vi "NoGV_Omniax_MotorDrive_XYZR_20112StableILK.vi"() -> ()   [LabVIEW 2010]
uses:
  <vilib>/Utility/file.llb/Read From Spreadsheet File (string).vi
  <vilib>/Utility/file.llb/Read From Spreadsheet File (DBL).vi
  <vilib>/Instr/_visa.llb/VISA Configure Serial Port (Instr).vi
  <vilib>/Utility/file.llb/Write To Spreadsheet File (string).vi
  <vilib>/Utility/file.llb/Write To Spreadsheet File (DBL).vi
panel:
  in  "GVposition SP 15360000":i64
  out "Scanning":bool
  out "Laser Shutter":bool
  in  "SHUTTER SYNC":bool
  in  "Laser Shutter":bool
  out "#th loop":dbl
  in  "# of loops":dbl
  in  "LOOP":bool
  out "OP":bool
  out "CL":bool
  out "V5 Valve \nopend/closed":bool
  in  "OK Button":bool
  out "STATUS":string
  in  "Delete Button":bool
  in  "String":string
  in  "Add Button":bool
  in  "Set Button":bool
  in  "Preset positions":i32(ring) items=["ZERO", "Default", "CDOSE", "QMS", "test", "test2", "test3", "yag position", "Sample Long Edge  ", "SPUTTER POS"]
  out "Presets":i32[][](array[numeric])
  out "X MINPOS":i32=-94296
  out "X MAXPOS":i32=-34296
  out "Y MINPOS":i32=-94296
  out "Y MAXPOS":i32=-34296
  out "R MAXPOS":i32=-34296
  out "R MINPOS":i32=-94296
  out "Z MINPOS":i32=-94296
  out "Z MAXPOS":i32=-34296
  in  "HARDSTOP":bool
  in  "GO":bool
  out "XYZR VEL PV Array":i32[](array[numeric])
  out "XYZ in RANGE Array":bool[](array[boolean])
  out "STEP SP Array":i32[](array[numeric])
  out "RUNHOLDArray":i32[](array[numeric])
  out "ZCONSTArray":dbl[](array[numeric])
  out "RCONSTArray":dbl[](array[numeric])
  out "XCONSTArray":dbl[](array[numeric])
  out "YCONSTArray":dbl[](array[numeric])
  out "Error Array":errorcluster[](array[cluster])
  out "COM PORT Array":refnum<visa-resource-name>[](array[refnum])
  out "Z COM PORT":refnum<visa-resource-name>="COM6"
  in  "Tab Control 3":enum32{"Status", "Reset"}(tab)
  out "Y in Range":bool
  out "Y Scan":bool
  out "Y in Motion":bool
  out "Y Backlash corr":bool
  out "X  in Range":bool
  out "X Scan":bool
  out "X  in Motion":bool
  out "X Backlash corr":bool
  out "Z in Range":bool
  out "Z Scan":bool
  out "Z in Motion":bool
  out "Z Backlash corr":bool
  out "R in Range":bool
  out "R Scan":bool
  out "R in Motion":bool
  out "R Backlash corr":bool
  out "X Ready":bool
  out "Y Ready":bool
  out "Z Ready":bool
  out "R Ready":bool
  in  "Reset Y Position mm":dbl
  out "Reset Y Motor Steps":i32
  in  "Reset X Position mm":dbl
  out "Reset X Motor Steps":i32
  in  "Reset Z Position mm":dbl
  out "Reset Z Motor Steps":i32
  in  "Reset R Position deg":dbl
  out "Reset R Motor Steps":i32
  in  "Reset":bool
  in  "Tab Control 2":enum32{"mm", "step"}(tab)
  in  "X Scan Length SP mm":dbl
  in  "X Scan Velocity SP mm/sec":dbl
  in  "Y Scan Length SP mm":dbl
  in  "Y Scan Velocity SP mm/sec":dbl
  in  "Set Scan \nParameters":bool
  in  "Z Scan Length SP mm":dbl
  in  "Z Scan Velocity SP mm/sec":dbl
  in  "R Scan Length SP deg":dbl
  in  "R Scan Velocity SP deg/sec":dbl
  in  "Z as dominating length":bool
  in  "X Scan Velocity SP steps/sec":i32=1 min=1 max=102400 step=1
  in  "X Scan Length SP steps":i32 min=-2304000 max=2304000 step=100
  out "X Scan length MV mm":dbl
  out "X Scan velocity MV mm/sec":dbl format="%#_6f"
  in  "Y Scan Velocity SP steps/sec":i32=1 min=1 max=102400 step=1
  in  "Y Scan Length SP steps":i32 min=-2304000 max=2304000 step=100
  out "Y Scan length MV mm":dbl
  out "Y Scan velocity MV mm/sec":dbl format="%#_6f"
  in  "Z Scan Velocity SP steps/sec":i32=1 min=1 max=204800 step=1
  in  "Z Scan Length SP steps":i32 min=-10240000 max=92160000 step=100
  out "Z Scan length MV mm":dbl
  out "Z Scan velocity MV mm/sec":dbl format="%#_6f"
  in  "R Scan Velocity SP steps/sec":i32=1 min=1 max=102400 step=1
  in  "R Scan Length SP steps":i32 min=-1501867 max=4642133 step=100
  out "R Scan length MV deg":dbl
  out "R Scan velocity MV deg/sec":dbl format="%#_6f"
  out "atan Y/Z":dbl
  in  "Tab Control":enum32{"mm", "step"}(tab)
  in  "X Position SP mm":dbl
  in  "X Velocity SP mm/sec":dbl
  in  "X Move Set":bool
  in  "Y Move Set":bool
  in  "Y Position SP mm":dbl
  in  "Y Velocity SP mm/sec":dbl
  in  "Z Position SP mm":dbl
  in  "Z Velocity SP mm/sec":dbl
  in  "Z Move Set":bool
  in  "R Position SP deg":dbl
  in  "R Velocity SP deg/sec":dbl
  in  "R Move Set":bool
  in  "X Velocity SP step/sec":i32 min=1 max=128000
  out "X Velocity MV mm/sec":dbl
  in  "Y Velocity SP step/sec":i32 min=1 max=128000
  out "Y Velocity MV mm/sec":dbl
  in  "Z Velocity SP step/sec":i32 min=1 max=204800
  out "Z Velocity MV mm/sec":dbl
  in  "R Velocity SP step/sec":i32 min=1 max=20000
  out "R Velocity MVdeg/sec":dbl
  in  "Y Step SP":i32=-20000 min=-2304000 max=2304000 step=500
  out "Y Position MV mm":dbl
  in  "X Step SP":i32=-20000 min=-2304000 max=2304000 step=500
  out "X Position MV mm":dbl
  in  "Z Step SP":i32=-20000 min=0 max=102400000 step=500
  out "Z Position MV mm":dbl
  in  "R Step SP":i32=-20000 min=-6144000 max=0 step=500
  out "R Position MV deg":dbl
  out "X Step PV":i32 max=2000
  out "Y Step PV":i32 max=2000
  out "Z Step PV":i32 max=2000
  out "R Step PV":i32 max=2000
  in  "Clear ZY":bool
  out "ZY Graph":cluster{dbl[], dbl[]}(graph)
  out "ZR Graph":cluster{"Y":dbl[], "Y":dbl[]}[](graph)
  out "XY Graph":cluster{"Y":dbl[], "Y":dbl[]}[](graph)
  out "X Scan Duration":dbl
  out "Y Scan Duration":dbl
  out "Z Scan Duration":dbl
  out "R Scan Duration":dbl
  out "R Backlash steps/sec":i32
  out "R Backlash":i32
  out "R Holding Current %":i32
  out "R Run Current %":i32
  out "R offset deg":dbl
  out "R deg/rev":dbl
  out "R steps/rev":u32
  out "R velocity PV step/sec":i32
  out "R COM PORT":refnum<visa-resource-name>="COM5"
  out "R Position deg PV":dbl=270.5
  out "Z Backlash steps/sec":i32
  out "Z Backlash":i32
  out "Z Holding Current %":i32
  out "Z Run Current %":i32
  out "Z offset mm":dbl
  out "Z mm/rev":dbl
  out "Z steps/rev":u32
  out "Z  velocity PV step/sec":i32
  out "Z Position mm PV":dbl=45.0
  out "X Position mm PV":dbl
  out "X velocity PV step/sec":i32
  in  "Send scan parameter":bool
  out "X Backlash steps/sec":i32
  out "X Backlash":i32
  out "X Holding Current %":i32
  out "X Run Current %":i32
  out "X offset mm":dbl
  out "X mm/rev":dbl
  out "X steps/rev":u32
  out "X COM PORT":refnum<visa-resource-name>="COM5"
  out "Y Backlash steps/sec":i32
  out "Y Backlash":i32
  out "Y Holding Current %":i32
  out "Y Run Current %":i32
  in  "Scan Cancel":bool
  out "Y Position mm PV":dbl
  out "Y offset mm":dbl
  out "Y mm/rev":dbl
  out "Y steps/rev":u32
  out "Y velocity PV step/sec":i32
  in  "Scan Go":bool
  in  "Stop":bool
  out "Y COM PORT":refnum<visa-resource-name>="COM5"
  # "MX"
  # "MY"
  # "MZ"
  # "MR"
  # "V5 Indicators"
  # "L"
  # "M"
  # "B"
  # "S"
  # "R"
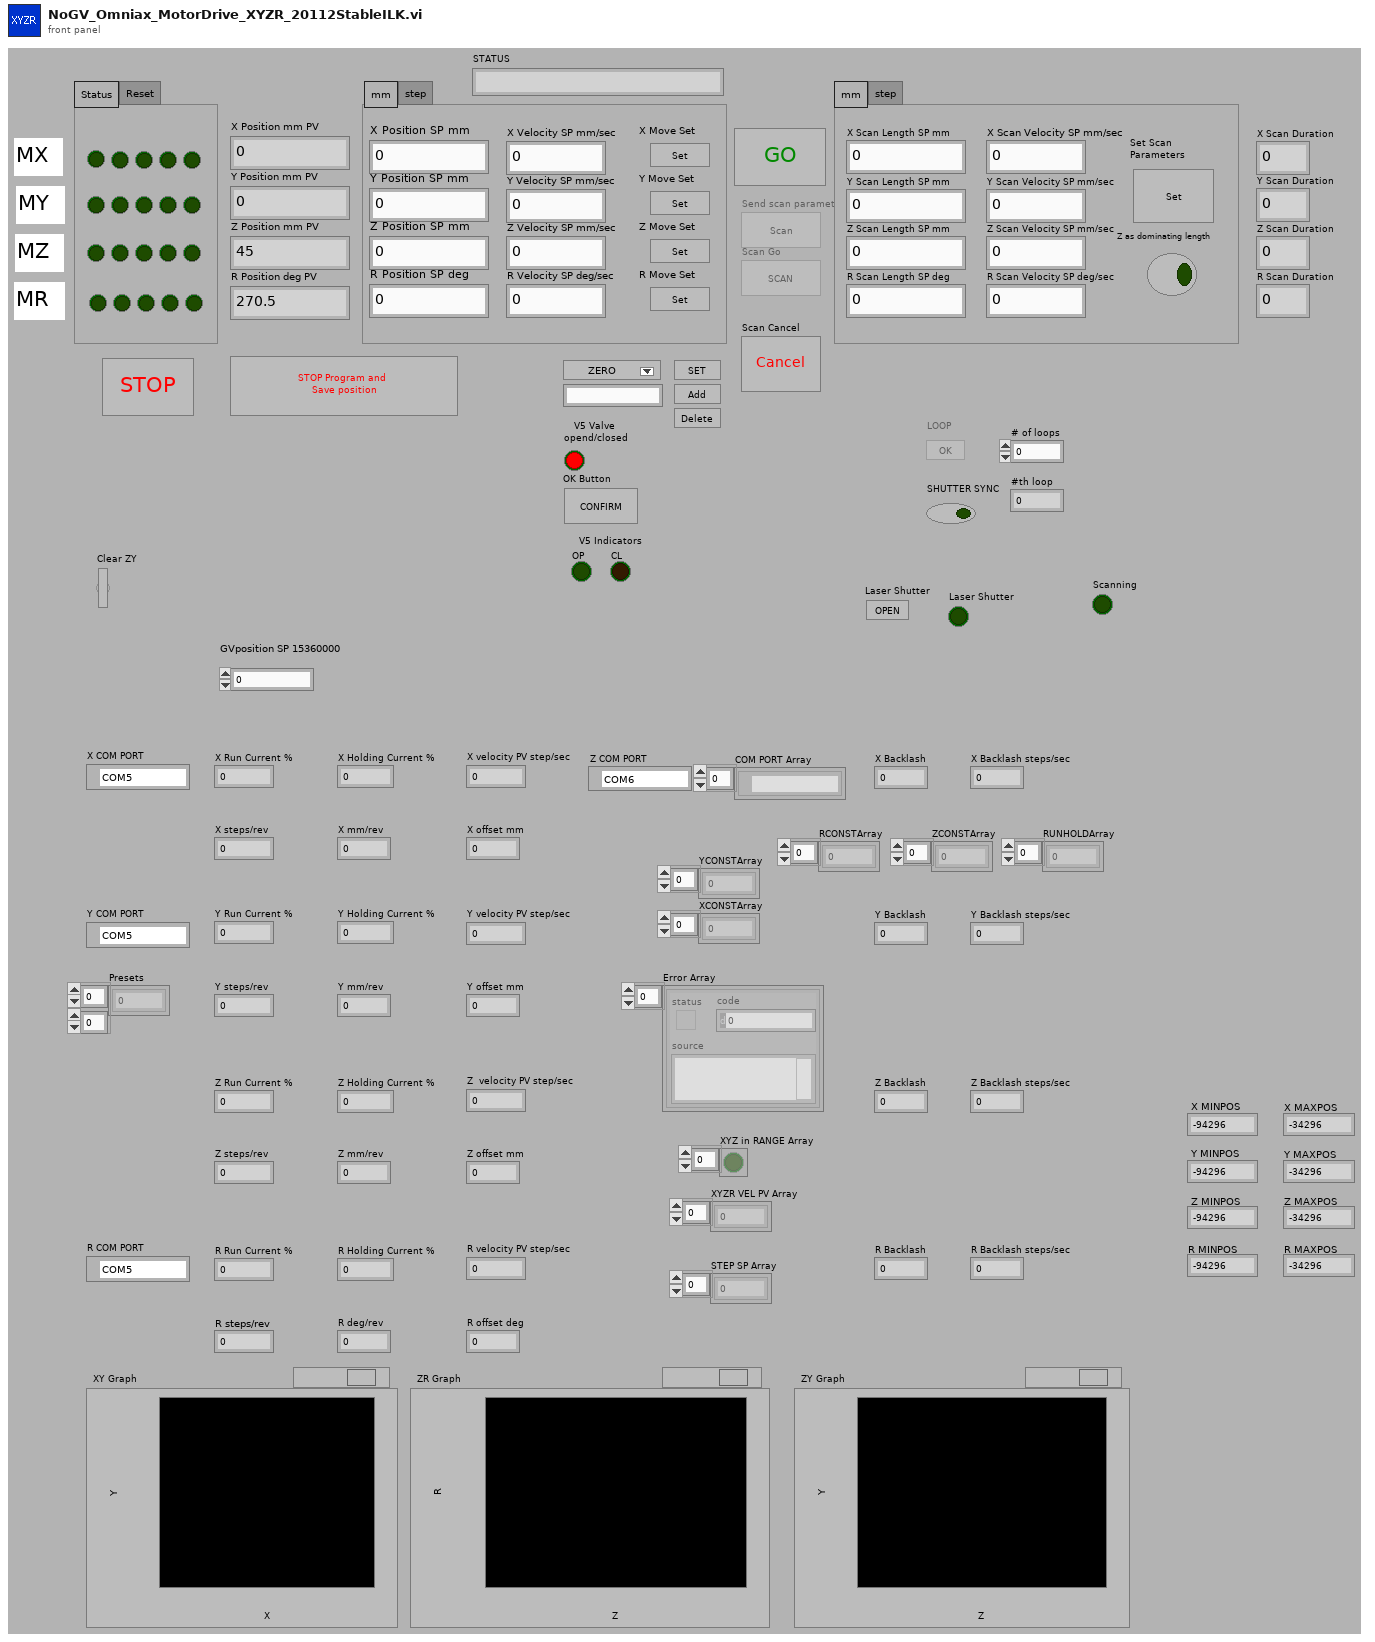
[diagram p1: front panel]
types:
  T1 = cluster{"Error Array OUT[0]":errorcluster, "Error Array OUT[1]":errorcluster, "Error Array OUT[2]":errorcluster, "Error Array OUT[3]":errorcluster, "Error Array OUT[4]":errorcluster, "Error Array OUT[5]":errorcluster, "Error Array OUT[6]":errorcluster, "Error Array OUT[7]":errorcluster, "Error Array OUT[8]":errorcluster}
  T2 = cluster{"COM PORT Array OUT[0]":refnum<visa-resource-name>, "COM PORT Array OUT[1]":refnum<visa-resource-name>, "COM PORT Array OUT[2]":refnum<visa-resource-name>, "COM PORT Array OUT[3]":refnum<visa-resource-name>, "COM PORT Array OUT[4]":refnum<visa-resource-name>, "COM PORT Array OUT[5]":refnum<visa-resource-name>, "COM PORT Array OUT[6]":refnum<visa-resource-name>, "COM PORT Array OUT[7]":refnum<visa-resource-name>, "COM PORT Array OUT[8]":refnum<visa-resource-name>}
  T3 = cluster{"STEP SP Array OUT[0]":i32, "STEP SP Array OUT[1]":i32, "STEP SP Array OUT[2]":i32, "STEP SP Array OUT[3]":i32, "STEP SP Array OUT[4]":i32, "STEP SP Array OUT[5]":i32, "STEP SP Array OUT[6]":i32, "STEP SP Array OUT[7]":i32, "STEP SP Array OUT[8]":i32}
  T4 = cluster{"XYZR MAX MIN POS[0]":i32, "XYZR MAX MIN POS[1]":i32, "XYZR MAX MIN POS[2]":i32, "XYZR MAX MIN POS[3]":i32, "XYZR MAX MIN POS[4]":i32, "XYZR MAX MIN POS[5]":i32, "XYZR MAX MIN POS[6]":i32, "XYZR MAX MIN POS[7]":i32, "XYZR MAX MIN POS[8]":i32}
  T5 = cluster{"XYZ in RANGE Array OUT[0]":bool, "XYZ in RANGE Array OUT[1]":bool, "XYZ in RANGE Array OUT[2]":bool, "XYZ in RANGE Array OUT[3]":bool, "XYZ in RANGE Array OUT[4]":bool, "XYZ in RANGE Array OUT[5]":bool, "XYZ in RANGE Array OUT[6]":bool, "XYZ in RANGE Array OUT[7]":bool, "XYZ in RANGE Array OUT[8]":bool}
  T6 = cluster{"XY Max Min array OUT[0]":dbl, "XY Max Min array OUT[1]":dbl, "XY Max Min array OUT[2]":dbl, "XY Max Min array OUT[3]":dbl, "XY Max Min array OUT[4]":dbl, "XY Max Min array OUT[5]":dbl, "XY Max Min array OUT[6]":dbl, "XY Max Min array OUT[7]":dbl, "XY Max Min array OUT[8]":dbl}
  T7 = cluster{"XYZR VEL PV Array OUT[0]":i32, "XYZR VEL PV Array OUT[1]":i32, "XYZR VEL PV Array OUT[2]":i32, "XYZR VEL PV Array OUT[3]":i32, "XYZR VEL PV Array OUT[4]":i32, "XYZR VEL PV Array OUT[5]":i32, "XYZR VEL PV Array OUT[6]":i32, "XYZR VEL PV Array OUT[7]":i32, "XYZR VEL PV Array OUT[8]":i32}
  T8 = cluster{"[0]":i32, "[1]":i32, "[2]":i32, "[3]":i32, "[4]":i32, "[5]":i32, "[6]":i32, "[7]":i32, "[8]":i32}
  T9 = enum8{"Enabled", "Disabled", "Disabled and Grayed Out"}
  T10 = enum16{"Stop", "Reset", "Run Current", "Holding Current", "Accel Rate", "Decel Rate", "Move to Relative Position", "Move to Absolute Position", "Echo Mode", "Print Parameter", "Send String", "Microstep Resolution", "Set Current Position", "Max Velocity"}
  T11 = cluster{"Presets[0]":i32, "Presets[1]":i32, "Presets[2]":i32, "Presets[3]":i32, "Presets[4]":i32, "Presets[5]":i32, "Presets[6]":i32, "Presets[7]":i32, "Presets[8]":i32}
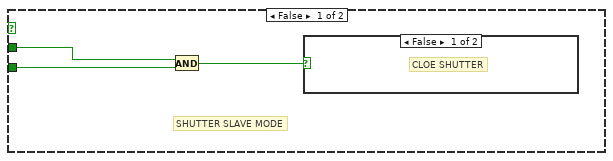
[diagram p2: hidden frame]
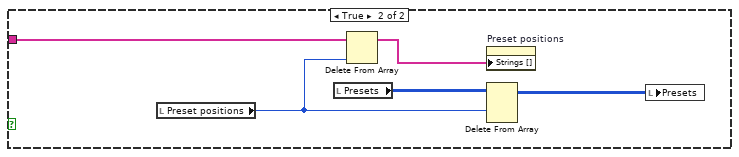
[diagram p4: hidden frame]
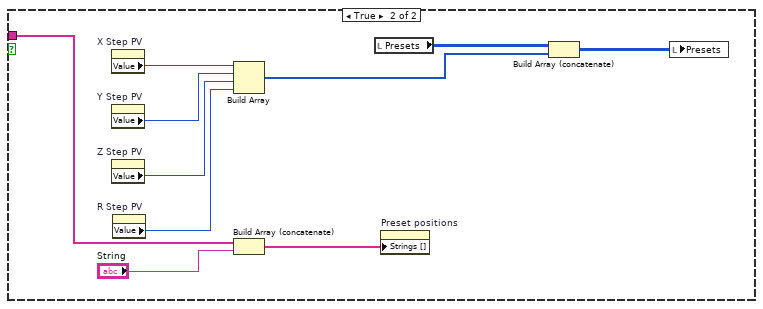
[diagram p5: hidden frame]
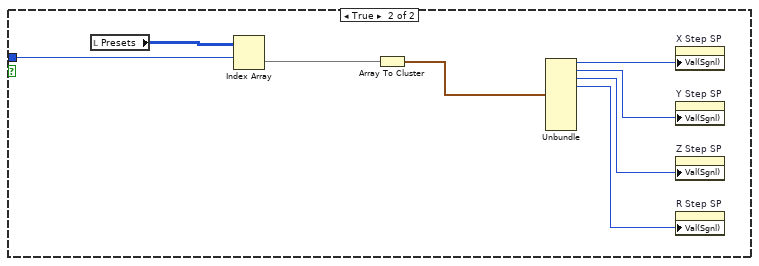
[diagram p6: hidden frame]
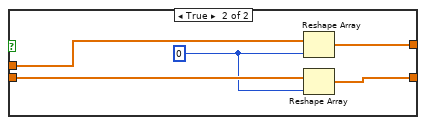
[diagram p8: hidden frame]
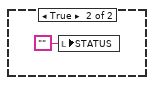
[diagram p10: hidden frame]
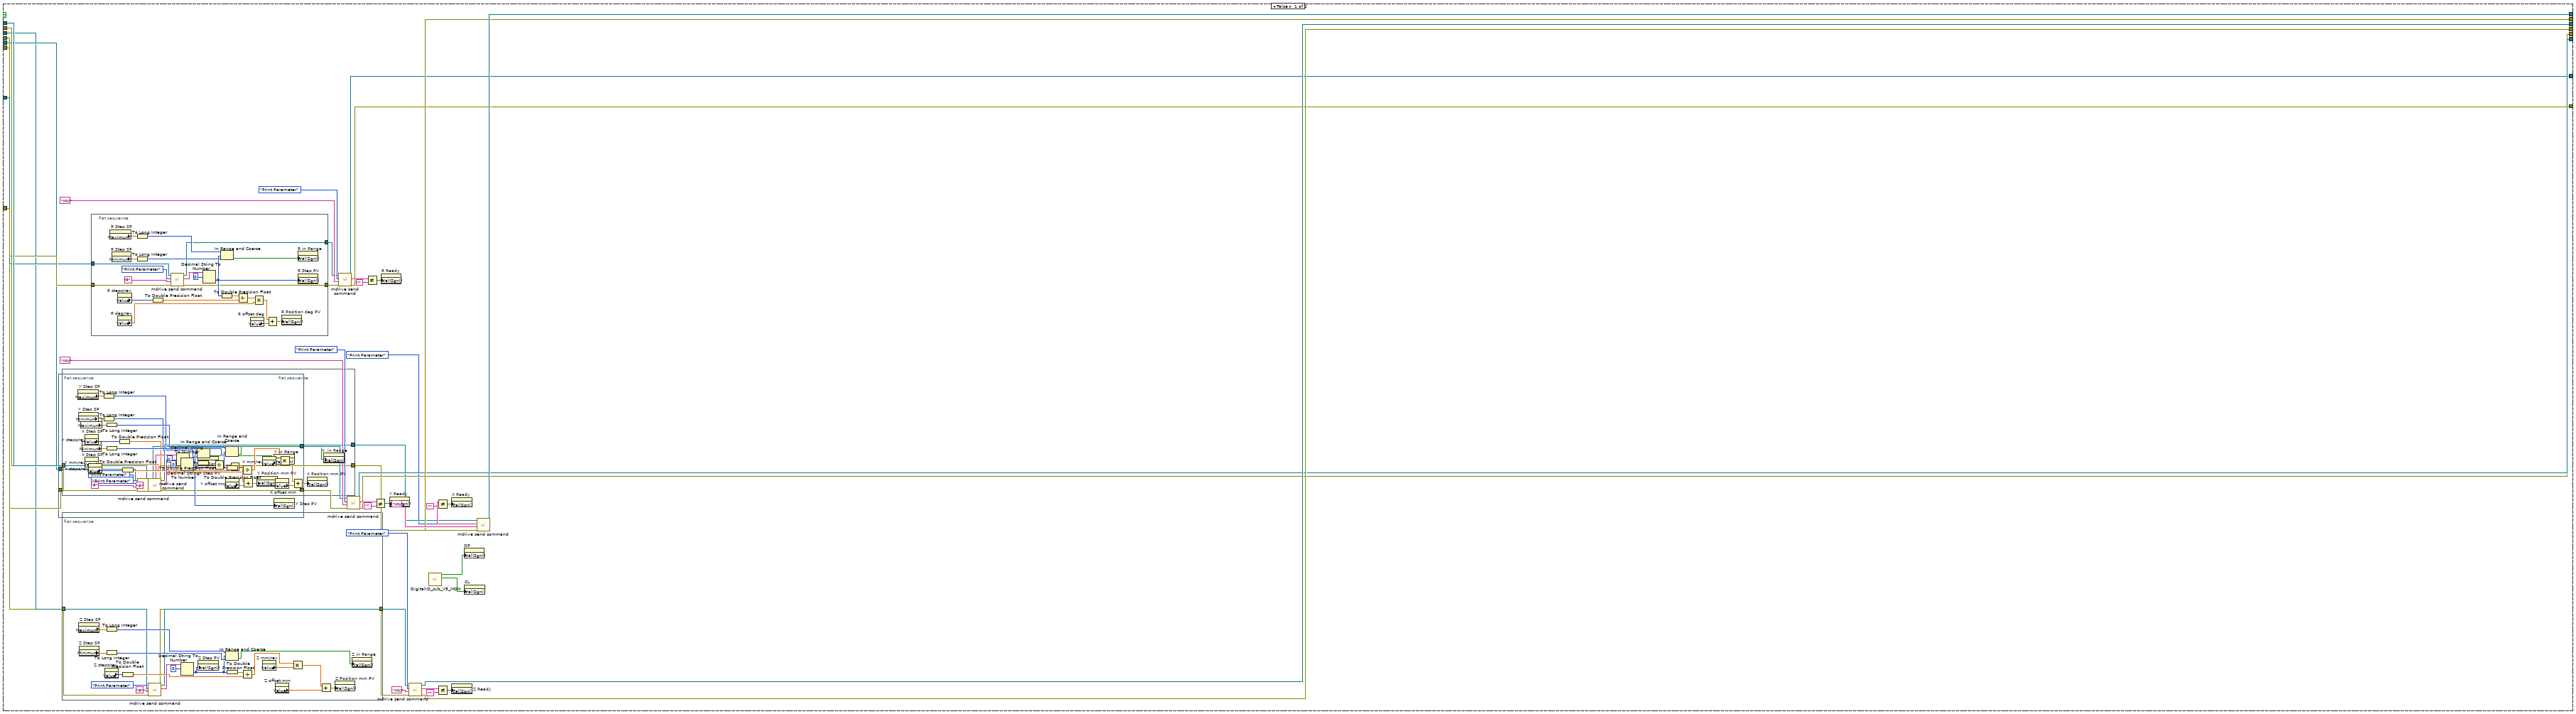
[diagram p11: hidden frame]
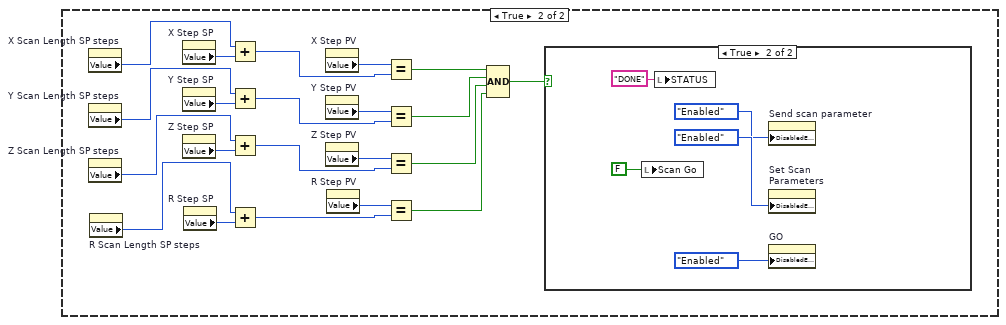
[diagram p14: hidden frame]
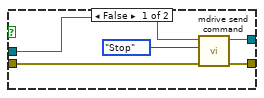
[diagram p16: hidden frame]
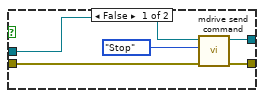
[diagram p18: hidden frame]
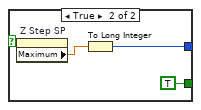
[diagram p20: hidden frame]
diagram:
  (unwired) FALSE ("LOOP MODE")
  n1 = flat-sequence {
    tunnel: [w153] -> w10
    tunnel: [w152] -> w9
    tunnel: [w151] -> w8
    tunnel: [w150] -> w7
    tunnel: [w149] -> w6
    tunnel: [w148] -> w5
    tunnel: [w147] -> w4
    tunnel: [w146] -> w3
    tunnel: [w143] -> w2
    tunnel: [w113] -> w1
    tunnel: [w188] -> w13
    tunnel: [w189] -> w14
    tunnel: [w190] -> w15
    tunnel: [w191] -> w16
    tunnel: [w192] -> w17
    tunnel: [w193] -> w18
    tunnel: [w194] -> w19
    tunnel: [w195] -> w20
    tunnel: [w196] -> w21
    tunnel: [w197] -> w22
    tunnel: w10 -> [w197]
    tunnel: w9 -> [w196]
    tunnel: w8 -> [w195]
    tunnel: w7 -> [w194]
    tunnel: w6 -> [w193]
    tunnel: w5 -> [w192]
    tunnel: w4 -> [w191]
    tunnel: w3 -> [w190]
    tunnel: w2 -> [w189]
    tunnel: w1 -> [w188]
    frame #0 {
      w113 = path "C:/Documents and Settings/b_ogasawara/Desktop/lv1/LV codes/IMS/PRESET.TXT"
      w111 = 0 ("element")
      w143 = path "C:/Documents and Settings/b_ogasawara/Desktop/lv1/LV codes/IMS/POS.TXT"
      w173 = refnum<visa-resource-name> "COM7" ("COM PORT")
      w174 = refnum<visa-resource-name> "COM5" ("COM PORT")
      w175 = refnum<visa-resource-name> "COM6" ("VISA resource name")
      w176 = refnum<visa-resource-name> "COM4" ("COM PORT")
      n2 = property on="Z Step SP" class="DigNum (strict)"() -> ("Maximum"=w68:dbl)  [unwired: 2 in, 2 out]
      n3 = property on="R Step SP" class="DigNum (strict)"() -> ("Maximum"=w66:dbl)  [unwired: 2 in, 2 out]
      n4 = property on="Z Step SP" class="DigNum (strict)"() -> ("Minimum"=w69:dbl)  [unwired: 2 in, 2 out]
      n5 = property on="R Step SP" class="DigNum (strict)"() -> ("Minimum"=w67:dbl)  [unwired: 2 in, 2 out]
      n6 = property on="X steps/rev" class="DigNum (strict)"() -> ("Value"=w84:u32)  [unwired: 2 in, 2 out]
      n7 = property on="Y steps/rev" class="DigNum (strict)"() -> ("Value"=w83:u32)  [unwired: 2 in, 2 out]
      n8 = property on="Z steps/rev" class="DigNum (strict)"() -> ("Value"=w82:u32)  [unwired: 2 in, 2 out]
      n9 = property on="R steps/rev" class="DigNum (strict)"() -> ("Value"=w81:u32)  [unwired: 2 in, 2 out]
      n10 = call "DigitalIO_sub_V5_MON.vi"() -> ("CL"=w70:bool, "OP"=w71:bool)  [unwired: 8 in]
      n11 = local read "RUNHOLDArray"() -> (w163:i32[])
      n12 = local read "STEP SP Array"() -> (w166:i32[])
      n13 = local read "XYZ in RANGE Array"() -> (w165:bool[])
      n14 = local read "XYZR VEL PV Array"() -> (w164:i32[])
      n15 = property on="R offset deg" class="DigNum (strict)"() -> ("Value"=w76:dbl)  [unwired: 2 in, 2 out]
      n16 = property on="X offset mm" class="DigNum (strict)"() -> ("Value"=w73:dbl)  [unwired: 2 in, 2 out]
      n17 = property on="Y offset mm" class="DigNum (strict)"() -> ("Value"=w74:dbl)  [unwired: 2 in, 2 out]
      n18 = property on="Z offset mm" class="DigNum (strict)"() -> ("Value"=w75:dbl)  [unwired: 2 in, 2 out]
      n19 = property on="OP" class="Bool (strict)"("Val(Sgnl)"=w71) -> ()  [unwired: 2 in, 2 out]
      n20 = property on="CL" class="Bool (strict)"("Val(Sgnl)"=w70) -> ()  [unwired: 2 in, 2 out]
      n21 = Build Array(w176, w175, w174, w173) -> (w171:refnum<visa-resource-name>[])
      n22 = Build Array(w68, w69, w66, w67) -> (w65:dbl[])
      n23 = local write "STATUS"("INITIALIZING" ("STATUS")) -> ()
      n24 = for {
        N: 4 -> [_]
        tunnel: w171 -> [w179] mode=indexing
        tunnel: [w178] -> w169 mode=indexing
        tunnel: [w177] -> w170 mode=indexing
        w181 = u16 0 items=["None", "XON/XOFF", "RTS/CTS", "XON/XOFF & RTS/CTS", "DTR/DSR", "XON/XOFF & DTR/DSR"] ("flow control (0:none)")
        w182 = u16 10 items=["1.0"=10, "1.5"=15, "2.0"=20] ("stop bits (10: 1 bit)")
        # "Stop bits"
        n25 = call-poly "VISA Configure Serial Port"("VISA resource name"=w179, "timeout (10sec)"=u32 10000, "baud rate (9600)"=u32 9600, "data bits (8)"=u16 8, "parity (0:none)"=enum16{"None", "Odd", "Even", "Mark", "Space"}."None", "stop bits (10: 1 bit)"=w182, "flow control (0:none)"=w181) -> ("VISA resource name out"=w178:refnum<visa-resource-name>, "error out"=w177:errorcluster)  [unwired: 7 in]
      }
      "COM PORT Array" <- w169
      "Error Array" <- w170
      n26 = call "InitializeMotorsXYZR_V2.vi"("COM PORT Array IN"=w169, "STEP SP Array IN"=w166, "XYZ in RANGE Array IN"=w165, "XYZR VEL PV Array IN"=w164, "RUNHOLDArray IN"=w163, "Error Array IN"=w170, "ZR Max Min array"=w65) -> ("XY Max Min array OUT"=w64:dbl[], "COM PORT Array OUT"=w168:refnum<visa-resource-name>[], "STEP SP Array OUT"=w162:i32[], "XYZ in RANGE Array OUT"=w161:bool[], "XYZR VEL PV Array OUT"=w160:i32[], "XYZR MAX MIN POS"=w145:i32[], "Error Array OUT"=w167:errorcluster[])  [unwired: 6 in]
      n27 = Array To Cluster(array=w167) -> (cluster=w158:T1)
      n28 = Array To Cluster(array=w168) -> (cluster=w159:T2)
      n29 = Array To Cluster(array=w162) -> (cluster=w157:T3)
      n30 = Array To Cluster(array=w145) -> (cluster=w154:T4)
      n31 = Array To Cluster(array=w161) -> (cluster=w156:T5)
      n32 = Array To Cluster(array=w64) -> (cluster=w63:T6)
      n33 = Array To Cluster(array=w160) -> (cluster=w155:T7)
      n34 = Unbundle(w157) -> ("STEP SP Array OUT[0]"=w127:i32, "STEP SP Array OUT[1]"=w128:i32, "STEP SP Array OUT[2]"=w129:i32, "STEP SP Array OUT[3]"=w130:i32)  [unwired: 5 out]
      n35 = Unbundle(w154) -> ("XYZR MAX MIN POS[0]"=w138:i32, "XYZR MAX MIN POS[1]"=w137:i32, "XYZR MAX MIN POS[2]"=w136:i32, "XYZR MAX MIN POS[3]"=w135:i32, "XYZR MAX MIN POS[4]"=w134:i32, "XYZR MAX MIN POS[5]"=w133:i32, "XYZR MAX MIN POS[6]"=w132:i32, "XYZR MAX MIN POS[7]"=w131:i32)  [unwired: 1 out]
      n36 = Unbundle(w156) -> ("XYZ in RANGE Array OUT[0]"=w142:bool, "XYZ in RANGE Array OUT[1]"=w141:bool, "XYZ in RANGE Array OUT[2]"=w140:bool, "XYZ in RANGE Array OUT[3]"=w139:bool)  [unwired: 5 out]
      n37 = Unbundle(w63) -> ("XY Max Min array OUT[0]"=w62:dbl, "XY Max Min array OUT[1]"=w60:dbl, "XY Max Min array OUT[2]"=w59:dbl, "XY Max Min array OUT[3]"=w61:dbl)  [unwired: 5 out]
      n38 = Unbundle(w155) -> ("XYZR VEL PV Array OUT[0]"=w126:i32, "XYZR VEL PV Array OUT[1]"=w125:i32, "XYZR VEL PV Array OUT[2]"=w124:i32, "XYZR VEL PV Array OUT[3]"=w123:i32)  [unwired: 5 out]
      n39 = call-poly <vilib>:"Read From Spreadsheet File.vi"("file path (dialog if empty)"=w113) -> ("all rows"=w118:string[][])  [unwired: 6 in, 4 out]
      n40 = call-poly <vilib>:"Read From Spreadsheet File.vi"("file path (dialog if empty)"=w143) -> ("first row"=w144:dbl[])  [unwired: 6 in, 4 out]
      n41 = To Long Integer(number=w144) -> (32bit integer=w110:i32[])
      n42 = Transpose 2D Array(2D array=w118) -> (transposed array=w117:string[][])
      n43 = property on="X Step SP" class="DigNum (strict)"("Val(Sgnl)"=w127) -> ()  [unwired: 2 in, 2 out]
      n44 = property on="Y Step SP" class="DigNum (strict)"("Val(Sgnl)"=w128) -> ()  [unwired: 2 in, 2 out]
      n45 = property on="Z Step SP" class="DigNum (strict)"("Val(Sgnl)"=w129) -> ()  [unwired: 2 in, 2 out]
      n46 = property on="R Step SP" class="DigNum (strict)"("Val(Sgnl)"=w130) -> ()  [unwired: 2 in, 2 out]
      n47 = property on="X MAXPOS" class="DigNum (strict)"("Val(Sgnl)"=w138) -> ()  [unwired: 2 in, 2 out]
      n48 = property on="X MINPOS" class="DigNum (strict)"("Val(Sgnl)"=w137) -> ()  [unwired: 2 in, 2 out]
      n49 = property on="Y MAXPOS" class="DigNum (strict)"("Val(Sgnl)"=w136) -> ()  [unwired: 2 in, 2 out]
      n50 = property on="Y MINPOS" class="DigNum (strict)"("Val(Sgnl)"=w135) -> ()  [unwired: 2 in, 2 out]
      n51 = property on="Z MAXPOS" class="DigNum (strict)"("Val(Sgnl)"=w134) -> ()  [unwired: 2 in, 2 out]
      n52 = property on="Z MINPOS" class="DigNum (strict)"("Val(Sgnl)"=w133) -> ()  [unwired: 2 in, 2 out]
      n53 = property on="R MAXPOS" class="DigNum (strict)"("Val(Sgnl)"=w132) -> ()  [unwired: 2 in, 2 out]
      n54 = property on="R MINPOS" class="DigNum (strict)"("Val(Sgnl)"=w131) -> ()  [unwired: 2 in, 2 out]
      n55 = property on="X  in Range" class="Bool (strict)"("Val(Sgnl)"=w142) -> ()  [unwired: 2 in, 2 out]
      n56 = property on="Y in Range" class="Bool (strict)"("Val(Sgnl)"=w141) -> ()  [unwired: 2 in, 2 out]
      n57 = property on="Z in Range" class="Bool (strict)"("Val(Sgnl)"=w140) -> ()  [unwired: 2 in, 2 out]
      n58 = property on="R in Range" class="Bool (strict)"("Val(Sgnl)"=w139) -> ()  [unwired: 2 in, 2 out]
      n59 = property on="X velocity PV step/sec" class="DigNum (strict)"("Val(Sgnl)"=w126) -> ()  [unwired: 2 in, 2 out]
      n60 = property on="R velocity PV step/sec" class="DigNum (strict)"("Val(Sgnl)"=w123) -> ()  [unwired: 2 in, 2 out]
      n61 = property on="X Step SP" class="DigNum (strict)"("Maximum"=w62) -> ()  [unwired: 2 in, 2 out]
      n62 = property on="X Step SP" class="DigNum (strict)"("Minimum"=w60) -> ()  [unwired: 2 in, 2 out]
      n63 = property on="Y Step SP" class="DigNum (strict)"("Maximum"=w59) -> ()  [unwired: 2 in, 2 out]
      n64 = property on="Y Step SP" class="DigNum (strict)"("Minimum"=w61) -> ()  [unwired: 2 in, 2 out]
      n65 = property on="Y velocity PV step/sec" class="DigNum (strict)"("Val(Sgnl)"=w125) -> ()  [unwired: 2 in, 2 out]
      n66 = property on="Z  velocity PV step/sec" class="DigNum (strict)"("Val(Sgnl)"=w124) -> ()  [unwired: 2 in, 2 out]
      n67 = Array To Cluster(array=w110) -> (cluster=w109:T8)
      n68 = Delete From Array(array=w117, index (row)=0) -> (deleted portion=w112:string[], array with subset deleted=w115:string[][])  [unwired: 2 in]
      n69 = Transpose 2D Array(2D array=w115) -> (transposed array=w114:string[][])
      n70 = property on="Preset positions" class="Ring (strict)"("Strings []"=w112) -> ()  [unwired: 2 in, 2 out]
      n71 = Unbundle(w109) -> ("[0]"=w85:i32, "[1]"=w86:i32, "[2]"=w87:i32, "[3]"=w88:i32)  [unwired: 5 out]
      n72 = To Double Precision Float(number=w84) -> (double precision float=w105:dbl)
      n73 = To Double Precision Float(number=w85) -> (double precision float=w106:dbl)
      n74 = To Double Precision Float(number=w83) -> (double precision float=w101:dbl)
      n75 = To Double Precision Float(number=w86) -> (double precision float=w102:dbl)
      n76 = To Double Precision Float(number=w87) -> (double precision float=w98:dbl)
      n77 = To Double Precision Float(number=w82) -> (double precision float=w97:dbl)
      n78 = To Double Precision Float(number=w88) -> (double precision float=w94:dbl)
      n79 = To Double Precision Float(number=w81) -> (double precision float=w93:dbl)
      n80 = property on="Reset X Motor Steps" class="DigNum (strict)"("Val(Sgnl)"=w85) -> ()  [unwired: 2 in, 2 out]
      n81 = property on="Reset Y Motor Steps" class="DigNum (strict)"("Val(Sgnl)"=w86) -> ()  [unwired: 2 in, 2 out]
      n82 = property on="Reset Z Motor Steps" class="DigNum (strict)"("Val(Sgnl)"=w87) -> ()  [unwired: 2 in, 2 out]
      n83 = property on="Reset R Motor Steps" class="DigNum (strict)"("Val(Sgnl)"=w88) -> ()  [unwired: 2 in, 2 out]
      n84 = Decimal String To Number(string=w114) -> (number=w116:i32[][])  [unwired: 2 in, 1 out]
      n85 = Divide(x=w106, y=w105) -> (x/y=w108:dbl)
      n86 = Divide(x=w102, y=w101) -> (x/y=w104:dbl)
      n87 = Divide(x=w98, y=w97) -> (x/y=w100:dbl)
      n88 = Divide(x=w94, y=w93) -> (x/y=w96:dbl)
      n89 = Initialize Array(w111, w111, 4 ("dimension size")) -> (w121:i32[][])
      n90 = Build Array (concatenate)(w121, w116) -> (→"Presets":i32[][])
      n91 = property on="X mm/rev" class="DigNum (strict)"() -> ("Value"=w78:dbl)  [unwired: 2 in, 2 out]
      n92 = property on="Y mm/rev" class="DigNum (strict)"() -> ("Value"=w79:dbl)  [unwired: 2 in, 2 out]
      n93 = property on="Z mm/rev" class="DigNum (strict)"() -> ("Value"=w80:dbl)  [unwired: 2 in, 2 out]
      n94 = property on="R deg/rev" class="DigNum (strict)"() -> ("Value"=w77:dbl)  [unwired: 2 in, 2 out]
      n95 = Multiply(x=w108, y=w78) -> (x*y=w107:dbl)
      n96 = Multiply(x=w104, y=w79) -> (x*y=w103:dbl)
      n97 = Multiply(x=w100, y=w80) -> (x*y=w99:dbl)
      n98 = Multiply(x=w96, y=w77) -> (x*y=w95:dbl)
      n99 = Add(x=w107, y=w73) -> (x+y=w89:dbl)
      n100 = Add(x=w103, y=w74) -> (x+y=w90:dbl)
      n101 = Add(x=w99, y=w75) -> (x+y=w91:dbl)
      n102 = Add(x=w95, y=w76) -> (x+y=w92:dbl)
      n103 = property on="X Position mm PV" class="DigNum (strict)"("Val(Sgnl)"=w89) -> ()  [unwired: 2 in, 2 out]
      n104 = property on="X Position SP mm" class="DigNum (strict)"("Val(Sgnl)"=w89) -> ()  [unwired: 2 in, 2 out]
      n105 = property on="Y Position SP mm" class="DigNum (strict)"("Val(Sgnl)"=w90) -> ()  [unwired: 2 in, 2 out]
      n106 = property on="Y Position mm PV" class="DigNum (strict)"("Val(Sgnl)"=w90) -> ()  [unwired: 2 in, 2 out]
      n107 = property on="Z Position SP mm" class="DigNum (strict)"("Val(Sgnl)"=w91) -> ()  [unwired: 2 in, 2 out]
      n108 = property on="Z Position mm PV" class="DigNum (strict)"("Val(Sgnl)"=w91) -> ()  [unwired: 2 in, 2 out]
      n109 = property on="R Position deg PV" class="DigNum (strict)"("Val(Sgnl)"=w92) -> ()  [unwired: 2 in, 2 out]
      n110 = property on="R Position SP deg" class="DigNum (strict)"("Val(Sgnl)"=w92) -> ()  [unwired: 2 in, 2 out]
      n111 = Unbundle(w159) -> ("COM PORT Array OUT[0]"=w153:refnum<visa-resource-name>, "COM PORT Array OUT[1]"=w152:refnum<visa-resource-name>, "COM PORT Array OUT[2]"=w151:refnum<visa-resource-name>, "COM PORT Array OUT[3]"=w150:refnum<visa-resource-name>)  [unwired: 5 out]
      n112 = Unbundle(w158) -> ("Error Array OUT[0]"=w149:errorcluster, "Error Array OUT[1]"=w148:errorcluster, "Error Array OUT[2]"=w147:errorcluster, "Error Array OUT[3]"=w146:errorcluster)  [unwired: 5 out]
      "X COM PORT" <- w176
      "Z COM PORT" <- w175
      "Y COM PORT" <- w174
      "R COM PORT" <- w173
    }
    frame #1 {
      w186 = T9."Disabled and Grayed Out" ("Disabled")
      w187 = T9."Enabled" ("Disabled")
      n113 = property on="LOOP" class="Bool (strict)"("DisabledEnum"=w186) -> ()  [unwired: 2 in, 2 out]
      n114 = property on="GO" class="Bool"("DisabledEnum"=w187) -> ()  [unwired: 2 in, 2 out]
      n115 = property on="Set Scan \nParameters" class="Bool"("DisabledEnum"=w187) -> ()  [unwired: 2 in, 2 out]
      n116 = property on="Send scan parameter" class="Bool"("DisabledEnum"=w186) -> ()  [unwired: 2 in, 2 out]
    }
  }
  n117 = local read "X  in Range"() -> (w33:bool)
  n118 = local read "Z  velocity PV step/sec"() -> (w26:i32)
  n119 = local read "Y in Range"() -> (w32:bool)
  n120 = local read "Z in Range"() -> (w31:bool)
  n121 = local read "R in Range"() -> (w30:bool)
  n122 = local read "X velocity PV step/sec"() -> (w29:i32)
  n123 = local read "Y velocity PV step/sec"() -> (w27:i32)
  n124 = local read "R velocity PV step/sec"() -> (w28:i32)
  n125 = flat-sequence {
    frame #0 {
      n126 = property on="Y Scan" class="Bool (strict)"("Val(Sgnl)"=FALSE ("Value (Signaling)")) -> ()  [unwired: 2 in, 2 out]
      n127 = property on="Z Scan Velocity SP mm/sec" class="DigNum (strict)"("Val(Sgnl)"=0.1 ("Value (Signaling)")) -> ()  [unwired: 2 in, 2 out]
      n128 = property on="Z Scan Velocity SP steps/sec" class="DigNum (strict)"("Minimum"=1.0 ("Data Entry Limits:Maximum")) -> ()  [unwired: 2 in, 2 out]
      n129 = property on="R Scan" class="Bool (strict)"("Val(Sgnl)"=FALSE ("Value (Signaling)")) -> ()  [unwired: 2 in, 2 out]
      n130 = property on="X Scan Velocity SP mm/sec" class="DigNum (strict)"("Val(Sgnl)"=0.1 ("Value (Signaling)")) -> ()  [unwired: 2 in, 2 out]
      n131 = property on="R Velocity SP deg/sec" class="DigNum (strict)"("Val(Sgnl)"=0.1 ("Value (Signaling)")) -> ()  [unwired: 2 in, 2 out]
      n132 = property on="Z Scan Velocity SP steps/sec" class="DigNum (strict)"("Maximum"=204800.0 ("Data Entry Limits:Maximum")) -> ()  [unwired: 2 in, 2 out]
      n133 = property on="X Scan" class="Bool (strict)"("Val(Sgnl)"=FALSE ("Value (Signaling)")) -> ()  [unwired: 2 in, 2 out]
      n134 = property on="Y Scan Velocity SP mm/sec" class="DigNum (strict)"("Val(Sgnl)"=0.1 ("Value (Signaling)")) -> ()  [unwired: 2 in, 2 out]
      n135 = property on="Z Scan" class="Bool (strict)"("Val(Sgnl)"=FALSE ("Value (Signaling)")) -> ()  [unwired: 2 in, 2 out]
      n136 = property on="Scan Go" class="Bool (strict)"("DisabledEnum"=T9."Disabled and Grayed Out" ("Disabled")) -> ()  [unwired: 2 in, 2 out]
    }
  }
  n137 = flat-sequence {
    tunnel: [w212] -> w45
    frame #0 {
      w210 = 0.2 ("MM/rev")
      w215 = u32 51200 ("step/rev")
      w217 = 128000 ("Value (Signaling)")
      w218 = 1.0 ("Data Entry Limits:Minimum")
      w211 = 0.0 ("offset")
      # "a=1000000"
      n138 = property on="X Velocity SP step/sec" class="DigNum (strict)"("Val(Sgnl)"=w217) -> ()  [unwired: 2 in, 2 out]
      n139 = To Double Precision Float(number=w215) -> (double precision float=w220:dbl)
      n140 = To Double Precision Float(number=w217) -> (double precision float=w209:dbl)
      n141 = Divide(x=w209, y=w220) -> (x/y=w219:dbl)
      n142 = property on="X Velocity SP step/sec" class="DigNum (strict)"("Maximum"=w209) -> ()  [unwired: 2 in, 2 out]
      n143 = Multiply(x=w219, y=w210) -> (x*y=w213:dbl)
      n144 = To Double Precision Float(number=w217) -> (double precision float=w216:dbl)
      n145 = To Double Precision Float(number=w215) -> (double precision float=w214:dbl)
      n146 = property on="X Velocity SP step/sec" class="DigNum (strict)"("Minimum"=w218) -> ()  [unwired: 2 in, 2 out]
      n147 = Build Array(w218, w216, w214, w213, w209, w210, w211) -> (w212:dbl[])
      n148 = property on="X Velocity SP mm/sec" class="DigNum (strict)"("Val(Sgnl)"=w213) -> ()  [unwired: 2 in, 2 out]
      "X offset mm" <- w211
      "X steps/rev" <- w215
      "X mm/rev" <- w210
    }
  }
  n149 = flat-sequence {
    tunnel: [w224] -> w46
    frame #0 {
      w222 = 0.2 ("MM/rev")
      w227 = u32 51200 ("step/rev")
      w229 = 128000 ("Value (Signaling)")
      w230 = 1.0 ("Data Entry Limits:Minimum")
      w223 = 0.0 ("offset")
      n150 = property on="Y Velocity SP step/sec" class="DigNum (strict)"("Val(Sgnl)"=w229) -> ()  [unwired: 2 in, 2 out]
      n151 = To Double Precision Float(number=w227) -> (double precision float=w232:dbl)
      n152 = To Double Precision Float(number=w229) -> (double precision float=w221:dbl)
      n153 = Divide(x=w221, y=w232) -> (x/y=w231:dbl)
      n154 = property on="Y Velocity SP step/sec" class="DigNum (strict)"("Maximum"=w221) -> ()  [unwired: 2 in, 2 out]
      n155 = Multiply(x=w231, y=w222) -> (x*y=w225:dbl)
      n156 = To Double Precision Float(number=w229) -> (double precision float=w228:dbl)
      n157 = To Double Precision Float(number=w227) -> (double precision float=w226:dbl)
      n158 = property on="Y Velocity SP step/sec" class="DigNum (strict)"("Minimum"=w230) -> ()  [unwired: 2 in, 2 out]
      n159 = Build Array(w230, w228, w226, w225, w221, w222, w223) -> (w224:dbl[])
      n160 = property on="Y Velocity SP mm/sec" class="DigNum (strict)"("Val(Sgnl)"=w225) -> ()  [unwired: 2 in, 2 out]
      "Y offset mm" <- w223
      "Y steps/rev" <- w227
      "Y mm/rev" <- w222
    }
  }
  n161 = flat-sequence {
    frame #0 {
      n162 = property on="X Backlash corr" class="Bool (strict)"("Val(Sgnl)"=FALSE ("Value (Signaling)")) -> ()  [unwired: 2 in, 2 out]
      n163 = property on="Y Backlash corr" class="Bool (strict)"("Val(Sgnl)"=FALSE ("Value (Signaling)")) -> ()  [unwired: 2 in, 2 out]
      n164 = property on="R Backlash corr" class="Bool (strict)"("Val(Sgnl)"=FALSE ("Value (Signaling)")) -> ()  [unwired: 2 in, 2 out]
      n165 = property on="Z Backlash corr" class="Bool (strict)"("Val(Sgnl)"=FALSE ("Value (Signaling)")) -> ()  [unwired: 2 in, 2 out]
      "Z Backlash steps/sec" <- 25600 ("Z Backlash steps/sec")
      "Z Backlash" <- -12800 ("Z Backlash")
      "X Backlash steps/sec" <- 25600 ("Value (Signaling)")
      "X Backlash" <- 5120 ("Backlash2")
      "Y Backlash" <- -5120 ("Backlash2")
      "Y Backlash steps/sec" <- 25600 ("Value (Signaling)")
      "R Backlash steps/sec" <- 6400 ("R Backlash steps/sec")
      "R Backlash" <- -12800 ("R Backlash")
    }
  }
  n166 = flat-sequence {
    tunnel: [w245] -> w43
    frame #0 {
      w247 = 0.2 ("Z mm/rev")
      w251 = u32 51200 ("step/rev")
      w253 = 204800 ("Value (Signaling)")
      w254 = 1.0 ("Data Entry Limits:Minimum")
      w246 = 0.0 ("Z offset mm")
      n167 = property on="Z Velocity SP step/sec" class="DigNum (strict)"("Val(Sgnl)"=w253) -> ()  [unwired: 2 in, 2 out]
      n168 = To Double Precision Float(number=w251) -> (double precision float=w256:dbl)
      n169 = To Double Precision Float(number=w253) -> (double precision float=w249:dbl)
      n170 = Divide(x=w249, y=w256) -> (x/y=w255:dbl)
      n171 = property on="Z Velocity SP step/sec" class="DigNum (strict)"("Maximum"=w249) -> ()  [unwired: 2 in, 2 out]
      n172 = Multiply(x=w255, y=w247) -> (x*y=w248:dbl)
      n173 = To Double Precision Float(number=w251) -> (double precision float=w250:dbl)
      n174 = To Double Precision Float(number=w253) -> (double precision float=w252:dbl)
      n175 = Build Array(w254, w252, w250, w249, w248, w247, w246) -> (w245:dbl[])
      n176 = property on="Z Velocity SP mm/sec" class="DigNum (strict)"("Val(Sgnl)"=w248) -> ()  [unwired: 2 in, 2 out]
      n177 = property on="Z Velocity SP step/sec" class="DigNum (strict)"("Minimum"=w254) -> ()  [unwired: 2 in, 2 out]
      "Z offset mm" <- w246
      "Z mm/rev" <- w247
      "Z steps/rev" <- w251
    }
  }
  n178 = flat-sequence {
    tunnel: [w257] -> w42
    frame #0 {
      w260 = 20 ("R Holding Current %")
      w259 = 40 ("R Run Current %")
      w262 = 20 ("Holding Current %")
      w261 = 40 ("Run Current %")
      w264 = 20 ("Holding Current %")
      w265 = 40 ("Run Current %")
      w263 = 40 ("Z Run Current %")
      w258 = 20 ("Z Holding Current %")
      n179 = Build Array(w265, w264, w263, w262, w261, w260, w259, w258) -> (w257:i32[])
      "Z Holding Current %" <- w258
      "Z Run Current %" <- w263
      "X Run Current %" <- w265
      "X Holding Current %" <- w264
      "Y Run Current %" <- w261
      "Y Holding Current %" <- w262
      "R Holding Current %" <- w260
      "R Run Current %" <- w259
    }
  }
  n180 = flat-sequence {
    tunnel: [w266] -> w44
    frame #0 {
      w275 = 1.0 ("Data Entry Limits:Minimum")
      w269 = 0.0 ("R offset deg")
      w270 = -3.0 ("R deg/rev")
      w273 = u32 51200 ("step/rev")
      w274 = 20000 ("Value (Signaling)")
      n181 = property on="R Velocity SP step/sec" class="DigNum (strict)"("Val(Sgnl)"=w274) -> ()  [unwired: 2 in, 2 out]
      n182 = To Double Precision Float(number=w273) -> (double precision float=w276:dbl)
      n183 = To Double Precision Float(number=w274) -> (double precision float=w272:dbl)
      n184 = Divide(x=w272, y=w276) -> (x/y=w278:dbl)
      n185 = property on="R Velocity SP step/sec" class="DigNum (strict)"("Maximum"=w272) -> ()  [unwired: 2 in, 2 out]
      n186 = Multiply(x=w278, y=w270) -> (x*y=w277:dbl)
      n187 = To Double Precision Float(number=w273) -> (double precision float=w267:dbl)
      n188 = To Double Precision Float(number=w274) -> (double precision float=w268:dbl)
      n189 = Absolute Value(x=w277) -> (abs(x)=w271:dbl)
      n190 = Build Array(w275, w268, w267, w272, w271, w270, w269) -> (w266:dbl[])
      n191 = property on="R Velocity SP deg/sec" class="DigNum (strict)"("Val(Sgnl)"=w271) -> ()  [unwired: 2 in, 2 out]
      n192 = property on="R Velocity SP step/sec" class="DigNum (strict)"("Minimum"=w275) -> ()  [unwired: 2 in, 2 out]
      "R offset deg" <- w269
      "R deg/rev" <- w270
      "R steps/rev" <- w273
    }
  }
  n193 = property on="Z Step SP" class="DigNum (strict)"("Minimum"=0.0 ("lower limit")) -> ()  [unwired: 2 in, 2 out]
  n194 = property on="R Step SP" class="DigNum (strict)"("Maximum"=0.0 ("Data Entry Limits:Maximum")) -> ()  [unwired: 2 in, 2 out]
  n195 = property on="R Step SP" class="DigNum (strict)"("Minimum"=-6144000.0 ("Data Entry Limits:Minimum")) -> ()  [unwired: 2 in, 2 out]
  n196 = property on="Z Step SP" class="DigNum (strict)"("Maximum"=102400000.0 ("upper limit")) -> ()  [unwired: 2 in, 2 out]
  n197 = Build Array(w33, w32, w31, w30) -> (→"XYZ in RANGE Array":bool[])
  n198 = Build Array("X Step SP", "Y Step SP", "Z Step SP", "R Step SP", "X Velocity SP step/sec", "Y Velocity SP step/sec", "Z Velocity SP step/sec", "R Velocity SP step/sec") -> (→"STEP SP Array":i32[])
  n199 = Build Array(w29, w27, w26, w28) -> (→"XYZR VEL PV Array":i32[])
  n200 = while {
    tunnel: [w306] -> w49
    tunnel: [w309] -> w50
    tunnel: [w312] -> w58
    tunnel: [w305] -> w57
    tunnel: [w311] -> w52
    tunnel: [w310] -> w51
    tunnel: [w308] -> w48
    tunnel: [w307] -> w47
    tunnel: w22 -> [w320]
    tunnel: w21 -> [w318]
    tunnel: w20 -> [w316]
    tunnel: w19 -> [w314]
    tunnel: w18 -> [w319]
    tunnel: w17 -> [w317]
    tunnel: w16 -> [w315]
    tunnel: w15 -> [w313]
    tunnel: w14 -> [w302]
    tunnel: w13 -> [w301]
    shift-right: [w295] -> _
    shift-left: dbl[] [] -> [w293]
    shift-right: [w294] -> _
    shift-left: dbl[] [] -> [w292]
    stop <- w303 stop-if-true
    # "XZYR"
    n201 = property on="Preset positions" class="Ring (strict)"() -> ("Strings []"=w296:string[])  [unwired: 2 in, 2 out]
    n202 = event shown="[0] Timeout" {
      selector: _ -> [_ _ _ _ _ _ _ _ _ _ _ _ _ _ _ _ _]
      dyn-events: _ -> [_ _ _ _ _ _ _ _ _ _ _ _ _ _ _ _ _]
      timeout: 100 -> [_ _ _ _ _ _ _ _ _ _ _ _ _ _ _ _ _]
      tunnel: w320 -> [w524 _ w1396 w1692 _ _ _ _ _ _ _ _ w2222 w2356 w2423 w2653 w2701]
      tunnel: w319 -> [w523 _ w1395 w1713 _ _ _ _ _ _ _ _ w2223 w2354 w2422 w2657 w2697]
      tunnel: w318 -> [w522 _ w1393 w1695 _ _ _ _ _ _ _ _ w2190 w2355 w2421 w2652 w2699]
      tunnel: w317 -> [w521 _ w1394 w1712 _ _ _ _ _ _ _ _ w2191 w2353 w2420 w2656 w2695]
      tunnel: w316 -> [w520 _ w1391 w1698 _ _ _ _ _ _ _ _ w2202 w2352 w2419 w2651 w2693]
      tunnel: w315 -> [w519 _ w1392 w1711 _ _ _ _ _ _ _ _ w2203 w2350 w2418 w2655 w2691]
      tunnel: w314 -> [w518 _ w1389 w1701 _ _ _ _ _ _ _ _ w2178 w2351 w2417 w2650 w2705]
      tunnel: w313 -> [w517 _ w1390 w1710 _ _ _ _ _ _ _ _ w2179 w2349 w2416 w2654 w2703]
      tunnel: [w500 _ _ _ _ _ _ _ _ _ _ _ _ _ _ _ _] -> w295
      tunnel: [w498 _ _ _ _ _ _ _ _ _ _ _ _ _ _ _ _] -> w294
      tunnel: w293 -> [w503 _ _ _ _ _ _ _ _ _ _ _ _ _ _ _ _]
      tunnel: w292 -> [w502 _ _ _ _ _ _ _ _ _ _ _ _ _ _ _ _]
      tunnel: [w496 _ w1374 _ _ _ _ _ _ _ _ _ _ _ _ _ _] -> w286
      tunnel: [w495 _ w1373 _ _ _ _ _ _ _ _ _ _ _ _ _ _] -> w283
      tunnel: [w494 _ w1372 _ _ _ _ _ _ _ _ _ _ _ _ _ _] -> w285
      tunnel: [w493 _ w1371 _ _ _ _ _ _ _ _ _ _ _ _ _ _] -> w284
      tunnel: [w490 _ w1370 _ _ _ _ _ _ _ _ _ _ _ _ _ _] -> w282
      tunnel: [w489 _ w1369 _ _ _ _ _ _ _ _ _ _ _ _ _ _] -> w281
      tunnel: [w492 _ w1368 _ _ _ _ _ _ _ _ _ _ _ _ _ _] -> w279
      tunnel: [_ _ w1367 _ _ _ _ _ _ _ _ _ _ _ _ _ _] -> w280
      tunnel: [w491 _ _ _ _ _ _ _ _ _ _ _ _ _ _ _ _] -> _
      event Timeout {
        # "R"
        # "Y"
        # "Z"
        # "X"
        n203 = event-data() -> ()  [unwired: 1 in, 2 out]
        n204 = property on="X Position mm PV" class="DigNum (strict)"() -> ("Value"=w537:dbl)  [unwired: 2 in, 2 out]
        n205 = property on="Z Position mm PV" class="DigNum (strict)"() -> ("Value"=w506:dbl)  [unwired: 2 in, 2 out]
        n206 = property on="Y Position mm PV" class="DigNum (strict)"() -> ("Value"=w505:dbl)  [unwired: 2 in, 2 out]
        n207 = property on="R Position deg PV" class="DigNum (strict)"() -> ("Value"=w538:dbl)  [unwired: 2 in, 2 out]
        n208 = property on="GO" class="Bool"() -> ("DisabledEnum"=w513:T9)  [unwired: 2 in, 2 out]
        n209 = property on="Y Scan Length SP steps" class="DigNum (strict)"() -> ("Value"=w527:i32)  [unwired: 2 in, 2 out]
        n210 = property on="Z Scan Length SP steps" class="DigNum (strict)"() -> ("Value"=w528:i32)  [unwired: 2 in, 2 out]
        n211 = call "Build XY Graph2"("Reset"=TRUE, "Y Input"=w538, "X Input"=w506) -> ("XY Graph"=→"ZR Graph":cluster{"Y":dbl[], "Y":dbl[]}[])  [unwired: 7 in, 1 out]
        n212 = call "Build XY Graph"("Reset"=TRUE, "Y Input"=w505, "X Input"=w537) -> ("XY Graph"=→"XY Graph":cluster{"Y":dbl[], "Y":dbl[]}[])  [unwired: 7 in, 1 out]
        n213 = Build Array (concatenate)(w503, w506) -> (w501:dbl[])
        n214 = Build Array (concatenate)(w502, w505) -> (w499:dbl[])
        n215 = Equal?(x=w513, y=T9."Enabled") -> (x = y?=w511:bool)
        n216 = To Double Precision Float(number=w527) -> (double precision float=w526:dbl)
        n217 = To Double Precision Float(number=w528) -> (double precision float=w525:dbl)
        n218 = Bundle(w501, w499) -> (→"ZY Graph":cluster{dbl[], dbl[]})  [unwired: 1 in]
        n219 = property on="Clear ZY" class="Bool (strict)"() -> ("Value"=w497:bool)  [unwired: 2 in, 2 out]
        n220 = property on="Scan Go" class="Bool (strict)"() -> ("DisabledEnum"=w510:T9)  [unwired: 2 in, 2 out]
        n221 = property on="GO" class="Bool"() -> ("DisabledEnum"=w516:T9)  [unwired: 2 in, 2 out]
        n222 = Divide(x=w526, y=w525) -> (x/y=w529:dbl)
        n223 = Equal?(x=w510, y=T9."Disabled and Grayed Out") -> (x = y?=w507:bool)
        n224 = Equal?(x=w516, y=T9."Disabled and Grayed Out") -> (x = y?=w514:bool)
        n225 = Inverse Tangent(1:w529) -> (0:w530:dbl)
        n226 = case shown="True" w514 {
          tunnel: [w580 w706] -> w496
          tunnel: [w579 w705] -> w495
          tunnel: [w578 w704] -> w494
          tunnel: [w577 w703] -> w493
          tunnel: [w576 w702] -> w490
          tunnel: [w575 w701] -> w489
          tunnel: [w574 w700] -> w492
          tunnel: [w573 w699] -> w491
          tunnel: w524 -> [w566 w698]
          tunnel: w523 -> [w564 w697]
          tunnel: w522 -> [w553 w696]
          tunnel: w521 -> [w552 w695]
          tunnel: w520 -> [w557 w694]
          tunnel: w519 -> [w556 w693]
          tunnel: w518 -> [w562 w692]
          tunnel: w517 -> [w563 w691]
          frame False {
            n227 = flat-sequence {
              tunnel: [w621] -> w558
              tunnel: w557 -> [w620]
              tunnel: [w619] -> w559
              tunnel: w556 -> [w618]
              frame #0 {
                n228 = property on="Y Step SP" class="DigNum (strict)"() -> ("Maximum"=w635:dbl)  [unwired: 2 in, 2 out]
                n229 = property on="Y Step SP" class="DigNum (strict)"() -> ("Minimum"=w637:dbl)  [unwired: 2 in, 2 out]
                n230 = property on="Y steps/rev" class="DigNum (strict)"() -> ("Value"=w632:u32)  [unwired: 2 in, 2 out]
                n231 = property on="Y mm/rev" class="DigNum (strict)"() -> ("Value"=w630:dbl)  [unwired: 2 in, 2 out]
                n232 = To Long Integer(number=w635) -> (32bit integer=w634:i32)
                n233 = To Long Integer(number=w637) -> (32bit integer=w636:i32)
                n234 = To Double Precision Float(number=w632) -> (double precision float=w633:dbl)
                n235 = call "mdrive send command.vi"("error in (no error)"=w618, "Extra"="P", "Command"=T10."Print Parameter", "VISA resource name"=w620) -> ("error out"=w619:errorcluster, "read buffer"=w639:string, "VISA resource name out"=w621:refnum<visa-resource-name>)  [unwired: 3 in]
                n236 = Decimal String To Number(string=w639, offset=0) -> (number=w622:i32)  [unwired: 1 in, 1 out]
                n237 = In Range and Coerce(upper limit=w634, x=w622, lower limit=w636) -> (In Range?=w623:bool)  [unwired: 1 out]
                n238 = To Double Precision Float(number=w622) -> (double precision float=w627:dbl)
                n239 = Divide(x=w627, y=w633) -> (x/y=w631:dbl)
                n240 = property on="Y offset mm" class="DigNum (strict)"() -> ("Value"=w628:dbl)  [unwired: 2 in, 2 out]
                n241 = Multiply(x=w631, y=w630) -> (x*y=w629:dbl)
                n242 = Add(x=w629, y=w628) -> (x+y=w626:dbl)
                n243 = property on="Y Position mm PV" class="DigNum (strict)"("Val(Sgnl)"=w626) -> ()  [unwired: 2 in, 2 out]
                n244 = property on="Y in Range" class="Bool (strict)"("Val(Sgnl)"=w623) -> ()  [unwired: 2 in, 2 out]
                n245 = property on="Y Step PV" class="DigNum (strict)"("Val(Sgnl)"=w622) -> ()  [unwired: 2 in, 2 out]
              }
            }
            n246 = flat-sequence {
              tunnel: [w665] -> w551
              tunnel: w566 -> [w664]
              tunnel: [w663] -> w565
              tunnel: w564 -> [w662]
              frame #0 {
                n247 = property on="X Step SP" class="DigNum (strict)"() -> ("Maximum"=w679:dbl)  [unwired: 2 in, 2 out]
                n248 = property on="X Step SP" class="DigNum (strict)"() -> ("Minimum"=w681:dbl)  [unwired: 2 in, 2 out]
                n249 = property on="X steps/rev" class="DigNum (strict)"() -> ("Value"=w676:u32)  [unwired: 2 in, 2 out]
                n250 = To Long Integer(number=w679) -> (32bit integer=w678:i32)
                n251 = To Long Integer(number=w681) -> (32bit integer=w680:i32)
                n252 = To Double Precision Float(number=w676) -> (double precision float=w677:dbl)
                n253 = call "mdrive send command.vi"("error in (no error)"=w662, "Extra"="P", "Command"=T10."Print Parameter", "VISA resource name"=w664) -> ("error out"=w663:errorcluster, "read buffer"=w683:string, "VISA resource name out"=w665:refnum<visa-resource-name>)  [unwired: 3 in]
                n254 = Decimal String To Number(string=w683, offset=0) -> (number=w666:i32)  [unwired: 1 in, 1 out]
                n255 = property on="X Step PV" class="DigNum (strict)"("Val(Sgnl)"=w666) -> ()  [unwired: 2 in, 2 out]
                n256 = In Range and Coerce(upper limit=w678, x=w666, lower limit=w680) -> (In Range?=w667:bool)  [unwired: 1 out]
                n257 = To Double Precision Float(number=w666) -> (double precision float=w671:dbl)
                n258 = Divide(x=w671, y=w677) -> (x/y=w675:dbl)
                n259 = property on="X mm/rev" class="DigNum (strict)"() -> ("Value"=w674:dbl)  [unwired: 2 in, 2 out]
                n260 = property on="X offset mm" class="DigNum (strict)"() -> ("Value"=w672:dbl)  [unwired: 2 in, 2 out]
                n261 = Multiply(x=w675, y=w674) -> (x*y=w673:dbl)
                n262 = Add(x=w673, y=w672) -> (x+y=w670:dbl)
                n263 = property on="X Position mm PV" class="DigNum (strict)"("Val(Sgnl)"=w670) -> ()  [unwired: 2 in, 2 out]
                n264 = property on="X  in Range" class="Bool (strict)"("Val(Sgnl)"=w667) -> ()  [unwired: 2 in, 2 out]
              }
            }
            n265 = flat-sequence {
              tunnel: [w599] -> w555
              tunnel: [w598] -> w554
              tunnel: w553 -> [w597]
              tunnel: w552 -> [w596]
              frame #0 {
                n266 = property on="Z Step SP" class="DigNum (strict)"() -> ("Maximum"=w613:dbl)  [unwired: 2 in, 2 out]
                n267 = property on="Z Step SP" class="DigNum (strict)"() -> ("Minimum"=w615:dbl)  [unwired: 2 in, 2 out]
                n268 = property on="Z steps/rev" class="DigNum (strict)"() -> ("Value"=w610:u32)  [unwired: 2 in, 2 out]
                n269 = To Long Integer(number=w613) -> (32bit integer=w612:i32)
                n270 = To Long Integer(number=w615) -> (32bit integer=w614:i32)
                n271 = To Double Precision Float(number=w610) -> (double precision float=w611:dbl)
                n272 = call "mdrive send command.vi"("error in (no error)"=w596, "Extra"="P", "Command"=T10."Print Parameter", "VISA resource name"=w597) -> ("error out"=w598:errorcluster, "read buffer"=w617:string, "VISA resource name out"=w599:refnum<visa-resource-name>)  [unwired: 3 in]
                n273 = Decimal String To Number(string=w617, offset=0) -> (number=w600:i32)  [unwired: 1 in, 1 out]
                n274 = property on="Z Step PV" class="DigNum (strict)"("Val(Sgnl)"=w600) -> ()  [unwired: 2 in, 2 out]
                n275 = In Range and Coerce(upper limit=w612, x=w600, lower limit=w614) -> (In Range?=w601:bool)  [unwired: 1 out]
                n276 = To Double Precision Float(number=w600) -> (double precision float=w605:dbl)
                n277 = Divide(x=w605, y=w611) -> (x/y=w609:dbl)
                n278 = property on="Z mm/rev" class="DigNum (strict)"() -> ("Value"=w608:dbl)  [unwired: 2 in, 2 out]
                n279 = property on="Z offset mm" class="DigNum (strict)"() -> ("Value"=w606:dbl)  [unwired: 2 in, 2 out]
                n280 = Multiply(x=w609, y=w608) -> (x*y=w607:dbl)
                n281 = Add(x=w607, y=w606) -> (x+y=w604:dbl)
                n282 = property on="Z Position mm PV" class="DigNum (strict)"("Val(Sgnl)"=w604) -> ()  [unwired: 2 in, 2 out]
                n283 = property on="Z in Range" class="Bool (strict)"("Val(Sgnl)"=w601) -> ()  [unwired: 2 in, 2 out]
              }
            }
            n284 = flat-sequence {
              tunnel: [w643] -> w560
              tunnel: w562 -> [w642]
              tunnel: [w641] -> w561
              tunnel: w563 -> [w640]
              frame #0 {
                n285 = property on="R Step SP" class="DigNum (strict)"() -> ("Maximum"=w657:dbl)  [unwired: 2 in, 2 out]
                n286 = property on="R Step SP" class="DigNum (strict)"() -> ("Minimum"=w659:dbl)  [unwired: 2 in, 2 out]
                n287 = property on="R steps/rev" class="DigNum (strict)"() -> ("Value"=w654:u32)  [unwired: 2 in, 2 out]
                n288 = property on="R deg/rev" class="DigNum (strict)"() -> ("Value"=w652:dbl)  [unwired: 2 in, 2 out]
                n289 = To Long Integer(number=w657) -> (32bit integer=w656:i32)
                n290 = To Long Integer(number=w659) -> (32bit integer=w658:i32)
                n291 = To Double Precision Float(number=w654) -> (double precision float=w655:dbl)
                n292 = call "mdrive send command.vi"("error in (no error)"=w640, "Extra"="P", "Command"=T10."Print Parameter", "VISA resource name"=w642) -> ("error out"=w641:errorcluster, "read buffer"=w661:string, "VISA resource name out"=w643:refnum<visa-resource-name>)  [unwired: 3 in]
                n293 = Decimal String To Number(string=w661, offset=0) -> (number=w644:i32)  [unwired: 1 in, 1 out]
                n294 = In Range and Coerce(upper limit=w656, x=w644, lower limit=w658) -> (In Range?=w645:bool)  [unwired: 1 out]
                n295 = To Double Precision Float(number=w644) -> (double precision float=w649:dbl)
                n296 = Divide(x=w649, y=w655) -> (x/y=w653:dbl)
                n297 = property on="R offset deg" class="DigNum (strict)"() -> ("Value"=w650:dbl)  [unwired: 2 in, 2 out]
                n298 = Multiply(x=w653, y=w652) -> (x*y=w651:dbl)
                n299 = Add(x=w651, y=w650) -> (x+y=w648:dbl)
                n300 = property on="R Position deg PV" class="DigNum (strict)"("Val(Sgnl)"=w648) -> ()  [unwired: 2 in, 2 out]
                n301 = property on="R in Range" class="Bool (strict)"("Val(Sgnl)"=w645) -> ()  [unwired: 2 in, 2 out]
                n302 = property on="R Step PV" class="DigNum (strict)"("Val(Sgnl)"=w644) -> ()  [unwired: 2 in, 2 out]
              }
            }
            n303 = call "mdrive send command.vi"("error in (no error)"=w561, "Extra"="MV", "Command"=T10."Print Parameter", "VISA resource name"=w560) -> ("error out"=w573:errorcluster, "read buffer"=w582:string, "VISA resource name out"=w574:refnum<visa-resource-name>)  [unwired: 3 in]
            n304 = call "mdrive send command.vi"("error in (no error)"=w559, "Extra"="MV", "Command"=T10."Print Parameter", "VISA resource name"=w558) -> ("error out"=w575:errorcluster, "read buffer"=w586:string, "VISA resource name out"=w576:refnum<visa-resource-name>)  [unwired: 3 in]
            n305 = Not Equal?(x=w582, y="") -> (x != y?=w569:bool)
            n306 = Not Equal?(x=w586, y="") -> (x != y?=w570:bool)
            n307 = property on="R Ready" class="Bool (strict)"("Val(Sgnl)"=w569) -> ()  [unwired: 2 in, 2 out]
            n308 = property on="Y Ready" class="Bool (strict)"("Val(Sgnl)"=w570) -> ()  [unwired: 2 in, 2 out]
            n309 = call "mdrive send command.vi"("error in (no error)"=w554, "Extra"="MV", "Command"=T10."Print Parameter", "VISA resource name"=w555) -> ("error out"=w577:errorcluster, "read buffer"=w590:string, "VISA resource name out"=w578:refnum<visa-resource-name>)  [unwired: 3 in]
            n310 = call "DigitalIO_sub_V5_MON.vi"() -> ("CL"=w567:bool, "OP"=w568:bool)  [unwired: 8 in]
            n311 = Not Equal?(x=w590, y="") -> (x != y?=w571:bool)
            n312 = property on="Z Ready" class="Bool (strict)"("Val(Sgnl)"=w571) -> ()  [unwired: 2 in, 2 out]
            n313 = property on="OP" class="Bool (strict)"("Val(Sgnl)"=w568) -> ()  [unwired: 2 in, 2 out]
            n314 = property on="CL" class="Bool (strict)"("Val(Sgnl)"=w567) -> ()  [unwired: 2 in, 2 out]
            n315 = call "mdrive send command.vi"("error in (no error)"=w565, "Extra"="MV", "Command"=T10."Print Parameter", "VISA resource name"=w551) -> ("error out"=w579:errorcluster, "read buffer"=w594:string, "VISA resource name out"=w580:refnum<visa-resource-name>)  [unwired: 3 in]
            n316 = Not Equal?(x=w594, y="") -> (x != y?=w572:bool)
            n317 = property on="X Ready" class="Bool (strict)"("Val(Sgnl)"=w572) -> ()  [unwired: 2 in, 2 out]
          }
          frame True {
            n318 = flat-sequence {
              tunnel: [w1070] -> w748
              tunnel: [w1081] -> w747
              tunnel: [w1080] -> w746
              tunnel: w696 -> [w1084]
              tunnel: w695 -> [w1083]
              tunnel: [w1120] -> w745
              tunnel: [w1119] -> w744
              tunnel: [w1118] -> w743
              tunnel: [w1111] -> w742
              tunnel: w748 -> [w1118]
              tunnel: w747 -> [w1117]
              tunnel: w746 -> [w1116]
              tunnel: w745 -> [w1130]
              tunnel: [w1130] -> w741
              tunnel: w744 -> [w1129]
              tunnel: [w1129] -> w740
              tunnel: w743 -> [w1128]
              tunnel: [w1128] -> w739
              tunnel: w742 -> [w1127]
              tunnel: [w1127] -> w738
              tunnel: [w1134] -> w737
              tunnel: [w1135] -> w736
              tunnel: [w1131] -> w735
              tunnel: w738 -> [w1131]
              tunnel: w739 -> [w1132]
              tunnel: w740 -> [w1136]
              tunnel: w741 -> [w1133]
              tunnel: w737 -> [w1147]
              tunnel: w736 -> [w1148]
              tunnel: w735 -> [w1150]
              tunnel: [w1146] -> w703
              tunnel: [w1145] -> w704
              frame #0 {
                n319 = property on="OP" class="Bool (strict)"() -> ("Value"=w1072:bool)  [unwired: 2 in, 2 out]
                n320 = case shown="False" w1072 {
                  tunnel: [2300000 w1101] -> w1069
                  tunnel: [FALSE ("Value (Signaling)") TRUE ("Value (Signaling)")] -> w1071
                  frame False {
                    n321 = property on="GVposition SP 15360000" class="DigNum (strict)" props=["Value"]() -> ()  [unwired: 2 in, 3 out]
                  }
                  frame True {
                    n322 = property on="Z Step SP" class="DigNum (strict)"() -> ("Maximum"=w1100:dbl)  [unwired: 2 in, 2 out]
                    n323 = To Long Integer(number=w1100) -> (32bit integer=w1101:i32)
                  }
                }
                n324 = property on="Z Step SP" class="DigNum (strict)"() -> ("Minimum"=w1085:dbl)  [unwired: 2 in, 2 out]
                n325 = property on="OK Button" class="Bool (strict)"() -> ("Value"=w1077:bool)  [unwired: 2 in, 2 out]
                n326 = property on="Z steps/rev" class="DigNum (strict)"() -> ("Value"=w1089:u32)  [unwired: 2 in, 2 out]
                n327 = To Double Precision Float(number=w1089) -> (double precision float=w1094:dbl)
                n328 = To Long Integer(number=w1085) -> (32bit integer=w1068:i32)
                n329 = property on="Z offset mm" class="DigNum (strict)"() -> ("Value"=w1087:dbl)  [unwired: 2 in, 2 out]
                n330 = Not Equal?(x=w1077, y=TRUE) -> (x != y?=w1075:bool)
                n331 = property on="V5 Valve \nopend/closed" class="Bool (strict)"("Val(Sgnl)"=w1071) -> ()  [unwired: 2 in, 2 out]
                n332 = call "mdrive send command.vi"("error in (no error)"=w1083, "Extra"="P", "Command"=T10."Print Parameter", "VISA resource name"=w1084) -> ("error out"=w1080:errorcluster, "read buffer"=w1096:string, "VISA resource name out"=w1081:refnum<visa-resource-name>)  [unwired: 3 in]
                n333 = Decimal String To Number(string=w1096, offset=0) -> (number=w1067:i32)  [unwired: 1 in, 1 out]
                n334 = property on="Z Step PV" class="DigNum (strict)"("Val(Sgnl)"=w1067) -> ()  [unwired: 2 in, 2 out]
                n335 = Equal?(x=w1067, y=15360000) -> (x = y?=w1074:bool)
                n336 = To Double Precision Float(number=w1067) -> (double precision float=w1092:dbl)
                n337 = In Range and Coerce(upper limit=w1067, x=w1069, lower limit=w1068) -> (In Range?=w1070:bool)  [unwired: 1 out]
                n338 = property on="Z in Range" class="Bool (strict)"("Val(Sgnl)"=w1070) -> ()  [unwired: 2 in, 2 out]
                n339 = Divide(x=w1092, y=w1094) -> (x/y=w1093:dbl)
                n340 = And(x=w1074, y=w1075) -> (x .and. y?=w1073:bool)
                n341 = case shown="True" w1073 {
                  tunnel: [FALSE ("true") w1109] -> w1078
                  frame False {
                  }
                  frame True {
                    n342 = One Button Dialog(message="HAVE YOU OPEND THE VALVE???\nTHEN REWRITE YOUR POSITION\n AND PRESS GO!") -> (true=w1109:bool)  [unwired: 1 in]
                  }
                }
                n343 = property on="Z mm/rev" class="DigNum (strict)"() -> ("Value"=w1088:dbl)  [unwired: 2 in, 2 out]
                n344 = Multiply(x=w1093, y=w1088) -> (x*y=w1082:dbl)
                n345 = Add(x=w1082, y=w1087) -> (x+y=w1086:dbl)
                n346 = property on="Z Position mm PV" class="DigNum (strict)"("Val(Sgnl)"=w1086) -> ()  [unwired: 2 in, 2 out]
                n347 = case shown="True" w1078 {
                  frame False {
                    n348 = call "DigitalIO_sub_V5_MON.vi"() -> ("CL"=w1102:bool, "OP"=w1103:bool)  [unwired: 8 in]
                    n349 = property on="OP" class="Bool (strict)"("Val(Sgnl)"=w1103) -> ()  [unwired: 2 in, 2 out]
                    n350 = property on="CL" class="Bool (strict)"("Val(Sgnl)"=w1102) -> ()  [unwired: 2 in, 2 out]
                  }
                  frame True {
                    n351 = while {
                      stop <- w1107 stop-if-true
                      n352 = call "DigitalIO_sub_V5_MON.vi"() -> ("CL"=w1104:bool, "OP"=w1105:bool)  [unwired: 8 in]
                      n353 = property on="OP" class="Bool (strict)"("Val(Sgnl)"=w1105) -> ()  [unwired: 2 in, 2 out]
                      n354 = property on="CL" class="Bool (strict)"("Val(Sgnl)"=w1104) -> ()  [unwired: 2 in, 2 out]
                      n355 = property on="V5 Valve \nopend/closed" class="Bool (strict)"("Val(Sgnl)"=w1104) -> ()  [unwired: 2 in, 2 out]
                      n356 = Equal?(x=w1104, y=TRUE) -> (x = y?=w1107:bool)
                    }
                  }
                }
              }
              frame #1 {
                n357 = call "mdrive send command.vi"("error in (no error)"=w1116, "Extra"="MV", "Command"=T10."Print Parameter", "VISA resource name"=w1117) -> ("error out"=w1119:errorcluster, "read buffer"=w1122:string, "VISA resource name out"=w1120:refnum<visa-resource-name>)  [unwired: 3 in]
                n358 = Decimal String To Number(string=w1122, offset=0 ("offset (0)")) -> (number=w1112:i32)  [unwired: 1 in, 1 out]
                n359 = Not Equal?(x=w1122, y="") -> (x != y?=w1115:bool)
                n360 = property on="Z Ready" class="Bool (strict)"("Val(Sgnl)"=w1115) -> ()  [unwired: 2 in, 2 out]
                n361 = Number To Boolean Array(number=w1112) -> (Boolean array=w1114:bool[])
                n362 = Index Array(array=w1114, index=0) -> (element=w1111:bool)
                n363 = property on="Z in Motion" class="Bool (strict)"("Val(Sgnl)"=w1111) -> ()  [unwired: 2 in, 2 out]
              }
              frame #2 {
                n364 = Wait (ms)(milliseconds to wait=u32 50) -> ()  [unwired: 1 out]
              }
              frame #3 {
                n365 = case shown="False" w1132 {
                  tunnel: w1133 -> [w1139 w1143]
                  tunnel: [w1140 w1143] -> w1134
                  tunnel: [w1141 w1142] -> w1135
                  tunnel: w1136 -> [w1138 w1142]
                  frame False {
                    n366 = call "mdrive send command.vi"("error in (no error)"=w1138, "Command"=T10."Stop", "VISA resource name"=w1139) -> ("error out"=w1141:errorcluster, "VISA resource name out"=w1140:refnum<visa-resource-name>)  [unwired: 4 in, 1 out]
                  }
                  frame True {
                  }
                }
              }
              frame #4 {
                n367 = property on="Z Backlash corr" class="Bool (strict)"() -> ("Value"=w1144:bool)  [unwired: 2 in, 2 out]
                n368 = Implies(1:w1150, 2:w1144) -> (0:w1149:bool)
                n369 = case shown="False" w1149 {
                  tunnel: w1148 -> [w1158 w1215]
                  tunnel: w1147 -> [w1157 w1216]
                  tunnel: [w1152 w1215] -> w1146
                  tunnel: [w1156 w1216] -> w1145
                  frame False {
                    # "Backlash"
                    n370 = flat-sequence {
                      tunnel: [w1171] -> w1170
                      tunnel: [w1175] -> w1169
                      tunnel: [w1174] -> w1168
                      tunnel: w1158 -> [w1173]
                      tunnel: w1157 -> [w1172]
                      tunnel: w1170 -> [w1183]
                      tunnel: [w1183] -> w1167
                      tunnel: w1169 -> [w1182]
                      tunnel: w1168 -> [w1181]
                      tunnel: [w1180] -> w1166
                      tunnel: [w1179] -> w1165
                      tunnel: [w1178] -> w1155
                      tunnel: w1167 -> [w1197]
                      tunnel: w1166 -> [w1188]
                      tunnel: w1165 -> [w1196]
                      tunnel: [w1188] -> w1164
                      tunnel: [w1196] -> w1163
                      tunnel: [w1187] -> w1160
                      tunnel: [w1195] -> w1159
                      tunnel: w1155 -> [w1195]
                      tunnel: w1164 -> [w1200]
                      tunnel: w1163 -> [w1201]
                      tunnel: [w1199] -> w1162
                      tunnel: [w1207] -> w1161
                      tunnel: w1160 -> [w1207]
                      tunnel: w1159 -> [w1203]
                      tunnel: [w1202] -> w1153
                      tunnel: w1162 -> [w1210]
                      tunnel: w1161 -> [w1209]
                      tunnel: [w1211] -> w1154
                      tunnel: w1153 -> [w1211]
                      tunnel: [w1210] -> w1151
                      tunnel: [w1214] -> w1156
                      tunnel: w1154 -> [w1214]
                      tunnel: [w1213] -> w1152
                      tunnel: w1151 -> [w1213]
                      frame #0 {
                        n371 = property on="Z Backlash steps/sec" class="DigNum (strict)"() -> ("Value"=w1171:i32)  [unwired: 2 in, 2 out]
                        n372 = Number To Decimal String(number=w1171) -> (decimal integer string=w1176:string)  [unwired: 1 in]
                        n373 = call "mdrive send command.vi"("error in (no error)"=w1173, "Extra"=w1176, "Command"=T10."Max Velocity", "VISA resource name"=w1172) -> ("error out"=w1174:errorcluster, "VISA resource name out"=w1175:refnum<visa-resource-name>)  [unwired: 3 in, 1 out]
                      }
                      frame #1 {
                        n374 = property on="Z Backlash" class="DigNum (strict)"() -> ("Value"=w1178:i32)  [unwired: 2 in, 2 out]
                        n375 = Number To Decimal String(number=w1178) -> (decimal integer string=w1184:string)  [unwired: 1 in]
                        n376 = call "mdrive send command.vi"("error in (no error)"=w1181, "Extra"=w1184, "Command"=T10."Move to Relative Position", "VISA resource name"=w1182) -> ("error out"=w1180:errorcluster, "VISA resource name out"=w1179:refnum<visa-resource-name>)  [unwired: 3 in, 1 out]
                      }
                      frame #2 {
                        n377 = To Double Precision Float(number=w1195) -> (double precision float=w1193:dbl)
                        n378 = To Double Precision Float(number=w1197) -> (double precision float=w1198:dbl)
                        n379 = Absolute Value(x=w1193) -> (abs(x)=w1194:dbl)
                        n380 = Divide(x=w1194, y=w1198) -> (x/y=w1191:dbl)
                        n381 = Multiply(x=1000.0, y=w1191) -> (x*y=w1189:dbl)
                        n382 = Add(x=w1189, y=300.0) -> (x+y=w1187:dbl)
                        n383 = To Unsigned Long Integer(number=w1187) -> (unsigned 32bit integer=w1186:u32)
                        n384 = Wait (ms)(milliseconds to wait=w1186) -> ()  [unwired: 1 out]
                      }
                      frame #3 {
                        n385 = Negate(x=w1203) -> (-x=w1204:i32)
                        n386 = Number To Decimal String(number=w1204) -> (decimal integer string=w1205:string)  [unwired: 1 in]
                        n387 = call "mdrive send command.vi"("error in (no error)"=w1200, "Extra"=w1205, "Command"=T10."Move to Relative Position", "VISA resource name"=w1201) -> ("error out"=w1199:errorcluster, "VISA resource name out"=w1202:refnum<visa-resource-name>)  [unwired: 3 in, 1 out]
                      }
                      frame #4 {
                        n388 = To Unsigned Long Integer(number=w1209) -> (unsigned 32bit integer=w1208:u32)
                        n389 = Wait (ms)(milliseconds to wait=w1208) -> ()  [unwired: 1 out]
                      }
                      frame #5 {
                        n390 = property on="Z Backlash corr" class="Bool (strict)"("Val(Sgnl)"=FALSE ("Value (Signaling)")) -> ()  [unwired: 2 in, 2 out]
                      }
                    }
                  }
                  frame True {
                  }
                }
              }
            }
            n391 = property on="Scan Go" class="Bool (strict)"() -> ("Value"=w690:bool)  [unwired: 2 in, 2 out]
            n392 = flat-sequence {
              tunnel: [w1222] -> w762
              tunnel: [w1221] -> w761
              tunnel: [w1220] -> w760
              tunnel: w698 -> [w1219]
              tunnel: w697 -> [w1218]
              tunnel: [w1244] -> w759
              tunnel: [w1243] -> w758
              tunnel: [w1241] -> w757
              tunnel: [w1242] -> w756
              tunnel: w762 -> [w1241]
              tunnel: w761 -> [w1240]
              tunnel: w760 -> [w1239]
              tunnel: w759 -> [w1258]
              tunnel: [w1258] -> w755
              tunnel: w758 -> [w1257]
              tunnel: [w1257] -> w754
              tunnel: w757 -> [w1256]
              tunnel: [w1256] -> w753
              tunnel: w756 -> [w1255]
              tunnel: [w1255] -> w752
              tunnel: [w1262] -> w751
              tunnel: [w1263] -> w750
              tunnel: [w1259] -> w749
              tunnel: w752 -> [w1259]
              tunnel: w753 -> [w1260]
              tunnel: w754 -> [w1264]
              tunnel: w755 -> [w1261]
              tunnel: w751 -> [w1274]
              tunnel: w750 -> [w1275]
              tunnel: w749 -> [w1277]
              tunnel: [w1273] -> w705
              tunnel: [w1272] -> w706
              frame #0 {
                n393 = property on="X Step SP" class="DigNum (strict)"() -> ("Maximum"=w1234:dbl)  [unwired: 2 in, 2 out]
                n394 = property on="X Step SP" class="DigNum (strict)"() -> ("Minimum"=w1236:dbl)  [unwired: 2 in, 2 out]
                n395 = property on="X steps/rev" class="DigNum (strict)"() -> ("Value"=w1231:u32)  [unwired: 2 in, 2 out]
                n396 = property on="X offset mm" class="DigNum (strict)"() -> ("Value"=w1227:dbl)  [unwired: 2 in, 2 out]
                n397 = To Long Integer(number=w1234) -> (32bit integer=w1233:i32)
                n398 = To Long Integer(number=w1236) -> (32bit integer=w1235:i32)
                n399 = To Double Precision Float(number=w1231) -> (double precision float=w1232:dbl)
                n400 = call "mdrive send command.vi"("error in (no error)"=w1218, "Extra"="P", "Command"=T10."Print Parameter", "VISA resource name"=w1219) -> ("error out"=w1220:errorcluster, "read buffer"=w1238:string, "VISA resource name out"=w1221:refnum<visa-resource-name>)  [unwired: 3 in]
                n401 = Decimal String To Number(string=w1238, offset=0) -> (number=w1217:i32)  [unwired: 1 in, 1 out]
                n402 = property on="X Step PV" class="DigNum (strict)"("Val(Sgnl)"=w1217) -> ()  [unwired: 2 in, 2 out]
                n403 = In Range and Coerce(upper limit=w1233, x=w1217, lower limit=w1235) -> (In Range?=w1222:bool)  [unwired: 1 out]
                n404 = To Double Precision Float(number=w1217) -> (double precision float=w1226:dbl)
                n405 = property on="X  in Range" class="Bool (strict)"("Val(Sgnl)"=w1222) -> ()  [unwired: 2 in, 2 out]
                n406 = Divide(x=w1226, y=w1232) -> (x/y=w1230:dbl)
                n407 = property on="X mm/rev" class="DigNum (strict)"() -> ("Value"=w1229:dbl)  [unwired: 2 in, 2 out]
                n408 = Multiply(x=w1230, y=w1229) -> (x*y=w1228:dbl)
                n409 = Add(x=w1228, y=w1227) -> (x+y=w1225:dbl)
                n410 = property on="X Position mm PV" class="DigNum (strict)"("Val(Sgnl)"=w1225) -> ()  [unwired: 2 in, 2 out]
              }
              frame #1 {
                n411 = call "mdrive send command.vi"("error in (no error)"=w1239, "Extra"="MV", "Command"=T10."Print Parameter", "VISA resource name"=w1240) -> ("error out"=w1243:errorcluster, "read buffer"=w1247:string, "VISA resource name out"=w1244:refnum<visa-resource-name>)  [unwired: 3 in]
                n412 = Decimal String To Number(string=w1247, offset=0 ("offset (0)")) -> (number=w1250:i32)  [unwired: 1 in, 1 out]
                n413 = Not Equal?(x=w1247, y="") -> (x != y?=w1245:bool)
                n414 = property on="X Ready" class="Bool (strict)"("Val(Sgnl)"=w1245) -> ()  [unwired: 2 in, 2 out]
                n415 = Number To Boolean Array(number=w1250) -> (Boolean array=w1249:bool[])
                n416 = Index Array(array=w1249, index=0) -> (element=w1242:bool)
                n417 = property on="X  in Motion" class="Bool (strict)"("Val(Sgnl)"=w1242) -> ()  [unwired: 2 in, 2 out]
              }
              frame #2 {
                n418 = Wait (ms)(milliseconds to wait=u32 50) -> ()  [unwired: 1 out]
              }
              frame #3 {
                n419 = case shown="True" w1260 {
                  tunnel: w1261 -> [w1267 w1271]
                  tunnel: [w1268 w1271] -> w1262
                  tunnel: [w1269 w1270] -> w1263
                  tunnel: w1264 -> [w1266 w1270]
                  frame False {
                    n420 = call "mdrive send command.vi"("error in (no error)"=w1266, "Command"=T10."Stop", "VISA resource name"=w1267) -> ("error out"=w1269:errorcluster, "VISA resource name out"=w1268:refnum<visa-resource-name>)  [unwired: 4 in, 1 out]
                  }
                  frame True {
                  }
                }
              }
              frame #4 {
                n421 = property on="X Backlash corr" class="Bool (strict)"() -> ("Value"=w1278:bool)  [unwired: 2 in, 2 out]
                n422 = Implies(1:w1277, 2:w1278) -> (0:w1276:bool)
                n423 = case shown="False" w1276 {
                  tunnel: w1275 -> [w1286 w1343]
                  tunnel: w1274 -> [w1285 w1344]
                  tunnel: [w1280 w1343] -> w1273
                  tunnel: [w1284 w1344] -> w1272
                  frame False {
                    # "Backlash"
                    n424 = flat-sequence {
                      tunnel: [w1301] -> w1298
                      tunnel: [w1303] -> w1297
                      tunnel: [w1302] -> w1296
                      tunnel: w1286 -> [w1300]
                      tunnel: w1285 -> [w1299]
                      tunnel: w1298 -> [w1311]
                      tunnel: [w1311] -> w1295
                      tunnel: w1297 -> [w1310]
                      tunnel: w1296 -> [w1309]
                      tunnel: [w1308] -> w1294
                      tunnel: [w1307] -> w1293
                      tunnel: [w1306] -> w1283
                      tunnel: w1295 -> [w1325]
                      tunnel: w1294 -> [w1316]
                      tunnel: w1293 -> [w1324]
                      tunnel: [w1316] -> w1292
                      tunnel: [w1324] -> w1291
                      tunnel: [w1315] -> w1288
                      tunnel: [w1323] -> w1287
                      tunnel: w1283 -> [w1323]
                      tunnel: w1292 -> [w1328]
                      tunnel: w1291 -> [w1329]
                      tunnel: [w1327] -> w1290
                      tunnel: [w1335] -> w1289
                      tunnel: w1288 -> [w1335]
                      tunnel: w1287 -> [w1331]
                      tunnel: [w1330] -> w1281
                      tunnel: w1290 -> [w1338]
                      tunnel: w1289 -> [w1337]
                      tunnel: [w1339] -> w1282
                      tunnel: w1281 -> [w1339]
                      tunnel: [w1338] -> w1279
                      tunnel: [w1342] -> w1284
                      tunnel: w1282 -> [w1342]
                      tunnel: [w1340] -> w1280
                      tunnel: w1279 -> [w1340]
                      frame #0 {
                        n425 = property on="X Backlash steps/sec" class="DigNum (strict)"() -> ("Value"=w1301:i32)  [unwired: 2 in, 2 out]
                        n426 = Number To Decimal String(number=w1301) -> (decimal integer string=w1304:string)  [unwired: 1 in]
                        n427 = call "mdrive send command.vi"("error in (no error)"=w1300, "Extra"=w1304, "Command"=T10."Max Velocity", "VISA resource name"=w1299) -> ("error out"=w1302:errorcluster, "VISA resource name out"=w1303:refnum<visa-resource-name>)  [unwired: 3 in, 1 out]
                      }
                      frame #1 {
                        n428 = property on="X Backlash" class="DigNum (strict)"() -> ("Value"=w1306:i32)  [unwired: 2 in, 2 out]
                        n429 = Number To Decimal String(number=w1306) -> (decimal integer string=w1312:string)  [unwired: 1 in]
                        n430 = call "mdrive send command.vi"("error in (no error)"=w1309, "Extra"=w1312, "Command"=T10."Move to Relative Position", "VISA resource name"=w1310) -> ("error out"=w1308:errorcluster, "VISA resource name out"=w1307:refnum<visa-resource-name>)  [unwired: 3 in, 1 out]
                      }
                      frame #2 {
                        n431 = To Double Precision Float(number=w1323) -> (double precision float=w1321:dbl)
                        n432 = To Double Precision Float(number=w1325) -> (double precision float=w1326:dbl)
                        n433 = Absolute Value(x=w1321) -> (abs(x)=w1322:dbl)
                        n434 = Divide(x=w1322, y=w1326) -> (x/y=w1319:dbl)
                        n435 = Multiply(x=1000.0, y=w1319) -> (x*y=w1317:dbl)
                        n436 = Add(x=w1317, y=300.0) -> (x+y=w1315:dbl)
                        n437 = To Unsigned Long Integer(number=w1315) -> (unsigned 32bit integer=w1314:u32)
                        n438 = Wait (ms)(milliseconds to wait=w1314) -> ()  [unwired: 1 out]
                      }
                      frame #3 {
                        n439 = Negate(x=w1331) -> (-x=w1332:i32)
                        n440 = Number To Decimal String(number=w1332) -> (decimal integer string=w1333:string)  [unwired: 1 in]
                        n441 = call "mdrive send command.vi"("error in (no error)"=w1328, "Extra"=w1333, "Command"=T10."Move to Relative Position", "VISA resource name"=w1329) -> ("error out"=w1327:errorcluster, "VISA resource name out"=w1330:refnum<visa-resource-name>)  [unwired: 3 in, 1 out]
                      }
                      frame #4 {
                        n442 = To Unsigned Long Integer(number=w1337) -> (unsigned 32bit integer=w1336:u32)
                        n443 = Wait (ms)(milliseconds to wait=w1336) -> ()  [unwired: 1 out]
                      }
                      frame #5 {
                        n444 = property on="X Backlash corr" class="Bool (strict)"("Val(Sgnl)"=FALSE ("Value (Signaling)")) -> ()  [unwired: 2 in, 2 out]
                      }
                    }
                  }
                  frame True {
                  }
                }
              }
            }
            n445 = flat-sequence {
              tunnel: [w948] -> w734
              tunnel: [w950] -> w733
              tunnel: [w949] -> w732
              tunnel: w694 -> [w941]
              tunnel: w693 -> [w940]
              tunnel: [w970] -> w731
              tunnel: [w969] -> w730
              tunnel: [w968] -> w729
              tunnel: [w961] -> w728
              tunnel: w734 -> [w968]
              tunnel: w733 -> [w967]
              tunnel: w732 -> [w966]
              tunnel: w731 -> [w980]
              tunnel: [w980] -> w727
              tunnel: w730 -> [w979]
              tunnel: [w979] -> w726
              tunnel: w729 -> [w978]
              tunnel: [w978] -> w725
              tunnel: w728 -> [w977]
              tunnel: [w977] -> w724
              tunnel: [w984] -> w723
              tunnel: [w985] -> w722
              tunnel: [w981] -> w721
              tunnel: w724 -> [w981]
              tunnel: w725 -> [w982]
              tunnel: w726 -> [w986]
              tunnel: w727 -> [w983]
              tunnel: w723 -> [w997]
              tunnel: w722 -> [w998]
              tunnel: w721 -> [w1000]
              tunnel: [w996] -> w701
              tunnel: [w995] -> w702
              frame #0 {
                n446 = property on="Y Step SP" class="DigNum (strict)"() -> ("Maximum"=w943:dbl)  [unwired: 2 in, 2 out]
                n447 = property on="Y Step SP" class="DigNum (strict)"() -> ("Minimum"=w942:dbl)  [unwired: 2 in, 2 out]
                n448 = property on="Y steps/rev" class="DigNum (strict)"() -> ("Value"=w944:u32)  [unwired: 2 in, 2 out]
                n449 = property on="Y offset mm" class="DigNum (strict)"() -> ("Value"=w946:dbl)  [unwired: 2 in, 2 out]
                n450 = To Long Integer(number=w943) -> (32bit integer=w957:i32)
                n451 = To Long Integer(number=w942) -> (32bit integer=w958:i32)
                n452 = To Double Precision Float(number=w944) -> (double precision float=w956:dbl)
                n453 = call "mdrive send command.vi"("error in (no error)"=w940, "Extra"="P", "Command"=T10."Print Parameter", "VISA resource name"=w941) -> ("error out"=w949:errorcluster, "read buffer"=w960:string, "VISA resource name out"=w950:refnum<visa-resource-name>)  [unwired: 3 in]
                n454 = Decimal String To Number(string=w960, offset=0) -> (number=w939:i32)  [unwired: 1 in, 1 out]
                n455 = property on="Y Step PV" class="DigNum (strict)"("Val(Sgnl)"=w939) -> ()  [unwired: 2 in, 2 out]
                n456 = In Range and Coerce(upper limit=w957, x=w939, lower limit=w958) -> (In Range?=w948:bool)  [unwired: 1 out]
                n457 = To Double Precision Float(number=w939) -> (double precision float=w953:dbl)
                n458 = property on="Y in Range" class="Bool (strict)"("Val(Sgnl)"=w948) -> ()  [unwired: 2 in, 2 out]
                n459 = Divide(x=w953, y=w956) -> (x/y=w955:dbl)
                n460 = property on="Y mm/rev" class="DigNum (strict)"() -> ("Value"=w945:dbl)  [unwired: 2 in, 2 out]
                n461 = Multiply(x=w955, y=w945) -> (x*y=w954:dbl)
                n462 = Add(x=w954, y=w946) -> (x+y=w947:dbl)
                n463 = property on="Y Position mm PV" class="DigNum (strict)"("Val(Sgnl)"=w947) -> ()  [unwired: 2 in, 2 out]
              }
              frame #1 {
                n464 = call "mdrive send command.vi"("error in (no error)"=w966, "Extra"="MV", "Command"=T10."Print Parameter", "VISA resource name"=w967) -> ("error out"=w969:errorcluster, "read buffer"=w972:string, "VISA resource name out"=w970:refnum<visa-resource-name>)  [unwired: 3 in]
                n465 = Decimal String To Number(string=w972, offset=0 ("offset (0)")) -> (number=w962:i32)  [unwired: 1 in, 1 out]
                n466 = Not Equal?(x=w972, y="") -> (x != y?=w965:bool)
                n467 = property on="Y Ready" class="Bool (strict)"("Val(Sgnl)"=w965) -> ()  [unwired: 2 in, 2 out]
                n468 = Number To Boolean Array(number=w962) -> (Boolean array=w964:bool[])
                n469 = Index Array(array=w964, index=0) -> (element=w961:bool)
                n470 = property on="Y in Motion" class="Bool (strict)"("Val(Sgnl)"=w961) -> ()  [unwired: 2 in, 2 out]
              }
              frame #2 {
                n471 = Wait (ms)(milliseconds to wait=u32 50) -> ()  [unwired: 1 out]
              }
              frame #3 {
                n472 = case shown="True" w982 {
                  tunnel: w983 -> [w989 w992]
                  tunnel: [w990 w992] -> w984
                  tunnel: [w991 w993] -> w985
                  tunnel: w986 -> [w988 w993]
                  frame False {
                    n473 = call "mdrive send command.vi"("error in (no error)"=w988, "Command"=T10."Stop", "VISA resource name"=w989) -> ("error out"=w991:errorcluster, "VISA resource name out"=w990:refnum<visa-resource-name>)  [unwired: 4 in, 1 out]
                  }
                  frame True {
                  }
                }
              }
              frame #4 {
                n474 = property on="Y Backlash corr" class="Bool (strict)"() -> ("Value"=w994:bool)  [unwired: 2 in, 2 out]
                n475 = Implies(1:w1000, 2:w994) -> (0:w999:bool)
                n476 = case shown="False" w999 {
                  tunnel: w998 -> [w1008 w1065]
                  tunnel: w997 -> [w1007 w1066]
                  tunnel: [w1002 w1065] -> w996
                  tunnel: [w1006 w1066] -> w995
                  frame False {
                    # "Backlash"
                    n477 = flat-sequence {
                      tunnel: [w1021] -> w1020
                      tunnel: [w1025] -> w1019
                      tunnel: [w1024] -> w1018
                      tunnel: w1008 -> [w1023]
                      tunnel: w1007 -> [w1022]
                      tunnel: w1020 -> [w1033]
                      tunnel: [w1033] -> w1017
                      tunnel: w1019 -> [w1032]
                      tunnel: w1018 -> [w1031]
                      tunnel: [w1030] -> w1016
                      tunnel: [w1029] -> w1015
                      tunnel: [w1028] -> w1005
                      tunnel: w1017 -> [w1047]
                      tunnel: w1016 -> [w1038]
                      tunnel: w1015 -> [w1046]
                      tunnel: [w1038] -> w1014
                      tunnel: [w1046] -> w1013
                      tunnel: [w1037] -> w1010
                      tunnel: [w1045] -> w1009
                      tunnel: w1005 -> [w1045]
                      tunnel: w1014 -> [w1050]
                      tunnel: w1013 -> [w1051]
                      tunnel: [w1049] -> w1012
                      tunnel: [w1057] -> w1011
                      tunnel: w1010 -> [w1057]
                      tunnel: w1009 -> [w1053]
                      tunnel: [w1052] -> w1003
                      tunnel: w1012 -> [w1060]
                      tunnel: w1011 -> [w1059]
                      tunnel: [w1061] -> w1004
                      tunnel: w1003 -> [w1061]
                      tunnel: [w1060] -> w1001
                      tunnel: [w1064] -> w1006
                      tunnel: w1004 -> [w1064]
                      tunnel: [w1063] -> w1002
                      tunnel: w1001 -> [w1063]
                      frame #0 {
                        n478 = property on="Y Backlash steps/sec" class="DigNum (strict)"() -> ("Value"=w1021:i32)  [unwired: 2 in, 2 out]
                        n479 = Number To Decimal String(number=w1021) -> (decimal integer string=w1026:string)  [unwired: 1 in]
                        n480 = call "mdrive send command.vi"("error in (no error)"=w1023, "Extra"=w1026, "Command"=T10."Max Velocity", "VISA resource name"=w1022) -> ("error out"=w1024:errorcluster, "VISA resource name out"=w1025:refnum<visa-resource-name>)  [unwired: 3 in, 1 out]
                      }
                      frame #1 {
                        n481 = property on="Y Backlash" class="DigNum (strict)"() -> ("Value"=w1028:i32)  [unwired: 2 in, 2 out]
                        n482 = Number To Decimal String(number=w1028) -> (decimal integer string=w1034:string)  [unwired: 1 in]
                        n483 = call "mdrive send command.vi"("error in (no error)"=w1031, "Extra"=w1034, "Command"=T10."Move to Relative Position", "VISA resource name"=w1032) -> ("error out"=w1030:errorcluster, "VISA resource name out"=w1029:refnum<visa-resource-name>)  [unwired: 3 in, 1 out]
                      }
                      frame #2 {
                        n484 = To Double Precision Float(number=w1045) -> (double precision float=w1043:dbl)
                        n485 = To Double Precision Float(number=w1047) -> (double precision float=w1048:dbl)
                        n486 = Absolute Value(x=w1043) -> (abs(x)=w1044:dbl)
                        n487 = Divide(x=w1044, y=w1048) -> (x/y=w1041:dbl)
                        n488 = Multiply(x=1000.0, y=w1041) -> (x*y=w1039:dbl)
                        n489 = Add(x=w1039, y=300.0) -> (x+y=w1037:dbl)
                        n490 = To Unsigned Long Integer(number=w1037) -> (unsigned 32bit integer=w1036:u32)
                        n491 = Wait (ms)(milliseconds to wait=w1036) -> ()  [unwired: 1 out]
                      }
                      frame #3 {
                        n492 = Negate(x=w1053) -> (-x=w1054:i32)
                        n493 = Number To Decimal String(number=w1054) -> (decimal integer string=w1055:string)  [unwired: 1 in]
                        n494 = call "mdrive send command.vi"("error in (no error)"=w1050, "Extra"=w1055, "Command"=T10."Move to Relative Position", "VISA resource name"=w1051) -> ("error out"=w1049:errorcluster, "VISA resource name out"=w1052:refnum<visa-resource-name>)  [unwired: 3 in, 1 out]
                      }
                      frame #4 {
                        n495 = To Unsigned Long Integer(number=w1059) -> (unsigned 32bit integer=w1058:u32)
                        n496 = Wait (ms)(milliseconds to wait=w1058) -> ()  [unwired: 1 out]
                      }
                      frame #5 {
                        n497 = property on="Y Backlash corr" class="Bool (strict)"("Val(Sgnl)"=FALSE ("Value (Signaling)")) -> ()  [unwired: 2 in, 2 out]
                      }
                    }
                  }
                  frame True {
                  }
                }
              }
            }
            n498 = flat-sequence {
              tunnel: [w820] -> w720
              tunnel: [w822] -> w719
              tunnel: [w821] -> w718
              tunnel: w692 -> [w813]
              tunnel: w691 -> [w812]
              tunnel: [w842] -> w717
              tunnel: [w841] -> w716
              tunnel: [w840] -> w715
              tunnel: [w833] -> w714
              tunnel: w720 -> [w840]
              tunnel: w719 -> [w839]
              tunnel: w718 -> [w838]
              tunnel: w717 -> [w852]
              tunnel: [w852] -> w713
              tunnel: w716 -> [w851]
              tunnel: [w851] -> w712
              tunnel: w715 -> [w850]
              tunnel: [w850] -> w711
              tunnel: w714 -> [w849]
              tunnel: [w849] -> w710
              tunnel: [w856] -> w709
              tunnel: [w857] -> w708
              tunnel: [w853] -> w707
              tunnel: w710 -> [w853]
              tunnel: w711 -> [w854]
              tunnel: w712 -> [w858]
              tunnel: w713 -> [w855]
              tunnel: w709 -> [w869]
              tunnel: w708 -> [w870]
              tunnel: w707 -> [w872]
              tunnel: [w868] -> w699
              tunnel: [w867] -> w700
              frame #0 {
                n499 = property on="R Step SP" class="DigNum (strict)"() -> ("Maximum"=w815:dbl)  [unwired: 2 in, 2 out]
                n500 = property on="R Step SP" class="DigNum (strict)"() -> ("Minimum"=w816:dbl)  [unwired: 2 in, 2 out]
                n501 = property on="R steps/rev" class="DigNum (strict)"() -> ("Value"=w814:u32)  [unwired: 2 in, 2 out]
                n502 = property on="R offset deg" class="DigNum (strict)"() -> ("Value"=w818:dbl)  [unwired: 2 in, 2 out]
                n503 = To Long Integer(number=w815) -> (32bit integer=w829:i32)
                n504 = To Long Integer(number=w816) -> (32bit integer=w830:i32)
                n505 = To Double Precision Float(number=w814) -> (double precision float=w828:dbl)
                n506 = call "mdrive send command.vi"("error in (no error)"=w812, "Extra"="P", "Command"=T10."Print Parameter", "VISA resource name"=w813) -> ("error out"=w821:errorcluster, "read buffer"=w832:string, "VISA resource name out"=w822:refnum<visa-resource-name>)  [unwired: 3 in]
                n507 = Decimal String To Number(string=w832, offset=0) -> (number=w811:i32)  [unwired: 1 in, 1 out]
                n508 = property on="R Step PV" class="DigNum (strict)"("Val(Sgnl)"=w811) -> ()  [unwired: 2 in, 2 out]
                n509 = In Range and Coerce(upper limit=w829, x=w811, lower limit=w830) -> (In Range?=w820:bool)  [unwired: 1 out]
                n510 = To Double Precision Float(number=w811) -> (double precision float=w825:dbl)
                n511 = property on="R in Range" class="Bool (strict)"("Val(Sgnl)"=w820) -> ()  [unwired: 2 in, 2 out]
                n512 = Divide(x=w825, y=w828) -> (x/y=w827:dbl)
                n513 = property on="R deg/rev" class="DigNum (strict)"() -> ("Value"=w817:dbl)  [unwired: 2 in, 2 out]
                n514 = Multiply(x=w827, y=w817) -> (x*y=w826:dbl)
                n515 = Add(x=w826, y=w818) -> (x+y=w819:dbl)
                n516 = property on="R Position deg PV" class="DigNum (strict)"("Val(Sgnl)"=w819) -> ()  [unwired: 2 in, 2 out]
              }
              frame #1 {
                n517 = call "mdrive send command.vi"("error in (no error)"=w838, "Extra"="MV", "Command"=T10."Print Parameter", "VISA resource name"=w839) -> ("error out"=w841:errorcluster, "read buffer"=w844:string, "VISA resource name out"=w842:refnum<visa-resource-name>)  [unwired: 3 in]
                n518 = Decimal String To Number(string=w844, offset=0 ("offset (0)")) -> (number=w834:i32)  [unwired: 1 in, 1 out]
                n519 = Not Equal?(x=w844, y="") -> (x != y?=w837:bool)
                n520 = property on="R Ready" class="Bool (strict)"("Val(Sgnl)"=w837) -> ()  [unwired: 2 in, 2 out]
                n521 = Number To Boolean Array(number=w834) -> (Boolean array=w836:bool[])
                n522 = Index Array(array=w836, index=0) -> (element=w833:bool)
                n523 = property on="R in Motion" class="Bool (strict)"("Val(Sgnl)"=w833) -> ()  [unwired: 2 in, 2 out]
              }
              frame #2 {
                n524 = Wait (ms)(milliseconds to wait=u32 50) -> ()  [unwired: 1 out]
              }
              frame #3 {
                n525 = case shown="True" w854 {
                  tunnel: w855 -> [w861 w865]
                  tunnel: [w862 w865] -> w856
                  tunnel: [w863 w864] -> w857
                  tunnel: w858 -> [w860 w864]
                  frame False {
                    n526 = call "mdrive send command.vi"("error in (no error)"=w860, "Command"=T10."Stop", "VISA resource name"=w861) -> ("error out"=w863:errorcluster, "VISA resource name out"=w862:refnum<visa-resource-name>)  [unwired: 4 in, 1 out]
                  }
                  frame True {
                  }
                }
              }
              frame #4 {
                n527 = property on="R Backlash corr" class="Bool (strict)"() -> ("Value"=w866:bool)  [unwired: 2 in, 2 out]
                n528 = Implies(1:w872, 2:w866) -> (0:w871:bool)
                n529 = case shown="False" w871 {
                  tunnel: w870 -> [w880 w937]
                  tunnel: w869 -> [w879 w938]
                  tunnel: [w874 w937] -> w868
                  tunnel: [w878 w938] -> w867
                  frame False {
                    # "Backlash"
                    n530 = flat-sequence {
                      tunnel: [w893] -> w892
                      tunnel: [w897] -> w891
                      tunnel: [w896] -> w890
                      tunnel: w880 -> [w895]
                      tunnel: w879 -> [w894]
                      tunnel: w892 -> [w905]
                      tunnel: [w905] -> w889
                      tunnel: w891 -> [w904]
                      tunnel: w890 -> [w903]
                      tunnel: [w902] -> w888
                      tunnel: [w901] -> w887
                      tunnel: [w900] -> w877
                      tunnel: w889 -> [w919]
                      tunnel: w888 -> [w910]
                      tunnel: w887 -> [w918]
                      tunnel: [w910] -> w886
                      tunnel: [w918] -> w885
                      tunnel: [w909] -> w882
                      tunnel: [w917] -> w881
                      tunnel: w877 -> [w917]
                      tunnel: w886 -> [w922]
                      tunnel: w885 -> [w923]
                      tunnel: [w921] -> w884
                      tunnel: [w929] -> w883
                      tunnel: w882 -> [w929]
                      tunnel: w881 -> [w925]
                      tunnel: [w924] -> w875
                      tunnel: w884 -> [w932]
                      tunnel: w883 -> [w931]
                      tunnel: [w933] -> w876
                      tunnel: w875 -> [w933]
                      tunnel: [w932] -> w873
                      tunnel: [w936] -> w878
                      tunnel: w876 -> [w936]
                      tunnel: [w935] -> w874
                      tunnel: w873 -> [w935]
                      frame #0 {
                        n531 = property on="R Backlash steps/sec" class="DigNum (strict)"() -> ("Value"=w893:i32)  [unwired: 2 in, 2 out]
                        n532 = Number To Decimal String(number=w893) -> (decimal integer string=w898:string)  [unwired: 1 in]
                        n533 = call "mdrive send command.vi"("error in (no error)"=w895, "Extra"=w898, "Command"=T10."Max Velocity", "VISA resource name"=w894) -> ("error out"=w896:errorcluster, "VISA resource name out"=w897:refnum<visa-resource-name>)  [unwired: 3 in, 1 out]
                      }
                      frame #1 {
                        n534 = property on="R Backlash" class="DigNum (strict)"() -> ("Value"=w900:i32)  [unwired: 2 in, 2 out]
                        n535 = Number To Decimal String(number=w900) -> (decimal integer string=w906:string)  [unwired: 1 in]
                        n536 = call "mdrive send command.vi"("error in (no error)"=w903, "Extra"=w906, "Command"=T10."Move to Relative Position", "VISA resource name"=w904) -> ("error out"=w902:errorcluster, "VISA resource name out"=w901:refnum<visa-resource-name>)  [unwired: 3 in, 1 out]
                      }
                      frame #2 {
                        n537 = To Double Precision Float(number=w917) -> (double precision float=w915:dbl)
                        n538 = To Double Precision Float(number=w919) -> (double precision float=w920:dbl)
                        n539 = Absolute Value(x=w915) -> (abs(x)=w916:dbl)
                        n540 = Divide(x=w916, y=w920) -> (x/y=w913:dbl)
                        n541 = Multiply(x=1000.0, y=w913) -> (x*y=w911:dbl)
                        n542 = Add(x=w911, y=300.0) -> (x+y=w909:dbl)
                        n543 = To Unsigned Long Integer(number=w909) -> (unsigned 32bit integer=w908:u32)
                        n544 = Wait (ms)(milliseconds to wait=w908) -> ()  [unwired: 1 out]
                      }
                      frame #3 {
                        n545 = Negate(x=w925) -> (-x=w926:i32)
                        n546 = Number To Decimal String(number=w926) -> (decimal integer string=w927:string)  [unwired: 1 in]
                        n547 = call "mdrive send command.vi"("error in (no error)"=w922, "Extra"=w927, "Command"=T10."Move to Relative Position", "VISA resource name"=w923) -> ("error out"=w921:errorcluster, "VISA resource name out"=w924:refnum<visa-resource-name>)  [unwired: 3 in, 1 out]
                      }
                      frame #4 {
                        n548 = To Unsigned Long Integer(number=w931) -> (unsigned 32bit integer=w930:u32)
                        n549 = Wait (ms)(milliseconds to wait=w930) -> ()  [unwired: 1 out]
                      }
                      frame #5 {
                        n550 = property on="R Backlash corr" class="Bool (strict)"("Val(Sgnl)"=FALSE ("Value (Signaling)")) -> ()  [unwired: 2 in, 2 out]
                      }
                    }
                  }
                  frame True {
                  }
                }
              }
            }
            n551 = Equal?(x=w690, y=TRUE) -> (x = y?=w685:bool)
            n552 = property on="STATUS" class="Str"() -> ("Value"=w688:string)  [unwired: 2 in, 2 out]
            n553 = Equal?(x=w688, y="SCANNING MODE" ("STATUS")) -> (x = y?=w686:bool)
            n554 = Or(x=w686, y=w685) -> (x .or. y?=w684:bool)
            n555 = case shown="False" w684 {
              frame False {
                n556 = property on="Y in Motion" class="Bool (strict)"() -> ("Value"=w766:bool)  [unwired: 2 in, 2 out]
                n557 = property on="Z in Motion" class="Bool (strict)"() -> ("Value"=w769:bool)  [unwired: 2 in, 2 out]
                n558 = property on="X  in Motion" class="Bool (strict)"() -> ("Value"=w767:bool)  [unwired: 2 in, 2 out]
                n559 = property on="R in Motion" class="Bool (strict)"() -> ("Value"=w768:bool)  [unwired: 2 in, 2 out]
                n560 = Compound Arithmetic op=AND(w767, w766, w769, w768) -> (w764:bool)
                n561 = Equal?(x=w764, y=FALSE) -> (x = y?=w765:bool)
                n562 = case shown="True" w765 {
                  frame False {
                  }
                  frame True {
                    n563 = property on="X Step SP" class="DigNum (strict)"() -> ("Value"=w777:i32)  [unwired: 2 in, 2 out]
                    n564 = property on="X Step PV" class="DigNum (strict)"() -> ("Value"=w776:i32)  [unwired: 2 in, 2 out]
                    n565 = property on="Y Step SP" class="DigNum (strict)"() -> ("Value"=w775:i32)  [unwired: 2 in, 2 out]
                    n566 = property on="Y Step PV" class="DigNum (strict)"() -> ("Value"=w774:i32)  [unwired: 2 in, 2 out]
                    n567 = property on="Z Step SP" class="DigNum (strict)"() -> ("Value"=w773:i32)  [unwired: 2 in, 2 out]
                    n568 = property on="Z Step PV" class="DigNum (strict)"() -> ("Value"=w772:i32)  [unwired: 2 in, 2 out]
                    n569 = property on="R Step SP" class="DigNum (strict)"() -> ("Value"=w770:i32)  [unwired: 2 in, 2 out]
                    n570 = property on="R Step PV" class="DigNum (strict)"() -> ("Value"=w771:i32)  [unwired: 2 in, 2 out]
                    n571 = Equal?(x=w777, y=w776) -> (x = y?=w782:bool)
                    n572 = Equal?(x=w775, y=w774) -> (x = y?=w781:bool)
                    n573 = Equal?(x=w773, y=w772) -> (x = y?=w779:bool)
                    n574 = Equal?(x=w770, y=w771) -> (x = y?=w780:bool)
                    n575 = Compound Arithmetic op=AND(w782, w781, w779, w780) -> (w778:bool)
                    n576 = case shown="True" w778 {
                      frame False {
                      }
                      frame True {
                        n577 = property on="GO" class="Bool"("DisabledEnum"=T9."Enabled" ("Disabled")) -> ()  [unwired: 2 in, 2 out]
                        n578 = local write "STATUS"("SCANNING DONE" ("STATUS")) -> ()
                      }
                    }
                  }
                }
              }
              frame True {
                n579 = property on="X Scan Length SP steps" class="DigNum (strict)"() -> ("Value"=w796:i32)  [unwired: 2 in, 2 out]
                n580 = property on="Y Scan Length SP steps" class="DigNum (strict)"() -> ("Value"=w795:i32)  [unwired: 2 in, 2 out]
                n581 = property on="Z Scan Length SP steps" class="DigNum (strict)"() -> ("Value"=w794:i32)  [unwired: 2 in, 2 out]
                n582 = property on="R Scan Length SP steps" class="DigNum (strict)"() -> ("Value"=w793:i32)  [unwired: 2 in, 2 out]
                n583 = property on="X Step SP" class="DigNum (strict)"() -> ("Value"=w792:i32)  [unwired: 2 in, 2 out]
                n584 = property on="Y Step SP" class="DigNum (strict)"() -> ("Value"=w791:i32)  [unwired: 2 in, 2 out]
                n585 = property on="Z Step SP" class="DigNum (strict)"() -> ("Value"=w790:i32)  [unwired: 2 in, 2 out]
                n586 = property on="R Step SP" class="DigNum (strict)"() -> ("Value"=w789:i32)  [unwired: 2 in, 2 out]
                n587 = Add(x=w796, y=w792) -> (x+y=w805:i32)
                n588 = Add(x=w795, y=w791) -> (x+y=w804:i32)
                n589 = Add(x=w794, y=w790) -> (x+y=w803:i32)
                n590 = Add(x=w793, y=w789) -> (x+y=w802:i32)
                n591 = property on="X Step PV" class="DigNum (strict)"() -> ("Value"=w788:i32)  [unwired: 2 in, 2 out]
                n592 = property on="Y Step PV" class="DigNum (strict)"() -> ("Value"=w787:i32)  [unwired: 2 in, 2 out]
                n593 = property on="Z Step PV" class="DigNum (strict)"() -> ("Value"=w786:i32)  [unwired: 2 in, 2 out]
                n594 = property on="R Step PV" class="DigNum (strict)"() -> ("Value"=w785:i32)  [unwired: 2 in, 2 out]
                n595 = Equal?(x=w788, y=w805) -> (x = y?=w801:bool)
                n596 = Equal?(x=w787, y=w804) -> (x = y?=w800:bool)
                n597 = Equal?(x=w786, y=w803) -> (x = y?=w798:bool)
                n598 = Equal?(x=w785, y=w802) -> (x = y?=w799:bool)
                n599 = Compound Arithmetic op=AND(w801, w800, w798, w799) -> (w797:bool)
                n600 = case shown="True" w797 {
                  frame False {
                  }
                  frame True {
                    n601 = local write "Scan Go"(FALSE ("Scan Go")) -> ()
                    n602 = local write "STATUS"("DONE" ("STATUS")) -> ()
                    n603 = property on="Send scan parameter" class="Bool"("DisabledEnum"=T9."Enabled" ("Disabled")) -> ()  [unwired: 2 in, 2 out]
                    n604 = property on="Set Scan \nParameters" class="Bool"("DisabledEnum"=T9."Enabled" ("Disabled")) -> ()  [unwired: 2 in, 2 out]
                    n605 = property on="GO" class="Bool"("DisabledEnum"=T9."Enabled" ("Disabled")) -> ()  [unwired: 2 in, 2 out]
                  }
                }
              }
            }
          }
        }
        n606 = case shown="False" w497 {
          tunnel: w501 -> [w542 w547]
          tunnel: [w542 w546] -> w500
          tunnel: w499 -> [w541 w545]
          tunnel: [w541 w544] -> w498
          frame False {
          }
          frame True {
            w543 = 0 ("dimension size")
            n607 = Reshape Array(w547, w543) -> (w546:dbl[])
            n608 = Reshape Array(w545, w543) -> (w544:dbl[])
          }
        }
        n609 = And(x=w511, y=w507) -> (x .and. y?=w508:bool)
        n610 = case shown="False" w507 {
          frame False {
            n611 = local write "STATUS"("SCANNING MODE" ("STATUS")) -> ()
          }
          frame True {
          }
        }
        n612 = Divide(x=w530, y=6.283185307179586) -> (x/y=w531:dbl)
        n613 = case shown="False" w508 {
          frame False {
          }
          frame True {
            n614 = local write "STATUS"("") -> ()
          }
        }
        n615 = Multiply(x=360.0, y=w531) -> (x*y=w534:dbl)
        n616 = property on="atan Y/Z" class="DigNum (strict)"("Val(Sgnl)"=w534) -> ()  [unwired: 2 in, 2 out]
      }
      event "OK Button": Value Change {
        n617 = event-data() -> ()  [unwired: 1 in, 5 out]
        n618 = property on="OK Button" class="Bool (strict)"() -> ("Value"=w1345:bool)  [unwired: 2 in, 2 out]
        n619 = property on="Z Step PV" class="DigNum (strict)"() -> ("Value"=w1350:i32)  [unwired: 2 in, 2 out]
        n620 = Greater?(x=w1350, y=15360000) -> (0:w1347:bool)
        n621 = Equal?(x=w1345, y=TRUE) -> (x = y?=w1348:bool)
        n622 = local write "STATUS"("VALVE CHANGED" ("STATUS")) -> ()
        n623 = And(x=w1348, y=w1347) -> (x .and. y?=w1346:bool)
        n624 = case shown="False" w1346 {
          frame False {
            n625 = property on="OK Button" class="Bool (strict)"() -> ("Value"=w1353:bool)  [unwired: 2 in, 2 out]
            n626 = property on="Z Step PV" class="DigNum (strict)"() -> ("Value"=w1358:i32)  [unwired: 2 in, 2 out]
            n627 = Greater?(x=w1358, y=15360000) -> (0:w1356:bool)
            n628 = Equal?(x=w1353, y=FALSE) -> (x = y?=w1355:bool)
            n629 = And(x=w1355, y=w1356) -> (x .and. y?=w1354:bool)
            n630 = case shown="True" w1354 {
              frame False {
              }
              frame True {
                n631 = One Button Dialog(message="YOU CAN'T CLOSE THE VALVE\nWHEN YOU ARE IN THE THIS\nPOSITION!!") -> (true=w1360:bool)  [unwired: 1 in]
                n632 = property on="OK Button" class="Bool (strict)"("Val(Sgnl)"=w1360) -> ()  [unwired: 2 in, 2 out]
              }
            }
          }
          frame True {
            n633 = flat-sequence {
              frame #0 {
                n634 = local read "OK Button"() -> (w1363:bool)
                n635 = call "DigitalIO_sub_V1_CNTL.vi"("OK Button"=w1363) -> ("Boolean"=w1362:bool)  [unwired: 2 in]
                n636 = property on="V5 Valve \nopend/closed" class="Bool (strict)"("Val(Sgnl)"=w1362) -> ()  [unwired: 2 in, 2 out]
              }
              frame #1 {
                n637 = call "DigitalIO_sub_V1_MON.vi"() -> ("CL"=w1365:bool, "OP"=w1364:bool)  [unwired: 8 in]
                n638 = property on="OP" class="Bool (strict)"("Val(Sgnl)"=w1364) -> ()  [unwired: 2 in, 2 out]
                n639 = property on="CL" class="Bool (strict)"("Val(Sgnl)"=w1365) -> ()  [unwired: 2 in, 2 out]
              }
              frame #2 {
                n640 = Wait (ms)(milliseconds to wait=u32 100) -> ()  [unwired: 1 out]
              }
            }
          }
        }
      }
      event "GO": Mouse Up {
        n641 = event-data() -> ()  [unwired: 1 in, 7 out]
        n642 = local write "STATUS"("MOVING" ("STATUS")) -> ()
        n643 = property on="X Position mm PV" class="DigNum (strict)"() -> ("Value"=w1387:dbl)  [unwired: 2 in, 2 out]
        n644 = property on="X Position SP mm" class="DigNum (strict)"() -> ("Value"=w1386:dbl)  [unwired: 2 in, 2 out]
        n645 = property on="Z Position mm PV" class="DigNum (strict)"() -> ("Value"=w1383:dbl)  [unwired: 2 in, 2 out]
        n646 = property on="Z Position SP mm" class="DigNum (strict)"() -> ("Value"=w1375:dbl)  [unwired: 2 in, 2 out]
        n647 = property on="Y Position mm PV" class="DigNum (strict)"() -> ("Value"=w1381:dbl)  [unwired: 2 in, 2 out]
        n648 = property on="Y Position SP mm" class="DigNum (strict)"() -> ("Value"=w1380:dbl)  [unwired: 2 in, 2 out]
        n649 = property on="R Position SP deg" class="DigNum (strict)"() -> ("Value"=w1378:dbl)  [unwired: 2 in, 2 out]
        n650 = property on="R Position deg PV" class="DigNum (strict)"() -> ("Value"=w1377:dbl)  [unwired: 2 in, 2 out]
        n651 = Not Equal?(x=w1387, y=w1386) -> (x != y?=w1385:bool)
        n652 = Not Equal?(x=w1383, y=w1375) -> (x != y?=w1384:bool)
        n653 = Not Equal?(x=w1381, y=w1380) -> (x != y?=w1382:bool)
        n654 = Not Equal?(x=w1378, y=w1377) -> (x != y?=w1379:bool)
        n655 = case shown="True" w1384 {
          tunnel: w1394 -> [w1537 w1544]
          tunnel: w1393 -> [w1538 w1543]
          tunnel: [w1538 w1542] -> w1372
          tunnel: [w1537 w1541] -> w1371
          frame False {
          }
          frame True {
            n656 = flat-sequence {
              tunnel: w1543 -> [w1566]
              tunnel: w1544 -> [w1567]
              tunnel: [w1567] -> w1540
              tunnel: [w1566] -> w1539
              tunnel: [w1582] -> w1558
              tunnel: [w1581] -> w1557
              tunnel: [w1569] -> w1556
              tunnel: w1540 -> [w1582]
              tunnel: w1539 -> [w1581]
              tunnel: [w1585] -> w1555
              tunnel: [w1584] -> w1554
              tunnel: [w1583] -> w1553
              tunnel: w1556 -> [w1583]
              tunnel: w1557 -> [w1584]
              tunnel: w1558 -> [w1585]
              tunnel: [w1601] -> w1552
              tunnel: [w1600] -> w1551
              tunnel: w1555 -> [w1599]
              tunnel: w1554 -> [w1598]
              tunnel: [w1597] -> w1550
              tunnel: w1553 -> [w1597]
              tunnel: w1552 -> [w1608]
              tunnel: [w1608] -> w1549
              tunnel: w1551 -> [w1607]
              tunnel: [w1607] -> w1548
              tunnel: w1550 -> [w1606]
              tunnel: [w1606] -> w1547
              tunnel: [w1613] -> w1546
              tunnel: [w1612] -> w1545
              tunnel: w1549 -> [w1611]
              tunnel: w1548 -> [w1610]
              tunnel: w1547 -> [w1609]
              tunnel: [w1617] -> w1541
              tunnel: [w1618] -> w1542
              tunnel: w1546 -> [w1618]
              tunnel: w1545 -> [w1617]
              frame #0 {
                n657 = property on="Z Position mm PV" class="DigNum (strict)"() -> ("Value"=w1559:dbl)  [unwired: 2 in, 2 out]
                n658 = property on="Z Position SP mm" class="DigNum (strict)"() -> ("Value"=w1561:dbl)  [unwired: 2 in, 2 out]
                n659 = Less?(x=w1559, y=60.0) -> (x < y?=w1563:bool)
                n660 = Greater?(x=w1561, y=60.0) -> (0:w1564:bool)
                n661 = And(x=w1563, y=w1564) -> (x .and. y?=w1565:bool)
                n662 = case shown="True" w1565 {
                  frame False {
                  }
                  frame True {
                    n663 = property on="Z Position SP mm" class="DigNum (strict)"("Val(Sgnl)"=60.0 ("Value (Signaling)")) -> ()  [unwired: 2 in, 2 out]
                  }
                }
              }
              frame #1 {
                n664 = property on="Z steps/rev" class="DigNum (strict)"() -> ("Value"=w1578:u32)  [unwired: 2 in, 2 out]
                n665 = To Double Precision Float(number=w1578) -> (double precision float=w1574:dbl)
                n666 = property on="Z offset mm" class="DigNum (strict)"() -> ("Value"=w1576:dbl)  [unwired: 2 in, 2 out]
                n667 = property on="Z Position SP mm" class="DigNum (strict)"() -> ("Value"=w1575:dbl)  [unwired: 2 in, 2 out]
                n668 = Subtract(x=w1575, y=w1576) -> (x-y=w1571:dbl)
                n669 = property on="Z mm/rev" class="DigNum (strict)"() -> ("Value"=w1577:dbl)  [unwired: 2 in, 2 out]
                n670 = Divide(x=w1571, y=w1577) -> (x/y=w1570:dbl)
                n671 = property on="Z Step SP" class="DigNum (strict)"() -> ("Maximum"=w1580:dbl)  [unwired: 2 in, 2 out]
                n672 = property on="Z Step SP" class="DigNum (strict)"() -> ("Minimum"=w1579:dbl)  [unwired: 2 in, 2 out]
                n673 = Multiply(x=w1570, y=w1574) -> (x*y=w1572:dbl)
                n674 = In Range and Coerce(upper limit=w1580, x=w1572, lower limit=w1579) -> (coerced(x)=w1573:dbl)  [unwired: 1 out]
                n675 = To Long Integer(number=w1573) -> (32bit integer=w1569:i32)
                n676 = property on="Z Step SP" class="DigNum (strict)"("Val(Sgnl)"=w1569) -> ()  [unwired: 2 in, 2 out]
              }
              frame #2 {
                n677 = property on="Z Step SP" class="DigNum (strict)"() -> ("Value"=w1594:i32)  [unwired: 2 in, 2 out]
                n678 = property on="Z Step PV" class="DigNum (strict)"() -> ("Value"=w1593:i32)  [unwired: 2 in, 2 out]
                n679 = property on="Z Backlash" class="DigNum (strict)"() -> ("Value"=w1586:i32)  [unwired: 2 in, 2 out]
                n680 = Subtract(x=w1594, y=w1593) -> (x-y=w1592:i32)
                n681 = Sign(1:w1586) -> (0:w1590:i32)
                n682 = Sign(1:w1592) -> (0:w1591:i32)
                n683 = Multiply(x=w1591, y=w1590) -> (x*y=w1589:i32)
                n684 = Equal?(x=w1589, y=1) -> (x = y?=w1587:bool)
                n685 = case shown="False" w1587 {
                  frame False {
                    n686 = property on="Z Backlash corr" class="Bool (strict)"("Val(Sgnl)"=FALSE ("Value (Signaling)")) -> ()  [unwired: 2 in, 2 out]
                  }
                  frame True {
                    n687 = property on="Z Backlash corr" class="Bool (strict)"("Val(Sgnl)"=TRUE ("Value (Signaling)")) -> ()  [unwired: 2 in, 2 out]
                  }
                }
              }
              frame #3 {
                # "Velocity Setting"
                n688 = property on="Z Velocity SP step/sec" class="DigNum (strict)"() -> ("Value"=w1602:i32)  [unwired: 2 in, 2 out]
                n689 = Number To Decimal String(number=w1602) -> (decimal integer string=w1603:string)  [unwired: 1 in]
                n690 = call "mdrive send command.vi"("error in (no error)"=w1599, "Extra"=w1603, "Command"=T10."Max Velocity", "VISA resource name"=w1598) -> ("error out"=w1600:errorcluster, "VISA resource name out"=w1601:refnum<visa-resource-name>)  [unwired: 3 in, 1 out]
              }
              frame #4 {
                n691 = Wait (ms)(milliseconds to wait=u32 50) -> ()  [unwired: 1 out]
              }
              frame #5 {
                # "Move to Abs Position"
                n692 = Number To Decimal String(number=w1609) -> (decimal integer string=w1615:string)  [unwired: 1 in]
                n693 = call "mdrive send command.vi"("error in (no error)"=w1610, "Extra"=w1615, "Command"=T10."Move to Absolute Position", "VISA resource name"=w1611) -> ("error out"=w1612:errorcluster, "VISA resource name out"=w1613:refnum<visa-resource-name>)  [unwired: 3 in, 1 out]
              }
              frame #6 {
                n694 = Wait (ms)(milliseconds to wait=u32 50) -> ()  [unwired: 1 out]
              }
            }
          }
        }
        n695 = property on="GO" class="Bool"("DisabledEnum"=T9."Disabled and Grayed Out" ("Disabled")) -> ()  [unwired: 2 in, 2 out]
        n696 = case shown="True" w1385 {
          tunnel: w1396 -> [w1620 w1624]
          tunnel: w1395 -> [w1619 w1623]
          tunnel: [w1620 w1622] -> w1374
          tunnel: [w1619 w1621] -> w1373
          frame False {
          }
          frame True {
            n697 = flat-sequence {
              tunnel: w1623 -> [w1651]
              tunnel: w1624 -> [w1652]
              tunnel: [w1652] -> w1638
              tunnel: [w1651] -> w1637
              tunnel: [w1640] -> w1636
              tunnel: [w1655] -> w1635
              tunnel: [w1654] -> w1634
              tunnel: [w1653] -> w1633
              tunnel: w1636 -> [w1653]
              tunnel: w1637 -> [w1654]
              tunnel: w1638 -> [w1655]
              tunnel: [w1671] -> w1632
              tunnel: [w1670] -> w1631
              tunnel: w1635 -> [w1669]
              tunnel: w1634 -> [w1668]
              tunnel: w1633 -> [w1667]
              tunnel: [w1667] -> w1630
              tunnel: w1632 -> [w1678]
              tunnel: [w1678] -> w1629
              tunnel: w1631 -> [w1677]
              tunnel: [w1677] -> w1628
              tunnel: [w1675] -> w1627
              tunnel: w1630 -> [w1675]
              tunnel: [w1683] -> w1626
              tunnel: [w1682] -> w1625
              tunnel: w1629 -> [w1681]
              tunnel: w1628 -> [w1680]
              tunnel: w1627 -> [w1679]
              tunnel: [w1687] -> w1621
              tunnel: [w1688] -> w1622
              tunnel: w1626 -> [w1688]
              tunnel: w1625 -> [w1687]
              frame #0 {
                n698 = property on="X steps/rev" class="DigNum (strict)"() -> ("Value"=w1650:u32)  [unwired: 2 in, 2 out]
                n699 = To Double Precision Float(number=w1650) -> (double precision float=w1645:dbl)
                n700 = property on="X offset mm" class="DigNum (strict)"() -> ("Value"=w1649:dbl)  [unwired: 2 in, 2 out]
                n701 = property on="X Position SP mm" class="DigNum (strict)"() -> ("Value"=w1648:dbl)  [unwired: 2 in, 2 out]
                n702 = Subtract(x=w1648, y=w1649) -> (x-y=w1642:dbl)
                n703 = property on="X mm/rev" class="DigNum (strict)"() -> ("Value"=w1639:dbl)  [unwired: 2 in, 2 out]
                n704 = Divide(x=w1642, y=w1639) -> (x/y=w1641:dbl)
                n705 = property on="X Step SP" class="DigNum (strict)"() -> ("Maximum"=w1647:dbl)  [unwired: 2 in, 2 out]
                n706 = property on="X Step SP" class="DigNum (strict)"() -> ("Minimum"=w1646:dbl)  [unwired: 2 in, 2 out]
                n707 = Multiply(x=w1641, y=w1645) -> (x*y=w1643:dbl)
                n708 = In Range and Coerce(upper limit=w1647, x=w1643, lower limit=w1646) -> (coerced(x)=w1644:dbl)  [unwired: 1 out]
                n709 = To Long Integer(number=w1644) -> (32bit integer=w1640:i32)
                n710 = property on="X Step SP" class="DigNum (strict)"("Val(Sgnl)"=w1640) -> ()  [unwired: 2 in, 2 out]
              }
              frame #1 {
                n711 = property on="X Step SP" class="DigNum (strict)"() -> ("Value"=w1664:i32)  [unwired: 2 in, 2 out]
                n712 = property on="X Step PV" class="DigNum (strict)"() -> ("Value"=w1663:i32)  [unwired: 2 in, 2 out]
                n713 = property on="X Backlash" class="DigNum (strict)"() -> ("Value"=w1656:i32)  [unwired: 2 in, 2 out]
                n714 = Subtract(x=w1664, y=w1663) -> (x-y=w1662:i32)
                n715 = Sign(1:w1656) -> (0:w1660:i32)
                n716 = Sign(1:w1662) -> (0:w1661:i32)
                n717 = Multiply(x=w1661, y=w1660) -> (x*y=w1659:i32)
                n718 = Equal?(x=w1659, y=1) -> (x = y?=w1657:bool)
                n719 = case shown="False" w1657 {
                  frame False {
                    n720 = property on="X Backlash corr" class="Bool (strict)"("Val(Sgnl)"=FALSE ("Value (Signaling)")) -> ()  [unwired: 2 in, 2 out]
                  }
                  frame True {
                    n721 = property on="X Backlash corr" class="Bool (strict)"("Val(Sgnl)"=TRUE ("Value (Signaling)")) -> ()  [unwired: 2 in, 2 out]
                  }
                }
              }
              frame #2 {
                # "Velocity Setting"
                n722 = property on="X Velocity SP step/sec" class="DigNum (strict)"() -> ("Value"=w1672:i32)  [unwired: 2 in, 2 out]
                n723 = Number To Decimal String(number=w1672) -> (decimal integer string=w1673:string)  [unwired: 1 in]
                n724 = call "mDrive Send Command.vi"("error in (no error)"=w1668, "Extra"=w1673, "Command"=T10."Max Velocity", "VISA resource name"=w1669) -> ("error out"=w1670:errorcluster, "VISA resource name out"=w1671:refnum<visa-resource-name>)  [unwired: 3 in, 1 out]
              }
              frame #3 {
                n725 = Wait (ms)(milliseconds to wait=u32 50) -> ()  [unwired: 1 out]
              }
              frame #4 {
                # "Move to Abs Position"
                n726 = Number To Decimal String(number=w1679) -> (decimal integer string=w1685:string)  [unwired: 1 in]
                n727 = call "mDrive Send Command.vi"("error in (no error)"=w1680, "Extra"=w1685, "Command"=T10."Move to Absolute Position", "VISA resource name"=w1681) -> ("error out"=w1682:errorcluster, "VISA resource name out"=w1683:refnum<visa-resource-name>)  [unwired: 3 in, 1 out]
              }
              frame #5 {
                n728 = Wait (ms)(milliseconds to wait=u32 50) -> ()  [unwired: 1 out]
              }
            }
          }
        }
        n729 = case shown="True" w1382 {
          tunnel: w1392 -> [w1467 w1472]
          tunnel: w1391 -> [w1468 w1471]
          tunnel: [w1468 w1470] -> w1370
          tunnel: [w1467 w1469] -> w1369
          frame False {
          }
          frame True {
            n730 = flat-sequence {
              tunnel: [w1500] -> w1486
              tunnel: [w1499] -> w1485
              tunnel: [w1487] -> w1484
              tunnel: w1471 -> [w1499]
              tunnel: w1472 -> [w1500]
              tunnel: [w1503] -> w1483
              tunnel: [w1502] -> w1482
              tunnel: [w1501] -> w1481
              tunnel: w1484 -> [w1501]
              tunnel: w1485 -> [w1502]
              tunnel: w1486 -> [w1503]
              tunnel: [w1519] -> w1480
              tunnel: [w1518] -> w1479
              tunnel: w1483 -> [w1517]
              tunnel: w1482 -> [w1516]
              tunnel: [w1515] -> w1478
              tunnel: w1481 -> [w1515]
              tunnel: w1480 -> [w1526]
              tunnel: [w1526] -> w1477
              tunnel: w1479 -> [w1525]
              tunnel: [w1525] -> w1476
              tunnel: [w1523] -> w1475
              tunnel: w1478 -> [w1523]
              tunnel: [w1531] -> w1474
              tunnel: [w1530] -> w1473
              tunnel: w1477 -> [w1529]
              tunnel: w1476 -> [w1528]
              tunnel: w1475 -> [w1527]
              tunnel: [w1534] -> w1469
              tunnel: [w1536] -> w1470
              tunnel: w1474 -> [w1536]
              tunnel: w1473 -> [w1534]
              frame #0 {
                n731 = property on="Y steps/rev" class="DigNum (strict)"() -> ("Value"=w1496:u32)  [unwired: 2 in, 2 out]
                n732 = To Double Precision Float(number=w1496) -> (double precision float=w1492:dbl)
                n733 = property on="Y offset mm" class="DigNum (strict)"() -> ("Value"=w1494:dbl)  [unwired: 2 in, 2 out]
                n734 = property on="Y Position SP mm" class="DigNum (strict)"() -> ("Value"=w1493:dbl)  [unwired: 2 in, 2 out]
                n735 = Subtract(x=w1493, y=w1494) -> (x-y=w1489:dbl)
                n736 = property on="Y mm/rev" class="DigNum (strict)"() -> ("Value"=w1495:dbl)  [unwired: 2 in, 2 out]
                n737 = Divide(x=w1489, y=w1495) -> (x/y=w1488:dbl)
                n738 = property on="Y Step SP" class="DigNum (strict)"() -> ("Maximum"=w1497:dbl)  [unwired: 2 in, 2 out]
                n739 = property on="Y Step SP" class="DigNum (strict)"() -> ("Minimum"=w1498:dbl)  [unwired: 2 in, 2 out]
                n740 = Multiply(x=w1488, y=w1492) -> (x*y=w1490:dbl)
                n741 = In Range and Coerce(upper limit=w1497, x=w1490, lower limit=w1498) -> (coerced(x)=w1491:dbl)  [unwired: 1 out]
                n742 = To Long Integer(number=w1491) -> (32bit integer=w1487:i32)
                n743 = property on="Y Step SP" class="DigNum (strict)"("Val(Sgnl)"=w1487) -> ()  [unwired: 2 in, 2 out]
              }
              frame #1 {
                n744 = property on="Y Step SP" class="DigNum (strict)"() -> ("Value"=w1512:i32)  [unwired: 2 in, 2 out]
                n745 = property on="Y Step PV" class="DigNum (strict)"() -> ("Value"=w1511:i32)  [unwired: 2 in, 2 out]
                n746 = property on="Y Backlash" class="DigNum (strict)"() -> ("Value"=w1504:i32)  [unwired: 2 in, 2 out]
                n747 = Subtract(x=w1512, y=w1511) -> (x-y=w1510:i32)
                n748 = Sign(1:w1504) -> (0:w1508:i32)
                n749 = Sign(1:w1510) -> (0:w1509:i32)
                n750 = Multiply(x=w1509, y=w1508) -> (x*y=w1507:i32)
                n751 = Equal?(x=w1507, y=1) -> (x = y?=w1505:bool)
                n752 = case shown="False" w1505 {
                  frame False {
                    n753 = property on="Y Backlash corr" class="Bool (strict)"("Val(Sgnl)"=FALSE ("Value (Signaling)")) -> ()  [unwired: 2 in, 2 out]
                  }
                  frame True {
                    n754 = property on="Y Backlash corr" class="Bool (strict)"("Val(Sgnl)"=TRUE ("Value (Signaling)")) -> ()  [unwired: 2 in, 2 out]
                  }
                }
              }
              frame #2 {
                # "Velocity Setting"
                n755 = property on="Y Velocity SP step/sec" class="DigNum (strict)"() -> ("Value"=w1520:i32)  [unwired: 2 in, 2 out]
                n756 = Number To Decimal String(number=w1520) -> (decimal integer string=w1521:string)  [unwired: 1 in]
                n757 = call "mdrive send command.vi"("error in (no error)"=w1517, "Extra"=w1521, "Command"=T10."Max Velocity", "VISA resource name"=w1516) -> ("error out"=w1518:errorcluster, "VISA resource name out"=w1519:refnum<visa-resource-name>)  [unwired: 3 in, 1 out]
              }
              frame #3 {
                n758 = Wait (ms)(milliseconds to wait=u32 50) -> ()  [unwired: 1 out]
              }
              frame #4 {
                # "Move to Abs Position"
                n759 = Number To Decimal String(number=w1527) -> (decimal integer string=w1533:string)  [unwired: 1 in]
                n760 = call "mdrive send command.vi"("error in (no error)"=w1528, "Extra"=w1533, "Command"=T10."Move to Absolute Position", "VISA resource name"=w1529) -> ("error out"=w1530:errorcluster, "VISA resource name out"=w1531:refnum<visa-resource-name>)  [unwired: 3 in, 1 out]
              }
              frame #5 {
                n761 = Wait (ms)(milliseconds to wait=u32 25) -> ()  [unwired: 1 out]
              }
            }
          }
        }
        n762 = case shown="True" w1379 {
          tunnel: w1390 -> [w1397 w1402]
          tunnel: w1389 -> [w1398 w1401]
          tunnel: [w1398 w1400] -> w1368
          tunnel: [w1397 w1399] -> w1367
          frame False {
          }
          frame True {
            n763 = flat-sequence {
              tunnel: w1401 -> [w1429]
              tunnel: w1402 -> [w1430]
              tunnel: [w1430] -> w1416
              tunnel: [w1429] -> w1415
              tunnel: [w1417] -> w1414
              tunnel: [w1433] -> w1413
              tunnel: [w1432] -> w1412
              tunnel: [w1431] -> w1411
              tunnel: w1414 -> [w1431]
              tunnel: w1415 -> [w1432]
              tunnel: w1416 -> [w1433]
              tunnel: [w1449] -> w1410
              tunnel: [w1448] -> w1409
              tunnel: w1413 -> [w1447]
              tunnel: w1412 -> [w1446]
              tunnel: [w1445] -> w1408
              tunnel: w1411 -> [w1445]
              tunnel: w1410 -> [w1456]
              tunnel: [w1456] -> w1407
              tunnel: w1409 -> [w1455]
              tunnel: [w1455] -> w1406
              tunnel: w1408 -> [w1454]
              tunnel: [w1454] -> w1405
              tunnel: [w1461] -> w1404
              tunnel: [w1460] -> w1403
              tunnel: w1407 -> [w1459]
              tunnel: w1406 -> [w1458]
              tunnel: w1405 -> [w1457]
              tunnel: [w1466] -> w1400
              tunnel: w1404 -> [w1466]
              tunnel: w1403 -> [w1465]
              tunnel: [w1465] -> w1399
              frame #0 {
                n764 = property on="R steps/rev" class="DigNum (strict)"() -> ("Value"=w1425:u32)  [unwired: 2 in, 2 out]
                n765 = To Double Precision Float(number=w1425) -> (double precision float=w1422:dbl)
                n766 = property on="R offset deg" class="DigNum (strict)"() -> ("Value"=w1426:dbl)  [unwired: 2 in, 2 out]
                n767 = property on="R Position SP deg" class="DigNum (strict)"() -> ("Value"=w1427:dbl)  [unwired: 2 in, 2 out]
                n768 = Subtract(x=w1427, y=w1426) -> (x-y=w1419:dbl)
                n769 = property on="R deg/rev" class="DigNum (strict)"() -> ("Value"=w1428:dbl)  [unwired: 2 in, 2 out]
                n770 = Divide(x=w1419, y=w1428) -> (x/y=w1418:dbl)
                n771 = property on="R Step SP" class="DigNum (strict)"() -> ("Maximum"=w1423:dbl)  [unwired: 2 in, 2 out]
                n772 = Multiply(x=w1418, y=w1422) -> (x*y=w1420:dbl)
                n773 = property on="R Step SP" class="DigNum (strict)"() -> ("Minimum"=w1424:dbl)  [unwired: 2 in, 2 out]
                n774 = In Range and Coerce(upper limit=w1423, x=w1420, lower limit=w1424) -> (coerced(x)=w1421:dbl)  [unwired: 1 out]
                n775 = To Long Integer(number=w1421) -> (32bit integer=w1417:i32)
                n776 = property on="R Step SP" class="DigNum (strict)"("Val(Sgnl)"=w1417) -> ()  [unwired: 2 in, 2 out]
              }
              frame #1 {
                n777 = property on="R Step SP" class="DigNum (strict)"() -> ("Value"=w1442:i32)  [unwired: 2 in, 2 out]
                n778 = property on="R Step PV" class="DigNum (strict)"() -> ("Value"=w1441:i32)  [unwired: 2 in, 2 out]
                n779 = property on="R Backlash" class="DigNum (strict)"() -> ("Value"=w1434:i32)  [unwired: 2 in, 2 out]
                n780 = Subtract(x=w1442, y=w1441) -> (x-y=w1440:i32)
                n781 = Sign(1:w1434) -> (0:w1438:i32)
                n782 = Sign(1:w1440) -> (0:w1439:i32)
                n783 = Multiply(x=w1439, y=w1438) -> (x*y=w1437:i32)
                n784 = Equal?(x=w1437, y=1) -> (x = y?=w1435:bool)
                n785 = case shown="False" w1435 {
                  frame False {
                    n786 = property on="R Backlash corr" class="Bool (strict)"("Val(Sgnl)"=FALSE ("Value (Signaling)")) -> ()  [unwired: 2 in, 2 out]
                  }
                  frame True {
                    n787 = property on="R Backlash corr" class="Bool (strict)"("Val(Sgnl)"=TRUE ("Value (Signaling)")) -> ()  [unwired: 2 in, 2 out]
                  }
                }
              }
              frame #2 {
                # "Velocity Setting"
                n788 = property on="R Velocity SP step/sec" class="DigNum (strict)"() -> ("Value"=w1450:i32)  [unwired: 2 in, 2 out]
                n789 = Number To Decimal String(number=w1450) -> (decimal integer string=w1451:string)  [unwired: 1 in]
                n790 = call "mdrive send command.vi"("error in (no error)"=w1447, "Extra"=w1451, "Command"=T10."Max Velocity", "VISA resource name"=w1446) -> ("error out"=w1448:errorcluster, "VISA resource name out"=w1449:refnum<visa-resource-name>)  [unwired: 3 in, 1 out]
              }
              frame #3 {
                n791 = Wait (ms)(milliseconds to wait=u32 50) -> ()  [unwired: 1 out]
              }
              frame #4 {
                # "Move to Abs Position"
                n792 = Number To Decimal String(number=w1457) -> (decimal integer string=w1463:string)  [unwired: 1 in]
                n793 = call "mdrive send command.vi"("error in (no error)"=w1458, "Extra"=w1463, "Command"=T10."Move to Absolute Position", "VISA resource name"=w1459) -> ("error out"=w1460:errorcluster, "VISA resource name out"=w1461:refnum<visa-resource-name>)  [unwired: 3 in, 1 out]
              }
              frame #5 {
                n794 = Wait (ms)(milliseconds to wait=u32 25) -> ()  [unwired: 1 out]
              }
            }
          }
        }
      }
      event "HARDSTOP": Mouse Down {
        n795 = event-data() -> ()  [unwired: 1 in, 7 out]
        n796 = flat-sequence {
          tunnel: w1713 -> [w1742]
          tunnel: [w1741] -> w1708
          tunnel: w1692 -> [w1740]
          tunnel: [w1739] -> w1690
          tunnel: [w1746] -> w1709
          tunnel: w1708 -> [w1746]
          tunnel: [w1745] -> w1691
          tunnel: w1690 -> [w1745]
          tunnel: w1709 -> [w1763]
          tunnel: w1691 -> [w1760]
          tunnel: [w1759] -> _
          tunnel: [w1758] -> _
          frame #0 {
            n797 = call "mDrive Send Command.vi"("error in (no error)"=w1742, "Command"=T10."Stop", "VISA resource name"=w1740) -> ("error out"=w1741:errorcluster, "VISA resource name out"=w1739:refnum<visa-resource-name>)  [unwired: 4 in, 1 out]
          }
          frame #1 {
            n798 = Wait (ms)(milliseconds to wait=u32 50) -> ()  [unwired: 1 out]
          }
          frame #2 {
            n799 = property on="X steps/rev" class="DigNum (strict)"() -> ("Value"=w1749:u32)  [unwired: 2 in, 2 out]
            n800 = property on="X offset mm" class="DigNum (strict)"() -> ("Value"=w1747:dbl)  [unwired: 2 in, 2 out]
            n801 = To Double Precision Float(number=w1749) -> (double precision float=w1754:dbl)
            n802 = call "mDrive Send Command.vi"("error in (no error)"=w1763, "Extra"="P", "Command"=T10."Print Parameter", "VISA resource name"=w1760) -> ("error out"=w1758:errorcluster, "read buffer"=w1753:string, "VISA resource name out"=w1759:refnum<visa-resource-name>)  [unwired: 3 in]
            n803 = Decimal String To Number(string=w1753, offset=0) -> (number=w1751:i32)  [unwired: 1 in, 1 out]
            n804 = property on="X Step PV" class="DigNum (strict)"("Val(Sgnl)"=w1751) -> ()  [unwired: 2 in, 2 out]
            n805 = To Double Precision Float(number=w1751) -> (double precision float=w1755:dbl)
            n806 = Divide(x=w1755, y=w1754) -> (x/y=w1757:dbl)
            n807 = property on="X mm/rev" class="DigNum (strict)"() -> ("Value"=w1748:dbl)  [unwired: 2 in, 2 out]
            n808 = Multiply(x=w1757, y=w1748) -> (x*y=w1756:dbl)
            n809 = Add(x=w1756, y=w1747) -> (x+y=w1750:dbl)
            n810 = property on="X Position mm PV" class="DigNum (strict)"("Val(Sgnl)"=w1750) -> ()  [unwired: 2 in, 2 out]
          }
        }
        n811 = property on="GO" class="Bool"("DisabledEnum"=T9."Enabled" ("Disabled")) -> ()  [unwired: 2 in, 2 out]
        n812 = flat-sequence {
          tunnel: w1710 -> [w1717]
          tunnel: [w1716] -> w1702
          tunnel: w1701 -> [w1715]
          tunnel: [w1714] -> w1699
          tunnel: [w1721] -> w1703
          tunnel: w1702 -> [w1721]
          tunnel: [w1720] -> w1700
          tunnel: w1699 -> [w1720]
          tunnel: w1703 -> [w1738]
          tunnel: w1700 -> [w1735]
          tunnel: [w1734] -> _
          tunnel: [w1733] -> _
          frame #0 {
            n813 = call "mDrive Send Command.vi"("error in (no error)"=w1717, "Command"=T10."Stop", "VISA resource name"=w1715) -> ("error out"=w1716:errorcluster, "VISA resource name out"=w1714:refnum<visa-resource-name>)  [unwired: 4 in, 1 out]
          }
          frame #1 {
            n814 = Wait (ms)(milliseconds to wait=u32 50) -> ()  [unwired: 1 out]
          }
          frame #2 {
            n815 = property on="R steps/rev" class="DigNum (strict)"() -> ("Value"=w1726:u32)  [unwired: 2 in, 2 out]
            n816 = property on="R offset deg" class="DigNum (strict)"() -> ("Value"=w1723:dbl)  [unwired: 2 in, 2 out]
            n817 = To Double Precision Float(number=w1726) -> (double precision float=w1729:dbl)
            n818 = call "mDrive Send Command.vi"("error in (no error)"=w1738, "Extra"="P", "Command"=T10."Print Parameter", "VISA resource name"=w1735) -> ("error out"=w1733:errorcluster, "read buffer"=w1728:string, "VISA resource name out"=w1734:refnum<visa-resource-name>)  [unwired: 3 in]
            n819 = Decimal String To Number(string=w1728, offset=0) -> (number=w1725:i32)  [unwired: 1 in, 1 out]
            n820 = property on="R Step PV" class="DigNum (strict)"("Val(Sgnl)"=w1725) -> ()  [unwired: 2 in, 2 out]
            n821 = To Double Precision Float(number=w1725) -> (double precision float=w1730:dbl)
            n822 = Divide(x=w1730, y=w1729) -> (x/y=w1732:dbl)
            n823 = property on="R deg/rev" class="DigNum (strict)"() -> ("Value"=w1724:dbl)  [unwired: 2 in, 2 out]
            n824 = Multiply(x=w1732, y=w1724) -> (x*y=w1731:dbl)
            n825 = Add(x=w1731, y=w1723) -> (x+y=w1722:dbl)
            n826 = property on="R Position deg PV" class="DigNum (strict)"("Val(Sgnl)"=w1722) -> ()  [unwired: 2 in, 2 out]
          }
        }
        n827 = flat-sequence {
          tunnel: w1712 -> [w1767]
          tunnel: [w1766] -> w1706
          tunnel: w1695 -> [w1765]
          tunnel: [w1764] -> w1693
          tunnel: [w1771] -> w1707
          tunnel: w1706 -> [w1771]
          tunnel: [w1770] -> w1694
          tunnel: w1693 -> [w1770]
          tunnel: w1707 -> [w1788]
          tunnel: w1694 -> [w1785]
          tunnel: [w1784] -> _
          tunnel: [w1783] -> _
          frame #0 {
            n828 = call "mDrive Send Command.vi"("error in (no error)"=w1767, "Command"=T10."Stop", "VISA resource name"=w1765) -> ("error out"=w1766:errorcluster, "VISA resource name out"=w1764:refnum<visa-resource-name>)  [unwired: 4 in, 1 out]
          }
          frame #1 {
            n829 = Wait (ms)(milliseconds to wait=u32 50) -> ()  [unwired: 1 out]
          }
          frame #2 {
            n830 = property on="Z steps/rev" class="DigNum (strict)"() -> ("Value"=w1774:u32)  [unwired: 2 in, 2 out]
            n831 = property on="Z offset mm" class="DigNum (strict)"() -> ("Value"=w1772:dbl)  [unwired: 2 in, 2 out]
            n832 = To Double Precision Float(number=w1774) -> (double precision float=w1779:dbl)
            n833 = call "mDrive Send Command.vi"("error in (no error)"=w1788, "Extra"="P", "Command"=T10."Print Parameter", "VISA resource name"=w1785) -> ("error out"=w1783:errorcluster, "read buffer"=w1778:string, "VISA resource name out"=w1784:refnum<visa-resource-name>)  [unwired: 3 in]
            n834 = Decimal String To Number(string=w1778, offset=0) -> (number=w1776:i32)  [unwired: 1 in, 1 out]
            n835 = property on="Z Step PV" class="DigNum (strict)"("Val(Sgnl)"=w1776) -> ()  [unwired: 2 in, 2 out]
            n836 = To Double Precision Float(number=w1776) -> (double precision float=w1780:dbl)
            n837 = Divide(x=w1780, y=w1779) -> (x/y=w1782:dbl)
            n838 = property on="Z mm/rev" class="DigNum (strict)"() -> ("Value"=w1773:dbl)  [unwired: 2 in, 2 out]
            n839 = Multiply(x=w1782, y=w1773) -> (x*y=w1781:dbl)
            n840 = Add(x=w1781, y=w1772) -> (x+y=w1775:dbl)
            n841 = property on="Z Position mm PV" class="DigNum (strict)"("Val(Sgnl)"=w1775) -> ()  [unwired: 2 in, 2 out]
          }
        }
        n842 = flat-sequence {
          tunnel: w1711 -> [w1792]
          tunnel: [w1791] -> w1704
          tunnel: w1698 -> [w1790]
          tunnel: [w1789] -> w1696
          tunnel: [w1796] -> w1705
          tunnel: w1704 -> [w1796]
          tunnel: [w1795] -> w1697
          tunnel: w1696 -> [w1795]
          tunnel: w1705 -> [w1813]
          tunnel: w1697 -> [w1810]
          tunnel: [w1809] -> _
          tunnel: [w1808] -> _
          frame #0 {
            n843 = call "mDrive Send Command.vi"("error in (no error)"=w1792, "Command"=T10."Stop", "VISA resource name"=w1790) -> ("error out"=w1791:errorcluster, "VISA resource name out"=w1789:refnum<visa-resource-name>)  [unwired: 4 in, 1 out]
          }
          frame #1 {
            n844 = Wait (ms)(milliseconds to wait=u32 50) -> ()  [unwired: 1 out]
          }
          frame #2 {
            n845 = property on="Y steps/rev" class="DigNum (strict)"() -> ("Value"=w1799:u32)  [unwired: 2 in, 2 out]
            n846 = property on="Y offset mm" class="DigNum (strict)"() -> ("Value"=w1797:dbl)  [unwired: 2 in, 2 out]
            n847 = To Double Precision Float(number=w1799) -> (double precision float=w1804:dbl)
            n848 = call "mDrive Send Command.vi"("error in (no error)"=w1813, "Extra"="P", "Command"=T10."Print Parameter", "VISA resource name"=w1810) -> ("error out"=w1808:errorcluster, "read buffer"=w1803:string, "VISA resource name out"=w1809:refnum<visa-resource-name>)  [unwired: 3 in]
            n849 = Decimal String To Number(string=w1803, offset=0) -> (number=w1800:i32)  [unwired: 1 in, 1 out]
            n850 = property on="Y Step PV" class="DigNum (strict)"("Val(Sgnl)"=w1800) -> ()  [unwired: 2 in, 2 out]
            n851 = To Double Precision Float(number=w1800) -> (double precision float=w1805:dbl)
            n852 = Divide(x=w1805, y=w1804) -> (x/y=w1807:dbl)
            n853 = property on="Y mm/rev" class="DigNum (strict)"() -> ("Value"=w1798:dbl)  [unwired: 2 in, 2 out]
            n854 = Multiply(x=w1807, y=w1798) -> (x*y=w1806:dbl)
            n855 = Add(x=w1806, y=w1797) -> (x+y=w1801:dbl)
            n856 = property on="Y Position mm PV" class="DigNum (strict)"("Val(Sgnl)"=w1801) -> ()  [unwired: 2 in, 2 out]
          }
        }
      }
      event "Reset Y Position mm", "Reset X Position mm", "Reset Z Position mm", "Reset R Position deg": Value Change {
        n857 = event-data() -> ()  [unwired: 1 in, 5 out]
        n858 = property on="Y steps/rev" class="DigNum (strict)"() -> ("Value"=w1844:u32)  [unwired: 2 in, 2 out]
        n859 = property on="X steps/rev" class="DigNum (strict)"() -> ("Value"=w1835:u32)  [unwired: 2 in, 2 out]
        n860 = property on="Z steps/rev" class="DigNum (strict)"() -> ("Value"=w1826:u32)  [unwired: 2 in, 2 out]
        n861 = property on="R steps/rev" class="DigNum (strict)"() -> ("Value"=w1817:u32)  [unwired: 2 in, 2 out]
        n862 = property on="R offset deg" class="DigNum (strict)"() -> ("Value"=w1815:dbl)  [unwired: 2 in, 2 out]
        n863 = property on="Y offset mm" class="DigNum (strict)"() -> ("Value"=w1842:dbl)  [unwired: 2 in, 2 out]
        n864 = property on="X offset mm" class="DigNum (strict)"() -> ("Value"=w1833:dbl)  [unwired: 2 in, 2 out]
        n865 = property on="Z offset mm" class="DigNum (strict)"() -> ("Value"=w1824:dbl)  [unwired: 2 in, 2 out]
        n866 = To Double Precision Float(number=w1817) -> (double precision float=w1820:dbl)
        n867 = To Double Precision Float(number=w1835) -> (double precision float=w1838:dbl)
        n868 = To Double Precision Float(number=w1826) -> (double precision float=w1829:dbl)
        n869 = property on="Reset Y Position mm" class="DigNum (strict)"() -> ("Value"=w1850:dbl)  [unwired: 2 in, 2 out]
        n870 = property on="Reset X Position mm" class="DigNum (strict)"() -> ("Value"=w1841:dbl)  [unwired: 2 in, 2 out]
        n871 = property on="Reset Z Position mm" class="DigNum (strict)"() -> ("Value"=w1832:dbl)  [unwired: 2 in, 2 out]
        n872 = property on="Reset R Position deg" class="DigNum (strict)"() -> ("Value"=w1823:dbl)  [unwired: 2 in, 2 out]
        n873 = local write "STATUS"("RESSETTING" ("STATUS")) -> ()
        n874 = Subtract(x=w1850, y=w1842) -> (x-y=w1849:dbl)
        n875 = Subtract(x=w1823, y=w1815) -> (x-y=w1822:dbl)
        n876 = Subtract(x=w1841, y=w1833) -> (x-y=w1840:dbl)
        n877 = Subtract(x=w1832, y=w1824) -> (x-y=w1831:dbl)
        n878 = property on="Y mm/rev" class="DigNum (strict)"() -> ("Value"=w1843:dbl)  [unwired: 2 in, 2 out]
        n879 = property on="X mm/rev" class="DigNum (strict)"() -> ("Value"=w1834:dbl)  [unwired: 2 in, 2 out]
        n880 = property on="Z mm/rev" class="DigNum (strict)"() -> ("Value"=w1825:dbl)  [unwired: 2 in, 2 out]
        n881 = property on="R deg/rev" class="DigNum (strict)"() -> ("Value"=w1816:dbl)  [unwired: 2 in, 2 out]
        n882 = Divide(x=w1822, y=w1816) -> (x/y=w1821:dbl)
        n883 = Divide(x=w1840, y=w1834) -> (x/y=w1839:dbl)
        n884 = Divide(x=w1831, y=w1825) -> (x/y=w1830:dbl)
        n885 = Divide(x=w1849, y=w1843) -> (x/y=w1848:dbl)
        n886 = To Double Precision Float(number=w1844) -> (double precision float=w1847:dbl)
        n887 = Multiply(x=w1848, y=w1847) -> (x*y=w1846:dbl)
        n888 = Multiply(x=w1821, y=w1820) -> (x*y=w1819:dbl)
        n889 = Multiply(x=w1839, y=w1838) -> (x*y=w1837:dbl)
        n890 = Multiply(x=w1830, y=w1829) -> (x*y=w1828:dbl)
        n891 = To Long Integer(number=w1846) -> (32bit integer=w1845:i32)
        n892 = To Long Integer(number=w1819) -> (32bit integer=w1818:i32)
        n893 = To Long Integer(number=w1837) -> (32bit integer=w1836:i32)
        n894 = To Long Integer(number=w1828) -> (32bit integer=w1827:i32)
        n895 = property on="Reset Y Motor Steps" class="DigNum (strict)"("Val(Sgnl)"=w1845) -> ()  [unwired: 2 in, 2 out]
        n896 = property on="Reset R Motor Steps" class="DigNum (strict)"("Val(Sgnl)"=w1818) -> ()  [unwired: 2 in, 2 out]
        n897 = property on="Reset X Motor Steps" class="DigNum (strict)"("Val(Sgnl)"=w1836) -> ()  [unwired: 2 in, 2 out]
        n898 = property on="Reset Z Motor Steps" class="DigNum (strict)"("Val(Sgnl)"=w1827) -> ()  [unwired: 2 in, 2 out]
      }
      event "Y Velocity SP step/sec", "X Velocity SP step/sec", "R Velocity SP step/sec", "Z Velocity SP step/sec", "Y Step SP", "X Step SP", "Z Step SP", "R Step SP": Value Change {
        n899 = event-data() -> ()  [unwired: 1 in, 5 out]
        n900 = property on="X Step SP" class="DigNum (strict)"() -> ("Value"=w1875:i32)  [unwired: 2 in, 2 out]
        n901 = property on="Z Step SP" class="DigNum (strict)"() -> ("Value"=w1867:i32)  [unwired: 2 in, 2 out]
        n902 = property on="Y Step SP" class="DigNum (strict)"() -> ("Value"=w1883:i32)  [unwired: 2 in, 2 out]
        n903 = property on="X steps/rev" class="DigNum (strict)"() -> ("Value"=w1900:u32)  [unwired: 2 in, 2 out]
        n904 = property on="X steps/rev" class="DigNum (strict)"() -> ("Value"=w1873:u32)  [unwired: 2 in, 2 out]
        n905 = property on="R Step SP" class="DigNum (strict)"() -> ("Value"=w1859:i32)  [unwired: 2 in, 2 out]
        n906 = property on="Z steps/rev" class="DigNum (strict)"() -> ("Value"=w1894:u32)  [unwired: 2 in, 2 out]
        n907 = property on="Z steps/rev" class="DigNum (strict)"() -> ("Value"=w1865:u32)  [unwired: 2 in, 2 out]
        n908 = property on="Y steps/rev" class="DigNum (strict)"() -> ("Value"=w1906:u32)  [unwired: 2 in, 2 out]
        n909 = property on="Y steps/rev" class="DigNum (strict)"() -> ("Value"=w1881:u32)  [unwired: 2 in, 2 out]
        n910 = property on="R steps/rev" class="DigNum (strict)"() -> ("Value"=w1888:u32)  [unwired: 2 in, 2 out]
        n911 = property on="R steps/rev" class="DigNum (strict)"() -> ("Value"=w1857:u32)  [unwired: 2 in, 2 out]
        n912 = property on="R offset deg" class="DigNum (strict)"() -> ("Value"=w1856:dbl)  [unwired: 2 in, 2 out]
        n913 = property on="X offset mm" class="DigNum (strict)"() -> ("Value"=w1872:dbl)  [unwired: 2 in, 2 out]
        n914 = property on="Z offset mm" class="DigNum (strict)"() -> ("Value"=w1864:dbl)  [unwired: 2 in, 2 out]
        n915 = property on="Y offset mm" class="DigNum (strict)"() -> ("Value"=w1880:dbl)  [unwired: 2 in, 2 out]
        n916 = To Double Precision Float(number=w1900) -> (double precision float=w1905:dbl)
        n917 = To Double Precision Float(number=w1875) -> (double precision float=w1876:dbl)
        n918 = To Double Precision Float(number=w1873) -> (double precision float=w1879:dbl)
        n919 = To Double Precision Float(number=w1888) -> (double precision float=w1893:dbl)
        n920 = To Double Precision Float(number=w1859) -> (double precision float=w1860:dbl)
        n921 = To Double Precision Float(number=w1857) -> (double precision float=w1863:dbl)
        n922 = To Double Precision Float(number=w1894) -> (double precision float=w1899:dbl)
        n923 = To Double Precision Float(number=w1867) -> (double precision float=w1868:dbl)
        n924 = To Double Precision Float(number=w1865) -> (double precision float=w1871:dbl)
        n925 = To Double Precision Float(number=w1906) -> (double precision float=w1911:dbl)
        n926 = To Double Precision Float(number=w1883) -> (double precision float=w1884:dbl)
        n927 = To Double Precision Float(number=w1881) -> (double precision float=w1887:dbl)
        n928 = Divide(x=w1876, y=w1879) -> (x/y=w1878:dbl)
        n929 = Divide(x=w1868, y=w1871) -> (x/y=w1870:dbl)
        n930 = Divide(x=w1884, y=w1887) -> (x/y=w1886:dbl)
        n931 = Divide(x=w1860, y=w1863) -> (x/y=w1862:dbl)
        n932 = property on="X Velocity SP step/sec" class="DigNum (strict)"() -> ("Value"=w1902:i32)  [unwired: 2 in, 2 out]
        n933 = property on="X mm/rev" class="DigNum (strict)"() -> ("Value"=w1853:dbl)  [unwired: 2 in, 2 out]
        n934 = property on="Z Velocity SP step/sec" class="DigNum (strict)"() -> ("Value"=w1896:i32)  [unwired: 2 in, 2 out]
        n935 = property on="Z mm/rev" class="DigNum (strict)"() -> ("Value"=w1854:dbl)  [unwired: 2 in, 2 out]
        n936 = property on="Y Velocity SP step/sec" class="DigNum (strict)"() -> ("Value"=w1908:i32)  [unwired: 2 in, 2 out]
        n937 = property on="Y mm/rev" class="DigNum (strict)"() -> ("Value"=w1852:dbl)  [unwired: 2 in, 2 out]
        n938 = property on="R Velocity SP step/sec" class="DigNum (strict)"() -> ("Value"=w1890:i32)  [unwired: 2 in, 2 out]
        n939 = property on="R deg/rev" class="DigNum (strict)"() -> ("Value"=w1855:dbl)  [unwired: 2 in, 2 out]
        n940 = Multiply(x=w1878, y=w1853) -> (x*y=w1877:dbl)
        n941 = Multiply(x=w1862, y=w1855) -> (x*y=w1861:dbl)
        n942 = Multiply(x=w1870, y=w1854) -> (x*y=w1869:dbl)
        n943 = Multiply(x=w1886, y=w1852) -> (x*y=w1885:dbl)
        n944 = To Double Precision Float(number=w1902) -> (double precision float=w1903:dbl)
        n945 = To Double Precision Float(number=w1890) -> (double precision float=w1891:dbl)
        n946 = To Double Precision Float(number=w1896) -> (double precision float=w1897:dbl)
        n947 = To Double Precision Float(number=w1908) -> (double precision float=w1909:dbl)
        n948 = Divide(x=w1903, y=w1905) -> (x/y=w1904:dbl)
        n949 = Add(x=w1877, y=w1872) -> (x+y=w1874:dbl)
        n950 = Divide(x=w1891, y=w1893) -> (x/y=w1892:dbl)
        n951 = Add(x=w1861, y=w1856) -> (x+y=w1858:dbl)
        n952 = Divide(x=w1897, y=w1899) -> (x/y=w1898:dbl)
        n953 = Add(x=w1869, y=w1864) -> (x+y=w1866:dbl)
        n954 = Divide(x=w1909, y=w1911) -> (x/y=w1910:dbl)
        n955 = Add(x=w1885, y=w1880) -> (x+y=w1882:dbl)
        n956 = Multiply(x=w1904, y=w1853) -> (x*y=w1901:dbl)
        n957 = Multiply(x=w1892, y=w1855) -> (x*y=w1889:dbl)
        n958 = Multiply(x=w1898, y=w1854) -> (x*y=w1895:dbl)
        n959 = Multiply(x=w1910, y=w1852) -> (x*y=w1907:dbl)
        n960 = property on="X Position MV mm" class="DigNum (strict)"("Val(Sgnl)"=w1874) -> ()  [unwired: 2 in, 2 out]
        n961 = property on="R Position MV deg" class="DigNum (strict)"("Val(Sgnl)"=w1858) -> ()  [unwired: 2 in, 2 out]
        n962 = property on="Z Position MV mm" class="DigNum (strict)"("Val(Sgnl)"=w1866) -> ()  [unwired: 2 in, 2 out]
        n963 = property on="Y Position MV mm" class="DigNum (strict)"("Val(Sgnl)"=w1882) -> ()  [unwired: 2 in, 2 out]
        n964 = property on="X Velocity MV mm/sec" class="DigNum (strict)"("Val(Sgnl)"=w1901) -> ()  [unwired: 2 in, 2 out]
        n965 = property on="Z Velocity MV mm/sec" class="DigNum (strict)"("Val(Sgnl)"=w1895) -> ()  [unwired: 2 in, 2 out]
        n966 = property on="Y Velocity MV mm/sec" class="DigNum (strict)"("Val(Sgnl)"=w1907) -> ()  [unwired: 2 in, 2 out]
        n967 = Absolute Value(x=w1889) -> (abs(x)=w1851:dbl)
        n968 = property on="R Velocity MVdeg/sec" class="DigNum (strict)"("Val(Sgnl)"=w1851) -> ()  [unwired: 2 in, 2 out]
      }
      event "Y Scan Length SP steps", "Y Scan Velocity SP steps/sec", "X Scan Velocity SP steps/sec", "X Scan Length SP steps", "Z Scan Velocity SP steps/sec", "Z Scan Length SP steps", "R Scan Velocity SP steps/sec", "R Scan Length SP steps": Value Change {
        n969 = event-data() -> ()  [unwired: 1 in, 5 out]
        n970 = property on="R Step PV" class="DigNum (strict)"() -> ("Value"=w1944:i32)  [unwired: 2 in, 2 out]
        n971 = property on="X steps/rev" class="DigNum (strict)"() -> ("Value"=w1985:u32)  [unwired: 2 in, 2 out]
        n972 = property on="Y steps/rev" class="DigNum (strict)"() -> ("Value"=w1973:u32)  [unwired: 2 in, 2 out]
        n973 = property on="Z steps/rev" class="DigNum (strict)"() -> ("Value"=w1960:u32)  [unwired: 2 in, 2 out]
        n974 = property on="X Step PV" class="DigNum (strict)"() -> ("Value"=w1984:i32)  [unwired: 2 in, 2 out]
        n975 = property on="Y Step PV" class="DigNum (strict)"() -> ("Value"=w1971:i32)  [unwired: 2 in, 2 out]
        n976 = property on="Z Step PV" class="DigNum (strict)"() -> ("Value"=w1958:i32)  [unwired: 2 in, 2 out]
        n977 = property on="R steps/rev" class="DigNum (strict)"() -> ("Value"=w1946:u32)  [unwired: 2 in, 2 out]
        n978 = To Double Precision Float(number=w1984) -> (double precision float=w1938:dbl)
        n979 = To Double Precision Float(number=w1971) -> (double precision float=w1937:dbl)
        n980 = To Double Precision Float(number=w1958) -> (double precision float=w1936:dbl)
        n981 = To Double Precision Float(number=w1944) -> (double precision float=w1935:dbl)
        n982 = To Double Precision Float(number=w1985) -> (double precision float=w1983:dbl)
        n983 = To Double Precision Float(number=w1973) -> (double precision float=w1928:dbl)
        n984 = To Double Precision Float(number=w1946) -> (double precision float=w1943:dbl)
        n985 = To Double Precision Float(number=w1960) -> (double precision float=w1957:dbl)
        n986 = property on="X Step SP" class="DigNum (strict)"() -> ("Maximum"=w1988:dbl)  [unwired: 2 in, 2 out]
        n987 = property on="Y Step SP" class="DigNum (strict)"() -> ("Maximum"=w1977:dbl)  [unwired: 2 in, 2 out]
        n988 = property on="Z Step SP" class="DigNum (strict)"() -> ("Maximum"=w1964:dbl)  [unwired: 2 in, 2 out]
        n989 = property on="R Step SP" class="DigNum (strict)"() -> ("Maximum"=w1952:dbl)  [unwired: 2 in, 2 out]
        n990 = property on="X Scan Length SP steps" class="DigNum (strict)"() -> ("Value"=w1982:i32)  [unwired: 2 in, 2 out]
        n991 = property on="X Scan Length SP mm" class="DigNum (strict)"() -> ("Value"=w1914:dbl)  [unwired: 2 in, 2 out]
        n992 = property on="Y Scan Length SP mm" class="DigNum (strict)"() -> ("Value"=w1915:dbl)  [unwired: 2 in, 2 out]
        n993 = property on="Y Scan Length SP steps" class="DigNum (strict)"() -> ("Value"=w1974:i32)  [unwired: 2 in, 2 out]
        n994 = property on="Z Scan Length SP steps" class="DigNum (strict)"() -> ("Value"=w1961:i32)  [unwired: 2 in, 2 out]
        n995 = property on="R Scan Length SP steps" class="DigNum (strict)"() -> ("Value"=w1947:i32)  [unwired: 2 in, 2 out]
        n996 = property on="X Step SP" class="DigNum (strict)"() -> ("Minimum"=w1989:dbl)  [unwired: 2 in, 2 out]
        n997 = property on="Y Step SP" class="DigNum (strict)"() -> ("Minimum"=w1978:dbl)  [unwired: 2 in, 2 out]
        n998 = property on="Z Step SP" class="DigNum (strict)"() -> ("Minimum"=w1965:dbl)  [unwired: 2 in, 2 out]
        n999 = property on="R Step SP" class="DigNum (strict)"() -> ("Minimum"=w1949:dbl)  [unwired: 2 in, 2 out]
        n1000 = property on="Z Scan Velocity SP steps/sec" class="DigNum (strict)"() -> ("Value"=w1956:i32)  [unwired: 2 in, 2 out]
        n1001 = property on="R Scan Velocity SP steps/sec" class="DigNum (strict)"() -> ("Value"=w1942:i32)  [unwired: 2 in, 2 out]
        n1002 = Subtract(x=w1988, y=w1938) -> (x-y=w1987:dbl)
        n1003 = Subtract(x=w1989, y=w1938) -> (x-y=w1990:dbl)
        n1004 = Subtract(x=w1978, y=w1937) -> (x-y=w1979:dbl)
        n1005 = Subtract(x=w1977, y=w1937) -> (x-y=w1976:dbl)
        n1006 = Subtract(x=w1965, y=w1936) -> (x-y=w1966:dbl)
        n1007 = Subtract(x=w1964, y=w1936) -> (x-y=w1963:dbl)
        n1008 = Subtract(x=w1949, y=w1935) -> (x-y=w1950:dbl)
        n1009 = Subtract(x=w1952, y=w1935) -> (x-y=w1951:dbl)
        n1010 = To Double Precision Float(number=w1947) -> (double precision float=w1932:dbl)
        n1011 = To Double Precision Float(number=w1961) -> (double precision float=w1934:dbl)
        n1012 = To Double Precision Float(number=w1982) -> (double precision float=w1925:dbl)
        n1013 = To Double Precision Float(number=w1974) -> (double precision float=w1927:dbl)
        n1014 = property on="X Scan Velocity SP steps/sec" class="DigNum (strict)"() -> ("Value"=w1986:i32)  [unwired: 2 in, 2 out]
        n1015 = property on="Y Scan Velocity SP steps/sec" class="DigNum (strict)"() -> ("Value"=w1970:i32)  [unwired: 2 in, 2 out]
        n1016 = Equal?(x=w1914, y=0.0) -> (x = y?=w1912:bool)
        n1017 = Equal?(x=w1915, y=0.0) -> (x = y?=w1913:bool)
        n1018 = property on="X Scan Length SP steps" class="DigNum (strict)"("Maximum"=w1987) -> ()  [unwired: 2 in, 2 out]
        n1019 = property on="X Scan Length SP steps" class="DigNum (strict)"("Minimum"=w1990) -> ()  [unwired: 2 in, 2 out]
        n1020 = property on="Y Scan Length SP steps" class="DigNum (strict)"("Minimum"=w1979) -> ()  [unwired: 2 in, 2 out]
        n1021 = property on="Y Scan Length SP steps" class="DigNum (strict)"("Maximum"=w1976) -> ()  [unwired: 2 in, 2 out]
        n1022 = property on="Z Scan Length SP steps" class="DigNum (strict)"("Minimum"=w1966) -> ()  [unwired: 2 in, 2 out]
        n1023 = property on="Z Scan Length SP steps" class="DigNum (strict)"("Maximum"=w1963) -> ()  [unwired: 2 in, 2 out]
        n1024 = property on="R Scan Length SP steps" class="DigNum (strict)"("Minimum"=w1950) -> ()  [unwired: 2 in, 2 out]
        n1025 = property on="R Scan Length SP steps" class="DigNum (strict)"("Maximum"=w1951) -> ()  [unwired: 2 in, 2 out]
        n1026 = Divide(x=w1925, y=w1983) -> (x/y=w1920:dbl)
        n1027 = Divide(x=w1927, y=w1928) -> (x/y=w1975:dbl)
        n1028 = Divide(x=w1934, y=w1957) -> (x/y=w1962:dbl)
        n1029 = Divide(x=w1932, y=w1943) -> (x/y=w1948:dbl)
        n1030 = To Double Precision Float(number=w1986) -> (double precision float=w1924:dbl)
        n1031 = To Double Precision Float(number=w1970) -> (double precision float=w1926:dbl)
        n1032 = To Double Precision Float(number=w1956) -> (double precision float=w1933:dbl)
        n1033 = To Double Precision Float(number=w1942) -> (double precision float=w1931:dbl)
        n1034 = property on="X mm/rev" class="DigNum (strict)"() -> ("Value"=w1919:dbl)  [unwired: 2 in, 2 out]
        n1035 = property on="Y mm/rev" class="DigNum (strict)"() -> ("Value"=w1972:dbl)  [unwired: 2 in, 2 out]
        n1036 = property on="Z mm/rev" class="DigNum (strict)"() -> ("Value"=w1959:dbl)  [unwired: 2 in, 2 out]
        n1037 = property on="R deg/rev" class="DigNum (strict)"() -> ("Value"=w1945:dbl)  [unwired: 2 in, 2 out]
        n1038 = Multiply(x=w1920, y=w1919) -> (x*y=w1980:dbl)
        n1039 = Divide(x=w1924, y=w1983) -> (x/y=w1918:dbl)
        n1040 = Multiply(x=w1975, y=w1972) -> (x*y=w1968:dbl)
        n1041 = Divide(x=w1926, y=w1928) -> (x/y=w1969:dbl)
        n1042 = Divide(x=w1932, y=w1931) -> (x/y=w1930:dbl)
        n1043 = Multiply(x=w1948, y=w1945) -> (x*y=w1940:dbl)
        n1044 = Divide(x=w1931, y=w1943) -> (x/y=w1941:dbl)
        n1045 = Multiply(x=w1962, y=w1959) -> (x*y=w1954:dbl)
        n1046 = Divide(x=w1934, y=w1933) -> (x/y=w1929:dbl)
        n1047 = Divide(x=w1933, y=w1957) -> (x/y=w1955:dbl)
        n1048 = case shown="True" w1912 {
          tunnel: w1925 -> [w1993 _]
          tunnel: w1924 -> [w1992 _]
          frame False {
            n1049 = Divide(x=w1993, y=w1992) -> (x/y=w1994:dbl)
            n1050 = Absolute Value(x=w1994) -> (abs(x)=→"X Scan Duration":dbl)
          }
          frame True {
            n1051 = local write "X Scan Duration"(0.0 ("X Scan Duration")) -> ()
          }
        }
        n1052 = case shown="True" w1913 {
          tunnel: w1927 -> [w1999 _]
          tunnel: w1926 -> [w1998 _]
          frame False {
            n1053 = Divide(x=w1999, y=w1998) -> (x/y=w1997:dbl)
            n1054 = Absolute Value(x=w1997) -> (abs(x)=→"Y Scan Duration":dbl)
          }
          frame True {
            n1055 = local write "Y Scan Duration"(0.0 ("Y Scan Duration")) -> ()
          }
        }
        n1056 = Multiply(x=w1919, y=w1918) -> (x*y=w1981:dbl)
        n1057 = Multiply(x=w1972, y=w1969) -> (x*y=w1967:dbl)
        n1058 = Multiply(x=w1945, y=w1941) -> (x*y=w1939:dbl)
        n1059 = Multiply(x=w1959, y=w1955) -> (x*y=w1953:dbl)
        n1060 = Absolute Value(x=w1930) -> (abs(x)=→"R Scan Duration":dbl)
        n1061 = Absolute Value(x=w1929) -> (abs(x)=→"Z Scan Duration":dbl)
        n1062 = property on="X Scan length MV mm" class="DigNum (strict)"("Val(Sgnl)"=w1980) -> ()  [unwired: 2 in, 2 out]
        n1063 = property on="Y Scan length MV mm" class="DigNum (strict)"("Value"=w1968) -> ()  [unwired: 2 in, 2 out]
        n1064 = property on="R Scan length MV deg" class="DigNum (strict)"("Value"=w1940) -> ()  [unwired: 2 in, 2 out]
        n1065 = property on="Z Scan length MV mm" class="DigNum (strict)"("Value"=w1954) -> ()  [unwired: 2 in, 2 out]
        n1066 = Absolute Value(x=w1939) -> (abs(x)=w1923:dbl)
        n1067 = property on="X Scan velocity MV mm/sec" class="DigNum (strict)"("Value"=w1981) -> ()  [unwired: 2 in, 2 out]
        n1068 = property on="Y Scan velocity MV mm/sec" class="DigNum (strict)"("Val(Sgnl)"=w1967) -> ()  [unwired: 2 in, 2 out]
        n1069 = property on="Z Scan velocity MV mm/sec" class="DigNum (strict)"("Val(Sgnl)"=w1953) -> ()  [unwired: 2 in, 2 out]
        n1070 = property on="R Scan Velocity SP deg/sec" class="DigNum (strict)"("Val(Sgnl)"=w1923) -> ()  [unwired: 2 in, 2 out]
      }
      event "Y Move Set": Mouse Down {
        n1071 = event-data() -> ()  [unwired: 1 in, 7 out]
        n1072 = property on="Y steps/rev" class="DigNum (strict)"() -> ("Value"=w2019:u32)  [unwired: 2 in, 2 out]
        n1073 = Wait (ms)(milliseconds to wait=u32 100) -> ()  [unwired: 1 out]
        n1074 = To Double Precision Float(number=w2019) -> (double precision float=w2004:dbl)
        n1075 = property on="Y offset mm" class="DigNum (strict)"() -> ("Value"=w2017:dbl)  [unwired: 2 in, 2 out]
        n1076 = property on="Y Position SP mm" class="DigNum (strict)"() -> ("Value"=w2016:dbl)  [unwired: 2 in, 2 out]
        n1077 = local write "STATUS"("SETTING Y" ("STATUS")) -> ()
        n1078 = property on="Y Velocity SP step/sec" class="DigNum (strict)"() -> ("Maximum"=w2006:dbl)  [unwired: 2 in, 2 out]
        n1079 = property on="Y Velocity SP step/sec" class="DigNum (strict)"() -> ("Minimum"=w2005:dbl)  [unwired: 2 in, 2 out]
        n1080 = Subtract(x=w2016, y=w2017) -> (x-y=w2020:dbl)
        n1081 = property on="Y Velocity SP mm/sec" class="DigNum (strict)"() -> ("Value"=w2010:dbl)  [unwired: 2 in, 2 out]
        n1082 = property on="Y mm/rev" class="DigNum (strict)"() -> ("Value"=w2003:dbl)  [unwired: 2 in, 2 out]
        n1083 = Divide(x=w2020, y=w2003) -> (x/y=w2021:dbl)
        n1084 = Divide(x=w2010, y=w2003) -> (x/y=w2011:dbl)
        n1085 = Multiply(x=w2021, y=w2004) -> (x*y=w2015:dbl)
        n1086 = Multiply(x=w2011, y=w2004) -> (x*y=w2008:dbl)
        n1087 = In Range and Coerce(upper limit=w2006, x=w2008, lower limit=w2005) -> (coerced(x)=w2007:dbl)  [unwired: 1 out]
        n1088 = property on="Y Step SP" class="DigNum (strict)"() -> ("Maximum"=w2013:dbl)  [unwired: 2 in, 2 out]
        n1089 = property on="Y Step SP" class="DigNum (strict)"() -> ("Minimum"=w2012:dbl)  [unwired: 2 in, 2 out]
        n1090 = To Long Integer(number=w2007) -> (32bit integer=w2009:i32)
        n1091 = In Range and Coerce(upper limit=w2013, x=w2015, lower limit=w2012) -> (coerced(x)=w2014:dbl)  [unwired: 1 out]
        n1092 = To Long Integer(number=w2014) -> (32bit integer=w2018:i32)
        n1093 = property on="Y Velocity SP step/sec" class="DigNum (strict)"("Val(Sgnl)"=w2009) -> ()  [unwired: 2 in, 2 out]
        n1094 = property on="Y Step SP" class="DigNum (strict)"("Val(Sgnl)"=w2018) -> ()  [unwired: 2 in, 2 out]
      }
      event "X Move Set": Mouse Down {
        n1095 = event-data() -> ()  [unwired: 1 in, 7 out]
        n1096 = property on="X steps/rev" class="DigNum (strict)"() -> ("Value"=w2040:u32)  [unwired: 2 in, 2 out]
        n1097 = Wait (ms)(milliseconds to wait=u32 100) -> ()  [unwired: 1 out]
        n1098 = property on="X offset mm" class="DigNum (strict)"() -> ("Value"=w2038:dbl)  [unwired: 2 in, 2 out]
        n1099 = property on="X Position SP mm" class="DigNum (strict)"() -> ("Value"=w2037:dbl)  [unwired: 2 in, 2 out]
        n1100 = local write "STATUS"("SETTING X" ("STATUS")) -> ()
        n1101 = property on="X Velocity SP step/sec" class="DigNum (strict)"() -> ("Maximum"=w2027:dbl)  [unwired: 2 in, 2 out]
        n1102 = property on="X Velocity SP step/sec" class="DigNum (strict)"() -> ("Minimum"=w2026:dbl)  [unwired: 2 in, 2 out]
        n1103 = Subtract(x=w2037, y=w2038) -> (x-y=w2041:dbl)
        n1104 = property on="X Velocity SP mm/sec" class="DigNum (strict)"() -> ("Value"=w2031:dbl)  [unwired: 2 in, 2 out]
        n1105 = property on="X mm/rev" class="DigNum (strict)"() -> ("Value"=w2024:dbl)  [unwired: 2 in, 2 out]
        n1106 = Divide(x=w2041, y=w2024) -> (x/y=w2042:dbl)
        n1107 = Divide(x=w2031, y=w2024) -> (x/y=w2032:dbl)
        n1108 = To Double Precision Float(number=w2040) -> (double precision float=w2025:dbl)
        n1109 = Multiply(x=w2042, y=w2025) -> (x*y=w2036:dbl)
        n1110 = Multiply(x=w2032, y=w2025) -> (x*y=w2029:dbl)
        n1111 = In Range and Coerce(upper limit=w2027, x=w2029, lower limit=w2026) -> (coerced(x)=w2028:dbl)  [unwired: 1 out]
        n1112 = property on="X Step SP" class="DigNum (strict)"() -> ("Maximum"=w2034:dbl)  [unwired: 2 in, 2 out]
        n1113 = property on="X Step SP" class="DigNum (strict)"() -> ("Minimum"=w2033:dbl)  [unwired: 2 in, 2 out]
        n1114 = To Long Integer(number=w2028) -> (32bit integer=w2030:i32)
        n1115 = In Range and Coerce(upper limit=w2034, x=w2036, lower limit=w2033) -> (coerced(x)=w2035:dbl)  [unwired: 1 out]
        n1116 = To Long Integer(number=w2035) -> (32bit integer=w2039:i32)
        n1117 = property on="X Velocity SP step/sec" class="DigNum (strict)"("Val(Sgnl)"=w2030) -> ()  [unwired: 2 in, 2 out]
        n1118 = property on="X Step SP" class="DigNum (strict)"("Val(Sgnl)"=w2039) -> ()  [unwired: 2 in, 2 out]
      }
      event "Z Move Set": Mouse Down {
        n1119 = event-data() -> ()  [unwired: 1 in, 7 out]
        n1120 = property on="Z steps/rev" class="DigNum (strict)"() -> ("Value"=w2059:u32)  [unwired: 2 in, 2 out]
        n1121 = Wait (ms)(milliseconds to wait=u32 100) -> ()  [unwired: 1 out]
        n1122 = property on="Z offset mm" class="DigNum (strict)"() -> ("Value"=w2057:dbl)  [unwired: 2 in, 2 out]
        n1123 = property on="Z Position SP mm" class="DigNum (strict)"() -> ("Value"=w2056:dbl)  [unwired: 2 in, 2 out]
        n1124 = local write "STATUS"("SETTING Z" ("STATUS")) -> ()
        n1125 = property on="Z Velocity SP step/sec" class="DigNum (strict)"() -> ("Maximum"=w2046:dbl)  [unwired: 2 in, 2 out]
        n1126 = property on="Z Velocity SP step/sec" class="DigNum (strict)"() -> ("Minimum"=w2045:dbl)  [unwired: 2 in, 2 out]
        n1127 = Subtract(x=w2056, y=w2057) -> (x-y=w2060:dbl)
        n1128 = property on="Z Velocity SP mm/sec" class="DigNum (strict)"() -> ("Value"=w2050:dbl)  [unwired: 2 in, 2 out]
        n1129 = property on="Z mm/rev" class="DigNum (strict)"() -> ("Value"=w2062:dbl)  [unwired: 2 in, 2 out]
        n1130 = Divide(x=w2060, y=w2062) -> (x/y=w2061:dbl)
        n1131 = Divide(x=w2050, y=w2062) -> (x/y=w2051:dbl)
        n1132 = To Double Precision Float(number=w2059) -> (double precision float=w2063:dbl)
        n1133 = Multiply(x=w2061, y=w2063) -> (x*y=w2055:dbl)
        n1134 = Multiply(x=w2051, y=w2063) -> (x*y=w2048:dbl)
        n1135 = In Range and Coerce(upper limit=w2046, x=w2048, lower limit=w2045) -> (coerced(x)=w2047:dbl)  [unwired: 1 out]
        n1136 = property on="Z Step SP" class="DigNum (strict)"() -> ("Maximum"=w2053:dbl)  [unwired: 2 in, 2 out]
        n1137 = property on="Z Step SP" class="DigNum (strict)"() -> ("Minimum"=w2052:dbl)  [unwired: 2 in, 2 out]
        n1138 = To Long Integer(number=w2047) -> (32bit integer=w2049:i32)
        n1139 = In Range and Coerce(upper limit=w2053, x=w2055, lower limit=w2052) -> (coerced(x)=w2054:dbl)  [unwired: 1 out]
        n1140 = To Long Integer(number=w2054) -> (32bit integer=w2058:i32)
        n1141 = property on="Z Velocity SP step/sec" class="DigNum (strict)"("Val(Sgnl)"=w2049) -> ()  [unwired: 2 in, 2 out]
        n1142 = property on="Z Step SP" class="DigNum (strict)"("Val(Sgnl)"=w2058) -> ()  [unwired: 2 in, 2 out]
      }
      event "R Move Set": Mouse Down {
        n1143 = event-data() -> ()  [unwired: 1 in, 7 out]
        n1144 = property on="R steps/rev" class="DigNum (strict)"() -> ("Value"=w2083:u32)  [unwired: 2 in, 2 out]
        n1145 = Wait (ms)(milliseconds to wait=u32 100) -> ()  [unwired: 1 out]
        n1146 = property on="R offset deg" class="DigNum (strict)"() -> ("Value"=w2081:dbl)  [unwired: 2 in, 2 out]
        n1147 = property on="R Position SP deg" class="DigNum (strict)"() -> ("Value"=w2080:dbl)  [unwired: 2 in, 2 out]
        n1148 = local write "STATUS"("SETTING R" ("STATUS")) -> ()
        n1149 = property on="R Velocity SP step/sec" class="DigNum (strict)"() -> ("Maximum"=w2070:dbl)  [unwired: 2 in, 2 out]
        n1150 = property on="R Velocity SP step/sec" class="DigNum (strict)"() -> ("Minimum"=w2069:dbl)  [unwired: 2 in, 2 out]
        n1151 = Subtract(x=w2080, y=w2081) -> (x-y=w2084:dbl)
        n1152 = property on="R Velocity SP deg/sec" class="DigNum (strict)"() -> ("Value"=w2074:dbl)  [unwired: 2 in, 2 out]
        n1153 = property on="R deg/rev" class="DigNum (strict)"() -> ("Value"=w2067:dbl)  [unwired: 2 in, 2 out]
        n1154 = Divide(x=w2084, y=w2067) -> (x/y=w2085:dbl)
        n1155 = Divide(x=w2074, y=w2067) -> (x/y=w2075:dbl)
        n1156 = To Double Precision Float(number=w2083) -> (double precision float=w2068:dbl)
        n1157 = Multiply(x=w2085, y=w2068) -> (x*y=w2079:dbl)
        n1158 = Multiply(x=w2075, y=w2068) -> (x*y=w2072:dbl)
        n1159 = property on="R Step SP" class="DigNum (strict)"() -> ("Maximum"=w2077:dbl)  [unwired: 2 in, 2 out]
        n1160 = property on="R Step SP" class="DigNum (strict)"() -> ("Minimum"=w2076:dbl)  [unwired: 2 in, 2 out]
        n1161 = Absolute Value(x=w2072) -> (abs(x)=w2066:dbl)
        n1162 = In Range and Coerce(upper limit=w2077, x=w2079, lower limit=w2076) -> (coerced(x)=w2078:dbl)  [unwired: 1 out]
        n1163 = In Range and Coerce(upper limit=w2070, x=w2066, lower limit=w2069) -> (coerced(x)=w2071:dbl)  [unwired: 1 out]
        n1164 = To Long Integer(number=w2078) -> (32bit integer=w2082:i32)
        n1165 = To Long Integer(number=w2071) -> (32bit integer=w2073:i32)
        n1166 = property on="R Step SP" class="DigNum (strict)"("Val(Sgnl)"=w2082) -> ()  [unwired: 2 in, 2 out]
        n1167 = property on="R Velocity SP step/sec" class="DigNum (strict)"("Val(Sgnl)"=w2073) -> ()  [unwired: 2 in, 2 out]
      }
      event "Set Scan \nParameters": Mouse Down {
        n1168 = event-data() -> ()  [unwired: 1 in, 7 out]
        n1169 = flat-sequence {
          frame #0 {
            n1170 = property on="Z steps/rev" class="DigNum (strict)"() -> ("Value"=w2154:u32)  [unwired: 2 in, 2 out]
            n1171 = property on="X steps/rev" class="DigNum (strict)"() -> ("Value"=w2137:u32)  [unwired: 2 in, 2 out]
            n1172 = property on="Y steps/rev" class="DigNum (strict)"() -> ("Value"=w2102:u32)  [unwired: 2 in, 2 out]
            n1173 = property on="R steps/rev" class="DigNum (strict)"() -> ("Value"=w2120:u32)  [unwired: 2 in, 2 out]
            n1174 = To Double Precision Float(number=w2154) -> (double precision float=w2140:dbl)
            n1175 = To Double Precision Float(number=w2137) -> (double precision float=w2123:dbl)
            n1176 = To Double Precision Float(number=w2102) -> (double precision float=w2088:dbl)
            n1177 = To Double Precision Float(number=w2120) -> (double precision float=w2106:dbl)
            n1178 = property on="R Velocity SP step/sec" class="DigNum (strict)"() -> ("Maximum"=w2108:dbl)  [unwired: 2 in, 2 out]
            n1179 = property on="Z mm/rev" class="DigNum (strict)"() -> ("Value"=w2139:dbl)  [unwired: 2 in, 2 out]
            n1180 = property on="X mm/rev" class="DigNum (strict)"() -> ("Value"=w2122:dbl)  [unwired: 2 in, 2 out]
            n1181 = property on="Y mm/rev" class="DigNum (strict)"() -> ("Value"=w2087:dbl)  [unwired: 2 in, 2 out]
            n1182 = property on="Z Scan Length SP mm" class="DigNum (strict)"() -> ("Value"=w2152:dbl)  [unwired: 2 in, 2 out]
            n1183 = property on="Z Scan Velocity SP mm/sec" class="DigNum (strict)"() -> ("Value"=w2146:dbl)  [unwired: 2 in, 2 out]
            n1184 = property on="X Scan Length SP mm" class="DigNum (strict)"() -> ("Value"=w2135:dbl)  [unwired: 2 in, 2 out]
            n1185 = property on="X Scan Velocity SP mm/sec" class="DigNum (strict)"() -> ("Value"=w2129:dbl)  [unwired: 2 in, 2 out]
            n1186 = property on="Y Scan Length SP mm" class="DigNum (strict)"() -> ("Value"=w2100:dbl)  [unwired: 2 in, 2 out]
            n1187 = property on="Y Scan Velocity SP mm/sec" class="DigNum (strict)"() -> ("Value"=w2094:dbl)  [unwired: 2 in, 2 out]
            n1188 = property on="R Scan Length SP deg" class="DigNum (strict)"() -> ("Value"=w2118:dbl)  [unwired: 2 in, 2 out]
            n1189 = property on="R deg/rev" class="DigNum (strict)"() -> ("Value"=w2105:dbl)  [unwired: 2 in, 2 out]
            n1190 = property on="Z Scan Velocity SP steps/sec" class="DigNum (strict)"() -> ("Maximum"=w2142:dbl)  [unwired: 2 in, 2 out]
            n1191 = property on="X Scan Velocity SP steps/sec" class="DigNum (strict)"() -> ("Maximum"=w2125:dbl)  [unwired: 2 in, 2 out]
            n1192 = property on="Y Scan Velocity SP steps/sec" class="DigNum (strict)"() -> ("Maximum"=w2090:dbl)  [unwired: 2 in, 2 out]
            n1193 = property on="R Scan Velocity SP steps/sec" class="DigNum (strict)"() -> ("Minimum"=w2107:dbl)  [unwired: 2 in, 2 out]
            n1194 = property on="Z Scan Velocity SP steps/sec" class="DigNum (strict)"() -> ("Minimum"=w2141:dbl)  [unwired: 2 in, 2 out]
            n1195 = property on="X Scan Velocity SP steps/sec" class="DigNum (strict)"() -> ("Minimum"=w2124:dbl)  [unwired: 2 in, 2 out]
            n1196 = property on="Y Scan Velocity SP steps/sec" class="DigNum (strict)"() -> ("Minimum"=w2089:dbl)  [unwired: 2 in, 2 out]
            n1197 = property on="R Scan Velocity SP deg/sec" class="DigNum (strict)"() -> ("Value"=w2112:dbl)  [unwired: 2 in, 2 out]
            n1198 = Divide(x=w2152, y=w2139) -> (x/y=w2155:dbl)
            n1199 = Divide(x=w2146, y=w2139) -> (x/y=w2147:dbl)
            n1200 = Divide(x=w2135, y=w2122) -> (x/y=w2138:dbl)
            n1201 = Divide(x=w2129, y=w2122) -> (x/y=w2130:dbl)
            n1202 = Divide(x=w2100, y=w2087) -> (x/y=w2103:dbl)
            n1203 = Divide(x=w2094, y=w2087) -> (x/y=w2095:dbl)
            n1204 = Divide(x=w2118, y=w2105) -> (x/y=w2121:dbl)
            n1205 = Multiply(x=w2155, y=w2140) -> (x*y=w2151:dbl)
            n1206 = Multiply(x=w2147, y=w2140) -> (x*y=w2144:dbl)
            n1207 = Multiply(x=w2138, y=w2123) -> (x*y=w2134:dbl)
            n1208 = Multiply(x=w2130, y=w2123) -> (x*y=w2127:dbl)
            n1209 = Multiply(x=w2103, y=w2088) -> (x*y=w2099:dbl)
            n1210 = Multiply(x=w2095, y=w2088) -> (x*y=w2092:dbl)
            n1211 = Multiply(x=w2121, y=w2106) -> (x*y=w2117:dbl)
            n1212 = Divide(x=w2112, y=w2105) -> (x/y=w2113:dbl)
            n1213 = property on="Z Step SP" class="DigNum (strict)"() -> ("Maximum"=w2148:dbl)  [unwired: 2 in, 2 out]
            n1214 = property on="X Step SP" class="DigNum (strict)"() -> ("Maximum"=w2131:dbl)  [unwired: 2 in, 2 out]
            n1215 = property on="Y Step SP" class="DigNum (strict)"() -> ("Maximum"=w2096:dbl)  [unwired: 2 in, 2 out]
            n1216 = property on="R Step SP" class="DigNum (strict)"() -> ("Maximum"=w2114:dbl)  [unwired: 2 in, 2 out]
            n1217 = property on="Z Step SP" class="DigNum (strict)"() -> ("Minimum"=w2149:dbl)  [unwired: 2 in, 2 out]
            n1218 = property on="X Step SP" class="DigNum (strict)"() -> ("Minimum"=w2132:dbl)  [unwired: 2 in, 2 out]
            n1219 = property on="Y Step SP" class="DigNum (strict)"() -> ("Minimum"=w2097:dbl)  [unwired: 2 in, 2 out]
            n1220 = property on="R Step SP" class="DigNum (strict)"() -> ("Minimum"=w2115:dbl)  [unwired: 2 in, 2 out]
            n1221 = Multiply(x=w2113, y=w2106) -> (x*y=w2110:dbl)
            n1222 = In Range and Coerce(upper limit=w2142, x=w2144, lower limit=w2141) -> (coerced(x)=w2143:dbl)  [unwired: 1 out]
            n1223 = In Range and Coerce(upper limit=w2125, x=w2127, lower limit=w2124) -> (coerced(x)=w2126:dbl)  [unwired: 1 out]
            n1224 = In Range and Coerce(upper limit=w2090, x=w2092, lower limit=w2089) -> (coerced(x)=w2091:dbl)  [unwired: 1 out]
            n1225 = To Long Integer(number=w2143) -> (32bit integer=w2145:i32)
            n1226 = To Long Integer(number=w2126) -> (32bit integer=w2128:i32)
            n1227 = To Long Integer(number=w2091) -> (32bit integer=w2093:i32)
            n1228 = Absolute Value(x=w2110) -> (abs(x)=w2104:dbl)
            n1229 = In Range and Coerce(upper limit=w2148, x=w2151, lower limit=w2149) -> (coerced(x)=w2150:dbl)  [unwired: 1 out]
            n1230 = In Range and Coerce(upper limit=w2131, x=w2134, lower limit=w2132) -> (coerced(x)=w2133:dbl)  [unwired: 1 out]
            n1231 = In Range and Coerce(upper limit=w2096, x=w2099, lower limit=w2097) -> (coerced(x)=w2098:dbl)  [unwired: 1 out]
            n1232 = In Range and Coerce(upper limit=w2114, x=w2117, lower limit=w2115) -> (coerced(x)=w2116:dbl)  [unwired: 1 out]
            n1233 = To Long Integer(number=w2150) -> (32bit integer=w2153:i32)
            n1234 = To Long Integer(number=w2133) -> (32bit integer=w2136:i32)
            n1235 = To Long Integer(number=w2098) -> (32bit integer=w2101:i32)
            n1236 = To Long Integer(number=w2116) -> (32bit integer=w2119:i32)
            n1237 = property on="Z Scan Velocity SP steps/sec" class="DigNum (strict)"("Val(Sgnl)"=w2145) -> ()  [unwired: 2 in, 2 out]
            n1238 = property on="X Scan Velocity SP steps/sec" class="DigNum (strict)"("Val(Sgnl)"=w2128) -> ()  [unwired: 2 in, 2 out]
            n1239 = property on="Y Scan Velocity SP steps/sec" class="DigNum (strict)"("Val(Sgnl)"=w2093) -> ()  [unwired: 2 in, 2 out]
            n1240 = In Range and Coerce(upper limit=w2108, x=w2104, lower limit=w2107) -> (coerced(x)=w2109:dbl)  [unwired: 1 out]
            n1241 = To Long Integer(number=w2109) -> (32bit integer=w2111:i32)
            n1242 = property on="Z Scan Length SP steps" class="DigNum (strict)"("Val(Sgnl)"=w2153) -> ()  [unwired: 2 in, 2 out]
            n1243 = property on="X Scan Length SP steps" class="DigNum (strict)"("Val(Sgnl)"=w2136) -> ()  [unwired: 2 in, 2 out]
            n1244 = property on="Y Scan Length SP steps" class="DigNum (strict)"("Val(Sgnl)"=w2101) -> ()  [unwired: 2 in, 2 out]
            n1245 = property on="R Scan Length SP steps" class="DigNum (strict)"("Val(Sgnl)"=w2119) -> ()  [unwired: 2 in, 2 out]
            n1246 = property on="R Scan Velocity SP steps/sec" class="DigNum (strict)"("Val(Sgnl)"=w2111) -> ()  [unwired: 2 in, 2 out]
          }
          frame #1 {
            n1247 = case shown="True" "Z as dominating length" {
              frame False {
              }
              frame True {
                n1248 = property on="Y Scan Length SP steps" class="DigNum (strict)"() -> ("Value"=w2165:i32)  [unwired: 2 in, 2 out]
                n1249 = property on="Z Scan Length SP steps" class="DigNum (strict)"() -> ("Value"=w2164:i32)  [unwired: 2 in, 2 out]
                n1250 = property on="X Scan Length SP steps" class="DigNum (strict)"() -> ("Value"=w2173:i32)  [unwired: 2 in, 2 out]
                n1251 = property on="Z Scan Length SP steps" class="DigNum (strict)"() -> ("Value"=w2172:i32)  [unwired: 2 in, 2 out]
                n1252 = property on="Y Scan Velocity SP steps/sec" class="DigNum (strict)"() -> ("Value"=w2161:i32)  [unwired: 2 in, 2 out]
                n1253 = property on="X Scan Velocity SP steps/sec" class="DigNum (strict)"() -> ("Value"=w2171:i32)  [unwired: 2 in, 2 out]
                n1254 = To Double Precision Float(number=w2165) -> (double precision float=w2163:dbl)
                n1255 = To Double Precision Float(number=w2164) -> (double precision float=w2162:dbl)
                n1256 = To Double Precision Float(number=w2173) -> (double precision float=w2167:dbl)
                n1257 = To Double Precision Float(number=w2172) -> (double precision float=w2168:dbl)
                n1258 = Divide(x=w2163, y=w2162) -> (x/y=w2157:dbl)
                n1259 = Divide(x=w2167, y=w2168) -> (x/y=w2174:dbl)
                n1260 = To Double Precision Float(number=w2161) -> (double precision float=w2160:dbl)
                n1261 = To Double Precision Float(number=w2171) -> (double precision float=w2169:dbl)
                n1262 = Multiply(x=w2157, y=w2160) -> (x*y=w2159:dbl)
                n1263 = Multiply(x=w2174, y=w2169) -> (x*y=w2170:dbl)
                n1264 = To Long Integer(number=w2159) -> (32bit integer=w2158:i32)
                n1265 = To Long Integer(number=w2170) -> (32bit integer=w2166:i32)
                n1266 = property on="Y Scan Velocity SP steps/sec" class="DigNum (strict)"("Val(Sgnl)"=w2158) -> ()  [unwired: 2 in, 2 out]
                n1267 = property on="X Scan Velocity SP steps/sec" class="DigNum (strict)"("Val(Sgnl)"=w2166) -> ()  [unwired: 2 in, 2 out]
              }
            }
          }
          frame #2 {
            w2175 = T9."Enabled" ("Disabled")
            n1268 = property on="Send scan parameter" class="Bool"("DisabledEnum"=w2175) -> ()  [unwired: 2 in, 2 out]
            n1269 = property on="LOOP" class="Bool (strict)"("DisabledEnum"=w2175) -> ()  [unwired: 2 in, 2 out]
          }
        }
        n1270 = local write "STATUS"("SCANNING PARAMETERS SET" ("STATUS")) -> ()
      }
      event "Send scan parameter": Mouse Up {
        n1271 = event-data() -> ()  [unwired: 1 in, 7 out]
        n1272 = local write "STATUS"("READY TO SCAN" ("STATUS")) -> ()
        n1273 = flat-sequence {
          tunnel: [w2229] -> w2189
          tunnel: [w2228] -> w2188
          tunnel: w2179 -> [w2227]
          tunnel: w2178 -> [w2226]
          tunnel: w2189 -> [w2235]
          tunnel: [w2235] -> w2187
          tunnel: w2188 -> [w2234]
          tunnel: [w2234] -> w2186
          tunnel: w2187 -> [w2241]
          tunnel: [w2240] -> w2185
          tunnel: w2186 -> [w2239]
          tunnel: [w2238] -> w2184
          tunnel: w2185 -> [w2247]
          tunnel: w2184 -> [w2246]
          tunnel: [w2247] -> w2183
          tunnel: [w2246] -> w2182
          tunnel: w2183 -> [w2252]
          tunnel: w2182 -> [w2251]
          tunnel: [w2252] -> w2181
          tunnel: [w2251] -> w2180
          tunnel: [w2254] -> _
          tunnel: [w2255] -> _
          tunnel: w2181 -> [w2255]
          tunnel: w2180 -> [w2254]
          frame #0 {
            n1274 = property on="R Scan Velocity SP steps/sec" class="DigNum (strict)"() -> ("Value"=w2231:i32)  [unwired: 2 in, 2 out]
            n1275 = Number To Decimal String(number=w2231) -> (decimal integer string=w2232:string)  [unwired: 1 in]
            n1276 = call "mDrive Send Command.vi"("error in (no error)"=w2227, "Extra"=w2232, "Command"=T10."Max Velocity", "VISA resource name"=w2226) -> ("error out"=w2228:errorcluster, "VISA resource name out"=w2229:refnum<visa-resource-name>)  [unwired: 3 in, 1 out]
          }
          frame #1 {
            n1277 = Wait (ms)(milliseconds to wait=u32 100) -> ()  [unwired: 1 out]
          }
          frame #2 {
            # "VELOCITY"
            n1278 = call "mdrive send command.vi"("error in (no error)"=w2239, "Extra"="VM", "Command"=T10."Print Parameter", "VISA resource name"=w2241) -> ("error out"=w2238:errorcluster, "read buffer"=w2243:string, "VISA resource name out"=w2240:refnum<visa-resource-name>)  [unwired: 3 in]
            n1279 = Decimal String To Number(string=w2243, offset=0) -> (number=w2242:i32)  [unwired: 1 in, 1 out]
            n1280 = property on="R velocity PV step/sec" class="DigNum (strict)"("Val(Sgnl)"=w2242) -> ()  [unwired: 2 in, 2 out]
          }
          frame #3 {
            n1281 = Wait (ms)(milliseconds to wait=u32 100) -> ()  [unwired: 1 out]
          }
          frame #4 {
            n1282 = property on="Scan Go" class="Bool (strict)"("DisabledEnum"=T9."Enabled" ("Disabled")) -> ()  [unwired: 2 in, 2 out]
            n1283 = property on="R Scan Velocity SP steps/sec" class="DigNum (strict)"("DisabledEnum"=T9."Disabled and Grayed Out" ("Disabled")) -> ()  [unwired: 2 in, 2 out]
            n1284 = property on="R Scan Length SP steps" class="DigNum (strict)"("DisabledEnum"=T9."Disabled and Grayed Out" ("Disabled")) -> ()  [unwired: 2 in, 2 out]
          }
          frame #5 {
            n1285 = property on="R Scan" class="Bool (strict)"("Val(Sgnl)"=TRUE ("Slew Ready 2")) -> ()  [unwired: 2 in, 2 out]
          }
        }
        n1286 = flat-sequence {
          tunnel: [w2289] -> w2213
          tunnel: [w2288] -> w2212
          tunnel: w2203 -> [w2287]
          tunnel: w2202 -> [w2286]
          tunnel: w2213 -> [w2295]
          tunnel: [w2295] -> w2211
          tunnel: w2212 -> [w2294]
          tunnel: [w2294] -> w2210
          tunnel: w2211 -> [w2299]
          tunnel: [w2298] -> w2209
          tunnel: w2210 -> [w2297]
          tunnel: [w2296] -> w2208
          tunnel: w2209 -> [w2307]
          tunnel: [w2307] -> w2207
          tunnel: w2208 -> [w2306]
          tunnel: [w2306] -> w2206
          tunnel: w2207 -> [w2312]
          tunnel: w2206 -> [w2311]
          tunnel: [w2312] -> w2205
          tunnel: [w2311] -> w2204
          tunnel: [w2314] -> _
          tunnel: [w2315] -> _
          tunnel: w2205 -> [w2315]
          tunnel: w2204 -> [w2314]
          frame #0 {
            n1287 = property on="Y Scan Velocity SP steps/sec" class="DigNum (strict)"() -> ("Value"=w2291:i32)  [unwired: 2 in, 2 out]
            n1288 = Number To Decimal String(number=w2291) -> (decimal integer string=w2292:string)  [unwired: 1 in]
            n1289 = call "mdrive send command.vi"("error in (no error)"=w2287, "Extra"=w2292, "Command"=T10."Max Velocity", "VISA resource name"=w2286) -> ("error out"=w2288:errorcluster, "VISA resource name out"=w2289:refnum<visa-resource-name>)  [unwired: 3 in, 1 out]
          }
          frame #1 {
            n1290 = Wait (ms)(milliseconds to wait=u32 100) -> ()  [unwired: 1 out]
          }
          frame #2 {
            # "VELOCITY"
            n1291 = call "mdrive send command.vi"("error in (no error)"=w2297, "Extra"="VM", "Command"=T10."Print Parameter", "VISA resource name"=w2299) -> ("error out"=w2296:errorcluster, "read buffer"=w2303:string, "VISA resource name out"=w2298:refnum<visa-resource-name>)  [unwired: 3 in]
            n1292 = Decimal String To Number(string=w2303, offset=0) -> (number=w2301:i32)  [unwired: 1 in, 1 out]
            n1293 = property on="Y velocity PV step/sec" class="DigNum (strict)"("Val(Sgnl)"=w2301) -> ()  [unwired: 2 in, 2 out]
          }
          frame #3 {
            n1294 = Wait (ms)(milliseconds to wait=u32 100) -> ()  [unwired: 1 out]
          }
          frame #4 {
            n1295 = property on="Scan Go" class="Bool (strict)"("DisabledEnum"=T9."Enabled" ("Disabled")) -> ()  [unwired: 2 in, 2 out]
            n1296 = property on="Y Scan Velocity SP steps/sec" class="DigNum (strict)"("DisabledEnum"=T9."Disabled and Grayed Out" ("Disabled")) -> ()  [unwired: 2 in, 2 out]
            n1297 = property on="Y Scan Length SP steps" class="DigNum (strict)"("DisabledEnum"=T9."Disabled and Grayed Out" ("Disabled")) -> ()  [unwired: 2 in, 2 out]
          }
          frame #5 {
            n1298 = property on="Y Scan" class="Bool (strict)"("Val(Sgnl)"=TRUE ("Slew Ready 2")) -> ()  [unwired: 2 in, 2 out]
          }
        }
        n1299 = flat-sequence {
          tunnel: [w2317] -> w2217
          tunnel: [w2316] -> w2215
          tunnel: w2223 -> [w2319]
          tunnel: w2222 -> [w2318]
          tunnel: w2217 -> [w2325]
          tunnel: [w2325] -> w2216
          tunnel: w2215 -> [w2324]
          tunnel: [w2324] -> w2214
          tunnel: w2216 -> [w2329]
          tunnel: [w2328] -> w2219
          tunnel: w2214 -> [w2327]
          tunnel: [w2326] -> w2218
          tunnel: w2219 -> [w2337]
          tunnel: [w2337] -> w2221
          tunnel: w2218 -> [w2336]
          tunnel: [w2336] -> w2220
          tunnel: w2221 -> [w2342]
          tunnel: w2220 -> [w2341]
          tunnel: [w2342] -> w2225
          tunnel: [w2341] -> w2224
          tunnel: [w2344] -> _
          tunnel: [w2345] -> _
          tunnel: w2225 -> [w2345]
          tunnel: w2224 -> [w2344]
          frame #0 {
            n1300 = property on="X Scan Velocity SP steps/sec" class="DigNum (strict)"() -> ("Value"=w2321:i32)  [unwired: 2 in, 2 out]
            n1301 = Number To Decimal String(number=w2321) -> (decimal integer string=w2322:string)  [unwired: 1 in]
            n1302 = call "mdrive send command.vi"("error in (no error)"=w2319, "Extra"=w2322, "Command"=T10."Max Velocity", "VISA resource name"=w2318) -> ("error out"=w2316:errorcluster, "VISA resource name out"=w2317:refnum<visa-resource-name>)  [unwired: 3 in, 1 out]
          }
          frame #1 {
            n1303 = Wait (ms)(milliseconds to wait=u32 100) -> ()  [unwired: 1 out]
          }
          frame #2 {
            # "VELOCITY"
            n1304 = call "mdrive send command.vi"("error in (no error)"=w2327, "Extra"="VM", "Command"=T10."Print Parameter", "VISA resource name"=w2329) -> ("error out"=w2326:errorcluster, "read buffer"=w2332:string, "VISA resource name out"=w2328:refnum<visa-resource-name>)  [unwired: 3 in]
            n1305 = Decimal String To Number(string=w2332, offset=0) -> (number=w2330:i32)  [unwired: 1 in, 1 out]
            n1306 = property on="X velocity PV step/sec" class="DigNum (strict)"("Val(Sgnl)"=w2330) -> ()  [unwired: 2 in, 2 out]
          }
          frame #3 {
            n1307 = Wait (ms)(milliseconds to wait=u32 100) -> ()  [unwired: 1 out]
          }
          frame #4 {
            n1308 = property on="Scan Go" class="Bool (strict)"("DisabledEnum"=T9."Enabled" ("Disabled")) -> ()  [unwired: 2 in, 2 out]
            n1309 = property on="X Scan Velocity SP steps/sec" class="DigNum (strict)"("DisabledEnum"=T9."Disabled and Grayed Out" ("Disabled")) -> ()  [unwired: 2 in, 2 out]
            n1310 = property on="X Scan Length SP steps" class="DigNum (strict)"("DisabledEnum"=T9."Disabled and Grayed Out" ("Disabled")) -> ()  [unwired: 2 in, 2 out]
          }
          frame #5 {
            n1311 = property on="X Scan" class="Bool (strict)"("Val(Sgnl)"=TRUE ("Slew Ready 2")) -> ()  [unwired: 2 in, 2 out]
          }
        }
        n1312 = flat-sequence {
          tunnel: [w2259] -> w2201
          tunnel: [w2258] -> w2200
          tunnel: w2191 -> [w2257]
          tunnel: w2190 -> [w2256]
          tunnel: w2201 -> [w2265]
          tunnel: [w2265] -> w2199
          tunnel: w2200 -> [w2264]
          tunnel: [w2264] -> w2198
          tunnel: w2199 -> [w2271]
          tunnel: [w2270] -> w2197
          tunnel: w2198 -> [w2269]
          tunnel: [w2268] -> w2196
          tunnel: w2197 -> [w2277]
          tunnel: [w2277] -> w2195
          tunnel: w2196 -> [w2276]
          tunnel: [w2276] -> w2194
          tunnel: w2195 -> [w2282]
          tunnel: w2194 -> [w2281]
          tunnel: [w2282] -> w2193
          tunnel: [w2281] -> w2192
          tunnel: [w2284] -> _
          tunnel: [w2285] -> _
          tunnel: w2193 -> [w2285]
          tunnel: w2192 -> [w2284]
          frame #0 {
            n1313 = property on="Z Scan Velocity SP steps/sec" class="DigNum (strict)"() -> ("Value"=w2261:i32)  [unwired: 2 in, 2 out]
            n1314 = Number To Decimal String(number=w2261) -> (decimal integer string=w2262:string)  [unwired: 1 in]
            n1315 = call "mdrive send command.vi"("error in (no error)"=w2257, "Extra"=w2262, "Command"=T10."Max Velocity", "VISA resource name"=w2256) -> ("error out"=w2258:errorcluster, "VISA resource name out"=w2259:refnum<visa-resource-name>)  [unwired: 3 in, 1 out]
          }
          frame #1 {
            n1316 = Wait (ms)(milliseconds to wait=u32 100) -> ()  [unwired: 1 out]
          }
          frame #2 {
            # "VELOCITY"
            n1317 = call "mdrive send command.vi"("error in (no error)"=w2269, "Extra"="VM", "Command"=T10."Print Parameter", "VISA resource name"=w2271) -> ("error out"=w2268:errorcluster, "read buffer"=w2272:string, "VISA resource name out"=w2270:refnum<visa-resource-name>)  [unwired: 3 in]
            n1318 = Decimal String To Number(string=w2272, offset=0) -> (number=w2273:i32)  [unwired: 1 in, 1 out]
            n1319 = property on="Z  velocity PV step/sec" class="DigNum (strict)"("Val(Sgnl)"=w2273) -> ()  [unwired: 2 in, 2 out]
          }
          frame #3 {
            n1320 = Wait (ms)(milliseconds to wait=u32 100) -> ()  [unwired: 1 out]
          }
          frame #4 {
            n1321 = property on="Scan Go" class="Bool (strict)"("DisabledEnum"=T9."Enabled" ("Disabled")) -> ()  [unwired: 2 in, 2 out]
            n1322 = property on="Z Scan Velocity SP steps/sec" class="DigNum (strict)"("DisabledEnum"=T9."Disabled and Grayed Out" ("Disabled")) -> ()  [unwired: 2 in, 2 out]
            n1323 = property on="Z Scan Length SP steps" class="DigNum (strict)"("DisabledEnum"=T9."Disabled and Grayed Out" ("Disabled")) -> ()  [unwired: 2 in, 2 out]
          }
          frame #5 {
            n1324 = property on="Z Scan" class="Bool (strict)"("Val(Sgnl)"=TRUE ("Slew Ready 2")) -> ()  [unwired: 2 in, 2 out]
          }
        }
        n1325 = property on="GO" class="Bool"("DisabledEnum"=T9."Disabled and Grayed Out" ("Disabled")) -> ()  [unwired: 2 in, 2 out]
      }
      event "Scan Cancel": Mouse Down {
        n1326 = event-data() -> ()  [unwired: 1 in, 7 out]
        n1327 = flat-sequence {
          tunnel: [w2370] -> w2358
          tunnel: [w2369] -> w2357
          tunnel: w2351 -> [w2367]
          tunnel: w2349 -> [w2366]
          tunnel: [w2374] -> _
          tunnel: [w2375] -> _
          tunnel: w2358 -> [w2375]
          tunnel: w2357 -> [w2374]
          frame #0 {
            n1328 = call "mDrive Send Command.vi"("error in (no error)"=w2366, "Command"=T10."Stop", "VISA resource name"=w2367) -> ("error out"=w2369:errorcluster, "VISA resource name out"=w2370:refnum<visa-resource-name>)  [unwired: 4 in, 1 out]
          }
          frame #1 {
            n1329 = property on="R Scan" class="Bool (strict)"("Value"=FALSE ("Slew Ready")) -> ()  [unwired: 2 in, 2 out]
            n1330 = property on="R Scan Length SP steps" class="DigNum (strict)"("DisabledEnum"=T9."Enabled" ("Disabled")) -> ()  [unwired: 2 in, 2 out]
            n1331 = property on="R Scan Velocity SP steps/sec" class="DigNum (strict)"("DisabledEnum"=T9."Enabled" ("Disabled")) -> ()  [unwired: 2 in, 2 out]
          }
        }
        n1332 = flat-sequence {
          tunnel: [w2390] -> w2362
          tunnel: [w2389] -> w2361
          tunnel: w2356 -> [w2387]
          tunnel: w2354 -> [w2386]
          tunnel: [w2394] -> _
          tunnel: [w2395] -> _
          tunnel: w2362 -> [w2395]
          tunnel: w2361 -> [w2394]
          frame #0 {
            n1333 = call "mDrive Send Command.vi"("error in (no error)"=w2386, "Command"=T10."Stop", "VISA resource name"=w2387) -> ("error out"=w2389:errorcluster, "VISA resource name out"=w2390:refnum<visa-resource-name>)  [unwired: 4 in, 1 out]
          }
          frame #1 {
            n1334 = property on="X Scan" class="Bool (strict)"("Value"=FALSE ("Slew Ready")) -> ()  [unwired: 2 in, 2 out]
            n1335 = property on="X Scan Velocity SP steps/sec" class="DigNum (strict)"("DisabledEnum"=T9."Enabled" ("Disabled")) -> ()  [unwired: 2 in, 2 out]
            n1336 = property on="X Scan Length SP steps" class="DigNum (strict)"("DisabledEnum"=T9."Enabled" ("Disabled")) -> ()  [unwired: 2 in, 2 out]
          }
        }
        n1337 = flat-sequence {
          tunnel: [w2380] -> w2360
          tunnel: [w2379] -> w2359
          tunnel: w2355 -> [w2377]
          tunnel: w2353 -> [w2376]
          tunnel: [w2384] -> _
          tunnel: [w2385] -> _
          tunnel: w2360 -> [w2385]
          tunnel: w2359 -> [w2384]
          frame #0 {
            n1338 = call "mDrive Send Command.vi"("error in (no error)"=w2376, "Command"=T10."Stop", "VISA resource name"=w2377) -> ("error out"=w2379:errorcluster, "VISA resource name out"=w2380:refnum<visa-resource-name>)  [unwired: 4 in, 1 out]
          }
          frame #1 {
            n1339 = property on="Z Scan" class="Bool (strict)"("Value"=FALSE ("Slew Ready")) -> ()  [unwired: 2 in, 2 out]
            n1340 = property on="Z Scan Velocity SP steps/sec" class="DigNum (strict)"("DisabledEnum"=T9."Enabled" ("Disabled")) -> ()  [unwired: 2 in, 2 out]
            n1341 = property on="Z Scan Length SP steps" class="DigNum (strict)"("DisabledEnum"=T9."Enabled" ("Disabled")) -> ()  [unwired: 2 in, 2 out]
          }
        }
        n1342 = flat-sequence {
          tunnel: [w2400] -> w2364
          tunnel: [w2399] -> w2363
          tunnel: w2352 -> [w2397]
          tunnel: w2350 -> [w2396]
          tunnel: [w2404] -> _
          tunnel: [w2405] -> _
          tunnel: w2364 -> [w2405]
          tunnel: w2363 -> [w2404]
          frame #0 {
            n1343 = call "mDrive Send Command.vi"("error in (no error)"=w2396, "Command"=T10."Stop", "VISA resource name"=w2397) -> ("error out"=w2399:errorcluster, "VISA resource name out"=w2400:refnum<visa-resource-name>)  [unwired: 4 in, 1 out]
          }
          frame #1 {
            n1344 = property on="Y Scan" class="Bool (strict)"("Value"=FALSE ("Slew Ready")) -> ()  [unwired: 2 in, 2 out]
            n1345 = property on="Y Scan Velocity SP steps/sec" class="DigNum (strict)"("DisabledEnum"=T9."Enabled" ("Disabled")) -> ()  [unwired: 2 in, 2 out]
            n1346 = property on="Y Scan Length SP steps" class="DigNum (strict)"("DisabledEnum"=T9."Enabled" ("Disabled")) -> ()  [unwired: 2 in, 2 out]
          }
        }
        n1347 = property on="GO" class="Bool"("DisabledEnum"=T9."Enabled" ("Disabled")) -> ()  [unwired: 2 in, 2 out]
        n1348 = property on="Set Scan \nParameters" class="Bool"("DisabledEnum"=T9."Enabled" ("Disabled")) -> ()  [unwired: 2 in, 2 out]
        n1349 = property on="Send scan parameter" class="Bool"("DisabledEnum"=T9."Enabled" ("Disabled")) -> ()  [unwired: 2 in, 2 out]
        n1350 = property on="Scan Go" class="Bool (strict)"("DisabledEnum"=T9."Disabled and Grayed Out" ("Disabled")) -> ()  [unwired: 2 in, 2 out]
      }
      event "Scan Go": Mouse Up {
        w2406 = T9."Disabled and Grayed Out" ("Disabled")
        n1351 = event-data() -> ()  [unwired: 1 in, 7 out]
        n1352 = flat-sequence {
          tunnel: [w2479] -> w2463
          tunnel: [w2477] -> w2456
          tunnel: [w2478] -> w2453
          tunnel: [w2472] -> w2452
          tunnel: [w2476] -> w2451
          tunnel: [w2475] -> w2450
          tunnel: [w2474] -> w2449
          tunnel: [w2473] -> w2448
          tunnel: w2423 -> [w2471]
          tunnel: w2422 -> [w2470]
          tunnel: w2421 -> [w2469]
          tunnel: w2420 -> [w2468]
          tunnel: w2419 -> [w2467]
          tunnel: w2418 -> [w2466]
          tunnel: w2417 -> [w2465]
          tunnel: w2416 -> [w2464]
          tunnel: [w2471] -> w2415
          tunnel: [w2470] -> w2414
          tunnel: [w2469] -> w2413
          tunnel: [w2468] -> w2412
          tunnel: [w2467] -> w2411
          tunnel: [w2466] -> w2410
          tunnel: [w2465] -> w2409
          tunnel: [w2464] -> w2408
          tunnel: [w2531] -> w2460
          tunnel: [w2530] -> w2458
          tunnel: w2463 -> [w2529]
          tunnel: w2456 -> [w2528]
          tunnel: [w2528] -> w2454
          tunnel: w2453 -> [w2527]
          tunnel: w2452 -> [w2516]
          tunnel: w2451 -> [w2526]
          tunnel: w2450 -> [w2522]
          tunnel: w2449 -> [w2519]
          tunnel: w2448 -> [w2525]
          tunnel: [w2524] -> w2446
          tunnel: [w2523] -> w2444
          tunnel: [w2522] -> w2441
          tunnel: [w2521] -> w2439
          tunnel: [w2520] -> w2437
          tunnel: [w2519] -> w2435
          tunnel: [w2518] -> w2433
          tunnel: [w2517] -> w2431
          tunnel: [w2516] -> w2430
          tunnel: w2415 -> [w2515]
          tunnel: w2414 -> [w2514]
          tunnel: w2413 -> [w2513]
          tunnel: w2412 -> [w2512]
          tunnel: w2411 -> [w2511]
          tunnel: w2410 -> [w2510]
          tunnel: w2409 -> [w2509]
          tunnel: w2408 -> [w2508]
          tunnel: w2460 -> [w2572]
          tunnel: [w2572] -> w2459
          tunnel: w2458 -> [w2571]
          tunnel: [w2571] -> w2457
          tunnel: [w2570] -> w2455
          tunnel: w2454 -> [w2570]
          tunnel: [w2569] -> w2447
          tunnel: w2446 -> [w2569]
          tunnel: [w2568] -> w2445
          tunnel: w2444 -> [w2568]
          tunnel: [w2567] -> w2443
          tunnel: [w2566] -> w2442
          tunnel: w2441 -> [w2566]
          tunnel: [w2565] -> w2440
          tunnel: w2439 -> [w2565]
          tunnel: [w2564] -> w2438
          tunnel: w2437 -> [w2564]
          tunnel: [w2563] -> w2436
          tunnel: w2435 -> [w2563]
          tunnel: [w2562] -> w2434
          tunnel: w2433 -> [w2562]
          tunnel: [w2561] -> w2432
          tunnel: w2431 -> [w2561]
          tunnel: w2430 -> [w2567]
          tunnel: w2459 -> [w2592]
          tunnel: [w2590] -> w2462
          tunnel: w2457 -> [w2591]
          tunnel: [w2589] -> w2461
          tunnel: w2455 -> [w2588]
          tunnel: w2447 -> [w2587]
          tunnel: w2445 -> [w2586]
          tunnel: w2443 -> [w2585]
          tunnel: w2442 -> [w2584]
          tunnel: w2440 -> [w2583]
          tunnel: w2438 -> [w2582]
          tunnel: w2436 -> [w2581]
          tunnel: w2434 -> [w2580]
          tunnel: w2432 -> [w2579]
          tunnel: [w2578] -> w2429
          tunnel: [w2577] -> w2428
          tunnel: [w2576] -> w2427
          tunnel: [w2575] -> w2426
          tunnel: [w2574] -> w2425
          tunnel: [w2573] -> w2424
          tunnel: w2462 -> [w2649]
          tunnel: w2461 -> [w2648]
          tunnel: [w2649] -> _
          tunnel: [w2648] -> _
          tunnel: [w2643] -> _
          tunnel: w2429 -> [w2643]
          tunnel: [w2642] -> _
          tunnel: w2428 -> [w2642]
          tunnel: w2427 -> [w2632]
          tunnel: [w2632] -> _
          tunnel: [w2631] -> _
          tunnel: w2426 -> [w2631]
          tunnel: [w2630] -> _
          tunnel: w2425 -> [w2630]
          tunnel: [w2629] -> _
          tunnel: w2424 -> [w2629]
          frame #0 {
            n1353 = property on="X Scan" class="Bool (strict)"() -> ("Value"=w2472:bool)  [unwired: 2 in, 2 out]
            n1354 = property on="Z Scan" class="Bool (strict)"() -> ("Value"=w2474:bool)  [unwired: 2 in, 2 out]
            n1355 = property on="Y Scan" class="Bool (strict)"() -> ("Value"=w2477:bool)  [unwired: 2 in, 2 out]
            n1356 = property on="R Scan" class="Bool (strict)"() -> ("Value"=w2475:bool)  [unwired: 2 in, 2 out]
            n1357 = case shown="False" w2472 {
              tunnel: ["" w2495] -> w2478
              frame False {
              }
              frame True {
                n1358 = property on="X Scan Length SP steps" class="DigNum (strict)"() -> ("Value"=w2500:i32)  [unwired: 2 in, 2 out]
                n1359 = Number To Decimal String(number=w2500) -> (decimal integer string=w2497:string)  [unwired: 1 in]
                n1360 = call <vilib>:"Space Constant.vi"() -> ("String"=w2498:string)
                n1361 = Concatenate Strings("MR", w2498, w2497, "\r") -> (w2495:string)
              }
            }
            n1362 = case shown="False" w2474 {
              tunnel: ["" w2488] -> w2476
              frame False {
              }
              frame True {
                n1363 = property on="Z Scan Length SP steps" class="DigNum (strict)"() -> ("Value"=w2493:i32)  [unwired: 2 in, 2 out]
                n1364 = Number To Decimal String(number=w2493) -> (decimal integer string=w2490:string)  [unwired: 1 in]
                n1365 = call <vilib>:"Space Constant.vi"() -> ("String"=w2491:string)
                n1366 = Concatenate Strings("MR", w2491, w2490, "\r") -> (w2488:string)
              }
            }
            n1367 = case shown="False" w2477 {
              tunnel: ["" w2502] -> w2479
              frame False {
              }
              frame True {
                n1368 = property on="Y Scan Length SP steps" class="DigNum (strict)"() -> ("Value"=w2507:i32)  [unwired: 2 in, 2 out]
                n1369 = Number To Decimal String(number=w2507) -> (decimal integer string=w2504:string)  [unwired: 1 in]
                n1370 = call <vilib>:"Space Constant.vi"() -> ("String"=w2505:string)
                n1371 = Concatenate Strings("MR", w2505, w2504, "\r") -> (w2502:string)
              }
            }
            n1372 = case shown="False" w2475 {
              tunnel: ["" w2481] -> w2473
              frame False {
              }
              frame True {
                n1373 = property on="R Scan Length SP steps" class="DigNum (strict)"() -> ("Value"=w2486:i32)  [unwired: 2 in, 2 out]
                n1374 = Number To Decimal String(number=w2486) -> (decimal integer string=w2483:string)  [unwired: 1 in]
                n1375 = call <vilib>:"Space Constant.vi"() -> ("String"=w2484:string)
                n1376 = Concatenate Strings("MR", w2484, w2483, "\r") -> (w2481:string)
              }
            }
          }
          frame #1 {
            n1377 = case shown="False" w2516 {
              tunnel: [w2547 w2552] -> w2524
              tunnel: [w2546 w2551] -> w2523
              tunnel: w2527 -> [_ w2550]
              tunnel: w2515 -> [w2547 w2549]
              tunnel: w2514 -> [w2546 w2548]
              frame False {
              }
              frame True {
                n1378 = VISA Write(VISA resource name=w2549, write buffer=w2550, error in (no error)=w2548) -> (VISA resource name out=w2552:refnum<visa-resource-name>, error out=w2551:errorcluster)  [unwired: 1 out]
              }
            }
            n1379 = case shown="True" w2519 {
              tunnel: [w2540 w2545] -> w2518
              tunnel: [w2539 w2544] -> w2517
              tunnel: w2526 -> [_ w2543]
              tunnel: w2513 -> [w2540 w2542]
              tunnel: w2512 -> [w2539 w2541]
              frame False {
              }
              frame True {
                n1380 = VISA Write(VISA resource name=w2542, write buffer=w2543, error in (no error)=w2541) -> (VISA resource name out=w2545:refnum<visa-resource-name>, error out=w2544:errorcluster)  [unwired: 1 out]
              }
            }
            n1381 = case shown="True" w2528 {
              tunnel: [w2554 w2559] -> w2531
              tunnel: [w2553 w2558] -> w2530
              tunnel: w2529 -> [_ w2557]
              tunnel: w2511 -> [w2554 w2556]
              tunnel: w2510 -> [w2553 w2555]
              frame False {
              }
              frame True {
                n1382 = VISA Write(VISA resource name=w2556, write buffer=w2557, error in (no error)=w2555) -> (VISA resource name out=w2559:refnum<visa-resource-name>, error out=w2558:errorcluster)  [unwired: 1 out]
              }
            }
            n1383 = case shown="True" w2522 {
              tunnel: [w2533 w2538] -> w2521
              tunnel: [w2532 w2537] -> w2520
              tunnel: w2525 -> [_ w2536]
              tunnel: w2509 -> [w2533 w2535]
              tunnel: w2508 -> [w2532 w2534]
              frame False {
              }
              frame True {
                n1384 = VISA Write(VISA resource name=w2535, write buffer=w2536, error in (no error)=w2534) -> (VISA resource name out=w2538:refnum<visa-resource-name>, error out=w2537:errorcluster)  [unwired: 1 out]
              }
            }
          }
          frame #2 {
            n1385 = Wait (ms)(milliseconds to wait=u32 100) -> ()  [unwired: 1 out]
          }
          frame #3 {
            n1386 = case shown="True" w2585 {
              tunnel: w2587 -> [w2612 w2616]
              tunnel: w2586 -> [w2611 w2615]
              tunnel: [w2612 w2614] -> w2574
              tunnel: [w2611 w2613] -> w2573
              frame False {
              }
              frame True {
                n1387 = property class="Instr"(reference=w2616, error in=w2615) -> (reference out=w2618:refnum<visa-resource-name>, error out=w2617:errorcluster, "Serial Settings:Number of Bytes at Serial Port"=w2619:u32)
                n1388 = VISA Read(VISA resource name=w2618, byte count=w2619, error in (no error)=w2617) -> (VISA resource name out=w2614:refnum<visa-resource-name>, error out=w2613:errorcluster)  [unwired: 2 out]
              }
            }
            n1389 = case shown="True" w2581 {
              tunnel: w2580 -> [w2594 w2598]
              tunnel: w2579 -> [w2593 w2597]
              tunnel: [w2594 w2596] -> w2578
              tunnel: [w2593 w2595] -> w2577
              frame False {
              }
              frame True {
                n1390 = property class="Instr"(reference=w2598, error in=w2597) -> (reference out=w2600:refnum<visa-resource-name>, error out=w2599:errorcluster, "Serial Settings:Number of Bytes at Serial Port"=w2601:u32)
                n1391 = VISA Read(VISA resource name=w2600, byte count=w2601, error in (no error)=w2599) -> (VISA resource name out=w2596:refnum<visa-resource-name>, error out=w2595:errorcluster)  [unwired: 2 out]
              }
            }
            n1392 = case shown="True" w2588 {
              tunnel: w2592 -> [w2621 w2625]
              tunnel: w2591 -> [w2620 w2624]
              tunnel: [w2621 w2623] -> w2590
              tunnel: [w2620 w2622] -> w2589
              frame False {
              }
              frame True {
                n1393 = property class="Instr"(reference=w2625, error in=w2624) -> (reference out=w2627:refnum<visa-resource-name>, error out=w2626:errorcluster, "Serial Settings:Number of Bytes at Serial Port"=w2628:u32)
                n1394 = VISA Read(VISA resource name=w2627, byte count=w2628, error in (no error)=w2626) -> (VISA resource name out=w2623:refnum<visa-resource-name>, error out=w2622:errorcluster)  [unwired: 2 out]
              }
            }
            n1395 = case shown="True" w2584 {
              tunnel: w2583 -> [w2603 w2607]
              tunnel: w2582 -> [w2602 w2606]
              tunnel: [w2603 w2605] -> w2576
              tunnel: [w2602 w2604] -> w2575
              frame False {
              }
              frame True {
                n1396 = property class="Instr"(reference=w2607, error in=w2606) -> (reference out=w2609:refnum<visa-resource-name>, error out=w2608:errorcluster, "Serial Settings:Number of Bytes at Serial Port"=w2610:u32)
                n1397 = VISA Read(VISA resource name=w2609, byte count=w2610, error in (no error)=w2608) -> (VISA resource name out=w2605:refnum<visa-resource-name>, error out=w2604:errorcluster)  [unwired: 2 out]
              }
            }
          }
          frame #4 {
            n1398 = property on="R Scan" class="Bool (strict)"("Val(Sgnl)"=FALSE ("Slew Ready 2")) -> ()  [unwired: 2 in, 2 out]
            n1399 = property on="Z Scan" class="Bool (strict)"("Val(Sgnl)"=FALSE ("Slew Ready 2")) -> ()  [unwired: 2 in, 2 out]
            n1400 = property on="Y Scan" class="Bool (strict)"("Val(Sgnl)"=FALSE ("Slew Ready 2")) -> ()  [unwired: 2 in, 2 out]
            n1401 = property on="X Scan" class="Bool (strict)"("Val(Sgnl)"=FALSE ("Slew Ready 2")) -> ()  [unwired: 2 in, 2 out]
            n1402 = property on="R Scan Length SP steps" class="DigNum (strict)"("DisabledEnum"=T9."Enabled" ("Disabled")) -> ()  [unwired: 2 in, 2 out]
            n1403 = property on="Z Scan Velocity SP steps/sec" class="DigNum (strict)"("DisabledEnum"=T9."Enabled" ("Disabled")) -> ()  [unwired: 2 in, 2 out]
            n1404 = property on="X Scan Length SP steps" class="DigNum (strict)"("DisabledEnum"=T9."Enabled" ("Disabled")) -> ()  [unwired: 2 in, 2 out]
            n1405 = property on="Y Scan Selocity SP steps/sec" class="DigNum (strict)"("DisabledEnum"=T9."Enabled" ("Disabled")) -> ()  [unwired: 2 in, 2 out]
            n1406 = property on="Z Scan Length SP steps" class="DigNum (strict)"("DisabledEnum"=T9."Enabled" ("Disabled")) -> ()  [unwired: 2 in, 2 out]
            n1407 = property on="X Scan Velocity SP steps/sec" class="DigNum (strict)"("DisabledEnum"=T9."Enabled" ("Disabled")) -> ()  [unwired: 2 in, 2 out]
            n1408 = property on="Y Scan Length SP steps" class="DigNum (strict)"("DisabledEnum"=T9."Enabled" ("Disabled")) -> ()  [unwired: 2 in, 2 out]
            n1409 = property on="R Scan Velocity SP steps/sec" class="DigNum (strict)"("DisabledEnum"=T9."Enabled" ("Disabled")) -> ()  [unwired: 2 in, 2 out]
            n1410 = property on="Scan Go" class="Bool (strict)"("DisabledEnum"=T9."Disabled and Grayed Out" ("Disabled")) -> ()  [unwired: 2 in, 2 out]
          }
        }
        n1411 = local write "STATUS"("SCANNING" ("STATUS")) -> ()
        n1412 = property on="GO" class="Bool"("DisabledEnum"=w2406) -> ()  [unwired: 2 in, 2 out]
        n1413 = property on="Set Scan \nParameters" class="Bool"("DisabledEnum"=w2406) -> ()  [unwired: 2 in, 2 out]
        n1414 = property on="Send scan parameter" class="Bool"("DisabledEnum"=w2406) -> ()  [unwired: 2 in, 2 out]
      }
      event "Reset": Mouse Down {
        n1415 = event-data() -> ()  [unwired: 1 in, 7 out]
        n1416 = flat-sequence {
          tunnel: [w2661] -> _
          tunnel: [w2662] -> _
          tunnel: w2654 -> [w2659]
          tunnel: w2650 -> [w2658]
          frame #0 {
            n1417 = property on="Reset R Motor Steps" class="DigNum (strict)"() -> ("Value"=w2660:i32)  [unwired: 2 in, 2 out]
            n1418 = Number To Decimal String(number=w2660) -> (decimal integer string=w2663:string)  [unwired: 1 in]
            n1419 = call "mDrive Send Command.vi"("error in (no error)"=w2659, "Extra"=w2663, "Command"=T10."Set Current Position", "VISA resource name"=w2658) -> ("error out"=w2662:errorcluster, "VISA resource name out"=w2661:refnum<visa-resource-name>)  [unwired: 3 in, 1 out]
          }
        }
        n1420 = flat-sequence {
          tunnel: [w2681] -> _
          tunnel: [w2682] -> _
          tunnel: w2657 -> [w2680]
          tunnel: w2653 -> [w2679]
          frame #0 {
            n1421 = property on="Reset X Motor Steps" class="DigNum (strict)"() -> ("Value"=w2683:i32)  [unwired: 2 in, 2 out]
            n1422 = Number To Decimal String(number=w2683) -> (decimal integer string=w2684:string)  [unwired: 1 in]
            n1423 = call "mDrive Send Command.vi"("error in (no error)"=w2680, "Extra"=w2684, "Command"=T10."Set Current Position", "VISA resource name"=w2679) -> ("error out"=w2682:errorcluster, "VISA resource name out"=w2681:refnum<visa-resource-name>)  [unwired: 3 in, 1 out]
          }
        }
        n1424 = flat-sequence {
          tunnel: [w2675] -> _
          tunnel: [w2676] -> _
          tunnel: w2656 -> [w2673]
          tunnel: w2652 -> [w2672]
          frame #0 {
            n1425 = property on="Reset Z Motor Steps" class="DigNum (strict)"() -> ("Value"=w2674:i32)  [unwired: 2 in, 2 out]
            n1426 = Number To Decimal String(number=w2674) -> (decimal integer string=w2677:string)  [unwired: 1 in]
            n1427 = call "mDrive Send Command.vi"("error in (no error)"=w2673, "Extra"=w2677, "Command"=T10."Set Current Position", "VISA resource name"=w2672) -> ("error out"=w2676:errorcluster, "VISA resource name out"=w2675:refnum<visa-resource-name>)  [unwired: 3 in, 1 out]
          }
        }
        n1428 = flat-sequence {
          tunnel: [w2668] -> _
          tunnel: [w2669] -> _
          tunnel: w2655 -> [w2666]
          tunnel: w2651 -> [w2665]
          frame #0 {
            n1429 = property on="Reset Y Motor Steps" class="DigNum (strict)"() -> ("Value"=w2667:i32)  [unwired: 2 in, 2 out]
            n1430 = Number To Decimal String(number=w2667) -> (decimal integer string=w2670:string)  [unwired: 1 in]
            n1431 = call "mDrive Send Command.vi"("error in (no error)"=w2666, "Extra"=w2670, "Command"=T10."Set Current Position", "VISA resource name"=w2665) -> ("error out"=w2669:errorcluster, "VISA resource name out"=w2668:refnum<visa-resource-name>)  [unwired: 3 in, 1 out]
          }
        }
      }
      event "LOOP": Mouse Up {
        n1432 = event-data() -> ()  [unwired: 1 in, 7 out]
        n1433 = flat-sequence {
          tunnel: w2705 -> [w4297]
          tunnel: [w4297] -> w2704
          tunnel: w2703 -> [w4296]
          tunnel: [w4296] -> w2702
          tunnel: w2701 -> [w4295]
          tunnel: [w4295] -> w2700
          tunnel: w2699 -> [w4294]
          tunnel: [w4294] -> w2698
          tunnel: w2697 -> [w4293]
          tunnel: [w4293] -> w2696
          tunnel: w2695 -> [w4292]
          tunnel: [w4292] -> w2694
          tunnel: w2693 -> [w4291]
          tunnel: [w4291] -> w2692
          tunnel: w2691 -> [w4290]
          tunnel: [w4290] -> w2690
          frame #0 {
            w4298 = T9."Disabled and Grayed Out" ("Disabled")
            n1434 = local write "STATUS"("ENTERING LOOP" ("STATUS")) -> ()
            n1435 = property on="Z Scan Length SP steps" class="DigNum (strict)"("DisabledEnum"=T9."Disabled and Grayed Out" ("Disabled")) -> ()  [unwired: 2 in, 2 out]
            n1436 = property on="Z Scan Velocity SP steps/sec" class="DigNum (strict)"("DisabledEnum"=T9."Disabled and Grayed Out" ("Disabled")) -> ()  [unwired: 2 in, 2 out]
            n1437 = property on="GO" class="Bool"("DisabledEnum"=w4298) -> ()  [unwired: 2 in, 2 out]
            n1438 = property on="Set Scan \nParameters" class="Bool"("DisabledEnum"=w4298) -> ()  [unwired: 2 in, 2 out]
            n1439 = property on="Scan Go" class="Bool (strict)"("DisabledEnum"=w4298) -> ()  [unwired: 2 in, 2 out]
            n1440 = property on="Send scan parameter" class="Bool"("DisabledEnum"=w4298) -> ()  [unwired: 2 in, 2 out]
            n1441 = property on="R Scan Length SP steps" class="DigNum (strict)"("DisabledEnum"=T9."Disabled and Grayed Out" ("Disabled")) -> ()  [unwired: 2 in, 2 out]
            n1442 = property on="R Scan Velocity SP steps/sec" class="DigNum (strict)"("DisabledEnum"=T9."Disabled and Grayed Out" ("Disabled")) -> ()  [unwired: 2 in, 2 out]
            n1443 = property on="Y Scan Length SP steps" class="DigNum (strict)"("DisabledEnum"=T9."Disabled and Grayed Out" ("Disabled")) -> ()  [unwired: 2 in, 2 out]
            n1444 = property on="Y Scan Velocity SP steps/sec" class="DigNum (strict)"("DisabledEnum"=T9."Disabled and Grayed Out" ("Disabled")) -> ()  [unwired: 2 in, 2 out]
            n1445 = property on="X Scan Length SP steps" class="DigNum (strict)"("DisabledEnum"=T9."Disabled and Grayed Out" ("Disabled")) -> ()  [unwired: 2 in, 2 out]
            n1446 = property on="X Scan Velocity SP steps/sec" class="DigNum (strict)"("DisabledEnum"=T9."Disabled and Grayed Out" ("Disabled")) -> ()  [unwired: 2 in, 2 out]
          }
        }
        n1447 = while {
          tunnel: w2700 -> [w2762]
          tunnel: w2696 -> [w2761]
          tunnel: w2698 -> [w2760]
          tunnel: w2694 -> [w2759]
          tunnel: w2692 -> [w2758]
          tunnel: w2690 -> [w2757]
          tunnel: w2702 -> [w2756]
          tunnel: w2704 -> [w2755]
          tunnel: [w2754] -> w2689 mode=indexing
          tunnel: [w2753] -> w2688 mode=indexing
          tunnel: [w2752] -> w2687 mode=indexing
          tunnel: [w2751] -> w2686 mode=indexing
          i -> [w2717]
          stop <- w2706 stop-if-true
          # "XZYR"
          n1448 = flat-sequence {
            tunnel: w2761 -> [w2790]
            tunnel: w2762 -> [w2791]
            tunnel: [w2787] -> w2778
            tunnel: [w2780] -> w2777
            tunnel: [w2786] -> w2776
            tunnel: [w2785] -> w2775
            tunnel: [w2784] -> w2774
            tunnel: [w2783] -> w2773
            tunnel: [w2779] -> w2772
            tunnel: [w2782] -> w2771
            tunnel: w2760 -> [w2795]
            tunnel: w2759 -> [w2794]
            tunnel: w2758 -> [w2793]
            tunnel: w2757 -> [w2792]
            tunnel: w2756 -> [w2789]
            tunnel: w2755 -> [w2788]
            tunnel: [w2925] -> w2734
            tunnel: [w2924] -> w2732
            tunnel: [w2923] -> w2730
            tunnel: [w2922] -> w2728
            tunnel: [w2920] -> w2726
            tunnel: [w2919] -> w2724
            tunnel: [w2921] -> w2722
            tunnel: w2778 -> [w2918]
            tunnel: w2777 -> [w2917]
            tunnel: w2776 -> [w2916]
            tunnel: w2775 -> [w2915]
            tunnel: w2774 -> [w2914]
            tunnel: w2773 -> [w2913]
            tunnel: w2772 -> [w2912]
            tunnel: w2771 -> [w2911]
            tunnel: [w2910] -> w2720
            tunnel: w2734 -> [w3050]
            tunnel: [w3050] -> w2733
            tunnel: w2732 -> [w3049]
            tunnel: [w3049] -> w2731
            tunnel: w2730 -> [w3048]
            tunnel: [w3048] -> w2729
            tunnel: w2728 -> [w3047]
            tunnel: [w3047] -> w2727
            tunnel: w2726 -> [w3046]
            tunnel: [w3046] -> w2725
            tunnel: w2724 -> [w3045]
            tunnel: [w3045] -> w2723
            tunnel: w2722 -> [w3044]
            tunnel: [w3044] -> w2721
            tunnel: w2720 -> [w3043]
            tunnel: [w3043] -> w2719
            tunnel: [w3065] -> w2750
            tunnel: [w3063] -> w2748
            tunnel: [w3056] -> w2746
            tunnel: [w3055] -> w2744
            tunnel: [w3054] -> w2742
            tunnel: [w3053] -> w2740
            tunnel: [w3052] -> w2738
            tunnel: [w3051] -> w2736
            tunnel: w2733 -> [w3066]
            tunnel: w2731 -> [w3064]
            tunnel: w2729 -> [w3061]
            tunnel: w2727 -> [w3060]
            tunnel: w2725 -> [w3058]
            tunnel: w2723 -> [w3057]
            tunnel: w2721 -> [w3059]
            tunnel: w2719 -> [w3062]
            tunnel: w2750 -> [w3348]
            tunnel: [w3348] -> w2749
            tunnel: w2748 -> [w3347]
            tunnel: [w3347] -> w2747
            tunnel: w2746 -> [w3346]
            tunnel: [w3346] -> w2745
            tunnel: w2744 -> [w3345]
            tunnel: [w3345] -> w2743
            tunnel: w2742 -> [w3344]
            tunnel: [w3344] -> w2741
            tunnel: w2740 -> [w3343]
            tunnel: [w3343] -> w2739
            tunnel: w2738 -> [w3342]
            tunnel: [w3342] -> w2737
            tunnel: w2736 -> [w3341]
            tunnel: [w3341] -> w2735
            tunnel: w2749 -> [w3366]
            tunnel: w2747 -> [w3364]
            tunnel: w2745 -> [w3365]
            tunnel: w2743 -> [w3363]
            tunnel: w2741 -> [w3362]
            tunnel: w2739 -> [w3361]
            tunnel: w2737 -> [w3360]
            tunnel: w2735 -> [w3359]
            tunnel: [w3358] -> w2770
            tunnel: [w3357] -> w2769
            tunnel: [w3356] -> w2768
            tunnel: [w3355] -> w2767
            tunnel: [w3354] -> w2766
            tunnel: [w3353] -> w2765
            tunnel: [w3352] -> w2764
            tunnel: [w3351] -> w2763
            tunnel: w2770 -> [w3659]
            tunnel: w2769 -> [w3660]
            tunnel: w2768 -> [w3662]
            tunnel: w2767 -> [w3661]
            tunnel: w2766 -> [w3665]
            tunnel: w2765 -> [w3666]
            tunnel: w2764 -> [w3663]
            tunnel: w2763 -> [w3664]
            tunnel: [w3668] -> w2716
            tunnel: [w3667] -> w2715
            tunnel: [w3669] -> w2714
            tunnel: [w3670] -> w2713
            tunnel: [w3673] -> w2712
            tunnel: [w3674] -> w2711
            tunnel: [w3671] -> w2710
            tunnel: [w3672] -> w2709
            tunnel: [w4269] -> _
            tunnel: [w4270] -> w2754
            tunnel: [w4271] -> _
            tunnel: [w4272] -> w2753
            tunnel: [w4273] -> _
            tunnel: [w4274] -> w2751
            tunnel: [w4275] -> w2752
            tunnel: [w4276] -> _
            tunnel: w2716 -> [w4276]
            tunnel: w2715 -> [w4275]
            tunnel: w2714 -> [w4274]
            tunnel: w2713 -> [w4273]
            tunnel: w2712 -> [w4272]
            tunnel: w2711 -> [w4271]
            tunnel: w2710 -> [w4270]
            tunnel: w2709 -> [w4269]
            frame #0 {
              n1449 = flat-sequence {
                tunnel: [w2887] -> w2819
                tunnel: [w2886] -> w2818
                tunnel: w2790 -> [w2889]
                tunnel: w2791 -> [w2888]
                tunnel: w2819 -> [w2895]
                tunnel: [w2895] -> w2817
                tunnel: w2818 -> [w2894]
                tunnel: [w2894] -> w2816
                tunnel: w2817 -> [w2899]
                tunnel: [w2898] -> w2815
                tunnel: w2816 -> [w2897]
                tunnel: [w2896] -> w2814
                tunnel: w2815 -> [w2907]
                tunnel: w2814 -> [w2905]
                tunnel: [w2907] -> w2787
                tunnel: [w2905] -> w2780
                frame #0 {
                  n1450 = property on="X Scan Velocity SP steps/sec" class="DigNum (strict)"() -> ("Value"=w2891:i32)  [unwired: 2 in, 2 out]
                  n1451 = Number To Decimal String(number=w2891) -> (decimal integer string=w2892:string)  [unwired: 1 in]
                  n1452 = call "mDrive Send Command.vi"("error in (no error)"=w2889, "Extra"=w2892, "Command"=T10."Max Velocity", "VISA resource name"=w2888) -> ("error out"=w2886:errorcluster, "VISA resource name out"=w2887:refnum<visa-resource-name>)  [unwired: 3 in, 1 out]
                }
                frame #1 {
                  n1453 = Wait (ms)(milliseconds to wait=u32 100) -> ()  [unwired: 1 out]
                }
                frame #2 {
                  # "VELOCITY"
                  n1454 = call "mDrive Send Command.vi"("error in (no error)"=w2897, "Extra"="VM", "Command"=T10."Print Parameter", "VISA resource name"=w2899) -> ("error out"=w2896:errorcluster, "read buffer"=w2902:string, "VISA resource name out"=w2898:refnum<visa-resource-name>)  [unwired: 3 in]
                  n1455 = Decimal String To Number(string=w2902, offset=0) -> (number=w2900:i32)  [unwired: 1 in, 1 out]
                  n1456 = property on="X velocity PV step/sec" class="DigNum (strict)"("Val(Sgnl)"=w2900) -> ()  [unwired: 2 in, 2 out]
                }
                frame #3 {
                  n1457 = Wait (ms)(milliseconds to wait=u32 100) -> ()  [unwired: 1 out]
                }
              }
              n1458 = flat-sequence {
                tunnel: [w2845] -> w2807
                tunnel: [w2844] -> w2806
                tunnel: w2794 -> [w2843]
                tunnel: w2795 -> [w2842]
                tunnel: w2807 -> [w2851]
                tunnel: [w2851] -> w2805
                tunnel: w2806 -> [w2850]
                tunnel: [w2850] -> w2804
                tunnel: w2805 -> [w2857]
                tunnel: [w2856] -> w2803
                tunnel: w2804 -> [w2855]
                tunnel: [w2854] -> w2802
                tunnel: w2803 -> [w2863]
                tunnel: w2802 -> [w2862]
                tunnel: [w2863] -> w2786
                tunnel: [w2862] -> w2785
                frame #0 {
                  n1459 = property on="Z Scan Velocity SP steps/sec" class="DigNum (strict)"() -> ("Value"=w2847:i32)  [unwired: 2 in, 2 out]
                  n1460 = Number To Decimal String(number=w2847) -> (decimal integer string=w2848:string)  [unwired: 1 in]
                  n1461 = call "mDrive Send Command.vi"("error in (no error)"=w2843, "Extra"=w2848, "Command"=T10."Max Velocity", "VISA resource name"=w2842) -> ("error out"=w2844:errorcluster, "VISA resource name out"=w2845:refnum<visa-resource-name>)  [unwired: 3 in, 1 out]
                }
                frame #1 {
                  n1462 = Wait (ms)(milliseconds to wait=u32 100) -> ()  [unwired: 1 out]
                }
                frame #2 {
                  # "VELOCITY"
                  n1463 = call "mDrive Send Command.vi"("error in (no error)"=w2855, "Extra"="VM", "Command"=T10."Print Parameter", "VISA resource name"=w2857) -> ("error out"=w2854:errorcluster, "read buffer"=w2858:string, "VISA resource name out"=w2856:refnum<visa-resource-name>)  [unwired: 3 in]
                  n1464 = Decimal String To Number(string=w2858, offset=0) -> (number=w2859:i32)  [unwired: 1 in, 1 out]
                  n1465 = property on="Z  velocity PV step/sec" class="DigNum (strict)"("Val(Sgnl)"=w2859) -> ()  [unwired: 2 in, 2 out]
                }
                frame #3 {
                  n1466 = Wait (ms)(milliseconds to wait=u32 100) -> ()  [unwired: 1 out]
                }
              }
              n1467 = flat-sequence {
                tunnel: [w2867] -> w2813
                tunnel: [w2866] -> w2812
                tunnel: w2792 -> [w2865]
                tunnel: w2793 -> [w2864]
                tunnel: w2813 -> [w2873]
                tunnel: [w2873] -> w2811
                tunnel: w2812 -> [w2872]
                tunnel: [w2872] -> w2810
                tunnel: w2811 -> [w2877]
                tunnel: [w2876] -> w2809
                tunnel: w2810 -> [w2875]
                tunnel: [w2874] -> w2808
                tunnel: w2809 -> [w2885]
                tunnel: w2808 -> [w2884]
                tunnel: [w2885] -> w2784
                tunnel: [w2884] -> w2783
                frame #0 {
                  n1468 = property on="Y Scan Velocity SP steps/sec" class="DigNum (strict)"() -> ("Value"=w2869:i32)  [unwired: 2 in, 2 out]
                  n1469 = Number To Decimal String(number=w2869) -> (decimal integer string=w2870:string)  [unwired: 1 in]
                  n1470 = call "mDrive Send Command.vi"("error in (no error)"=w2865, "Extra"=w2870, "Command"=T10."Max Velocity", "VISA resource name"=w2864) -> ("error out"=w2866:errorcluster, "VISA resource name out"=w2867:refnum<visa-resource-name>)  [unwired: 3 in, 1 out]
                }
                frame #1 {
                  n1471 = Wait (ms)(milliseconds to wait=u32 100) -> ()  [unwired: 1 out]
                }
                frame #2 {
                  # "VELOCITY"
                  n1472 = call "mDrive Send Command.vi"("error in (no error)"=w2875, "Extra"="VM", "Command"=T10."Print Parameter", "VISA resource name"=w2877) -> ("error out"=w2874:errorcluster, "read buffer"=w2881:string, "VISA resource name out"=w2876:refnum<visa-resource-name>)  [unwired: 3 in]
                  n1473 = Decimal String To Number(string=w2881, offset=0) -> (number=w2879:i32)  [unwired: 1 in, 1 out]
                  n1474 = property on="Y velocity PV step/sec" class="DigNum (strict)"("Val(Sgnl)"=w2879) -> ()  [unwired: 2 in, 2 out]
                }
                frame #3 {
                  n1475 = Wait (ms)(milliseconds to wait=u32 100) -> ()  [unwired: 1 out]
                }
              }
              n1476 = flat-sequence {
                tunnel: [w2823] -> w2801
                tunnel: [w2822] -> w2800
                tunnel: w2789 -> [w2821]
                tunnel: w2788 -> [w2820]
                tunnel: w2801 -> [w2829]
                tunnel: [w2829] -> w2799
                tunnel: w2800 -> [w2828]
                tunnel: [w2828] -> w2798
                tunnel: w2799 -> [w2835]
                tunnel: [w2834] -> w2797
                tunnel: w2798 -> [w2833]
                tunnel: [w2832] -> w2796
                tunnel: w2797 -> [w2839]
                tunnel: w2796 -> [w2841]
                tunnel: [w2841] -> w2782
                tunnel: [w2839] -> w2779
                frame #0 {
                  n1477 = property on="R Scan Velocity SP steps/sec" class="DigNum (strict)"() -> ("Value"=w2825:i32)  [unwired: 2 in, 2 out]
                  n1478 = Number To Decimal String(number=w2825) -> (decimal integer string=w2826:string)  [unwired: 1 in]
                  n1479 = call "mDrive Send Command.vi"("error in (no error)"=w2821, "Extra"=w2826, "Command"=T10."Max Velocity", "VISA resource name"=w2820) -> ("error out"=w2822:errorcluster, "VISA resource name out"=w2823:refnum<visa-resource-name>)  [unwired: 3 in, 1 out]
                }
                frame #1 {
                  n1480 = Wait (ms)(milliseconds to wait=u32 100) -> ()  [unwired: 1 out]
                }
                frame #2 {
                  # "VELOCITY"
                  n1481 = call "mDrive Send Command.vi"("error in (no error)"=w2833, "Extra"="VM", "Command"=T10."Print Parameter", "VISA resource name"=w2835) -> ("error out"=w2832:errorcluster, "read buffer"=w2837:string, "VISA resource name out"=w2834:refnum<visa-resource-name>)  [unwired: 3 in]
                  n1482 = Decimal String To Number(string=w2837, offset=0) -> (number=w2836:i32)  [unwired: 1 in, 1 out]
                  n1483 = property on="R velocity PV step/sec" class="DigNum (strict)"("Val(Sgnl)"=w2836) -> ()  [unwired: 2 in, 2 out]
                }
                frame #3 {
                  n1484 = Wait (ms)(milliseconds to wait=u32 100) -> ()  [unwired: 1 out]
                }
              }
              n1485 = local write "STATUS"("LOOP INITIALIZING" ("STATUS")) -> ()
            }
            frame #1 {
              w2908 = TRUE ("R in Motion")
              n1486 = flat-sequence {
                tunnel: [w2985] -> w2953
                tunnel: [w2984] -> w2952
                tunnel: [w2983] -> w2951
                tunnel: [w2982] -> w2950
                tunnel: w2918 -> [w2981]
                tunnel: w2917 -> [w2980]
                tunnel: w2916 -> [w2979]
                tunnel: w2915 -> [w2978]
                tunnel: w2914 -> [w2977]
                tunnel: w2913 -> [w2976]
                tunnel: w2912 -> [w2975]
                tunnel: w2911 -> [w2974]
                tunnel: [w2981] -> w2949
                tunnel: [w2980] -> w2948
                tunnel: [w2979] -> w2947
                tunnel: [w2978] -> w2946
                tunnel: [w2977] -> w2945
                tunnel: [w2976] -> w2944
                tunnel: [w2975] -> w2943
                tunnel: [w2974] -> w2942
                tunnel: [w3005] -> w2941
                tunnel: [w3004] -> w2940
                tunnel: w2953 -> [w3003]
                tunnel: w2952 -> [w3002]
                tunnel: w2951 -> [w3001]
                tunnel: w2950 -> [w3000]
                tunnel: [w2999] -> w2939
                tunnel: [w2998] -> w2938
                tunnel: [w2997] -> w2937
                tunnel: [w2996] -> w2936
                tunnel: [w2995] -> w2935
                tunnel: [w2994] -> w2934
                tunnel: w2949 -> [w2993]
                tunnel: w2948 -> [w2992]
                tunnel: w2947 -> [w2991]
                tunnel: w2946 -> [w2990]
                tunnel: w2945 -> [w2989]
                tunnel: w2944 -> [w2988]
                tunnel: w2943 -> [w2987]
                tunnel: w2942 -> [w2986]
                tunnel: w2941 -> [w3014]
                tunnel: [w3014] -> w2933
                tunnel: w2940 -> [w3013]
                tunnel: [w3013] -> w2932
                tunnel: [w3012] -> w2931
                tunnel: w2939 -> [w3012]
                tunnel: [w3011] -> w2930
                tunnel: w2938 -> [w3011]
                tunnel: [w3010] -> w2929
                tunnel: w2937 -> [w3010]
                tunnel: [w3009] -> w2928
                tunnel: w2936 -> [w3009]
                tunnel: [w3008] -> w2927
                tunnel: w2935 -> [w3008]
                tunnel: [w3007] -> w2926
                tunnel: w2934 -> [w3007]
                tunnel: w2933 -> [w3042]
                tunnel: w2932 -> [w3041]
                tunnel: w2931 -> [w3038]
                tunnel: w2930 -> [w3037]
                tunnel: w2929 -> [w3036]
                tunnel: w2928 -> [w3035]
                tunnel: w2927 -> [w3034]
                tunnel: w2926 -> [w3033]
                tunnel: [w3040] -> w2922
                tunnel: [w3039] -> w2921
                tunnel: [w3032] -> w2923
                tunnel: [w3031] -> w2920
                tunnel: [w3030] -> w2919
                tunnel: [w3029] -> w2925
                tunnel: [w3028] -> w2924
                tunnel: [w3015] -> w2910
                frame #0 {
                  n1487 = property on="X Scan Length SP steps" class="DigNum (strict)"() -> ("Value"=w2968:i32)  [unwired: 2 in, 2 out]
                  n1488 = property on="Z Scan Length SP steps" class="DigNum (strict)"() -> ("Value"=w2973:i32)  [unwired: 2 in, 2 out]
                  n1489 = property on="Y Scan Length SP steps" class="DigNum (strict)"() -> ("Value"=w2963:i32)  [unwired: 2 in, 2 out]
                  n1490 = property on="R Scan Length SP steps" class="DigNum (strict)"() -> ("Value"=w2958:i32)  [unwired: 2 in, 2 out]
                  n1491 = Number To Decimal String(number=w2968) -> (decimal integer string=w2965:string)  [unwired: 1 in]
                  n1492 = Number To Decimal String(number=w2973) -> (decimal integer string=w2970:string)  [unwired: 1 in]
                  n1493 = Number To Decimal String(number=w2963) -> (decimal integer string=w2960:string)  [unwired: 1 in]
                  n1494 = Number To Decimal String(number=w2958) -> (decimal integer string=w2955:string)  [unwired: 1 in]
                  n1495 = call <vilib>:"Space Constant.vi"() -> ("String"=w2966:string)
                  n1496 = call <vilib>:"Space Constant.vi"() -> ("String"=w2971:string)
                  n1497 = call <vilib>:"Space Constant.vi"() -> ("String"=w2961:string)
                  n1498 = call <vilib>:"Space Constant.vi"() -> ("String"=w2956:string)
                  n1499 = Concatenate Strings("MR", w2966, w2965, "\r") -> (w2984:string)
                  n1500 = Concatenate Strings("MR", w2971, w2970, "\r") -> (w2983:string)
                  n1501 = Concatenate Strings("MR", w2961, w2960, "\r") -> (w2985:string)
                  n1502 = Concatenate Strings("MR", w2956, w2955, "\r") -> (w2982:string)
                }
                frame #1 {
                  n1503 = VISA Write(VISA resource name=w2993, write buffer=w3002, error in (no error)=w2992) -> (VISA resource name out=w2999:refnum<visa-resource-name>, error out=w2998:errorcluster)  [unwired: 1 out]
                  n1504 = VISA Write(VISA resource name=w2991, write buffer=w3001, error in (no error)=w2990) -> (VISA resource name out=w2995:refnum<visa-resource-name>, error out=w2994:errorcluster)  [unwired: 1 out]
                  n1505 = VISA Write(VISA resource name=w2989, write buffer=w3003, error in (no error)=w2988) -> (VISA resource name out=w3005:refnum<visa-resource-name>, error out=w3004:errorcluster)  [unwired: 1 out]
                  n1506 = VISA Write(VISA resource name=w2987, write buffer=w3000, error in (no error)=w2986) -> (VISA resource name out=w2997:refnum<visa-resource-name>, error out=w2996:errorcluster)  [unwired: 1 out]
                }
                frame #2 {
                  n1507 = Wait (ms)(milliseconds to wait=u32 100) -> ()  [unwired: 1 out]
                }
                frame #3 {
                  n1508 = property class="Instr"(reference=w3038, error in=w3037) -> (reference out=w3020:refnum<visa-resource-name>, error out=w3019:errorcluster, "Serial Settings:Number of Bytes at Serial Port"=w3021:u32)
                  n1509 = property class="Instr"(reference=w3034, error in=w3033) -> (reference out=w3017:refnum<visa-resource-name>, error out=w3016:errorcluster, "Serial Settings:Number of Bytes at Serial Port"=w3018:u32)
                  n1510 = property class="Instr"(reference=w3042, error in=w3041) -> (reference out=w3023:refnum<visa-resource-name>, error out=w3022:errorcluster, "Serial Settings:Number of Bytes at Serial Port"=w3024:u32)
                  n1511 = property class="Instr"(reference=w3036, error in=w3035) -> (reference out=w3026:refnum<visa-resource-name>, error out=w3025:errorcluster, "Serial Settings:Number of Bytes at Serial Port"=w3027:u32)
                  n1512 = VISA Read(VISA resource name=w3020, byte count=w3021, error in (no error)=w3019) -> (VISA resource name out=w3029:refnum<visa-resource-name>, error out=w3028:errorcluster)  [unwired: 2 out]
                  n1513 = VISA Read(VISA resource name=w3017, byte count=w3018, error in (no error)=w3016) -> (VISA resource name out=w3015:refnum<visa-resource-name>, error out=w3032:errorcluster)  [unwired: 2 out]
                  n1514 = VISA Read(VISA resource name=w3023, byte count=w3024, error in (no error)=w3022) -> (VISA resource name out=w3040:refnum<visa-resource-name>, error out=w3039:errorcluster)  [unwired: 2 out]
                  n1515 = VISA Read(VISA resource name=w3026, byte count=w3027, error in (no error)=w3025) -> (VISA resource name out=w3031:refnum<visa-resource-name>, error out=w3030:errorcluster)  [unwired: 2 out]
                }
              }
              n1516 = local write "STATUS"("LOOP SCANNING" ("STATUS")) -> ()
              n1517 = property on="Y in Motion" class="Bool (strict)"("Value"=w2908) -> ()  [unwired: 2 in, 2 out]
              n1518 = property on="Z in Motion" class="Bool (strict)"("Value"=w2908) -> ()  [unwired: 2 in, 2 out]
              n1519 = property on="X  in Motion" class="Bool (strict)"("Value"=w2908) -> ()  [unwired: 2 in, 2 out]
              n1520 = property on="R in Motion" class="Bool (strict)"("Value"=w2908) -> ()  [unwired: 2 in, 2 out]
            }
            frame #2 {
            }
            frame #3 {
              n1521 = while {
                tunnel: w3066 -> [w3088]
                tunnel: [w3076] -> w3065
                tunnel: w3064 -> [w3087]
                tunnel: [w3075] -> w3063
                tunnel: w3062 -> [w3086]
                tunnel: w3061 -> [w3085]
                tunnel: w3060 -> [w3084]
                tunnel: w3059 -> [w3083]
                tunnel: w3058 -> [w3082]
                tunnel: w3057 -> [w3081]
                tunnel: [w3078] -> w3056
                tunnel: [w3077] -> w3055
                tunnel: [w3074] -> w3054
                tunnel: [w3073] -> w3053
                tunnel: [w3072] -> w3052
                tunnel: [w3071] -> w3051
                stop <- w3067 stop-if-true
                n1522 = flat-sequence {
                  tunnel: [w3243] -> w3115
                  tunnel: [w3235] -> w3114
                  tunnel: [w3234] -> w3113
                  tunnel: w3086 -> [w3237]
                  tunnel: w3085 -> [w3232]
                  tunnel: [w3265] -> w3112
                  tunnel: [w3264] -> w3111
                  tunnel: [w3263] -> w3110
                  tunnel: w3115 -> [w3263]
                  tunnel: w3114 -> [w3262]
                  tunnel: w3113 -> [w3261]
                  tunnel: w3112 -> [w3274]
                  tunnel: [w3274] -> w3107
                  tunnel: w3111 -> [w3273]
                  tunnel: [w3273] -> w3108
                  tunnel: w3110 -> [w3272]
                  tunnel: [w3272] -> w3109
                  tunnel: w3109 -> [w3277]
                  tunnel: w3108 -> [w3279]
                  tunnel: w3107 -> [w3278]
                  tunnel: [w3276] -> w3078
                  tunnel: [w3275] -> w3077
                  frame #0 {
                    n1523 = property on="OP" class="Bool (strict)"(error in=w3232) -> ("Value"=w3231:bool)  [unwired: 1 in, 2 out]
                    n1524 = case shown="False" w3231 {
                      tunnel: [w3253 w3255] -> w3249
                      frame False {
                        n1525 = property on="GVposition SP 15360000" class="DigNum (strict)"() -> ("Value"=w3253:i64)  [unwired: 2 in, 2 out]
                      }
                      frame True {
                        n1526 = property on="Z Step SP" class="DigNum (strict)"() -> ("Maximum"=w3254:dbl)  [unwired: 2 in, 2 out]
                        n1527 = To Long Integer(number=w3254) -> (32bit integer=w3255:i32)
                      }
                    }
                    n1528 = property on="Z Step SP" class="DigNum (strict)"() -> ("Minimum"=w3238:dbl)  [unwired: 2 in, 2 out]
                    n1529 = property on="Z steps/rev" class="DigNum (strict)"() -> ("Value"=w3242:u32)  [unwired: 2 in, 2 out]
                    n1530 = property on="Z offset mm" class="DigNum (strict)"() -> ("Value"=w3240:dbl)  [unwired: 2 in, 2 out]
                    n1531 = To Long Integer(number=w3238) -> (32bit integer=w3250:i32)
                    n1532 = To Double Precision Float(number=w3242) -> (double precision float=w3248:dbl)
                    n1533 = call "mDrive Send Command.vi"("error in (no error)"=w3232, "Extra"="P", "Command"=T10."Print Parameter", "VISA resource name"=w3237) -> ("error out"=w3234:errorcluster, "read buffer"=w3252:string, "VISA resource name out"=w3235:refnum<visa-resource-name>)  [unwired: 3 in]
                    n1534 = Decimal String To Number(string=w3252, offset=0) -> (number=w3233:i32)  [unwired: 1 in, 1 out]
                    n1535 = property on="Z Step PV" class="DigNum (strict)"("Val(Sgnl)"=w3233) -> ()  [unwired: 2 in, 2 out]
                    n1536 = In Range and Coerce(upper limit=w3249, x=w3233, lower limit=w3250) -> (In Range?=w3243:bool)  [unwired: 1 out]
                    n1537 = To Double Precision Float(number=w3233) -> (double precision float=w3246:dbl)
                    n1538 = property on="Z in Range" class="Bool (strict)"("Val(Sgnl)"=w3243) -> ()  [unwired: 2 in, 2 out]
                    n1539 = Divide(x=w3246, y=w3248) -> (x/y=w3247:dbl)
                    n1540 = property on="Z mm/rev" class="DigNum (strict)"() -> ("Value"=w3241:dbl)  [unwired: 2 in, 2 out]
                    n1541 = Multiply(x=w3247, y=w3241) -> (x*y=w3236:dbl)
                    n1542 = Add(x=w3236, y=w3240) -> (x+y=w3239:dbl)
                    n1543 = property on="Z Position mm PV" class="DigNum (strict)"("Val(Sgnl)"=w3239) -> ()  [unwired: 2 in, 2 out]
                  }
                  frame #1 {
                    n1544 = call "mDrive Send Command.vi"("error in (no error)"=w3261, "Extra"="MV", "Command"=T10."Print Parameter", "VISA resource name"=w3262) -> ("error out"=w3264:errorcluster, "read buffer"=w3267:string, "VISA resource name out"=w3265:refnum<visa-resource-name>)  [unwired: 3 in]
                    n1545 = Decimal String To Number(string=w3267, offset=0 ("offset (0)")) -> (number=w3257:i32)  [unwired: 1 in, 1 out]
                    n1546 = Not Equal?(x=w3267, y="") -> (x != y?=w3260:bool)
                    n1547 = property on="Z Ready" class="Bool (strict)"("Val(Sgnl)"=w3260) -> ()  [unwired: 2 in, 2 out]
                    n1548 = Number To Boolean Array(number=w3257) -> (Boolean array=w3259:bool[])
                    n1549 = Index Array(array=w3259, index=0) -> (element=w3256:bool)
                    n1550 = property on="Z in Motion" class="Bool (strict)"("Val(Sgnl)"=w3256) -> ()  [unwired: 2 in, 2 out]
                  }
                  frame #2 {
                    n1551 = Wait (ms)(milliseconds to wait=u32 10) -> ()  [unwired: 1 out]
                  }
                  frame #3 {
                    n1552 = case shown="False" w3277 {
                      tunnel: w3278 -> [w3282 w3286]
                      tunnel: [w3283 w3286] -> w3276
                      tunnel: [w3284 w3285] -> w3275
                      tunnel: w3279 -> [w3281 w3285]
                      frame False {
                        n1553 = call "mDrive Send Command.vi"("error in (no error)"=w3281, "Command"=T10."Stop", "VISA resource name"=w3282) -> ("error out"=w3284:errorcluster, "VISA resource name out"=w3283:refnum<visa-resource-name>)  [unwired: 4 in, 1 out]
                      }
                      frame True {
                      }
                    }
                  }
                }
                n1554 = flat-sequence {
                  tunnel: [w3292] -> w3124
                  tunnel: [w3291] -> w3123
                  tunnel: [w3290] -> w3122
                  tunnel: w3088 -> [w3289]
                  tunnel: w3087 -> [w3288]
                  tunnel: [w3314] -> w3121
                  tunnel: [w3313] -> w3120
                  tunnel: [w3311] -> w3119
                  tunnel: w3124 -> [w3311]
                  tunnel: w3123 -> [w3310]
                  tunnel: w3122 -> [w3309]
                  tunnel: w3121 -> [w3327]
                  tunnel: [w3327] -> w3116
                  tunnel: w3120 -> [w3326]
                  tunnel: [w3326] -> w3117
                  tunnel: w3119 -> [w3325]
                  tunnel: [w3325] -> w3118
                  tunnel: w3118 -> [w3330]
                  tunnel: w3117 -> [w3332]
                  tunnel: w3116 -> [w3331]
                  tunnel: [w3329] -> w3076
                  tunnel: [w3328] -> w3075
                  frame #0 {
                    n1555 = property on="X Step SP" class="DigNum (strict)"() -> ("Maximum"=w3304:dbl)  [unwired: 2 in, 2 out]
                    n1556 = property on="X Step SP" class="DigNum (strict)"() -> ("Minimum"=w3306:dbl)  [unwired: 2 in, 2 out]
                    n1557 = property on="X steps/rev" class="DigNum (strict)"() -> ("Value"=w3301:u32)  [unwired: 2 in, 2 out]
                    n1558 = property on="X offset mm" class="DigNum (strict)"() -> ("Value"=w3297:dbl)  [unwired: 2 in, 2 out]
                    n1559 = To Long Integer(number=w3304) -> (32bit integer=w3303:i32)
                    n1560 = To Long Integer(number=w3306) -> (32bit integer=w3305:i32)
                    n1561 = To Double Precision Float(number=w3301) -> (double precision float=w3302:dbl)
                    n1562 = call "mDrive Send Command.vi"("error in (no error)"=w3288, "Extra"="P", "Command"=T10."Print Parameter", "VISA resource name"=w3289) -> ("error out"=w3290:errorcluster, "read buffer"=w3308:string, "VISA resource name out"=w3291:refnum<visa-resource-name>)  [unwired: 3 in]
                    n1563 = Decimal String To Number(string=w3308, offset=0) -> (number=w3287:i32)  [unwired: 1 in, 1 out]
                    n1564 = property on="X Step PV" class="DigNum (strict)"("Val(Sgnl)"=w3287) -> ()  [unwired: 2 in, 2 out]
                    n1565 = In Range and Coerce(upper limit=w3303, x=w3287, lower limit=w3305) -> (In Range?=w3292:bool)  [unwired: 1 out]
                    n1566 = To Double Precision Float(number=w3287) -> (double precision float=w3296:dbl)
                    n1567 = property on="X  in Range" class="Bool (strict)"("Val(Sgnl)"=w3292) -> ()  [unwired: 2 in, 2 out]
                    n1568 = Divide(x=w3296, y=w3302) -> (x/y=w3300:dbl)
                    n1569 = property on="X mm/rev" class="DigNum (strict)"() -> ("Value"=w3299:dbl)  [unwired: 2 in, 2 out]
                    n1570 = Multiply(x=w3300, y=w3299) -> (x*y=w3298:dbl)
                    n1571 = Add(x=w3298, y=w3297) -> (x+y=w3295:dbl)
                    n1572 = property on="X Position mm PV" class="DigNum (strict)"("Val(Sgnl)"=w3295) -> ()  [unwired: 2 in, 2 out]
                  }
                  frame #1 {
                    n1573 = call "mDrive Send Command.vi"("error in (no error)"=w3309, "Extra"="MV", "Command"=T10."Print Parameter", "VISA resource name"=w3310) -> ("error out"=w3313:errorcluster, "read buffer"=w3317:string, "VISA resource name out"=w3314:refnum<visa-resource-name>)  [unwired: 3 in]
                    n1574 = Decimal String To Number(string=w3317, offset=0 ("offset (0)")) -> (number=w3320:i32)  [unwired: 1 in, 1 out]
                    n1575 = Not Equal?(x=w3317, y="") -> (x != y?=w3315:bool)
                    n1576 = property on="X Ready" class="Bool (strict)"("Val(Sgnl)"=w3315) -> ()  [unwired: 2 in, 2 out]
                    n1577 = Number To Boolean Array(number=w3320) -> (Boolean array=w3319:bool[])
                    n1578 = Index Array(array=w3319, index=0) -> (element=w3312:bool)
                    n1579 = property on="X  in Motion" class="Bool (strict)"("Val(Sgnl)"=w3312) -> ()  [unwired: 2 in, 2 out]
                  }
                  frame #2 {
                    n1580 = Wait (ms)(milliseconds to wait=u32 10) -> ()  [unwired: 1 out]
                  }
                  frame #3 {
                    n1581 = case shown="False" w3330 {
                      tunnel: w3331 -> [w3335 w3339]
                      tunnel: [w3336 w3339] -> w3329
                      tunnel: [w3337 w3338] -> w3328
                      tunnel: w3332 -> [w3334 w3338]
                      frame False {
                        n1582 = call "mDrive Send Command.vi"("error in (no error)"=w3334, "Command"=T10."Stop", "VISA resource name"=w3335) -> ("error out"=w3337:errorcluster, "VISA resource name out"=w3336:refnum<visa-resource-name>)  [unwired: 4 in, 1 out]
                      }
                      frame True {
                      }
                    }
                  }
                }
                n1583 = flat-sequence {
                  tunnel: [w3187] -> w3106
                  tunnel: [w3189] -> w3105
                  tunnel: [w3188] -> w3104
                  tunnel: w3084 -> [w3180]
                  tunnel: w3083 -> [w3179]
                  tunnel: [w3209] -> w3103
                  tunnel: [w3208] -> w3102
                  tunnel: [w3207] -> w3101
                  tunnel: w3106 -> [w3207]
                  tunnel: w3105 -> [w3206]
                  tunnel: w3104 -> [w3205]
                  tunnel: w3103 -> [w3218]
                  tunnel: [w3218] -> w3098
                  tunnel: w3102 -> [w3217]
                  tunnel: [w3217] -> w3099
                  tunnel: w3101 -> [w3216]
                  tunnel: [w3216] -> w3100
                  tunnel: w3100 -> [w3221]
                  tunnel: w3099 -> [w3223]
                  tunnel: w3098 -> [w3222]
                  tunnel: [w3219] -> w3074
                  tunnel: [w3220] -> w3073
                  frame #0 {
                    n1584 = property on="Y Step SP" class="DigNum (strict)"() -> ("Maximum"=w3182:dbl)  [unwired: 2 in, 2 out]
                    n1585 = property on="Y Step SP" class="DigNum (strict)"() -> ("Minimum"=w3181:dbl)  [unwired: 2 in, 2 out]
                    n1586 = property on="Y steps/rev" class="DigNum (strict)"() -> ("Value"=w3183:u32)  [unwired: 2 in, 2 out]
                    n1587 = property on="Y offset mm" class="DigNum (strict)"() -> ("Value"=w3185:dbl)  [unwired: 2 in, 2 out]
                    n1588 = To Long Integer(number=w3182) -> (32bit integer=w3196:i32)
                    n1589 = To Long Integer(number=w3181) -> (32bit integer=w3197:i32)
                    n1590 = To Double Precision Float(number=w3183) -> (double precision float=w3195:dbl)
                    n1591 = call "mDrive Send Command.vi"("error in (no error)"=w3179, "Extra"="P", "Command"=T10."Print Parameter", "VISA resource name"=w3180) -> ("error out"=w3188:errorcluster, "read buffer"=w3199:string, "VISA resource name out"=w3189:refnum<visa-resource-name>)  [unwired: 3 in]
                    n1592 = Decimal String To Number(string=w3199, offset=0) -> (number=w3178:i32)  [unwired: 1 in, 1 out]
                    n1593 = property on="Y Step PV" class="DigNum (strict)"("Val(Sgnl)"=w3178) -> ()  [unwired: 2 in, 2 out]
                    n1594 = In Range and Coerce(upper limit=w3196, x=w3178, lower limit=w3197) -> (In Range?=w3187:bool)  [unwired: 1 out]
                    n1595 = To Double Precision Float(number=w3178) -> (double precision float=w3192:dbl)
                    n1596 = property on="Y in Range" class="Bool (strict)"("Val(Sgnl)"=w3187) -> ()  [unwired: 2 in, 2 out]
                    n1597 = Divide(x=w3192, y=w3195) -> (x/y=w3194:dbl)
                    n1598 = property on="Y mm/rev" class="DigNum (strict)"() -> ("Value"=w3184:dbl)  [unwired: 2 in, 2 out]
                    n1599 = Multiply(x=w3194, y=w3184) -> (x*y=w3193:dbl)
                    n1600 = Add(x=w3193, y=w3185) -> (x+y=w3186:dbl)
                    n1601 = property on="Y Position mm PV" class="DigNum (strict)"("Val(Sgnl)"=w3186) -> ()  [unwired: 2 in, 2 out]
                  }
                  frame #1 {
                    n1602 = call "mDrive Send Command.vi"("error in (no error)"=w3205, "Extra"="MV", "Command"=T10."Print Parameter", "VISA resource name"=w3206) -> ("error out"=w3208:errorcluster, "read buffer"=w3211:string, "VISA resource name out"=w3209:refnum<visa-resource-name>)  [unwired: 3 in]
                    n1603 = Decimal String To Number(string=w3211, offset=0 ("offset (0)")) -> (number=w3201:i32)  [unwired: 1 in, 1 out]
                    n1604 = Not Equal?(x=w3211, y="") -> (x != y?=w3204:bool)
                    n1605 = property on="Y Ready" class="Bool (strict)"("Val(Sgnl)"=w3204) -> ()  [unwired: 2 in, 2 out]
                    n1606 = Number To Boolean Array(number=w3201) -> (Boolean array=w3203:bool[])
                    n1607 = Index Array(array=w3203, index=0) -> (element=w3200:bool)
                    n1608 = property on="Y in Motion" class="Bool (strict)"("Val(Sgnl)"=w3200) -> ()  [unwired: 2 in, 2 out]
                  }
                  frame #2 {
                    n1609 = Wait (ms)(milliseconds to wait=u32 10) -> ()  [unwired: 1 out]
                  }
                  frame #3 {
                    n1610 = case shown="False" w3221 {
                      tunnel: w3222 -> [w3226 w3229]
                      tunnel: [w3227 w3229] -> w3219
                      tunnel: [w3228 w3230] -> w3220
                      tunnel: w3223 -> [w3225 w3230]
                      frame False {
                        n1611 = call "mDrive Send Command.vi"("error in (no error)"=w3225, "Command"=T10."Stop", "VISA resource name"=w3226) -> ("error out"=w3228:errorcluster, "VISA resource name out"=w3227:refnum<visa-resource-name>)  [unwired: 4 in, 1 out]
                      }
                      frame True {
                      }
                    }
                  }
                }
                n1612 = flat-sequence {
                  tunnel: [w3134] -> w3097
                  tunnel: [w3136] -> w3096
                  tunnel: [w3135] -> w3095
                  tunnel: w3082 -> [w3127]
                  tunnel: w3081 -> [w3126]
                  tunnel: [w3156] -> w3094
                  tunnel: [w3155] -> w3093
                  tunnel: [w3154] -> w3092
                  tunnel: w3097 -> [w3154]
                  tunnel: w3096 -> [w3153]
                  tunnel: w3095 -> [w3152]
                  tunnel: w3094 -> [w3165]
                  tunnel: [w3165] -> w3089
                  tunnel: w3093 -> [w3164]
                  tunnel: [w3164] -> w3090
                  tunnel: w3092 -> [w3163]
                  tunnel: [w3163] -> w3091
                  tunnel: w3091 -> [w3168]
                  tunnel: w3090 -> [w3170]
                  tunnel: w3089 -> [w3169]
                  tunnel: [w3167] -> w3072
                  tunnel: [w3166] -> w3071
                  frame #0 {
                    n1613 = property on="R Step SP" class="DigNum (strict)"() -> ("Maximum"=w3129:dbl)  [unwired: 2 in, 2 out]
                    n1614 = property on="R Step SP" class="DigNum (strict)"() -> ("Minimum"=w3130:dbl)  [unwired: 2 in, 2 out]
                    n1615 = property on="R steps/rev" class="DigNum (strict)"() -> ("Value"=w3128:u32)  [unwired: 2 in, 2 out]
                    n1616 = property on="R offset deg" class="DigNum (strict)"() -> ("Value"=w3132:dbl)  [unwired: 2 in, 2 out]
                    n1617 = To Long Integer(number=w3129) -> (32bit integer=w3143:i32)
                    n1618 = To Long Integer(number=w3130) -> (32bit integer=w3144:i32)
                    n1619 = To Double Precision Float(number=w3128) -> (double precision float=w3142:dbl)
                    n1620 = call "mDrive Send Command.vi"("error in (no error)"=w3126, "Extra"="P", "Command"=T10."Print Parameter", "VISA resource name"=w3127) -> ("error out"=w3135:errorcluster, "read buffer"=w3146:string, "VISA resource name out"=w3136:refnum<visa-resource-name>)  [unwired: 3 in]
                    n1621 = Decimal String To Number(string=w3146, offset=0) -> (number=w3125:i32)  [unwired: 1 in, 1 out]
                    n1622 = property on="R Step PV" class="DigNum (strict)"("Val(Sgnl)"=w3125) -> ()  [unwired: 2 in, 2 out]
                    n1623 = In Range and Coerce(upper limit=w3143, x=w3125, lower limit=w3144) -> (In Range?=w3134:bool)  [unwired: 1 out]
                    n1624 = To Double Precision Float(number=w3125) -> (double precision float=w3139:dbl)
                    n1625 = property on="R in Range" class="Bool (strict)"("Val(Sgnl)"=w3134) -> ()  [unwired: 2 in, 2 out]
                    n1626 = Divide(x=w3139, y=w3142) -> (x/y=w3141:dbl)
                    n1627 = property on="R deg/rev" class="DigNum (strict)"() -> ("Value"=w3131:dbl)  [unwired: 2 in, 2 out]
                    n1628 = Multiply(x=w3141, y=w3131) -> (x*y=w3140:dbl)
                    n1629 = Add(x=w3140, y=w3132) -> (x+y=w3133:dbl)
                    n1630 = property on="R Position deg PV" class="DigNum (strict)"("Val(Sgnl)"=w3133) -> ()  [unwired: 2 in, 2 out]
                  }
                  frame #1 {
                    n1631 = call "mDrive Send Command.vi"("error in (no error)"=w3152, "Extra"="MV", "Command"=T10."Print Parameter", "VISA resource name"=w3153) -> ("error out"=w3155:errorcluster, "read buffer"=w3158:string, "VISA resource name out"=w3156:refnum<visa-resource-name>)  [unwired: 3 in]
                    n1632 = Decimal String To Number(string=w3158, offset=0 ("offset (0)")) -> (number=w3148:i32)  [unwired: 1 in, 1 out]
                    n1633 = Not Equal?(x=w3158, y="") -> (x != y?=w3151:bool)
                    n1634 = property on="R Ready" class="Bool (strict)"("Val(Sgnl)"=w3151) -> ()  [unwired: 2 in, 2 out]
                    n1635 = Number To Boolean Array(number=w3148) -> (Boolean array=w3150:bool[])
                    n1636 = Index Array(array=w3150, index=0) -> (element=w3147:bool)
                    n1637 = property on="R in Motion" class="Bool (strict)"("Val(Sgnl)"=w3147) -> ()  [unwired: 2 in, 2 out]
                  }
                  frame #2 {
                    n1638 = Wait (ms)(milliseconds to wait=u32 10) -> ()  [unwired: 1 out]
                  }
                  frame #3 {
                    n1639 = case shown="False" w3168 {
                      tunnel: w3169 -> [w3173 w3177]
                      tunnel: [w3174 w3177] -> w3167
                      tunnel: [w3175 w3176] -> w3166
                      tunnel: w3170 -> [w3172 w3176]
                      frame False {
                        n1640 = call "mDrive Send Command.vi"("error in (no error)"=w3172, "Command"=T10."Stop", "VISA resource name"=w3173) -> ("error out"=w3175:errorcluster, "VISA resource name out"=w3174:refnum<visa-resource-name>)  [unwired: 4 in, 1 out]
                      }
                      frame True {
                      }
                    }
                  }
                }
                n1641 = property on="Y in Motion" class="Bool (strict)"() -> ("Value"=w3080:bool)  [unwired: 2 in, 2 out]
                n1642 = property on="Z in Motion" class="Bool (strict)"() -> ("Value"=w3070:bool)  [unwired: 2 in, 2 out]
                n1643 = property on="X  in Motion" class="Bool (strict)"() -> ("Value"=w3079:bool)  [unwired: 2 in, 2 out]
                n1644 = property on="R in Motion" class="Bool (strict)"() -> ("Value"=w3069:bool)  [unwired: 2 in, 2 out]
                n1645 = Compound Arithmetic op=OR(w3079, w3080, w3070, w3069) -> (w3068:bool)
                n1646 = Not(x=w3068) -> (.not. x?=w3067:bool)
              }
            }
            frame #4 {
              n1647 = Wait (ms)(milliseconds to wait=u32 300) -> ()  [unwired: 1 out]
            }
            frame #5 {
              w3349 = TRUE ("R in Motion")
              n1648 = property on="X Position mm PV" class="DigNum (strict)"() -> ("Value"=w3378:dbl)  [unwired: 2 in, 2 out]
              n1649 = property on="X Position SP mm" class="DigNum (strict)"() -> ("Value"=w3377:dbl)  [unwired: 2 in, 2 out]
              n1650 = property on="Z Position mm PV" class="DigNum (strict)"() -> ("Value"=w3374:dbl)  [unwired: 2 in, 2 out]
              n1651 = property on="Z Position SP mm" class="DigNum (strict)"() -> ("Value"=w3367:dbl)  [unwired: 2 in, 2 out]
              n1652 = property on="Y Position mm PV" class="DigNum (strict)"() -> ("Value"=w3372:dbl)  [unwired: 2 in, 2 out]
              n1653 = property on="Y Position SP mm" class="DigNum (strict)"() -> ("Value"=w3371:dbl)  [unwired: 2 in, 2 out]
              n1654 = property on="R Position SP deg" class="DigNum (strict)"() -> ("Value"=w3369:dbl)  [unwired: 2 in, 2 out]
              n1655 = property on="R Position deg PV" class="DigNum (strict)"() -> ("Value"=w3368:dbl)  [unwired: 2 in, 2 out]
              n1656 = local write "STATUS"("LOOP HOMING" ("STATUS")) -> ()
              n1657 = Not Equal?(x=w3378, y=w3377) -> (x != y?=w3376:bool)
              n1658 = Not Equal?(x=w3374, y=w3367) -> (x != y?=w3375:bool)
              n1659 = Not Equal?(x=w3372, y=w3371) -> (x != y?=w3373:bool)
              n1660 = Not Equal?(x=w3369, y=w3368) -> (x != y?=w3370:bool)
              n1661 = case shown="True" w3376 {
                tunnel: w3366 -> [w3590 w3594]
                tunnel: w3364 -> [w3589 w3593]
                tunnel: [w3590 w3592] -> w3351
                tunnel: [w3589 w3591] -> w3352
                frame False {
                }
                frame True {
                  n1662 = flat-sequence {
                    tunnel: w3593 -> [w3609]
                    tunnel: w3594 -> [w3622]
                    tunnel: [w3622] -> w3608
                    tunnel: [w3609] -> w3607
                    tunnel: [w3611] -> w3606
                    tunnel: [w3625] -> w3605
                    tunnel: [w3624] -> w3604
                    tunnel: [w3623] -> w3603
                    tunnel: w3606 -> [w3623]
                    tunnel: w3607 -> [w3624]
                    tunnel: w3608 -> [w3625]
                    tunnel: [w3641] -> w3602
                    tunnel: [w3640] -> w3601
                    tunnel: w3605 -> [w3639]
                    tunnel: w3604 -> [w3638]
                    tunnel: w3603 -> [w3637]
                    tunnel: [w3637] -> w3600
                    tunnel: w3602 -> [w3648]
                    tunnel: [w3648] -> w3599
                    tunnel: w3601 -> [w3647]
                    tunnel: [w3647] -> w3598
                    tunnel: [w3645] -> w3597
                    tunnel: w3600 -> [w3645]
                    tunnel: [w3653] -> w3596
                    tunnel: [w3652] -> w3595
                    tunnel: w3599 -> [w3651]
                    tunnel: w3598 -> [w3650]
                    tunnel: w3597 -> [w3649]
                    tunnel: [w3657] -> w3591
                    tunnel: [w3658] -> w3592
                    tunnel: w3596 -> [w3658]
                    tunnel: w3595 -> [w3657]
                    frame #0 {
                      n1663 = property on="X steps/rev" class="DigNum (strict)"() -> ("Value"=w3621:u32)  [unwired: 2 in, 2 out]
                      n1664 = To Double Precision Float(number=w3621) -> (double precision float=w3616:dbl)
                      n1665 = property on="X offset mm" class="DigNum (strict)"() -> ("Value"=w3620:dbl)  [unwired: 2 in, 2 out]
                      n1666 = property on="X Position SP mm" class="DigNum (strict)"() -> ("Value"=w3619:dbl)  [unwired: 2 in, 2 out]
                      n1667 = Subtract(x=w3619, y=w3620) -> (x-y=w3613:dbl)
                      n1668 = property on="X mm/rev" class="DigNum (strict)"() -> ("Value"=w3610:dbl)  [unwired: 2 in, 2 out]
                      n1669 = Divide(x=w3613, y=w3610) -> (x/y=w3612:dbl)
                      n1670 = property on="X Step SP" class="DigNum (strict)"() -> ("Maximum"=w3618:dbl)  [unwired: 2 in, 2 out]
                      n1671 = property on="X Step SP" class="DigNum (strict)"() -> ("Minimum"=w3617:dbl)  [unwired: 2 in, 2 out]
                      n1672 = Multiply(x=w3612, y=w3616) -> (x*y=w3614:dbl)
                      n1673 = In Range and Coerce(upper limit=w3618, x=w3614, lower limit=w3617) -> (coerced(x)=w3615:dbl)  [unwired: 1 out]
                      n1674 = To Long Integer(number=w3615) -> (32bit integer=w3611:i32)
                      n1675 = property on="X Step SP" class="DigNum (strict)"("Val(Sgnl)"=w3611) -> ()  [unwired: 2 in, 2 out]
                    }
                    frame #1 {
                      n1676 = property on="X Step SP" class="DigNum (strict)"() -> ("Value"=w3634:i32)  [unwired: 2 in, 2 out]
                      n1677 = property on="X Step PV" class="DigNum (strict)"() -> ("Value"=w3633:i32)  [unwired: 2 in, 2 out]
                      n1678 = property on="X Backlash" class="DigNum (strict)"() -> ("Value"=w3626:i32)  [unwired: 2 in, 2 out]
                      n1679 = Subtract(x=w3634, y=w3633) -> (x-y=w3632:i32)
                      n1680 = Sign(1:w3626) -> (0:w3630:i32)
                      n1681 = Sign(1:w3632) -> (0:w3631:i32)
                      n1682 = Multiply(x=w3631, y=w3630) -> (x*y=w3629:i32)
                      n1683 = Equal?(x=w3629, y=1) -> (x = y?=w3627:bool)
                      n1684 = case shown="True" w3627 {
                        frame False {
                          n1685 = property on="X Backlash corr" class="Bool (strict)"("Val(Sgnl)"=FALSE ("Value (Signaling)")) -> ()  [unwired: 2 in, 2 out]
                        }
                        frame True {
                          n1686 = property on="X Backlash corr" class="Bool (strict)"("Val(Sgnl)"=TRUE ("Value (Signaling)")) -> ()  [unwired: 2 in, 2 out]
                        }
                      }
                    }
                    frame #2 {
                      # "Velocity Setting"
                      n1687 = property on="X Velocity SP step/sec" class="DigNum (strict)"() -> ("Value"=w3642:i32)  [unwired: 2 in, 2 out]
                      n1688 = Number To Decimal String(number=w3642) -> (decimal integer string=w3643:string)  [unwired: 1 in]
                      n1689 = call "mDrive Send Command.vi"("error in (no error)"=w3638, "Extra"=w3643, "Command"=T10."Max Velocity", "VISA resource name"=w3639) -> ("error out"=w3640:errorcluster, "VISA resource name out"=w3641:refnum<visa-resource-name>)  [unwired: 3 in, 1 out]
                    }
                    frame #3 {
                      n1690 = Wait (ms)(milliseconds to wait=u32 50) -> ()  [unwired: 1 out]
                    }
                    frame #4 {
                      # "Move to Abs Position"
                      n1691 = Number To Decimal String(number=w3649) -> (decimal integer string=w3655:string)  [unwired: 1 in]
                      n1692 = call "mDrive Send Command.vi"("error in (no error)"=w3650, "Extra"=w3655, "Command"=T10."Move to Absolute Position", "VISA resource name"=w3651) -> ("error out"=w3652:errorcluster, "VISA resource name out"=w3653:refnum<visa-resource-name>)  [unwired: 3 in, 1 out]
                    }
                    frame #5 {
                      n1693 = Wait (ms)(milliseconds to wait=u32 50) -> ()  [unwired: 1 out]
                    }
                  }
                }
              }
              n1694 = case shown="True" w3375 {
                tunnel: w3363 -> [w3519 w3524]
                tunnel: w3365 -> [w3520 w3523]
                tunnel: [w3520 w3522] -> w3353
                tunnel: [w3519 w3521] -> w3354
                frame False {
                }
                frame True {
                  n1695 = flat-sequence {
                    tunnel: [w3552] -> w3538
                    tunnel: [w3551] -> w3537
                    tunnel: [w3540] -> w3536
                    tunnel: w3524 -> [w3552]
                    tunnel: w3523 -> [w3551]
                    tunnel: [w3555] -> w3535
                    tunnel: [w3554] -> w3534
                    tunnel: [w3553] -> w3533
                    tunnel: w3536 -> [w3553]
                    tunnel: w3537 -> [w3554]
                    tunnel: w3538 -> [w3555]
                    tunnel: [w3571] -> w3532
                    tunnel: [w3570] -> w3531
                    tunnel: w3535 -> [w3569]
                    tunnel: w3534 -> [w3568]
                    tunnel: [w3567] -> w3530
                    tunnel: w3533 -> [w3567]
                    tunnel: w3532 -> [w3578]
                    tunnel: [w3578] -> w3529
                    tunnel: w3531 -> [w3577]
                    tunnel: [w3577] -> w3528
                    tunnel: w3530 -> [w3576]
                    tunnel: [w3576] -> w3527
                    tunnel: [w3583] -> w3526
                    tunnel: [w3582] -> w3525
                    tunnel: w3529 -> [w3581]
                    tunnel: w3528 -> [w3580]
                    tunnel: w3527 -> [w3579]
                    tunnel: [w3587] -> w3521
                    tunnel: [w3588] -> w3522
                    tunnel: w3526 -> [w3588]
                    tunnel: w3525 -> [w3587]
                    frame #0 {
                      n1696 = property on="Z steps/rev" class="DigNum (strict)"() -> ("Value"=w3539:u32)  [unwired: 2 in, 2 out]
                      n1697 = To Double Precision Float(number=w3539) -> (double precision float=w3545:dbl)
                      n1698 = property on="Z offset mm" class="DigNum (strict)"() -> ("Value"=w3547:dbl)  [unwired: 2 in, 2 out]
                      n1699 = property on="Z Position SP mm" class="DigNum (strict)"() -> ("Value"=w3546:dbl)  [unwired: 2 in, 2 out]
                      n1700 = Subtract(x=w3546, y=w3547) -> (x-y=w3542:dbl)
                      n1701 = property on="Z mm/rev" class="DigNum (strict)"() -> ("Value"=w3548:dbl)  [unwired: 2 in, 2 out]
                      n1702 = Divide(x=w3542, y=w3548) -> (x/y=w3541:dbl)
                      n1703 = property on="Z Step SP" class="DigNum (strict)"() -> ("Maximum"=w3550:dbl)  [unwired: 2 in, 2 out]
                      n1704 = property on="Z Step SP" class="DigNum (strict)"() -> ("Minimum"=w3549:dbl)  [unwired: 2 in, 2 out]
                      n1705 = Multiply(x=w3541, y=w3545) -> (x*y=w3543:dbl)
                      n1706 = In Range and Coerce(upper limit=w3550, x=w3543, lower limit=w3549) -> (coerced(x)=w3544:dbl)  [unwired: 1 out]
                      n1707 = To Long Integer(number=w3544) -> (32bit integer=w3540:i32)
                      n1708 = property on="Z Step SP" class="DigNum (strict)"("Val(Sgnl)"=w3540) -> ()  [unwired: 2 in, 2 out]
                    }
                    frame #1 {
                      n1709 = property on="Z Step SP" class="DigNum (strict)"() -> ("Value"=w3564:i32)  [unwired: 2 in, 2 out]
                      n1710 = property on="Z Backlash" class="DigNum (strict)"() -> ("Value"=w3556:i32)  [unwired: 2 in, 2 out]
                      n1711 = property on="Z Step PV" class="DigNum (strict)"() -> ("Value"=w3563:i32)  [unwired: 2 in, 2 out]
                      n1712 = Subtract(x=w3564, y=w3563) -> (x-y=w3562:i32)
                      n1713 = Sign(1:w3556) -> (0:w3560:i32)
                      n1714 = Sign(1:w3562) -> (0:w3561:i32)
                      n1715 = Multiply(x=w3561, y=w3560) -> (x*y=w3559:i32)
                      n1716 = Equal?(x=w3559, y=1) -> (x = y?=w3557:bool)
                      n1717 = case shown="False" w3557 {
                        frame False {
                          n1718 = property on="Z Backlash corr" class="Bool (strict)"("Val(Sgnl)"=FALSE ("Value (Signaling)")) -> ()  [unwired: 2 in, 2 out]
                        }
                        frame True {
                          n1719 = property on="Z Backlash corr" class="Bool (strict)"("Val(Sgnl)"=TRUE ("Value (Signaling)")) -> ()  [unwired: 2 in, 2 out]
                        }
                      }
                    }
                    frame #2 {
                      # "Velocity Setting"
                      n1720 = property on="Z Velocity SP step/sec" class="DigNum (strict)"() -> ("Value"=w3572:i32)  [unwired: 2 in, 2 out]
                      n1721 = Number To Decimal String(number=w3572) -> (decimal integer string=w3573:string)  [unwired: 1 in]
                      n1722 = call "mDrive Send Command.vi"("error in (no error)"=w3569, "Extra"=w3573, "Command"=T10."Max Velocity", "VISA resource name"=w3568) -> ("error out"=w3570:errorcluster, "VISA resource name out"=w3571:refnum<visa-resource-name>)  [unwired: 3 in, 1 out]
                    }
                    frame #3 {
                      n1723 = Wait (ms)(milliseconds to wait=u32 50) -> ()  [unwired: 1 out]
                    }
                    frame #4 {
                      # "Move to Abs Position"
                      n1724 = Number To Decimal String(number=w3579) -> (decimal integer string=w3585:string)  [unwired: 1 in]
                      n1725 = call "mDrive Send Command.vi"("error in (no error)"=w3580, "Extra"=w3585, "Command"=T10."Move to Absolute Position", "VISA resource name"=w3581) -> ("error out"=w3582:errorcluster, "VISA resource name out"=w3583:refnum<visa-resource-name>)  [unwired: 3 in, 1 out]
                    }
                    frame #5 {
                      n1726 = Wait (ms)(milliseconds to wait=u32 50) -> ()  [unwired: 1 out]
                    }
                  }
                }
              }
              n1727 = case shown="True" w3373 {
                tunnel: w3361 -> [w3449 w3454]
                tunnel: w3362 -> [w3450 w3453]
                tunnel: [w3450 w3452] -> w3355
                tunnel: [w3449 w3451] -> w3356
                frame False {
                }
                frame True {
                  n1728 = flat-sequence {
                    tunnel: [w3482] -> w3468
                    tunnel: [w3481] -> w3467
                    tunnel: [w3469] -> w3466
                    tunnel: w3453 -> [w3481]
                    tunnel: w3454 -> [w3482]
                    tunnel: [w3485] -> w3465
                    tunnel: [w3484] -> w3464
                    tunnel: [w3483] -> w3463
                    tunnel: w3466 -> [w3483]
                    tunnel: w3467 -> [w3484]
                    tunnel: w3468 -> [w3485]
                    tunnel: [w3501] -> w3462
                    tunnel: [w3500] -> w3461
                    tunnel: w3465 -> [w3499]
                    tunnel: w3464 -> [w3498]
                    tunnel: [w3497] -> w3460
                    tunnel: w3463 -> [w3497]
                    tunnel: w3462 -> [w3508]
                    tunnel: [w3508] -> w3459
                    tunnel: w3461 -> [w3507]
                    tunnel: [w3507] -> w3458
                    tunnel: [w3505] -> w3457
                    tunnel: w3460 -> [w3505]
                    tunnel: [w3513] -> w3456
                    tunnel: [w3512] -> w3455
                    tunnel: w3459 -> [w3511]
                    tunnel: w3458 -> [w3510]
                    tunnel: w3457 -> [w3509]
                    tunnel: [w3516] -> w3451
                    tunnel: [w3518] -> w3452
                    tunnel: w3456 -> [w3518]
                    tunnel: w3455 -> [w3516]
                    frame #0 {
                      n1729 = property on="Y steps/rev" class="DigNum (strict)"() -> ("Value"=w3478:u32)  [unwired: 2 in, 2 out]
                      n1730 = To Double Precision Float(number=w3478) -> (double precision float=w3474:dbl)
                      n1731 = property on="Y offset mm" class="DigNum (strict)"() -> ("Value"=w3476:dbl)  [unwired: 2 in, 2 out]
                      n1732 = property on="Y Position SP mm" class="DigNum (strict)"() -> ("Value"=w3475:dbl)  [unwired: 2 in, 2 out]
                      n1733 = Subtract(x=w3475, y=w3476) -> (x-y=w3471:dbl)
                      n1734 = property on="Y mm/rev" class="DigNum (strict)"() -> ("Value"=w3477:dbl)  [unwired: 2 in, 2 out]
                      n1735 = Divide(x=w3471, y=w3477) -> (x/y=w3470:dbl)
                      n1736 = property on="Y Step SP" class="DigNum (strict)"() -> ("Maximum"=w3479:dbl)  [unwired: 2 in, 2 out]
                      n1737 = property on="Y Step SP" class="DigNum (strict)"() -> ("Minimum"=w3480:dbl)  [unwired: 2 in, 2 out]
                      n1738 = Multiply(x=w3470, y=w3474) -> (x*y=w3472:dbl)
                      n1739 = In Range and Coerce(upper limit=w3479, x=w3472, lower limit=w3480) -> (coerced(x)=w3473:dbl)  [unwired: 1 out]
                      n1740 = To Long Integer(number=w3473) -> (32bit integer=w3469:i32)
                      n1741 = property on="Y Step SP" class="DigNum (strict)"("Val(Sgnl)"=w3469) -> ()  [unwired: 2 in, 2 out]
                    }
                    frame #1 {
                      n1742 = property on="Y Step SP" class="DigNum (strict)"() -> ("Value"=w3494:i32)  [unwired: 2 in, 2 out]
                      n1743 = property on="Y Backlash" class="DigNum (strict)"() -> ("Value"=w3486:i32)  [unwired: 2 in, 2 out]
                      n1744 = property on="Y Step PV" class="DigNum (strict)"() -> ("Value"=w3493:i32)  [unwired: 2 in, 2 out]
                      n1745 = Subtract(x=w3494, y=w3493) -> (x-y=w3492:i32)
                      n1746 = Sign(1:w3486) -> (0:w3490:i32)
                      n1747 = Sign(1:w3492) -> (0:w3491:i32)
                      n1748 = Multiply(x=w3491, y=w3490) -> (x*y=w3489:i32)
                      n1749 = Equal?(x=w3489, y=1) -> (x = y?=w3487:bool)
                      n1750 = case shown="True" w3487 {
                        frame False {
                          n1751 = property on="Y Backlash corr" class="Bool (strict)"("Val(Sgnl)"=FALSE ("Value (Signaling)")) -> ()  [unwired: 2 in, 2 out]
                        }
                        frame True {
                          n1752 = property on="Y Backlash corr" class="Bool (strict)"("Val(Sgnl)"=TRUE ("Value (Signaling)")) -> ()  [unwired: 2 in, 2 out]
                        }
                      }
                    }
                    frame #2 {
                      # "Velocity Setting"
                      n1753 = property on="Y Velocity SP step/sec" class="DigNum (strict)"() -> ("Value"=w3502:i32)  [unwired: 2 in, 2 out]
                      n1754 = Number To Decimal String(number=w3502) -> (decimal integer string=w3503:string)  [unwired: 1 in]
                      n1755 = call "mDrive Send Command.vi"("error in (no error)"=w3499, "Extra"=w3503, "Command"=T10."Max Velocity", "VISA resource name"=w3498) -> ("error out"=w3500:errorcluster, "VISA resource name out"=w3501:refnum<visa-resource-name>)  [unwired: 3 in, 1 out]
                    }
                    frame #3 {
                      n1756 = Wait (ms)(milliseconds to wait=u32 50) -> ()  [unwired: 1 out]
                    }
                    frame #4 {
                      # "Move to Abs Position"
                      n1757 = Number To Decimal String(number=w3509) -> (decimal integer string=w3515:string)  [unwired: 1 in]
                      n1758 = call "mDrive Send Command.vi"("error in (no error)"=w3510, "Extra"=w3515, "Command"=T10."Move to Absolute Position", "VISA resource name"=w3511) -> ("error out"=w3512:errorcluster, "VISA resource name out"=w3513:refnum<visa-resource-name>)  [unwired: 3 in, 1 out]
                    }
                    frame #5 {
                      n1759 = Wait (ms)(milliseconds to wait=u32 25) -> ()  [unwired: 1 out]
                    }
                  }
                }
              }
              n1760 = case shown="True" w3370 {
                tunnel: w3359 -> [w3379 w3384]
                tunnel: w3360 -> [w3380 w3383]
                tunnel: [w3380 w3382] -> w3358
                tunnel: [w3379 w3381] -> w3357
                frame False {
                }
                frame True {
                  n1761 = flat-sequence {
                    tunnel: w3383 -> [w3411]
                    tunnel: w3384 -> [w3412]
                    tunnel: [w3412] -> w3398
                    tunnel: [w3411] -> w3397
                    tunnel: [w3399] -> w3396
                    tunnel: [w3415] -> w3395
                    tunnel: [w3414] -> w3394
                    tunnel: [w3413] -> w3393
                    tunnel: w3396 -> [w3413]
                    tunnel: w3397 -> [w3414]
                    tunnel: w3398 -> [w3415]
                    tunnel: [w3431] -> w3392
                    tunnel: [w3430] -> w3391
                    tunnel: w3395 -> [w3429]
                    tunnel: w3394 -> [w3428]
                    tunnel: [w3427] -> w3390
                    tunnel: w3393 -> [w3427]
                    tunnel: w3392 -> [w3438]
                    tunnel: [w3438] -> w3389
                    tunnel: w3391 -> [w3437]
                    tunnel: [w3437] -> w3388
                    tunnel: w3390 -> [w3436]
                    tunnel: [w3436] -> w3387
                    tunnel: [w3443] -> w3386
                    tunnel: [w3442] -> w3385
                    tunnel: w3389 -> [w3441]
                    tunnel: w3388 -> [w3440]
                    tunnel: w3387 -> [w3439]
                    tunnel: [w3448] -> w3382
                    tunnel: w3386 -> [w3448]
                    tunnel: w3385 -> [w3447]
                    tunnel: [w3447] -> w3381
                    frame #0 {
                      n1762 = property on="R steps/rev" class="DigNum (strict)"() -> ("Value"=w3407:u32)  [unwired: 2 in, 2 out]
                      n1763 = To Double Precision Float(number=w3407) -> (double precision float=w3404:dbl)
                      n1764 = property on="R offset deg" class="DigNum (strict)"() -> ("Value"=w3408:dbl)  [unwired: 2 in, 2 out]
                      n1765 = property on="R Position SP deg" class="DigNum (strict)"() -> ("Value"=w3409:dbl)  [unwired: 2 in, 2 out]
                      n1766 = Subtract(x=w3409, y=w3408) -> (x-y=w3401:dbl)
                      n1767 = property on="R deg/rev" class="DigNum (strict)"() -> ("Value"=w3410:dbl)  [unwired: 2 in, 2 out]
                      n1768 = Divide(x=w3401, y=w3410) -> (x/y=w3400:dbl)
                      n1769 = property on="R Step SP" class="DigNum (strict)"() -> ("Maximum"=w3405:dbl)  [unwired: 2 in, 2 out]
                      n1770 = Multiply(x=w3400, y=w3404) -> (x*y=w3402:dbl)
                      n1771 = property on="R Step SP" class="DigNum (strict)"() -> ("Minimum"=w3406:dbl)  [unwired: 2 in, 2 out]
                      n1772 = In Range and Coerce(upper limit=w3405, x=w3402, lower limit=w3406) -> (coerced(x)=w3403:dbl)  [unwired: 1 out]
                      n1773 = To Long Integer(number=w3403) -> (32bit integer=w3399:i32)
                      n1774 = property on="R Step SP" class="DigNum (strict)"("Val(Sgnl)"=w3399) -> ()  [unwired: 2 in, 2 out]
                    }
                    frame #1 {
                      n1775 = property on="R Step SP" class="DigNum (strict)"() -> ("Value"=w3424:i32)  [unwired: 2 in, 2 out]
                      n1776 = property on="R Step PV" class="DigNum (strict)"() -> ("Value"=w3423:i32)  [unwired: 2 in, 2 out]
                      n1777 = property on="R Backlash" class="DigNum (strict)"() -> ("Value"=w3416:i32)  [unwired: 2 in, 2 out]
                      n1778 = Subtract(x=w3424, y=w3423) -> (x-y=w3422:i32)
                      n1779 = Sign(1:w3416) -> (0:w3420:i32)
                      n1780 = Sign(1:w3422) -> (0:w3421:i32)
                      n1781 = Multiply(x=w3421, y=w3420) -> (x*y=w3419:i32)
                      n1782 = Equal?(x=w3419, y=1) -> (x = y?=w3417:bool)
                      n1783 = case shown="True" w3417 {
                        frame False {
                          n1784 = property on="R Backlash corr" class="Bool (strict)"("Val(Sgnl)"=FALSE ("Value (Signaling)")) -> ()  [unwired: 2 in, 2 out]
                        }
                        frame True {
                          n1785 = property on="R Backlash corr" class="Bool (strict)"("Val(Sgnl)"=TRUE ("Value (Signaling)")) -> ()  [unwired: 2 in, 2 out]
                        }
                      }
                    }
                    frame #2 {
                      # "Velocity Setting"
                      n1786 = property on="R Velocity SP step/sec" class="DigNum (strict)"() -> ("Value"=w3432:i32)  [unwired: 2 in, 2 out]
                      n1787 = Number To Decimal String(number=w3432) -> (decimal integer string=w3433:string)  [unwired: 1 in]
                      n1788 = call "mDrive Send Command.vi"("error in (no error)"=w3429, "Extra"=w3433, "Command"=T10."Max Velocity", "VISA resource name"=w3428) -> ("error out"=w3430:errorcluster, "VISA resource name out"=w3431:refnum<visa-resource-name>)  [unwired: 3 in, 1 out]
                    }
                    frame #3 {
                      n1789 = Wait (ms)(milliseconds to wait=u32 50) -> ()  [unwired: 1 out]
                    }
                    frame #4 {
                      # "Move to Abs Position"
                      n1790 = Number To Decimal String(number=w3439) -> (decimal integer string=w3445:string)  [unwired: 1 in]
                      n1791 = call "mDrive Send Command.vi"("error in (no error)"=w3440, "Extra"=w3445, "Command"=T10."Move to Absolute Position", "VISA resource name"=w3441) -> ("error out"=w3442:errorcluster, "VISA resource name out"=w3443:refnum<visa-resource-name>)  [unwired: 3 in, 1 out]
                    }
                    frame #5 {
                      n1792 = Wait (ms)(milliseconds to wait=u32 25) -> ()  [unwired: 1 out]
                    }
                  }
                }
              }
              n1793 = property on="Y in Motion" class="Bool (strict)"("Value"=w3349) -> ()  [unwired: 2 in, 2 out]
              n1794 = property on="R in Motion" class="Bool (strict)"("Value"=w3349) -> ()  [unwired: 2 in, 2 out]
              n1795 = property on="X  in Motion" class="Bool (strict)"("Value"=w3349) -> ()  [unwired: 2 in, 2 out]
              n1796 = property on="Z in Motion" class="Bool (strict)"("Value"=w3349) -> ()  [unwired: 2 in, 2 out]
            }
            frame #6 {
              n1797 = while {
                tunnel: [w3696] -> w3672
                tunnel: [w3695] -> w3671
                tunnel: [w3694] -> w3674
                tunnel: [w3693] -> w3673
                tunnel: [w3692] -> w3670
                tunnel: [w3691] -> w3669
                tunnel: [w3690] -> w3668
                tunnel: [w3689] -> w3667
                tunnel: w3666 -> [w3678]
                tunnel: w3665 -> [w3677]
                tunnel: w3664 -> [w3680]
                tunnel: w3663 -> [w3679]
                tunnel: w3662 -> [w3685]
                tunnel: w3661 -> [w3684]
                tunnel: w3660 -> [w3683]
                tunnel: w3659 -> [w3682]
                stop <- w3681 stop-if-true
                n1798 = flat-sequence {
                  tunnel: [w4143] -> w3752
                  tunnel: [w4142] -> w3751
                  tunnel: [w4141] -> w3750
                  tunnel: w3678 -> [w4139]
                  tunnel: w3677 -> [w4138]
                  tunnel: [w4167] -> w3749
                  tunnel: [w4166] -> w3748
                  tunnel: [w4164] -> w3747
                  tunnel: [w4165] -> w3746
                  tunnel: w3752 -> [w4164]
                  tunnel: w3751 -> [w4163]
                  tunnel: w3750 -> [w4162]
                  tunnel: w3749 -> [w4181]
                  tunnel: [w4181] -> w3742
                  tunnel: w3748 -> [w4180]
                  tunnel: [w4180] -> w3743
                  tunnel: w3747 -> [w4179]
                  tunnel: [w4179] -> w3744
                  tunnel: w3746 -> [w4178]
                  tunnel: [w4178] -> w3745
                  tunnel: [w4185] -> w3741
                  tunnel: [w4186] -> w3740
                  tunnel: [w4182] -> w3739
                  tunnel: w3745 -> [w4182]
                  tunnel: w3744 -> [w4183]
                  tunnel: w3743 -> [w4187]
                  tunnel: w3742 -> [w4184]
                  tunnel: w3741 -> [w4197]
                  tunnel: w3740 -> [w4198]
                  tunnel: w3739 -> [w4200]
                  tunnel: [w4196] -> w3695
                  tunnel: [w4195] -> w3696
                  frame #0 {
                    n1799 = property on="OP" class="Bool (strict)"() -> ("Value"=w4137:bool)  [unwired: 2 in, 2 out]
                    n1800 = case shown="False" w4137 {
                      tunnel: [w4159 w4160] -> w4154
                      frame False {
                        n1801 = property on="GVposition SP 15360000" class="DigNum (strict)"() -> ("Value"=w4159:i64)  [unwired: 2 in, 2 out]
                      }
                      frame True {
                        n1802 = property on="Z Step SP" class="DigNum (strict)"() -> ("Maximum"=w4161:dbl)  [unwired: 2 in, 2 out]
                        n1803 = To Long Integer(number=w4161) -> (32bit integer=w4160:i32)
                      }
                    }
                    n1804 = property on="Z Step SP" class="DigNum (strict)"() -> ("Minimum"=w4156:dbl)  [unwired: 2 in, 2 out]
                    n1805 = property on="Z steps/rev" class="DigNum (strict)"() -> ("Value"=w4152:u32)  [unwired: 2 in, 2 out]
                    n1806 = property on="Z offset mm" class="DigNum (strict)"() -> ("Value"=w4148:dbl)  [unwired: 2 in, 2 out]
                    n1807 = To Long Integer(number=w4156) -> (32bit integer=w4155:i32)
                    n1808 = To Double Precision Float(number=w4152) -> (double precision float=w4153:dbl)
                    n1809 = call "mDrive Send Command.vi"("error in (no error)"=w4138, "Extra"="P", "Command"=T10."Print Parameter", "VISA resource name"=w4139) -> ("error out"=w4141:errorcluster, "read buffer"=w4158:string, "VISA resource name out"=w4142:refnum<visa-resource-name>)  [unwired: 3 in]
                    n1810 = Decimal String To Number(string=w4158, offset=0) -> (number=w4140:i32)  [unwired: 1 in, 1 out]
                    n1811 = property on="Z Step PV" class="DigNum (strict)"("Val(Sgnl)"=w4140) -> ()  [unwired: 2 in, 2 out]
                    n1812 = In Range and Coerce(upper limit=w4154, x=w4140, lower limit=w4155) -> (In Range?=w4143:bool)  [unwired: 1 out]
                    n1813 = To Double Precision Float(number=w4140) -> (double precision float=w4147:dbl)
                    n1814 = property on="Z in Range" class="Bool (strict)"("Val(Sgnl)"=w4143) -> ()  [unwired: 2 in, 2 out]
                    n1815 = Divide(x=w4147, y=w4153) -> (x/y=w4151:dbl)
                    n1816 = property on="Z mm/rev" class="DigNum (strict)"() -> ("Value"=w4150:dbl)  [unwired: 2 in, 2 out]
                    n1817 = Multiply(x=w4151, y=w4150) -> (x*y=w4149:dbl)
                    n1818 = Add(x=w4149, y=w4148) -> (x+y=w4146:dbl)
                    n1819 = property on="Z Position mm PV" class="DigNum (strict)"("Val(Sgnl)"=w4146) -> ()  [unwired: 2 in, 2 out]
                  }
                  frame #1 {
                    n1820 = call "mDrive Send Command.vi"("error in (no error)"=w4162, "Extra"="MV", "Command"=T10."Print Parameter", "VISA resource name"=w4163) -> ("error out"=w4166:errorcluster, "read buffer"=w4170:string, "VISA resource name out"=w4167:refnum<visa-resource-name>)  [unwired: 3 in]
                    n1821 = Decimal String To Number(string=w4170, offset=0 ("offset (0)")) -> (number=w4173:i32)  [unwired: 1 in, 1 out]
                    n1822 = Not Equal?(x=w4170, y="") -> (x != y?=w4168:bool)
                    n1823 = property on="Z Ready" class="Bool (strict)"("Val(Sgnl)"=w4168) -> ()  [unwired: 2 in, 2 out]
                    n1824 = Number To Boolean Array(number=w4173) -> (Boolean array=w4172:bool[])
                    n1825 = Index Array(array=w4172, index=0) -> (element=w4165:bool)
                    n1826 = property on="Z in Motion" class="Bool (strict)"("Val(Sgnl)"=w4165) -> ()  [unwired: 2 in, 2 out]
                  }
                  frame #2 {
                    n1827 = Wait (ms)(milliseconds to wait=u32 50) -> ()  [unwired: 1 out]
                  }
                  frame #3 {
                    n1828 = case shown="True" w4183 {
                      tunnel: w4184 -> [w4190 w4194]
                      tunnel: [w4191 w4194] -> w4185
                      tunnel: [w4192 w4193] -> w4186
                      tunnel: w4187 -> [w4189 w4193]
                      frame False {
                        n1829 = call "mDrive Send Command.vi"("error in (no error)"=w4189, "Command"=T10."Stop", "VISA resource name"=w4190) -> ("error out"=w4192:errorcluster, "VISA resource name out"=w4191:refnum<visa-resource-name>)  [unwired: 4 in, 1 out]
                      }
                      frame True {
                      }
                    }
                  }
                  frame #4 {
                    n1830 = property on="Z Backlash corr" class="Bool (strict)"() -> ("Value"=w4201:bool)  [unwired: 2 in, 2 out]
                    n1831 = Implies(1:w4200, 2:w4201) -> (0:w4199:bool)
                    n1832 = case shown="False" w4199 {
                      tunnel: w4198 -> [w4209 w4266]
                      tunnel: w4197 -> [w4208 w4267]
                      tunnel: [w4203 w4266] -> w4196
                      tunnel: [w4207 w4267] -> w4195
                      frame False {
                        # "Backlash"
                        n1833 = flat-sequence {
                          tunnel: [w4224] -> w4221
                          tunnel: [w4226] -> w4220
                          tunnel: [w4225] -> w4219
                          tunnel: w4209 -> [w4223]
                          tunnel: w4208 -> [w4222]
                          tunnel: w4221 -> [w4234]
                          tunnel: [w4234] -> w4218
                          tunnel: w4220 -> [w4233]
                          tunnel: w4219 -> [w4232]
                          tunnel: [w4231] -> w4217
                          tunnel: [w4230] -> w4216
                          tunnel: [w4229] -> w4206
                          tunnel: w4218 -> [w4248]
                          tunnel: w4217 -> [w4239]
                          tunnel: w4216 -> [w4247]
                          tunnel: [w4239] -> w4215
                          tunnel: [w4247] -> w4214
                          tunnel: [w4238] -> w4211
                          tunnel: [w4246] -> w4210
                          tunnel: w4206 -> [w4246]
                          tunnel: w4215 -> [w4251]
                          tunnel: w4214 -> [w4252]
                          tunnel: [w4250] -> w4213
                          tunnel: [w4258] -> w4212
                          tunnel: w4211 -> [w4258]
                          tunnel: w4210 -> [w4254]
                          tunnel: [w4253] -> w4204
                          tunnel: w4213 -> [w4261]
                          tunnel: w4212 -> [w4260]
                          tunnel: [w4262] -> w4205
                          tunnel: w4204 -> [w4262]
                          tunnel: [w4261] -> w4202
                          tunnel: [w4265] -> w4207
                          tunnel: w4205 -> [w4265]
                          tunnel: [w4263] -> w4203
                          tunnel: w4202 -> [w4263]
                          frame #0 {
                            n1834 = property on="Z Backlash steps/sec" class="DigNum (strict)"() -> ("Value"=w4224:i32)  [unwired: 2 in, 2 out]
                            n1835 = Number To Decimal String(number=w4224) -> (decimal integer string=w4227:string)  [unwired: 1 in]
                            n1836 = call "mDrive Send Command.vi"("error in (no error)"=w4223, "Extra"=w4227, "Command"=T10."Max Velocity", "VISA resource name"=w4222) -> ("error out"=w4225:errorcluster, "VISA resource name out"=w4226:refnum<visa-resource-name>)  [unwired: 3 in, 1 out]
                          }
                          frame #1 {
                            n1837 = property on="Z Backlash" class="DigNum (strict)"() -> ("Value"=w4229:i32)  [unwired: 2 in, 2 out]
                            n1838 = Number To Decimal String(number=w4229) -> (decimal integer string=w4235:string)  [unwired: 1 in]
                            n1839 = call "mDrive Send Command.vi"("error in (no error)"=w4232, "Extra"=w4235, "Command"=T10."Move to Relative Position", "VISA resource name"=w4233) -> ("error out"=w4231:errorcluster, "VISA resource name out"=w4230:refnum<visa-resource-name>)  [unwired: 3 in, 1 out]
                          }
                          frame #2 {
                            n1840 = To Double Precision Float(number=w4246) -> (double precision float=w4244:dbl)
                            n1841 = To Double Precision Float(number=w4248) -> (double precision float=w4249:dbl)
                            n1842 = Absolute Value(x=w4244) -> (abs(x)=w4245:dbl)
                            n1843 = Divide(x=w4245, y=w4249) -> (x/y=w4242:dbl)
                            n1844 = Multiply(x=1000.0, y=w4242) -> (x*y=w4240:dbl)
                            n1845 = Add(x=w4240, y=300.0) -> (x+y=w4238:dbl)
                            n1846 = To Unsigned Long Integer(number=w4238) -> (unsigned 32bit integer=w4237:u32)
                            n1847 = Wait (ms)(milliseconds to wait=w4237) -> ()  [unwired: 1 out]
                          }
                          frame #3 {
                            n1848 = Negate(x=w4254) -> (-x=w4255:i32)
                            n1849 = Number To Decimal String(number=w4255) -> (decimal integer string=w4256:string)  [unwired: 1 in]
                            n1850 = call "mDrive Send Command.vi"("error in (no error)"=w4251, "Extra"=w4256, "Command"=T10."Move to Relative Position", "VISA resource name"=w4252) -> ("error out"=w4250:errorcluster, "VISA resource name out"=w4253:refnum<visa-resource-name>)  [unwired: 3 in, 1 out]
                          }
                          frame #4 {
                            n1851 = To Unsigned Long Integer(number=w4260) -> (unsigned 32bit integer=w4259:u32)
                            n1852 = Wait (ms)(milliseconds to wait=w4259) -> ()  [unwired: 1 out]
                          }
                          frame #5 {
                            n1853 = property on="Z Backlash corr" class="Bool (strict)"("Val(Sgnl)"=FALSE ("Value (Signaling)")) -> ()  [unwired: 2 in, 2 out]
                          }
                        }
                      }
                      frame True {
                      }
                    }
                  }
                }
                n1854 = flat-sequence {
                  tunnel: [w4020] -> w3738
                  tunnel: [w4013] -> w3737
                  tunnel: [w4012] -> w3736
                  tunnel: w3680 -> [w4010]
                  tunnel: w3679 -> [w4009]
                  tunnel: [w4040] -> w3735
                  tunnel: [w4039] -> w3734
                  tunnel: [w4038] -> w3733
                  tunnel: [w4031] -> w3732
                  tunnel: w3738 -> [w4038]
                  tunnel: w3737 -> [w4037]
                  tunnel: w3736 -> [w4036]
                  tunnel: w3735 -> [w4050]
                  tunnel: [w4050] -> w3728
                  tunnel: w3734 -> [w4049]
                  tunnel: [w4049] -> w3729
                  tunnel: w3733 -> [w4048]
                  tunnel: [w4048] -> w3730
                  tunnel: w3732 -> [w4047]
                  tunnel: [w4047] -> w3731
                  tunnel: [w4054] -> w3727
                  tunnel: [w4055] -> w3726
                  tunnel: [w4051] -> w3725
                  tunnel: w3731 -> [w4051]
                  tunnel: w3730 -> [w4052]
                  tunnel: w3729 -> [w4056]
                  tunnel: w3728 -> [w4053]
                  tunnel: w3727 -> [w4067]
                  tunnel: w3726 -> [w4068]
                  tunnel: w3725 -> [w4070]
                  tunnel: [w4066] -> w3693
                  tunnel: [w4065] -> w3694
                  frame #0 {
                    n1855 = property on="X Step SP" class="DigNum (strict)"() -> ("Maximum"=w4021:dbl)  [unwired: 2 in, 2 out]
                    n1856 = property on="X Step SP" class="DigNum (strict)"() -> ("Minimum"=w4015:dbl)  [unwired: 2 in, 2 out]
                    n1857 = property on="X steps/rev" class="DigNum (strict)"() -> ("Value"=w4019:u32)  [unwired: 2 in, 2 out]
                    n1858 = property on="X offset mm" class="DigNum (strict)"() -> ("Value"=w4017:dbl)  [unwired: 2 in, 2 out]
                    n1859 = To Long Integer(number=w4021) -> (32bit integer=w4027:i32)
                    n1860 = To Long Integer(number=w4015) -> (32bit integer=w4028:i32)
                    n1861 = To Double Precision Float(number=w4019) -> (double precision float=w4026:dbl)
                    n1862 = call "mDrive Send Command.vi"("error in (no error)"=w4009, "Extra"="P", "Command"=T10."Print Parameter", "VISA resource name"=w4010) -> ("error out"=w4012:errorcluster, "read buffer"=w4030:string, "VISA resource name out"=w4013:refnum<visa-resource-name>)  [unwired: 3 in]
                    n1863 = Decimal String To Number(string=w4030, offset=0) -> (number=w4011:i32)  [unwired: 1 in, 1 out]
                    n1864 = property on="X Step PV" class="DigNum (strict)"("Val(Sgnl)"=w4011) -> ()  [unwired: 2 in, 2 out]
                    n1865 = In Range and Coerce(upper limit=w4027, x=w4011, lower limit=w4028) -> (In Range?=w4020:bool)  [unwired: 1 out]
                    n1866 = To Double Precision Float(number=w4011) -> (double precision float=w4024:dbl)
                    n1867 = property on="X  in Range" class="Bool (strict)"("Val(Sgnl)"=w4020) -> ()  [unwired: 2 in, 2 out]
                    n1868 = Divide(x=w4024, y=w4026) -> (x/y=w4025:dbl)
                    n1869 = property on="X mm/rev" class="DigNum (strict)"() -> ("Value"=w4018:dbl)  [unwired: 2 in, 2 out]
                    n1870 = Multiply(x=w4025, y=w4018) -> (x*y=w4014:dbl)
                    n1871 = Add(x=w4014, y=w4017) -> (x+y=w4016:dbl)
                    n1872 = property on="X Position mm PV" class="DigNum (strict)"("Val(Sgnl)"=w4016) -> ()  [unwired: 2 in, 2 out]
                  }
                  frame #1 {
                    n1873 = call "mDrive Send Command.vi"("error in (no error)"=w4036, "Extra"="MV", "Command"=T10."Print Parameter", "VISA resource name"=w4037) -> ("error out"=w4039:errorcluster, "read buffer"=w4042:string, "VISA resource name out"=w4040:refnum<visa-resource-name>)  [unwired: 3 in]
                    n1874 = Decimal String To Number(string=w4042, offset=0 ("offset (0)")) -> (number=w4032:i32)  [unwired: 1 in, 1 out]
                    n1875 = Not Equal?(x=w4042, y="") -> (x != y?=w4035:bool)
                    n1876 = property on="X Ready" class="Bool (strict)"("Val(Sgnl)"=w4035) -> ()  [unwired: 2 in, 2 out]
                    n1877 = Number To Boolean Array(number=w4032) -> (Boolean array=w4034:bool[])
                    n1878 = Index Array(array=w4034, index=0) -> (element=w4031:bool)
                    n1879 = property on="X  in Motion" class="Bool (strict)"("Val(Sgnl)"=w4031) -> ()  [unwired: 2 in, 2 out]
                  }
                  frame #2 {
                    n1880 = Wait (ms)(milliseconds to wait=u32 50) -> ()  [unwired: 1 out]
                  }
                  frame #3 {
                    n1881 = case shown="False" w4052 {
                      tunnel: w4053 -> [w4059 w4063]
                      tunnel: [w4060 w4063] -> w4054
                      tunnel: [w4061 w4062] -> w4055
                      tunnel: w4056 -> [w4058 w4062]
                      frame False {
                        n1882 = call "mDrive Send Command.vi"("error in (no error)"=w4058, "Command"=T10."Stop", "VISA resource name"=w4059) -> ("error out"=w4061:errorcluster, "VISA resource name out"=w4060:refnum<visa-resource-name>)  [unwired: 4 in, 1 out]
                      }
                      frame True {
                      }
                    }
                  }
                  frame #4 {
                    n1883 = property on="X Backlash corr" class="Bool (strict)"() -> ("Value"=w4064:bool)  [unwired: 2 in, 2 out]
                    n1884 = Implies(1:w4070, 2:w4064) -> (0:w4069:bool)
                    n1885 = case shown="False" w4069 {
                      tunnel: w4068 -> [w4078 w4135]
                      tunnel: w4067 -> [w4077 w4136]
                      tunnel: [w4072 w4135] -> w4066
                      tunnel: [w4076 w4136] -> w4065
                      frame False {
                        # "Backlash"
                        n1886 = flat-sequence {
                          tunnel: [w4091] -> w4090
                          tunnel: [w4095] -> w4089
                          tunnel: [w4094] -> w4088
                          tunnel: w4078 -> [w4093]
                          tunnel: w4077 -> [w4092]
                          tunnel: w4090 -> [w4103]
                          tunnel: [w4103] -> w4087
                          tunnel: w4089 -> [w4102]
                          tunnel: w4088 -> [w4101]
                          tunnel: [w4100] -> w4086
                          tunnel: [w4099] -> w4085
                          tunnel: [w4098] -> w4075
                          tunnel: w4087 -> [w4117]
                          tunnel: w4086 -> [w4108]
                          tunnel: w4085 -> [w4116]
                          tunnel: [w4108] -> w4084
                          tunnel: [w4116] -> w4083
                          tunnel: [w4107] -> w4080
                          tunnel: [w4115] -> w4079
                          tunnel: w4075 -> [w4115]
                          tunnel: w4084 -> [w4120]
                          tunnel: w4083 -> [w4121]
                          tunnel: [w4119] -> w4082
                          tunnel: [w4127] -> w4081
                          tunnel: w4080 -> [w4127]
                          tunnel: w4079 -> [w4123]
                          tunnel: [w4122] -> w4073
                          tunnel: w4082 -> [w4130]
                          tunnel: w4081 -> [w4129]
                          tunnel: [w4131] -> w4074
                          tunnel: w4073 -> [w4131]
                          tunnel: [w4130] -> w4071
                          tunnel: [w4134] -> w4076
                          tunnel: w4074 -> [w4134]
                          tunnel: [w4133] -> w4072
                          tunnel: w4071 -> [w4133]
                          frame #0 {
                            n1887 = property on="X Backlash steps/sec" class="DigNum (strict)"() -> ("Value"=w4091:i32)  [unwired: 2 in, 2 out]
                            n1888 = Number To Decimal String(number=w4091) -> (decimal integer string=w4096:string)  [unwired: 1 in]
                            n1889 = call "mDrive Send Command.vi"("error in (no error)"=w4093, "Extra"=w4096, "Command"=T10."Max Velocity", "VISA resource name"=w4092) -> ("error out"=w4094:errorcluster, "VISA resource name out"=w4095:refnum<visa-resource-name>)  [unwired: 3 in, 1 out]
                          }
                          frame #1 {
                            n1890 = property on="X Backlash" class="DigNum (strict)"() -> ("Value"=w4098:i32)  [unwired: 2 in, 2 out]
                            n1891 = Number To Decimal String(number=w4098) -> (decimal integer string=w4104:string)  [unwired: 1 in]
                            n1892 = call "mDrive Send Command.vi"("error in (no error)"=w4101, "Extra"=w4104, "Command"=T10."Move to Relative Position", "VISA resource name"=w4102) -> ("error out"=w4100:errorcluster, "VISA resource name out"=w4099:refnum<visa-resource-name>)  [unwired: 3 in, 1 out]
                          }
                          frame #2 {
                            n1893 = To Double Precision Float(number=w4115) -> (double precision float=w4113:dbl)
                            n1894 = To Double Precision Float(number=w4117) -> (double precision float=w4118:dbl)
                            n1895 = Absolute Value(x=w4113) -> (abs(x)=w4114:dbl)
                            n1896 = Divide(x=w4114, y=w4118) -> (x/y=w4111:dbl)
                            n1897 = Multiply(x=1000.0, y=w4111) -> (x*y=w4109:dbl)
                            n1898 = Add(x=w4109, y=300.0) -> (x+y=w4107:dbl)
                            n1899 = To Unsigned Long Integer(number=w4107) -> (unsigned 32bit integer=w4106:u32)
                            n1900 = Wait (ms)(milliseconds to wait=w4106) -> ()  [unwired: 1 out]
                          }
                          frame #3 {
                            n1901 = Negate(x=w4123) -> (-x=w4124:i32)
                            n1902 = Number To Decimal String(number=w4124) -> (decimal integer string=w4125:string)  [unwired: 1 in]
                            n1903 = call "mDrive Send Command.vi"("error in (no error)"=w4120, "Extra"=w4125, "Command"=T10."Move to Relative Position", "VISA resource name"=w4121) -> ("error out"=w4119:errorcluster, "VISA resource name out"=w4122:refnum<visa-resource-name>)  [unwired: 3 in, 1 out]
                          }
                          frame #4 {
                            n1904 = To Unsigned Long Integer(number=w4129) -> (unsigned 32bit integer=w4128:u32)
                            n1905 = Wait (ms)(milliseconds to wait=w4128) -> ()  [unwired: 1 out]
                          }
                          frame #5 {
                            n1906 = property on="X Backlash corr" class="Bool (strict)"("Val(Sgnl)"=FALSE ("Value (Signaling)")) -> ()  [unwired: 2 in, 2 out]
                          }
                        }
                      }
                      frame True {
                      }
                    }
                  }
                }
                n1907 = flat-sequence {
                  tunnel: [w3890] -> w3724
                  tunnel: [w3892] -> w3723
                  tunnel: [w3891] -> w3722
                  tunnel: w3685 -> [w3882]
                  tunnel: w3684 -> [w3881]
                  tunnel: [w3912] -> w3721
                  tunnel: [w3911] -> w3720
                  tunnel: [w3910] -> w3719
                  tunnel: [w3903] -> w3718
                  tunnel: w3724 -> [w3910]
                  tunnel: w3723 -> [w3909]
                  tunnel: w3722 -> [w3908]
                  tunnel: w3721 -> [w3922]
                  tunnel: [w3922] -> w3714
                  tunnel: w3720 -> [w3921]
                  tunnel: [w3921] -> w3715
                  tunnel: w3719 -> [w3920]
                  tunnel: [w3920] -> w3716
                  tunnel: w3718 -> [w3919]
                  tunnel: [w3919] -> w3717
                  tunnel: [w3926] -> w3713
                  tunnel: [w3927] -> w3712
                  tunnel: [w3923] -> w3711
                  tunnel: w3717 -> [w3923]
                  tunnel: w3716 -> [w3924]
                  tunnel: w3715 -> [w3928]
                  tunnel: w3714 -> [w3925]
                  tunnel: w3713 -> [w3939]
                  tunnel: w3712 -> [w3940]
                  tunnel: w3711 -> [w3942]
                  tunnel: [w3938] -> w3691
                  tunnel: [w3937] -> w3692
                  frame #0 {
                    n1908 = property on="Y Step SP" class="DigNum (strict)"() -> ("Maximum"=w3885:dbl)  [unwired: 2 in, 2 out]
                    n1909 = property on="Y Step SP" class="DigNum (strict)"() -> ("Minimum"=w3884:dbl)  [unwired: 2 in, 2 out]
                    n1910 = property on="Y steps/rev" class="DigNum (strict)"() -> ("Value"=w3886:u32)  [unwired: 2 in, 2 out]
                    n1911 = property on="Y offset mm" class="DigNum (strict)"() -> ("Value"=w3888:dbl)  [unwired: 2 in, 2 out]
                    n1912 = To Long Integer(number=w3885) -> (32bit integer=w3899:i32)
                    n1913 = To Long Integer(number=w3884) -> (32bit integer=w3900:i32)
                    n1914 = To Double Precision Float(number=w3886) -> (double precision float=w3898:dbl)
                    n1915 = call "mDrive Send Command.vi"("error in (no error)"=w3882, "Extra"="P", "Command"=T10."Print Parameter", "VISA resource name"=w3881) -> ("error out"=w3891:errorcluster, "read buffer"=w3902:string, "VISA resource name out"=w3892:refnum<visa-resource-name>)  [unwired: 3 in]
                    n1916 = Decimal String To Number(string=w3902, offset=0) -> (number=w3883:i32)  [unwired: 1 in, 1 out]
                    n1917 = property on="Y Step PV" class="DigNum (strict)"("Val(Sgnl)"=w3883) -> ()  [unwired: 2 in, 2 out]
                    n1918 = In Range and Coerce(upper limit=w3899, x=w3883, lower limit=w3900) -> (In Range?=w3890:bool)  [unwired: 1 out]
                    n1919 = To Double Precision Float(number=w3883) -> (double precision float=w3895:dbl)
                    n1920 = property on="Y in Range" class="Bool (strict)"("Val(Sgnl)"=w3890) -> ()  [unwired: 2 in, 2 out]
                    n1921 = Divide(x=w3895, y=w3898) -> (x/y=w3897:dbl)
                    n1922 = property on="Y mm/rev" class="DigNum (strict)"() -> ("Value"=w3887:dbl)  [unwired: 2 in, 2 out]
                    n1923 = Multiply(x=w3897, y=w3887) -> (x*y=w3896:dbl)
                    n1924 = Add(x=w3896, y=w3888) -> (x+y=w3889:dbl)
                    n1925 = property on="Y Position mm PV" class="DigNum (strict)"("Val(Sgnl)"=w3889) -> ()  [unwired: 2 in, 2 out]
                  }
                  frame #1 {
                    n1926 = call "mDrive Send Command.vi"("error in (no error)"=w3908, "Extra"="MV", "Command"=T10."Print Parameter", "VISA resource name"=w3909) -> ("error out"=w3911:errorcluster, "read buffer"=w3914:string, "VISA resource name out"=w3912:refnum<visa-resource-name>)  [unwired: 3 in]
                    n1927 = Decimal String To Number(string=w3914, offset=0 ("offset (0)")) -> (number=w3904:i32)  [unwired: 1 in, 1 out]
                    n1928 = Not Equal?(x=w3914, y="") -> (x != y?=w3907:bool)
                    n1929 = property on="Y Ready" class="Bool (strict)"("Val(Sgnl)"=w3907) -> ()  [unwired: 2 in, 2 out]
                    n1930 = Number To Boolean Array(number=w3904) -> (Boolean array=w3906:bool[])
                    n1931 = Index Array(array=w3906, index=0) -> (element=w3903:bool)
                    n1932 = property on="Y in Motion" class="Bool (strict)"("Val(Sgnl)"=w3903) -> ()  [unwired: 2 in, 2 out]
                  }
                  frame #2 {
                    n1933 = Wait (ms)(milliseconds to wait=u32 50) -> ()  [unwired: 1 out]
                  }
                  frame #3 {
                    n1934 = case shown="False" w3924 {
                      tunnel: w3925 -> [w3931 w3934]
                      tunnel: [w3932 w3934] -> w3926
                      tunnel: [w3933 w3935] -> w3927
                      tunnel: w3928 -> [w3930 w3935]
                      frame False {
                        n1935 = call "mDrive Send Command.vi"("error in (no error)"=w3930, "Command"=T10."Stop", "VISA resource name"=w3931) -> ("error out"=w3933:errorcluster, "VISA resource name out"=w3932:refnum<visa-resource-name>)  [unwired: 4 in, 1 out]
                      }
                      frame True {
                      }
                    }
                  }
                  frame #4 {
                    n1936 = property on="Y Backlash corr" class="Bool (strict)"() -> ("Value"=w3936:bool)  [unwired: 2 in, 2 out]
                    n1937 = Implies(1:w3942, 2:w3936) -> (0:w3941:bool)
                    n1938 = case shown="False" w3941 {
                      tunnel: w3940 -> [w3950 w4007]
                      tunnel: w3939 -> [w3949 w4008]
                      tunnel: [w3944 w4007] -> w3938
                      tunnel: [w3948 w4008] -> w3937
                      frame False {
                        # "Backlash"
                        n1939 = flat-sequence {
                          tunnel: [w3963] -> w3962
                          tunnel: [w3967] -> w3961
                          tunnel: [w3966] -> w3960
                          tunnel: w3950 -> [w3965]
                          tunnel: w3949 -> [w3964]
                          tunnel: w3962 -> [w3975]
                          tunnel: [w3975] -> w3959
                          tunnel: w3961 -> [w3974]
                          tunnel: w3960 -> [w3973]
                          tunnel: [w3972] -> w3958
                          tunnel: [w3971] -> w3957
                          tunnel: [w3970] -> w3947
                          tunnel: w3959 -> [w3989]
                          tunnel: w3958 -> [w3980]
                          tunnel: w3957 -> [w3988]
                          tunnel: [w3980] -> w3956
                          tunnel: [w3988] -> w3955
                          tunnel: [w3979] -> w3952
                          tunnel: [w3987] -> w3951
                          tunnel: w3947 -> [w3987]
                          tunnel: w3956 -> [w3992]
                          tunnel: w3955 -> [w3993]
                          tunnel: [w3991] -> w3954
                          tunnel: [w3999] -> w3953
                          tunnel: w3952 -> [w3999]
                          tunnel: w3951 -> [w3995]
                          tunnel: [w3994] -> w3945
                          tunnel: w3954 -> [w4002]
                          tunnel: w3953 -> [w4001]
                          tunnel: [w4003] -> w3946
                          tunnel: w3945 -> [w4003]
                          tunnel: [w4002] -> w3943
                          tunnel: [w4006] -> w3948
                          tunnel: w3946 -> [w4006]
                          tunnel: [w4005] -> w3944
                          tunnel: w3943 -> [w4005]
                          frame #0 {
                            n1940 = property on="Y Backlash steps/sec" class="DigNum (strict)"() -> ("Value"=w3963:i32)  [unwired: 2 in, 2 out]
                            n1941 = Number To Decimal String(number=w3963) -> (decimal integer string=w3968:string)  [unwired: 1 in]
                            n1942 = call "mDrive Send Command.vi"("error in (no error)"=w3965, "Extra"=w3968, "Command"=T10."Max Velocity", "VISA resource name"=w3964) -> ("error out"=w3966:errorcluster, "VISA resource name out"=w3967:refnum<visa-resource-name>)  [unwired: 3 in, 1 out]
                          }
                          frame #1 {
                            n1943 = property on="Y Backlash" class="DigNum (strict)"() -> ("Value"=w3970:i32)  [unwired: 2 in, 2 out]
                            n1944 = Number To Decimal String(number=w3970) -> (decimal integer string=w3976:string)  [unwired: 1 in]
                            n1945 = call "mDrive Send Command.vi"("error in (no error)"=w3973, "Extra"=w3976, "Command"=T10."Move to Relative Position", "VISA resource name"=w3974) -> ("error out"=w3972:errorcluster, "VISA resource name out"=w3971:refnum<visa-resource-name>)  [unwired: 3 in, 1 out]
                          }
                          frame #2 {
                            n1946 = To Double Precision Float(number=w3987) -> (double precision float=w3985:dbl)
                            n1947 = To Double Precision Float(number=w3989) -> (double precision float=w3990:dbl)
                            n1948 = Absolute Value(x=w3985) -> (abs(x)=w3986:dbl)
                            n1949 = Divide(x=w3986, y=w3990) -> (x/y=w3983:dbl)
                            n1950 = Multiply(x=1000.0, y=w3983) -> (x*y=w3981:dbl)
                            n1951 = Add(x=w3981, y=300.0) -> (x+y=w3979:dbl)
                            n1952 = To Unsigned Long Integer(number=w3979) -> (unsigned 32bit integer=w3978:u32)
                            n1953 = Wait (ms)(milliseconds to wait=w3978) -> ()  [unwired: 1 out]
                          }
                          frame #3 {
                            n1954 = Negate(x=w3995) -> (-x=w3996:i32)
                            n1955 = Number To Decimal String(number=w3996) -> (decimal integer string=w3997:string)  [unwired: 1 in]
                            n1956 = call "mDrive Send Command.vi"("error in (no error)"=w3992, "Extra"=w3997, "Command"=T10."Move to Relative Position", "VISA resource name"=w3993) -> ("error out"=w3991:errorcluster, "VISA resource name out"=w3994:refnum<visa-resource-name>)  [unwired: 3 in, 1 out]
                          }
                          frame #4 {
                            n1957 = To Unsigned Long Integer(number=w4001) -> (unsigned 32bit integer=w4000:u32)
                            n1958 = Wait (ms)(milliseconds to wait=w4000) -> ()  [unwired: 1 out]
                          }
                          frame #5 {
                            n1959 = property on="Y Backlash corr" class="Bool (strict)"("Val(Sgnl)"=FALSE ("Value (Signaling)")) -> ()  [unwired: 2 in, 2 out]
                          }
                        }
                      }
                      frame True {
                      }
                    }
                  }
                }
                n1960 = flat-sequence {
                  tunnel: [w3762] -> w3710
                  tunnel: [w3764] -> w3709
                  tunnel: [w3763] -> w3708
                  tunnel: w3683 -> [w3754]
                  tunnel: w3682 -> [w3753]
                  tunnel: [w3784] -> w3707
                  tunnel: [w3783] -> w3706
                  tunnel: [w3782] -> w3705
                  tunnel: [w3775] -> w3704
                  tunnel: w3710 -> [w3782]
                  tunnel: w3709 -> [w3781]
                  tunnel: w3708 -> [w3780]
                  tunnel: w3707 -> [w3794]
                  tunnel: [w3794] -> w3700
                  tunnel: w3706 -> [w3793]
                  tunnel: [w3793] -> w3701
                  tunnel: w3705 -> [w3792]
                  tunnel: [w3792] -> w3702
                  tunnel: w3704 -> [w3791]
                  tunnel: [w3791] -> w3703
                  tunnel: [w3798] -> w3699
                  tunnel: [w3799] -> w3698
                  tunnel: [w3795] -> w3697
                  tunnel: w3703 -> [w3795]
                  tunnel: w3702 -> [w3796]
                  tunnel: w3701 -> [w3800]
                  tunnel: w3700 -> [w3797]
                  tunnel: w3699 -> [w3811]
                  tunnel: w3698 -> [w3812]
                  tunnel: w3697 -> [w3814]
                  tunnel: [w3810] -> w3689
                  tunnel: [w3809] -> w3690
                  frame #0 {
                    n1961 = property on="R Step SP" class="DigNum (strict)"() -> ("Maximum"=w3757:dbl)  [unwired: 2 in, 2 out]
                    n1962 = property on="R Step SP" class="DigNum (strict)"() -> ("Minimum"=w3758:dbl)  [unwired: 2 in, 2 out]
                    n1963 = property on="R steps/rev" class="DigNum (strict)"() -> ("Value"=w3756:u32)  [unwired: 2 in, 2 out]
                    n1964 = property on="R offset deg" class="DigNum (strict)"() -> ("Value"=w3760:dbl)  [unwired: 2 in, 2 out]
                    n1965 = To Long Integer(number=w3757) -> (32bit integer=w3771:i32)
                    n1966 = To Long Integer(number=w3758) -> (32bit integer=w3772:i32)
                    n1967 = To Double Precision Float(number=w3756) -> (double precision float=w3770:dbl)
                    n1968 = call "mDrive Send Command.vi"("error in (no error)"=w3754, "Extra"="P", "Command"=T10."Print Parameter", "VISA resource name"=w3753) -> ("error out"=w3763:errorcluster, "read buffer"=w3774:string, "VISA resource name out"=w3764:refnum<visa-resource-name>)  [unwired: 3 in]
                    n1969 = Decimal String To Number(string=w3774, offset=0) -> (number=w3755:i32)  [unwired: 1 in, 1 out]
                    n1970 = property on="R Step PV" class="DigNum (strict)"("Val(Sgnl)"=w3755) -> ()  [unwired: 2 in, 2 out]
                    n1971 = In Range and Coerce(upper limit=w3771, x=w3755, lower limit=w3772) -> (In Range?=w3762:bool)  [unwired: 1 out]
                    n1972 = To Double Precision Float(number=w3755) -> (double precision float=w3767:dbl)
                    n1973 = property on="R in Range" class="Bool (strict)"("Val(Sgnl)"=w3762) -> ()  [unwired: 2 in, 2 out]
                    n1974 = Divide(x=w3767, y=w3770) -> (x/y=w3769:dbl)
                    n1975 = property on="R deg/rev" class="DigNum (strict)"() -> ("Value"=w3759:dbl)  [unwired: 2 in, 2 out]
                    n1976 = Multiply(x=w3769, y=w3759) -> (x*y=w3768:dbl)
                    n1977 = Add(x=w3768, y=w3760) -> (x+y=w3761:dbl)
                    n1978 = property on="R Position deg PV" class="DigNum (strict)"("Val(Sgnl)"=w3761) -> ()  [unwired: 2 in, 2 out]
                  }
                  frame #1 {
                    n1979 = call "mDrive Send Command.vi"("error in (no error)"=w3780, "Extra"="MV", "Command"=T10."Print Parameter", "VISA resource name"=w3781) -> ("error out"=w3783:errorcluster, "read buffer"=w3786:string, "VISA resource name out"=w3784:refnum<visa-resource-name>)  [unwired: 3 in]
                    n1980 = Decimal String To Number(string=w3786, offset=0 ("offset (0)")) -> (number=w3776:i32)  [unwired: 1 in, 1 out]
                    n1981 = Not Equal?(x=w3786, y="") -> (x != y?=w3779:bool)
                    n1982 = property on="R Ready" class="Bool (strict)"("Val(Sgnl)"=w3779) -> ()  [unwired: 2 in, 2 out]
                    n1983 = Number To Boolean Array(number=w3776) -> (Boolean array=w3778:bool[])
                    n1984 = Index Array(array=w3778, index=0) -> (element=w3775:bool)
                    n1985 = property on="R in Motion" class="Bool (strict)"("Val(Sgnl)"=w3775) -> ()  [unwired: 2 in, 2 out]
                  }
                  frame #2 {
                    n1986 = Wait (ms)(milliseconds to wait=u32 50) -> ()  [unwired: 1 out]
                  }
                  frame #3 {
                    n1987 = case shown="False" w3796 {
                      tunnel: w3797 -> [w3803 w3807]
                      tunnel: [w3804 w3807] -> w3798
                      tunnel: [w3805 w3806] -> w3799
                      tunnel: w3800 -> [w3802 w3806]
                      frame False {
                        n1988 = call "mDrive Send Command.vi"("error in (no error)"=w3802, "Command"=T10."Stop", "VISA resource name"=w3803) -> ("error out"=w3805:errorcluster, "VISA resource name out"=w3804:refnum<visa-resource-name>)  [unwired: 4 in, 1 out]
                      }
                      frame True {
                      }
                    }
                  }
                  frame #4 {
                    n1989 = property on="R Backlash corr" class="Bool (strict)"() -> ("Value"=w3808:bool)  [unwired: 2 in, 2 out]
                    n1990 = Implies(1:w3814, 2:w3808) -> (0:w3813:bool)
                    n1991 = case shown="False" w3813 {
                      tunnel: w3812 -> [w3822 w3879]
                      tunnel: w3811 -> [w3821 w3880]
                      tunnel: [w3816 w3879] -> w3810
                      tunnel: [w3820 w3880] -> w3809
                      frame False {
                        # "Backlash"
                        n1992 = flat-sequence {
                          tunnel: [w3835] -> w3834
                          tunnel: [w3839] -> w3833
                          tunnel: [w3838] -> w3832
                          tunnel: w3822 -> [w3837]
                          tunnel: w3821 -> [w3836]
                          tunnel: w3834 -> [w3847]
                          tunnel: [w3847] -> w3831
                          tunnel: w3833 -> [w3846]
                          tunnel: w3832 -> [w3845]
                          tunnel: [w3844] -> w3830
                          tunnel: [w3843] -> w3829
                          tunnel: [w3842] -> w3819
                          tunnel: w3831 -> [w3861]
                          tunnel: w3830 -> [w3852]
                          tunnel: w3829 -> [w3860]
                          tunnel: [w3852] -> w3828
                          tunnel: [w3860] -> w3827
                          tunnel: [w3851] -> w3824
                          tunnel: [w3859] -> w3823
                          tunnel: w3819 -> [w3859]
                          tunnel: w3828 -> [w3864]
                          tunnel: w3827 -> [w3865]
                          tunnel: [w3863] -> w3826
                          tunnel: [w3871] -> w3825
                          tunnel: w3824 -> [w3871]
                          tunnel: w3823 -> [w3867]
                          tunnel: [w3866] -> w3817
                          tunnel: w3826 -> [w3874]
                          tunnel: w3825 -> [w3873]
                          tunnel: [w3875] -> w3818
                          tunnel: w3817 -> [w3875]
                          tunnel: [w3874] -> w3815
                          tunnel: [w3878] -> w3820
                          tunnel: w3818 -> [w3878]
                          tunnel: [w3877] -> w3816
                          tunnel: w3815 -> [w3877]
                          frame #0 {
                            n1993 = property on="R Backlash steps/sec" class="DigNum (strict)"() -> ("Value"=w3835:i32)  [unwired: 2 in, 2 out]
                            n1994 = Number To Decimal String(number=w3835) -> (decimal integer string=w3840:string)  [unwired: 1 in]
                            n1995 = call "mDrive Send Command.vi"("error in (no error)"=w3837, "Extra"=w3840, "Command"=T10."Max Velocity", "VISA resource name"=w3836) -> ("error out"=w3838:errorcluster, "VISA resource name out"=w3839:refnum<visa-resource-name>)  [unwired: 3 in, 1 out]
                          }
                          frame #1 {
                            n1996 = property on="R Backlash steps/sec" class="DigNum (strict)"() -> ("Value"=w3842:i32)  [unwired: 2 in, 2 out]
                            n1997 = Number To Decimal String(number=w3842) -> (decimal integer string=w3848:string)  [unwired: 1 in]
                            n1998 = call "mDrive Send Command.vi"("error in (no error)"=w3845, "Extra"=w3848, "Command"=T10."Move to Relative Position", "VISA resource name"=w3846) -> ("error out"=w3844:errorcluster, "VISA resource name out"=w3843:refnum<visa-resource-name>)  [unwired: 3 in, 1 out]
                          }
                          frame #2 {
                            n1999 = To Double Precision Float(number=w3859) -> (double precision float=w3857:dbl)
                            n2000 = To Double Precision Float(number=w3861) -> (double precision float=w3862:dbl)
                            n2001 = Absolute Value(x=w3857) -> (abs(x)=w3858:dbl)
                            n2002 = Divide(x=w3858, y=w3862) -> (x/y=w3855:dbl)
                            n2003 = Multiply(x=1000.0, y=w3855) -> (x*y=w3853:dbl)
                            n2004 = Add(x=w3853, y=300.0) -> (x+y=w3851:dbl)
                            n2005 = To Unsigned Long Integer(number=w3851) -> (unsigned 32bit integer=w3850:u32)
                            n2006 = Wait (ms)(milliseconds to wait=w3850) -> ()  [unwired: 1 out]
                          }
                          frame #3 {
                            n2007 = Negate(x=w3867) -> (-x=w3868:i32)
                            n2008 = Number To Decimal String(number=w3868) -> (decimal integer string=w3869:string)  [unwired: 1 in]
                            n2009 = call "mDrive Send Command.vi"("error in (no error)"=w3864, "Extra"=w3869, "Command"=T10."Move to Relative Position", "VISA resource name"=w3865) -> ("error out"=w3863:errorcluster, "VISA resource name out"=w3866:refnum<visa-resource-name>)  [unwired: 3 in, 1 out]
                          }
                          frame #4 {
                            n2010 = To Unsigned Long Integer(number=w3873) -> (unsigned 32bit integer=w3872:u32)
                            n2011 = Wait (ms)(milliseconds to wait=w3872) -> ()  [unwired: 1 out]
                          }
                          frame #5 {
                            n2012 = property on="R Backlash corr" class="Bool (strict)"("Val(Sgnl)"=FALSE ("Value (Signaling)")) -> ()  [unwired: 2 in, 2 out]
                          }
                        }
                      }
                      frame True {
                      }
                    }
                  }
                }
                n2013 = property on="Y in Motion" class="Bool (strict)"() -> ("Value"=w3688:bool)  [unwired: 2 in, 2 out]
                n2014 = property on="Z in Motion" class="Bool (strict)"() -> ("Value"=w3676:bool)  [unwired: 2 in, 2 out]
                n2015 = property on="X  in Motion" class="Bool (strict)"() -> ("Value"=w3687:bool)  [unwired: 2 in, 2 out]
                n2016 = property on="R in Motion" class="Bool (strict)"() -> ("Value"=w3675:bool)  [unwired: 2 in, 2 out]
                n2017 = Compound Arithmetic op=OR(w3687, w3688, w3676, w3675) -> (w3686:bool)
                n2018 = Not(x=w3686) -> (.not. x?=w3681:bool)
              }
            }
            frame #7 {
              n2019 = Wait (ms)(milliseconds to wait=u32 1000) -> ()  [unwired: 1 out]
            }
          }
          n2020 = Increment(x=w2717) -> (x+1=w2718:i32)
          n2021 = property on="#th loop" class="DigNum (strict)"("Val(Sgnl)"=w2718) -> ()  [unwired: 2 in, 2 out]
          n2022 = property on="#th loop" class="DigNum (strict)"() -> ("Value"=w2707:dbl)  [unwired: 2 in, 2 out]
          n2023 = property on="# of loops" class="DigNum (strict)"() -> ("Value"=w2708:dbl)  [unwired: 2 in, 2 out]
          n2024 = Greater Or Equal?(x=w2707, y=w2708) -> (x >= y?=w2706:bool)
        }
        n2025 = flat-sequence {
          tunnel: [w4278] -> _
          tunnel: w2689 -> [w4278]
          tunnel: w2688 -> [_]
          tunnel: [w4277] -> _
          tunnel: w2687 -> [w4277]
          tunnel: w2686 -> [_]
          frame #0 {
            w4281 = T9."Enabled" ("Disabled")
            n2026 = local write "STATUS"("LEAVING LOOP" ("STATUS")) -> ()
            n2027 = property on="Z Scan Length SP steps" class="DigNum (strict)"("DisabledEnum"=T9."Enabled" ("Disabled")) -> ()  [unwired: 2 in, 2 out]
            n2028 = property on="Z Scan Velocity SP steps/sec" class="DigNum (strict)"("DisabledEnum"=T9."Enabled" ("Disabled")) -> ()  [unwired: 2 in, 2 out]
            n2029 = property on="R Scan Length SP steps" class="DigNum (strict)"("DisabledEnum"=T9."Enabled" ("Disabled")) -> ()  [unwired: 2 in, 2 out]
            n2030 = property on="X Scan Velocity SP steps/sec" class="DigNum (strict)"("DisabledEnum"=T9."Enabled" ("Disabled")) -> ()  [unwired: 2 in, 2 out]
            n2031 = property on="GO" class="Bool"("DisabledEnum"=w4281) -> ()  [unwired: 2 in, 2 out]
            n2032 = property on="Set Scan \nParameters" class="Bool"("DisabledEnum"=w4281) -> ()  [unwired: 2 in, 2 out]
            n2033 = property on="Y Scan Length SP steps" class="DigNum (strict)"("DisabledEnum"=T9."Enabled" ("Disabled")) -> ()  [unwired: 2 in, 2 out]
            n2034 = property on="R Scan Velocity SP steps/sec" class="DigNum (strict)"("DisabledEnum"=T9."Enabled" ("Disabled")) -> ()  [unwired: 2 in, 2 out]
            n2035 = property on="X Scan Length SP steps" class="DigNum (strict)"("DisabledEnum"=T9."Enabled" ("Disabled")) -> ()  [unwired: 2 in, 2 out]
            n2036 = property on="Y Scan Selocity SP steps/sec" class="DigNum (strict)"("DisabledEnum"=T9."Enabled" ("Disabled")) -> ()  [unwired: 2 in, 2 out]
            n2037 = property on="Send scan parameter" class="Bool"("DisabledEnum"=w4281) -> ()  [unwired: 2 in, 2 out]
            n2038 = property on="Scan Go" class="Bool (strict)"("DisabledEnum"=T9."Disabled and Grayed Out" ("Disabled")) -> ()  [unwired: 2 in, 2 out]
          }
        }
      }
    }
    n2039 = case shown="False" "Delete Button" {
      tunnel: w296 -> [_ w329]
      frame False {
      }
      frame True {
        n2040 = local read "Preset positions"() -> (w327:i32)
        n2041 = local read "Presets"() -> (w328:i32[][])
        n2042 = Delete From Array(array=w329, index=w327) -> (array with subset deleted=w325:string[])  [unwired: 1 in, 1 out]
        n2043 = property on="Preset positions" class="Ring (strict)"("Strings []"=w325) -> ()  [unwired: 2 in, 2 out]
        n2044 = Delete From Array(array=w328, index (row)=w327) -> (array with subset deleted=w326:i32[][])  [unwired: 2 in, 1 out]
        n2045 = local write "Presets"(w326) -> ()
      }
    }
    n2046 = case shown="False" "Add Button" {
      tunnel: w296 -> [_ w339]
      frame False {
      }
      frame True {
        n2047 = property on="X Step PV" class="DigNum (strict)"() -> ("Value"=w333:i32)  [unwired: 2 in, 2 out]
        n2048 = property on="Y Step PV" class="DigNum (strict)"() -> ("Value"=w332:i32)  [unwired: 2 in, 2 out]
        n2049 = property on="Z Step PV" class="DigNum (strict)"() -> ("Value"=w330:i32)  [unwired: 2 in, 2 out]
        n2050 = property on="R Step PV" class="DigNum (strict)"() -> ("Value"=w331:i32)  [unwired: 2 in, 2 out]
        n2051 = Build Array(w333, w332, w330, w331) -> (w336:i32[])
        n2052 = Build Array (concatenate)(w339, "String") -> (w334:string[])
        n2053 = local read "Presets"() -> (w337:i32[][])
        n2054 = property on="Preset positions" class="Ring (strict)"("Strings []"=w334) -> ()  [unwired: 2 in, 2 out]
        n2055 = Build Array (concatenate)(w337, w336) -> (w335:i32[][])
        n2056 = local write "Presets"(w335) -> ()
      }
    }
    n2057 = case shown="False" "Set Button" {
      tunnel: "Preset positions" -> [_ w346]
      frame False {
      }
      frame True {
        n2058 = local read "Presets"() -> (w347:i32[][])
        n2059 = Index Array(array=w347, index (row)=w346) -> (element=w345:i32[])  [unwired: 1 in]
        n2060 = Array To Cluster(array=w345) -> (cluster=w344:T11)
        n2061 = Unbundle(w344) -> ("Presets[0]"=w343:i32, "Presets[1]"=w342:i32, "Presets[2]"=w341:i32, "Presets[3]"=w340:i32)  [unwired: 5 out]
        n2062 = property on="X Step SP" class="DigNum (strict)"("Val(Sgnl)"=w343) -> ()  [unwired: 2 in, 2 out]
        n2063 = property on="Y Step SP" class="DigNum (strict)"("Val(Sgnl)"=w342) -> ()  [unwired: 2 in, 2 out]
        n2064 = property on="Z Step SP" class="DigNum (strict)"("Val(Sgnl)"=w341) -> ()  [unwired: 2 in, 2 out]
        n2065 = property on="R Step SP" class="DigNum (strict)"("Val(Sgnl)"=w340) -> ()  [unwired: 2 in, 2 out]
      }
    }
    n2066 = property on="STATUS" class="Str"() -> ("Value"=w289:string)  [unwired: 2 in, 2 out]
    n2067 = Equal?(x=w289, y="SCANNING MODE" ("STATUS")) -> (x = y?=w287:bool)
    "Scanning" <- w287
    n2068 = case shown="True" "Laser Shutter" {
      tunnel: "SHUTTER SYNC" -> [w323 _]
      tunnel: w287 -> [w322 _]
      frame False {
        # "SHUTTER SLAVE MODE"
        n2069 = And(x=w323, y=w322) -> (x .and. y?=w324:bool)
        n2070 = case shown="False" w324 {
          frame False {
            # "CLOE SHUTTER"
          }
          frame True {
            # "OPEN SHUTTER"
          }
        }
      }
      frame True {
        # "FORCE TO OPEN SHUTTER"
      }
    }
    n2071 = case shown="True" "Stop" {
      selector: "Stop" -> [w356 w398]
      tunnel: [w356 w395] -> w303
      tunnel: w286 -> [w355 w364]
      tunnel: w283 -> [w354 w363]
      tunnel: [w355 w371] -> w312
      tunnel: [w353 w377] -> w311
      tunnel: [w352 w374] -> w310
      tunnel: [w351 w383] -> w309
      tunnel: [w349 w366] -> w308
      tunnel: [w348 w365] -> w307
      tunnel: [w350 w380] -> w306
      tunnel: [w354 w368] -> w305
      tunnel: w302 -> [_ w390]
      tunnel: w301 -> [_ w367]
      tunnel: w285 -> [w353 w362]
      tunnel: w284 -> [w352 w361]
      tunnel: w282 -> [w351 w360]
      tunnel: w281 -> [w350 w359]
      tunnel: w280 -> [w348 w358]
      tunnel: w279 -> [w349 w357]
      frame False {
      }
      frame True {
        n2072 = flat-sequence {
          tunnel: w398 -> [w464]
          tunnel: [w464] -> w397
          tunnel: [w463] -> w393
          tunnel: [w462] -> w391
          tunnel: w390 -> [w462]
          tunnel: [w417] -> w388
          tunnel: [w416] -> w386
          tunnel: [w426] -> w384
          tunnel: [w425] -> w381
          tunnel: [w436] -> w378
          tunnel: [w434] -> w375
          tunnel: [w445] -> w372
          tunnel: [w443] -> w369
          tunnel: w367 -> [w453]
          tunnel: w364 -> [w406]
          tunnel: w363 -> [w405]
          tunnel: w362 -> [w404]
          tunnel: w361 -> [w403]
          tunnel: w360 -> [w402]
          tunnel: w359 -> [w401]
          tunnel: w358 -> [w400]
          tunnel: w357 -> [w399]
          tunnel: w397 -> [w476]
          tunnel: [w476] -> w396
          tunnel: [w465] -> w394
          tunnel: w393 -> [w475]
          tunnel: [w474] -> w392
          tunnel: w391 -> [w474]
          tunnel: [w473] -> w389
          tunnel: w388 -> [w473]
          tunnel: [w472] -> w387
          tunnel: w386 -> [w472]
          tunnel: [w471] -> w385
          tunnel: w384 -> [w471]
          tunnel: [w470] -> w382
          tunnel: w381 -> [w470]
          tunnel: [w469] -> w379
          tunnel: w378 -> [w469]
          tunnel: [w468] -> w376
          tunnel: w375 -> [w468]
          tunnel: [w467] -> w373
          tunnel: w372 -> [w467]
          tunnel: [w466] -> w370
          tunnel: w369 -> [w466]
          tunnel: w396 -> [w488]
          tunnel: [w488] -> w395
          tunnel: w394 -> [w479]
          tunnel: w392 -> [w487]
          tunnel: w389 -> [w478]
          tunnel: [w478] -> _
          tunnel: w387 -> [w486]
          tunnel: [w486] -> w365
          tunnel: w385 -> [w485]
          tunnel: [w485] -> w383
          tunnel: [w484] -> w380
          tunnel: w382 -> [w484]
          tunnel: [w483] -> w377
          tunnel: w379 -> [w483]
          tunnel: [w482] -> w374
          tunnel: w376 -> [w482]
          tunnel: [w481] -> w371
          tunnel: w373 -> [w481]
          tunnel: [w480] -> w368
          tunnel: w370 -> [w480]
          tunnel: [w478] -> w366
          frame #0 {
            # "R"
            # "Y"
            # "Z"
            # "X"
            n2073 = local read "Presets"() -> (w452:i32[][])
            n2074 = property on="Preset positions" class="Ring (strict)"() -> ("Strings []"=w451:string[])  [unwired: 2 in, 2 out]
            n2075 = property on="R Ready" class="Bool (strict)"("Val(Sgnl)"=FALSE ("Value (Signaling)")) -> ()  [unwired: 2 in, 2 out]
            n2076 = property on="R in Range" class="Bool (strict)"("Val(Sgnl)"=FALSE ("Value (Signaling)")) -> ()  [unwired: 2 in, 2 out]
            n2077 = property on="Z in Range" class="Bool (strict)"("Val(Sgnl)"=FALSE ("Value (Signaling)")) -> ()  [unwired: 2 in, 2 out]
            n2078 = property on="Z Ready" class="Bool (strict)"("Val(Sgnl)"=FALSE ("Value (Signaling)")) -> ()  [unwired: 2 in, 2 out]
            n2079 = property on="Y in Range" class="Bool (strict)"("Val(Sgnl)"=FALSE ("Value (Signaling)")) -> ()  [unwired: 2 in, 2 out]
            n2080 = property on="X  in Range" class="Bool (strict)"("Val(Sgnl)"=FALSE ("Value (Signaling)")) -> ()  [unwired: 2 in, 2 out]
            n2081 = property on="Y Ready" class="Bool (strict)"("Val(Sgnl)"=FALSE ("Value (Signaling)")) -> ()  [unwired: 2 in, 2 out]
            n2082 = property on="X Ready" class="Bool (strict)"("Val(Sgnl)"=FALSE ("Value (Signaling)")) -> ()  [unwired: 2 in, 2 out]
            n2083 = Number To Fractional String(number=w452) -> (F-format string=w454:string[][])  [unwired: 3 in]
            n2084 = call "mDrive Send Command.vi"("error in (no error)"=w405, "Command"=T10."Stop", "VISA resource name"=w406) -> ("error out"=w444:errorcluster, "VISA resource name out"=w446:refnum<visa-resource-name>)  [unwired: 4 in, 1 out]
            n2085 = call "mDrive Send Command.vi"("error in (no error)"=w403, "Command"=T10."Stop", "VISA resource name"=w404) -> ("error out"=w435:errorcluster, "VISA resource name out"=w437:refnum<visa-resource-name>)  [unwired: 4 in, 1 out]
            n2086 = Transpose 2D Array(2D array=w454) -> (transposed array=w455:string[][])
            n2087 = call "mDrive Send Command.vi"("error in (no error)"=w401, "Command"=T10."Stop", "VISA resource name"=w402) -> ("error out"=w427:errorcluster, "VISA resource name out"=w428:refnum<visa-resource-name>)  [unwired: 4 in, 1 out]
            n2088 = call "mDrive Send Command.vi"("error in (no error)"=w400, "Command"=T10."Stop", "VISA resource name"=w399) -> ("error out"=w418:errorcluster, "VISA resource name out"=w419:refnum<visa-resource-name>)  [unwired: 4 in, 1 out]
            n2089 = Build Array (concatenate)(w451, w455) -> (w456:string[][])
            n2090 = Transpose 2D Array(2D array=w456) -> (transposed array=w457:string[][])
            n2091 = call "mDrive Send Command.vi"("error in (no error)"=w444, "Extra"="P", "Command"=T10."Print Parameter", "VISA resource name"=w446) -> ("error out"=w443:errorcluster, "read buffer"=w450:string, "VISA resource name out"=w445:refnum<visa-resource-name>)  [unwired: 3 in]
            n2092 = call "mDrive Send Command.vi"("error in (no error)"=w435, "Extra"="P", "Command"=T10."Print Parameter", "VISA resource name"=w437) -> ("error out"=w434:errorcluster, "read buffer"=w441:string, "VISA resource name out"=w436:refnum<visa-resource-name>)  [unwired: 3 in]
            n2093 = call "mDrive Send Command.vi"("error in (no error)"=w427, "Extra"="P", "Command"=T10."Print Parameter", "VISA resource name"=w428) -> ("error out"=w425:errorcluster, "read buffer"=w432:string, "VISA resource name out"=w426:refnum<visa-resource-name>)  [unwired: 3 in]
            n2094 = call "mDrive Send Command.vi"("error in (no error)"=w418, "Extra"="P", "Command"=T10."Print Parameter", "VISA resource name"=w419) -> ("error out"=w416:errorcluster, "read buffer"=w423:string, "VISA resource name out"=w417:refnum<visa-resource-name>)  [unwired: 3 in]
            n2095 = call-poly <vilib>:"Write To Spreadsheet File.vi"("2D data"=w457, "file path (dialog if empty)"=w453) -> ()  [unwired: 6 in, 1 out]
            n2096 = Decimal String To Number(string=w450, offset=0) -> (number=w442:i32)  [unwired: 1 in, 1 out]
            n2097 = Decimal String To Number(string=w441, offset=0) -> (number=w433:i32)  [unwired: 1 in, 1 out]
            n2098 = Decimal String To Number(string=w432, offset=0) -> (number=w424:i32)  [unwired: 1 in, 1 out]
            n2099 = Decimal String To Number(string=w423, offset=0) -> (number=w415:i32)  [unwired: 1 in, 1 out]
            n2100 = Build Array(w442, w424, w433, w415) -> (w463:i32[])
          }
          frame #1 {
            n2101 = To Double Precision Float(number=w475) -> (double precision float=w465:dbl[])
            n2102 = Wait (ms)(milliseconds to wait=u32 20) -> ()  [unwired: 1 out]
          }
          frame #2 {
            n2103 = call-poly <vilib>:"Write To Spreadsheet File.vi"("1D data"=w479, "file path (dialog if empty)"=w487) -> ()  [unwired: 6 in, 1 out]
          }
        }
      }
    }
  }
  n2104 = flat-sequence {
    tunnel: w58 -> [w4312]
    tunnel: w57 -> [w4309]
    frame #0 {
      n2105 = call "mDrive Send Command.vi"("error in (no error)"=w4309, "Command"=T10."Stop", "VISA resource name"=w4312) -> ("error out"=w4310:errorcluster, "VISA resource name out"=w4311:refnum<visa-resource-name>)  [unwired: 4 in, 1 out]
      n2106 = VISA Close(VISA resource name=w4311, error in (no error)=w4310) -> ()  [unwired: 1 out]
    }
  }
  n2107 = flat-sequence {
    tunnel: w52 -> [w4317]
    tunnel: w51 -> [w4314]
    frame #0 {
      n2108 = call "mDrive Send Command.vi"("error in (no error)"=w4314, "Command"=T10."Stop", "VISA resource name"=w4317) -> ("error out"=w4315:errorcluster, "VISA resource name out"=w4316:refnum<visa-resource-name>)  [unwired: 4 in, 1 out]
      n2109 = VISA Close(VISA resource name=w4316, error in (no error)=w4315) -> ()  [unwired: 1 out]
    }
  }
  n2110 = flat-sequence {
    tunnel: w50 -> [w4322]
    tunnel: w49 -> [w4319]
    frame #0 {
      n2111 = call "mDrive Send Command.vi"("error in (no error)"=w4319, "Command"=T10."Stop", "VISA resource name"=w4322) -> ("error out"=w4320:errorcluster, "VISA resource name out"=w4321:refnum<visa-resource-name>)  [unwired: 4 in, 1 out]
      n2112 = VISA Close(VISA resource name=w4321, error in (no error)=w4320) -> ()  [unwired: 1 out]
    }
  }
  n2113 = flat-sequence {
    tunnel: w48 -> [w4327]
    tunnel: w47 -> [w4324]
    frame #0 {
      n2114 = call "mDrive Send Command.vi"("error in (no error)"=w4324, "Command"=T10."Stop", "VISA resource name"=w4327) -> ("error out"=w4325:errorcluster, "VISA resource name out"=w4326:refnum<visa-resource-name>)  [unwired: 4 in, 1 out]
      n2115 = VISA Close(VISA resource name=w4326, error in (no error)=w4325) -> ()  [unwired: 1 out]
    }
  }
  "YCONSTArray" <- w46
  "XCONSTArray" <- w45
  "RCONSTArray" <- w44
  "ZCONSTArray" <- w43
  "RUNHOLDArray" <- w42
